vi "New Tutu Outer loop_PN.vi"(6 "Const psi2":dbl=-0.7854, 8 "Const psi1":dbl=0.7854, 11 "Measured stats":dbl[](array[numeric])=[1.0, 0.0, 0.0, 0.156025, 0.156025, 0.156025, 0.0, 0.0, 0.0]) -> (2 "Converged":bool=TRUE, 3 "Corrected stats":dbl[](array[numeric])=[0.5313101533513194, -2.164673295316678e-14, 0.0, 0.20114821816046824, 0.47554583238904846, 0.156025, 1.0016756706463598e-14, 0.0, 0.0] format="%#_3g")   [LabVIEW 2010]
uses:
  XW calib map/Map method.ctl
  XW calib map/XW_Map_Global.vi
panel:
  out "POST PROC. XW Map method":T1=enum."Const. Psi_eff (std.)"
  out "2D true PDF output":string="\t-3.411158E+0\t-3.342246E+0\t-3.273333E+0\t-3.204421E+0\t-3.135509E+0\t-3.066596E+0\t-2.997684E+0\t-2.928772E+0\t-2.859860E+0\t-2.790947E+0\t-2.722035E+0\t-2.653123E+0\t-2.584211E+0\t-2.515298E+0\t-2.446386E+0\t-2.377474E+0\t-2.308561E+0\t-2.239649E+0\t-2.170737E+0\t-2.101825E+0\t-2.032912E+0\t-1.964000E+0\t-1.895088E+0\t-1.826175E+0\t-1.757263E+0\t-1.688351E+0\t-1.619439E+0\t-1.550526E+0\t-1.481614E+0\t-1.412702E+0\t-1.343789E+0\t-1.274877E+0\t-1.205965E+0\t-1.137053E+0\t-1.068140E+0\t-9.992281E-1\t-9.303158E-1\t-8.614035E-1\t-7.924912E-1\t-7.235789E-1\t-6.546667E-1\t-5.857544E-1\t-5.168421E-1\t-4.479298E-1\t-3.790175E-1\t-3.101053E-1\t-2.411930E-1\t-1.722807E-1\t-1.033684E-1\t-3.445614E-2\t3.445614E-2\t1.033684E-1\t1.722807E-1\t2.411930E-1\t3.101053E-1\t3.790175E-1\t4.479298E-1\t5.168421E-1\t5.857544E-1\t6.546667E-1\t7.235789E-1\t7.924912E-1\t8.614035E-1\t9.303158E-1\t9.992281E-1\t1.068140E+0\t1.137053E+0\t1.205965E+0\t1.274877E+0\t1.343789E+0\t1.412702E+0\t1.481614E+0\t1.550526E+0\t1.619439E+0\t1.688351E+0\t1.757263E+0\t1.826175E+0\t1.895088E+0\t1.964000E+0\t2.032912E+0\t2.101825E+0\t2.170737E+0\t2.239649E+0\t2.308561E+0\t2.377474E+0\t2.446386E+0\t2.515298E+0\t2.584211E+0\t2.653123E+0\t2.722035E+0\t2.790947E+0\t2.859860E+0\t2.928772E+0\t2.997684E+0\t3.066596E+0\t3.135509E+0\t3.204421E+0\t3.273333E+0\t3.342246E+0\t3.411158E+0\r\n-1.694652E+0\t1.119788E-11\t1.826614E-11\t2.949991E-11\t4.716912E-11\t7.467200E-11\t1.170364E-10\t1.816130E-10\t2.790205E-10\t4.244127E-10\t6.391513E-10\t9.529760E-10\t1.406771E-9\t2.056022E-9\t2.975056E-9\t4.262119E-9\t6.045318E-9\t8.489374E-9\t1.180308E-8\t1.624718E-8\t2.214235E-8\t2.987668E-8\t3.991206E-8\t5.278845E-8\t6.912526E-8\t8.961850E-8\t1.150328E-7\t1.461869E-7\t1.839326E-7\t2.291246E-7\t2.825842E-7\t3.450539E-7\t4.171470E-7\t4.992917E-7\t5.916742E-7\t6.941830E-7\t8.063588E-7\t9.273544E-7\t1.055908E-6\t1.190336E-6\t1.328545E-6\t1.468067E-6\t1.606122E-6\t1.739699E-6\t1.865661E-6\t1.980863E-6\t2.082281E-6\t2.167141E-6\t2.233048E-6\t2.278096E-6\t2.300959E-6\t2.300959E-6\t2.278096E-6\t2.233048E-6\t2.167141E-6\t2.082281E-6\t1.980863E-6\t1.865661E-6\t1.739699E-6\t1.606122E-6\t1.468067E-6\t1.328545E-6\t1.190336E-6\t1.055908E-6\t9.273544E-7\t8.063588E-7\t6.941830E-7\t5.916742E-7\t4.992917E-7\t4.171470E-7\t3.450539E-7\t2.825842E-7\t2.291246E-7\t1.839326E-7\t1.461869E-7\t1.150328E-7\t8.961850E-8\t6.912526E-8\t5.278845E-8\t3.991206E-8\t2.987668E-8\t2.214235E-8\t1.624718E-8\t1.180308E-8\t8.489374E-9\t6.045318E-9\t4.262119E-9\t2.975056E-9\t2.056022E-9\t1.406771E-9\t9.529760E-10\t6.391513E-10\t4.244127E-10\t2.790205E-10\t1.816130E-10\t1.170364E-10\t7.467200E-11\t4.716912E-11\t2.949991E-11\t1.826614E-11\t1.119788E-11\r\n-1.649695E+0\t1.832407E-11\t2.989048E-11\t4.827329E-11\t7.718695E-11\t1.221923E-10\t1.915169E-10\t2.971893E-10\t4.565857E-10\t6.945037E-10\t1.045899E-9\t1.559438E-9\t2.302022E-9\t3.364448E-9\t4.868344E-9\t6.974479E-9\t9.892483E-9\t1.389191E-8\t1.931441E-8\t2.658668E-8\t3.623346E-8\t4.888983E-8\t6.531159E-8\t8.638237E-8\t1.131157E-7\t1.466506E-7\t1.882382E-7\t2.392185E-7\t3.009850E-7\t3.749366E-7\t4.624172E-7\t5.646419E-7\t6.826142E-7\t8.170348E-7\t9.682084E-7\t1.135952E-6\t1.319516E-6\t1.517511E-6\t1.727875E-6\t1.947852E-6\t2.174014E-6\t2.402326E-6\t2.628237E-6\t2.846822E-6\t3.052945E-6\t3.241460E-6\t3.407419E-6\t3.546282E-6\t3.654132E-6\t3.727847E-6\t3.765261E-6\t3.765261E-6\t3.727847E-6\t3.654132E-6\t3.546282E-6\t3.407419E-6\t3.241460E-6\t3.052945E-6\t2.846822E-6\t2.628237E-6\t2.402326E-6\t2.174014E-6\t1.947852E-6\t1.727875E-6\t1.517511E-6\t1.319516E-6\t1.135952E-6\t9.682084E-7\t8.170348E-7\t6.826142E-7\t5.646419E-7\t4.624172E-7\t3.749366E-7\t3.009850E-7\t2.392185E-7\t1.882382E-7\t1.466506E-7\t1.131157E-7\t8.638237E-8\t6.531159E-8\t4.888983E-8\t3.623346E-8\t2.658668E-8\t1.931441E-8\t1.389191E-8\t9.892483E-9\t6.974479E-9\t4.868344E-9\t3.364448E-9\t2.302022E-9\t1.559438E-9\t1.045899E-9\t6.945037E-10\t4.565857E-10\t2.971893E-10\t1.915169E-10\t1.221923E-10\t7.718695E-11\t4.827329E-11\t2.989048E-11\t1.832407E-11\r\n-1.604737E+0\t2.968549E-11\t4.842339E-11\t7.820403E-11\t1.250449E-10\t1.979549E-10\t3.102625E-10\t4.814547E-10\t7.396812E-10\t1.125115E-9\t1.694385E-9\t2.526332E-9\t3.729338E-9\t5.450497E-9\t7.886849E-9\t1.129884E-8\t1.602609E-8\t2.250526E-8\t3.128986E-8\t4.307114E-8\t5.869918E-8\t7.920284E-8\t1.058065E-7\t1.399418E-7\t1.832505E-7\t2.375779E-7\t3.049510E-7\t3.875404E-7\t4.876037E-7\t6.074074E-7\t7.491283E-7\t9.147351E-7\t1.105853E-6\t1.323618E-6\t1.568524E-6\t1.840274E-6\t2.137651E-6\t2.458409E-6\t2.799204E-6\t3.155572E-6\t3.521962E-6\t3.891833E-6\t4.257815E-6\t4.611928E-6\t4.945853E-6\t5.251253E-6\t5.520110E-6\t5.745073E-6\t5.919792E-6\t6.039213E-6\t6.099824E-6\t6.099824E-6\t6.039213E-6\t5.919792E-6\t5.745073E-6\t5.520110E-6\t5.251253E-6\t4.945853E-6\t4.611928E-6\t4.257815E-6\t3.891833E-6\t3.521962E-6\t3.155572E-6\t2.799204E-6\t2.458409E-6\t2.137651E-6\t1.840274E-6\t1.568524E-6\t1.323618E-6\t1.105853E-6\t9.147351E-7\t7.491283E-7\t6.074074E-7\t4.876037E-7\t3.875404E-7\t3.049510E-7\t2.375779E-7\t1.832505E-7\t1.399418E-7\t1.058065E-7\t7.920284E-8\t5.869918E-8\t4.307114E-8\t3.128986E-8\t2.250526E-8\t1.602609E-8\t1.129884E-8\t7.886849E-9\t5.450497E-9\t3.729338E-9\t2.526332E-9\t1.694385E-9\t1.125115E-9\t7.396812E-10\t4.814547E-10\t3.102625E-10\t1.979549E-10\t1.250449E-10\t7.820403E-11\t4.842339E-11\t2.968549E-11\r\n-1.559779E+0\t4.761048E-11\t7.766288E-11\t1.254260E-10\t2.005508E-10\t3.174859E-10\t4.976083E-10\t7.721714E-10\t1.186323E-9\t1.804493E-9\t2.717505E-9\t4.051806E-9\t5.981223E-9\t8.741670E-9\t1.264916E-8\t1.812142E-8\t2.570312E-8\t3.609461E-8\t5.018362E-8\t6.907878E-8\t9.414350E-8\t1.270279E-7\t1.696957E-7\t2.244428E-7\t2.939026E-7\t3.810346E-7\t4.890895E-7\t6.215489E-7\t7.820335E-7\t9.741782E-7\t1.201474E-6\t1.467080E-6\t1.773601E-6\t2.122859E-6\t2.515645E-6\t2.951486E-6\t3.428428E-6\t3.942870E-6\t4.489448E-6\t5.061001E-6\t5.648628E-6\t6.241838E-6\t6.828812E-6\t7.396748E-6\t7.932307E-6\t8.422117E-6\t8.853317E-6\t9.214120E-6\t9.494339E-6\t9.685870E-6\t9.783080E-6\t9.783080E-6\t9.685870E-6\t9.494339E-6\t9.214120E-6\t8.853317E-6\t8.422117E-6\t7.932307E-6\t7.396748E-6\t6.828812E-6\t6.241838E-6\t5.648628E-6\t5.061001E-6\t4.489448E-6\t3.942870E-6\t3.428428E-6\t2.951486E-6\t2.515645E-6\t2.122859E-6\t1.773601E-6\t1.467080E-6\t1.201474E-6\t9.741782E-7\t7.820335E-7\t6.215489E-7\t4.890895E-7\t3.810346E-7\t2.939026E-7\t2.244428E-7\t1.696957E-7\t1.270279E-7\t9.414350E-8\t6.907878E-8\t5.018362E-8\t3.609461E-8\t2.570312E-8\t1.812142E-8\t1.264916E-8\t8.741670E-9\t5.981223E-9\t4.051806E-9\t2.717505E-9\t1.804493E-9\t1.186323E-9\t7.721714E-10\t4.976083E-10\t3.174859E-10\t2.005508E-10\t1.254260E-10\t7.766288E-11\t4.761048E-11\r\n-1.514821E+0\t7.559567E-11\t1.233127E-10\t1.991507E-10\t3.184336E-10\t5.041025E-10\t7.900998E-10\t1.226050E-9\t1.883637E-9\t2.865164E-9\t4.314841E-9\t6.433437E-9\t9.496956E-9\t1.387998E-8\t2.008428E-8\t2.877310E-8\t4.081128E-8\t5.731084E-8\t7.968129E-8\t1.096829E-7\t1.494806E-7\t2.016942E-7\t2.694419E-7\t3.563691E-7\t4.666571E-7\t6.050047E-7\t7.765738E-7\t9.868922E-7\t1.241709E-6\t1.546795E-6\t1.907695E-6\t2.329421E-6\t2.816114E-6\t3.370664E-6\t3.994328E-6\t4.686354E-6\t5.443641E-6\t6.260469E-6\t7.128322E-6\t8.035831E-6\t8.968862E-6\t9.910759E-6\t1.084275E-5\t1.174452E-5\t1.259488E-5\t1.337259E-5\t1.405725E-5\t1.463013E-5\t1.507506E-5\t1.537917E-5\t1.553352E-5\t1.553352E-5\t1.537917E-5\t1.507506E-5\t1.463013E-5\t1.405725E-5\t1.337259E-5\t1.259488E-5\t1.174452E-5\t1.084275E-5\t9.910759E-6\t8.968862E-6\t8.035831E-6\t7.128322E-6\t6.260469E-6\t5.443641E-6\t4.686354E-6\t3.994328E-6\t3.370664E-6\t2.816114E-6\t2.329421E-6\t1.907695E-6\t1.546795E-6\t1.241709E-6\t9.868922E-7\t7.765738E-7\t6.050047E-7\t4.666571E-7\t3.563691E-7\t2.694419E-7\t2.016942E-7\t1.494806E-7\t1.096829E-7\t7.968129E-8\t5.731084E-8\t4.081128E-8\t2.877310E-8\t2.008428E-8\t1.387998E-8\t9.496956E-9\t6.433437E-9\t4.314841E-9\t2.865164E-9\t1.883637E-9\t1.226050E-9\t7.900998E-10\t5.041025E-10\t3.184336E-10\t1.991507E-10\t1.233127E-10\t7.559567E-11\r\n-1.469864E+0\t1.188304E-10\t1.938377E-10\t3.130490E-10\t5.005521E-10\t7.924089E-10\t1.241974E-9\t1.927252E-9\t2.960927E-9\t4.503809E-9\t6.782584E-9\t1.011285E-8\t1.492845E-8\t2.181822E-8\t3.157088E-8\t4.522902E-8\t6.415207E-8\t9.008806E-8\t1.252526E-7\t1.724128E-7\t2.349715E-7\t3.170472E-7\t4.235412E-7\t5.601837E-7\t7.335476E-7\t9.510191E-7\t1.220712E-6\t1.551316E-6\t1.951867E-6\t2.431438E-6\t2.998744E-6\t3.661664E-6\t4.426706E-6\t5.298415E-6\t6.278765E-6\t7.366574E-6\t8.556968E-6\t9.840956E-6\t1.120515E-5\t1.263168E-5\t1.409833E-5\t1.557892E-5\t1.704394E-5\t1.846144E-5\t1.979814E-5\t2.102065E-5\t2.209688E-5\t2.299740E-5\t2.369679E-5\t2.417483E-5\t2.441746E-5\t2.441746E-5\t2.417483E-5\t2.369679E-5\t2.299740E-5\t2.209688E-5\t2.102065E-5\t1.979814E-5\t1.846144E-5\t1.704394E-5\t1.557892E-5\t1.409833E-5\t1.263168E-5\t1.120515E-5\t9.840956E-6\t8.556968E-6\t7.366574E-6\t6.278765E-6\t5.298415E-6\t4.426706E-6\t3.661664E-6\t2.998744E-6\t2.431438E-6\t1.951867E-6\t1.551316E-6\t1.220712E-6\t9.510191E-7\t7.335476E-7\t5.601837E-7\t4.235412E-7\t3.170472E-7\t2.349715E-7\t1.724128E-7\t1.252526E-7\t9.008806E-8\t6.415207E-8\t4.522902E-8\t3.157088E-8\t2.181822E-8\t1.492845E-8\t1.011285E-8\t6.782584E-9\t4.503809E-9\t2.960927E-9\t1.927252E-9\t1.241974E-9\t7.924089E-10\t5.005521E-10\t3.130490E-10\t1.938377E-10\t1.188304E-10\r\n-1.424906E+0\t1.849243E-10\t3.016510E-10\t4.871680E-10\t7.789612E-10\t1.233150E-9\t1.932765E-9\t2.999198E-9\t4.607807E-9\t7.008845E-9\t1.055509E-8\t1.573766E-8\t2.323172E-8\t3.395360E-8\t4.913073E-8\t7.038558E-8\t9.983371E-8\t1.401954E-7\t1.949186E-7\t2.683095E-7\t3.656636E-7\t4.933901E-7\t6.591165E-7\t8.717601E-7\t1.141550E-6\t1.479980E-6\t1.899677E-6\t2.414163E-6\t3.037503E-6\t3.783814E-6\t4.666657E-6\t5.698296E-6\t6.888858E-6\t8.245414E-6\t9.771039E-6\t1.146389E-5\t1.331639E-5\t1.531454E-5\t1.743750E-5\t1.965748E-5\t2.193988E-5\t2.424398E-5\t2.652385E-5\t2.872977E-5\t3.080994E-5\t3.271242E-5\t3.438725E-5\t3.578864E-5\t3.687704E-5\t3.762097E-5\t3.799855E-5\t3.799855E-5\t3.762097E-5\t3.687704E-5\t3.578864E-5\t3.438725E-5\t3.271242E-5\t3.080994E-5\t2.872977E-5\t2.652385E-5\t2.424398E-5\t2.193988E-5\t1.965748E-5\t1.743750E-5\t1.531454E-5\t1.331639E-5\t1.146389E-5\t9.771039E-6\t8.245414E-6\t6.888858E-6\t5.698296E-6\t4.666657E-6\t3.783814E-6\t3.037503E-6\t2.414163E-6\t1.899677E-6\t1.479980E-6\t1.141550E-6\t8.717601E-7\t6.591165E-7\t4.933901E-7\t3.656636E-7\t2.683095E-7\t1.949186E-7\t1.401954E-7\t9.983371E-8\t7.038558E-8\t4.913073E-8\t3.395360E-8\t2.323172E-8\t1.573766E-8\t1.055509E-8\t7.008845E-9\t4.607807E-9\t2.999198E-9\t1.932765E-9\t1.233150E-9\t7.789612E-10\t4.871680E-10\t3.016510E-10\t1.849243E-10\r\n-1.379948E+0\t2.849027E-10\t4.647372E-10\t7.505530E-10\t1.200103E-9\t1.899846E-9\t2.977704E-9\t4.620699E-9\t7.098995E-9\t1.079814E-8\t1.626164E-8\t2.424614E-8\t3.579184E-8\t5.231044E-8\t7.569302E-8\t1.084392E-7\t1.538083E-7\t2.159913E-7\t3.003004E-7\t4.133697E-7\t5.633578E-7\t7.601390E-7\t1.015465E-6\t1.343073E-6\t1.758723E-6\t2.280123E-6\t2.926728E-6\t3.719369E-6\t4.679714E-6\t5.829514E-6\t7.189662E-6\t8.779052E-6\t1.061328E-5\t1.270326E-5\t1.505370E-5\t1.766179E-5\t2.051583E-5\t2.359426E-5\t2.686500E-5\t3.028519E-5\t3.380157E-5\t3.735137E-5\t4.086383E-5\t4.426238E-5\t4.746718E-5\t5.039822E-5\t5.297854E-5\t5.513760E-5\t5.681444E-5\t5.796057E-5\t5.854227E-5\t5.854227E-5\t5.796057E-5\t5.681444E-5\t5.513760E-5\t5.297854E-5\t5.039822E-5\t4.746718E-5\t4.426238E-5\t4.086383E-5\t3.735137E-5\t3.380157E-5\t3.028519E-5\t2.686500E-5\t2.359426E-5\t2.051583E-5\t1.766179E-5\t1.505370E-5\t1.270326E-5\t1.061328E-5\t8.779052E-6\t7.189662E-6\t5.829514E-6\t4.679714E-6\t3.719369E-6\t2.926728E-6\t2.280123E-6\t1.758723E-6\t1.343073E-6\t1.015465E-6\t7.601390E-7\t5.633578E-7\t4.133697E-7\t3.003004E-7\t2.159913E-7\t1.538083E-7\t1.084392E-7\t7.569302E-8\t5.231044E-8\t3.579184E-8\t2.424614E-8\t1.626164E-8\t1.079814E-8\t7.098995E-9\t4.620699E-9\t2.977704E-9\t1.899846E-9\t1.200103E-9\t7.505530E-10\t4.647372E-10\t2.849027E-10\r\n-1.334990E+0\t4.345454E-10\t7.088365E-10\t1.144775E-9\t1.830447E-9\t2.897725E-9\t4.541718E-9\t7.047683E-9\t1.082768E-8\t1.646978E-8\t2.480293E-8\t3.698123E-8\t5.459120E-8\t7.978606E-8\t1.154501E-7\t1.653960E-7\t2.345948E-7\t3.294390E-7\t4.580307E-7\t6.304886E-7\t8.592568E-7\t1.159396E-6\t1.548829E-6\t2.048511E-6\t2.682478E-6\t3.477739E-6\t4.463967E-6\t5.672937E-6\t7.137695E-6\t8.891418E-6\t1.096597E-5\t1.339018E-5\t1.618782E-5\t1.937554E-5\t2.296054E-5\t2.693849E-5\t3.129159E-5\t3.598695E-5\t4.097562E-5\t4.619224E-5\t5.155557E-5\t5.696986E-5\t6.232722E-5\t6.751083E-5\t7.239893E-5\t7.686947E-5\t8.080508E-5\t8.409816E-5\t8.665575E-5\t8.840387E-5\t8.929111E-5\t8.929111E-5\t8.840387E-5\t8.665575E-5\t8.409816E-5\t8.080508E-5\t7.686947E-5\t7.239893E-5\t6.751083E-5\t6.232722E-5\t5.696986E-5\t5.155557E-5\t4.619224E-5\t4.097562E-5\t3.598695E-5\t3.129159E-5\t2.693849E-5\t2.296054E-5\t1.937554E-5\t1.618782E-5\t1.339018E-5\t1.096597E-5\t8.891418E-6\t7.137695E-6\t5.672937E-6\t4.463967E-6\t3.477739E-6\t2.682478E-6\t2.048511E-6\t1.548829E-6\t1.159396E-6\t8.592568E-7\t6.304886E-7\t4.580307E-7\t3.294390E-7\t2.345948E-7\t1.653960E-7\t1.154501E-7\t7.978606E-8\t5.459120E-8\t3.698123E-8\t2.480293E-8\t1.646978E-8\t1.082768E-8\t7.047683E-9\t4.541718E-9\t2.897725E-9\t1.830447E-9\t1.144775E-9\t7.088365E-10\t4.345454E-10\r\n-1.290033E+0\t6.561602E-10\t1.070338E-9\t1.728601E-9\t2.763960E-9\t4.375542E-9\t6.857960E-9\t1.064195E-8\t1.634972E-8\t2.486924E-8\t3.745224E-8\t5.584137E-8\t8.243230E-8\t1.204763E-7\t1.743288E-7\t2.497467E-7\t3.542364E-7\t4.974504E-7\t6.916229E-7\t9.520330E-7\t1.297471E-6\t1.750679E-6\t2.338720E-6\t3.093236E-6\t4.050521E-6\t5.251360E-6\t6.740556E-6\t8.566091E-6\t1.077786E-5\t1.342597E-5\t1.655853E-5\t2.021906E-5\t2.444349E-5\t2.925691E-5\t3.467023E-5\t4.067692E-5\t4.725007E-5\t5.434003E-5\t6.187287E-5\t6.974993E-5\t7.784851E-5\t8.602405E-5\t9.411363E-5\t1.019408E-4\t1.093218E-4\t1.160723E-4\t1.220151E-4\t1.269876E-4\t1.308495E-4\t1.334892E-4\t1.348289E-4\t1.348289E-4\t1.334892E-4\t1.308495E-4\t1.269876E-4\t1.220151E-4\t1.160723E-4\t1.093218E-4\t1.019408E-4\t9.411363E-5\t8.602405E-5\t7.784851E-5\t6.974993E-5\t6.187287E-5\t5.434003E-5\t4.725007E-5\t4.067692E-5\t3.467023E-5\t2.925691E-5\t2.444349E-5\t2.021906E-5\t1.655853E-5\t1.342597E-5\t1.077786E-5\t8.566091E-6\t6.740556E-6\t5.251360E-6\t4.050521E-6\t3.093236E-6\t2.338720E-6\t1.750679E-6\t1.297471E-6\t9.520330E-7\t6.916229E-7\t4.974504E-7\t3.542364E-7\t2.497467E-7\t1.743288E-7\t1.204763E-7\t8.243230E-8\t5.584137E-8\t3.745224E-8\t2.486924E-8\t1.634972E-8\t1.064195E-8\t6.857960E-9\t4.375542E-9\t2.763960E-9\t1.728601E-9\t1.070338E-9\t6.561602E-10\r\n-1.245075E+0\t9.808909E-10\t1.600043E-9\t2.584078E-9\t4.131832E-9\t6.540978E-9\t1.025193E-8\t1.590860E-8\t2.444112E-8\t3.717691E-8\t5.598718E-8\t8.347701E-8\t1.232277E-7\t1.800995E-7\t2.606034E-7\t3.733451E-7\t5.295464E-7\t7.436363E-7\t1.033904E-6\t1.423190E-6\t1.939584E-6\t2.617081E-6\t3.496142E-6\t4.624064E-6\t6.055105E-6\t7.850233E-6\t1.007643E-5\t1.280541E-5\t1.611178E-5\t2.007043E-5\t2.475328E-5\t3.022539E-5\t3.654046E-5\t4.373602E-5\t5.182837E-5\t6.080774E-5\t7.063391E-5\t8.123266E-5\t9.249348E-5\t1.042689E-4\t1.163754E-4\t1.285970E-4\t1.406900E-4\t1.523909E-4\t1.634247E-4\t1.735160E-4\t1.823997E-4\t1.898331E-4\t1.956063E-4\t1.995523E-4\t2.015551E-4\t2.015551E-4\t1.995523E-4\t1.956063E-4\t1.898331E-4\t1.823997E-4\t1.735160E-4\t1.634247E-4\t1.523909E-4\t1.406900E-4\t1.285970E-4\t1.163754E-4\t1.042689E-4\t9.249348E-5\t8.123266E-5\t7.063391E-5\t6.080774E-5\t5.182837E-5\t4.373602E-5\t3.654046E-5\t3.022539E-5\t2.475328E-5\t2.007043E-5\t1.611178E-5\t1.280541E-5\t1.007643E-5\t7.850233E-6\t6.055105E-6\t4.624064E-6\t3.496142E-6\t2.617081E-6\t1.939584E-6\t1.423190E-6\t1.033904E-6\t7.436363E-7\t5.295464E-7\t3.733451E-7\t2.606034E-7\t1.800995E-7\t1.232277E-7\t8.347701E-8\t5.598718E-8\t3.717691E-8\t2.444112E-8\t1.590860E-8\t1.025193E-8\t6.540978E-9\t4.131832E-9\t2.584078E-9\t1.600043E-9\t9.808909E-10\r\n-1.200117E+0\t1.451669E-9\t2.367983E-9\t3.824305E-9\t6.114902E-9\t9.680316E-9\t1.517234E-8\t2.354392E-8\t3.617162E-8\t5.501995E-8\t8.285819E-8\t1.235417E-7\t1.823707E-7\t2.665382E-7\t3.856798E-7\t5.525319E-7\t7.837019E-7\t1.100544E-6\t1.530126E-6\t2.106249E-6\t2.870486E-6\t3.873148E-6\t5.174113E-6\t6.843381E-6\t8.961249E-6\t1.161795E-5\t1.491260E-5\t1.895136E-5\t2.384462E-5\t2.970322E-5\t3.663360E-5\t4.473204E-5\t5.407804E-5\t6.472710E-5\t7.670337E-5\t8.999239E-5\t1.045346E-4\t1.202202E-4\t1.368857E-4\t1.543126E-4\t1.722297E-4\t1.903170E-4\t2.082141E-4\t2.255308E-4\t2.418603E-4\t2.567949E-4\t2.699424E-4\t2.809435E-4\t2.894875E-4\t2.953274E-4\t2.982914E-4\t2.982914E-4\t2.953274E-4\t2.894875E-4\t2.809435E-4\t2.699424E-4\t2.567949E-4\t2.418603E-4\t2.255308E-4\t2.082141E-4\t1.903170E-4\t1.722297E-4\t1.543126E-4\t1.368857E-4\t1.202202E-4\t1.045346E-4\t8.999239E-5\t7.670337E-5\t6.472710E-5\t5.407804E-5\t4.473204E-5\t3.663360E-5\t2.970322E-5\t2.384462E-5\t1.895136E-5\t1.491260E-5\t1.161795E-5\t8.961249E-6\t6.843381E-6\t5.174113E-6\t3.873148E-6\t2.870486E-6\t2.106249E-6\t1.530126E-6\t1.100544E-6\t7.837019E-7\t5.525319E-7\t3.856798E-7\t2.665382E-7\t1.823707E-7\t1.235417E-7\t8.285819E-8\t5.501995E-8\t3.617162E-8\t2.354392E-8\t1.517234E-8\t9.680316E-9\t6.114902E-9\t3.824305E-9\t2.367983E-9\t1.451669E-9\r\n-1.155159E+0\t2.126917E-9\t3.469457E-9\t5.603191E-9\t8.959267E-9\t1.418314E-8\t2.222980E-8\t3.449544E-8\t5.299695E-8\t8.061264E-8\t1.213999E-7\t1.810076E-7\t2.672010E-7\t3.905192E-7\t5.650799E-7\t8.095438E-7\t1.148243E-6\t1.612465E-6\t2.241868E-6\t3.085977E-6\t4.205701E-6\t5.674754E-6\t7.580866E-6\t1.002660E-5\t1.312960E-5\t1.702207E-5\t2.184924E-5\t2.776664E-5\t3.493601E-5\t4.351975E-5\t5.367382E-5\t6.553928E-5\t7.923260E-5\t9.483510E-5\t1.123822E-4\t1.318526E-4\t1.531592E-4\t1.761410E-4\t2.005584E-4\t2.260916E-4\t2.523428E-4\t2.788435E-4\t3.050655E-4\t3.304371E-4\t3.543623E-4\t3.762437E-4\t3.955069E-4\t4.116251E-4\t4.241434E-4\t4.326998E-4\t4.370425E-4\t4.370425E-4\t4.326998E-4\t4.241434E-4\t4.116251E-4\t3.955069E-4\t3.762437E-4\t3.543623E-4\t3.304371E-4\t3.050655E-4\t2.788435E-4\t2.523428E-4\t2.260916E-4\t2.005584E-4\t1.761410E-4\t1.531592E-4\t1.318526E-4\t1.123822E-4\t9.483510E-5\t7.923260E-5\t6.553928E-5\t5.367382E-5\t4.351975E-5\t3.493601E-5\t2.776664E-5\t2.184924E-5\t1.702207E-5\t1.312960E-5\t1.002660E-5\t7.580866E-6\t5.674754E-6\t4.205701E-6\t3.085977E-6\t2.241868E-6\t1.612465E-6\t1.148243E-6\t8.095438E-7\t5.650799E-7\t3.905192E-7\t2.672010E-7\t1.810076E-7\t1.213999E-7\t8.061264E-8\t5.299695E-8\t3.449544E-8\t2.222980E-8\t1.418314E-8\t8.959267E-9\t5.603191E-9\t3.469457E-9\t2.126917E-9\r\n-1.110201E+0\t3.085102E-9\t5.032462E-9\t8.127453E-9\t1.299546E-8\t2.057271E-8\t3.224442E-8\t5.003579E-8\t7.687231E-8\t1.169290E-7\t1.760911E-7\t2.625522E-7\t3.875762E-7\t5.664499E-7\t8.196509E-7\t1.174247E-6\t1.665532E-6\t2.338888E-6\t3.251839E-6\t4.476223E-6\t6.100387E-6\t8.231256E-6\t1.099608E-5\t1.454363E-5\t1.904454E-5\t2.469059E-5\t3.169242E-5\t4.027563E-5\t5.067484E-5\t6.312559E-5\t7.785411E-5\t9.506501E-5\t1.149272E-4\t1.375587E-4\t1.630108E-4\t1.912528E-4\t2.221581E-4\t2.554933E-4\t2.909109E-4\t3.279468E-4\t3.660244E-4\t4.044637E-4\t4.424989E-4\t4.793005E-4\t5.140041E-4\t5.457432E-4\t5.736845E-4\t5.970640E-4\t6.152219E-4\t6.276329E-4\t6.339320E-4\t6.339320E-4\t6.276329E-4\t6.152219E-4\t5.970640E-4\t5.736845E-4\t5.457432E-4\t5.140041E-4\t4.793005E-4\t4.424989E-4\t4.044637E-4\t3.660244E-4\t3.279468E-4\t2.909109E-4\t2.554933E-4\t2.221581E-4\t1.912528E-4\t1.630108E-4\t1.375587E-4\t1.149272E-4\t9.506501E-5\t7.785411E-5\t6.312559E-5\t5.067484E-5\t4.027563E-5\t3.169242E-5\t2.469059E-5\t1.904454E-5\t1.454363E-5\t1.099608E-5\t8.231256E-6\t6.100387E-6\t4.476223E-6\t3.251839E-6\t2.338888E-6\t1.665532E-6\t1.174247E-6\t8.196509E-7\t5.664499E-7\t3.875762E-7\t2.625522E-7\t1.760911E-7\t1.169290E-7\t7.687231E-8\t5.003579E-8\t3.224442E-8\t2.057271E-8\t1.299546E-8\t8.127453E-9\t5.032462E-9\t3.085102E-9\r\n-1.065244E+0\t4.430214E-9\t7.226627E-9\t1.167104E-8\t1.866150E-8\t2.954246E-8\t4.630306E-8\t7.185150E-8\t1.103888E-7\t1.679103E-7\t2.528672E-7\t3.770256E-7\t5.565602E-7\t8.134232E-7\t1.177020E-6\t1.686221E-6\t2.391707E-6\t3.358648E-6\t4.669648E-6\t6.427866E-6\t8.760169E-6\t1.182010E-5\t1.579039E-5\t2.088468E-5\t2.734800E-5\t3.545574E-5\t4.551038E-5\t5.783590E-5\t7.276918E-5\t9.064849E-5\t1.117987E-4\t1.365136E-4\t1.650357E-4\t1.975346E-4\t2.340839E-4\t2.746394E-4\t3.190195E-4\t3.668889E-4\t4.177487E-4\t4.709324E-4\t5.256118E-4\t5.808108E-4\t6.354294E-4\t6.882765E-4\t7.381110E-4\t7.836884E-4\t8.238121E-4\t8.573853E-4\t8.834600E-4\t9.012822E-4\t9.103277E-4\t9.103277E-4\t9.012822E-4\t8.834600E-4\t8.573853E-4\t8.238121E-4\t7.836884E-4\t7.381110E-4\t6.882765E-4\t6.354294E-4\t5.808108E-4\t5.256118E-4\t4.709324E-4\t4.177487E-4\t3.668889E-4\t3.190195E-4\t2.746394E-4\t2.340839E-4\t1.975346E-4\t1.650357E-4\t1.365136E-4\t1.117987E-4\t9.064849E-5\t7.276918E-5\t5.783590E-5\t4.551038E-5\t3.545574E-5\t2.734800E-5\t2.088468E-5\t1.579039E-5\t1.182010E-5\t8.760169E-6\t6.427866E-6\t4.669648E-6\t3.358648E-6\t2.391707E-6\t1.686221E-6\t1.177020E-6\t8.134232E-7\t5.565602E-7\t3.770256E-7\t2.528672E-7\t1.679103E-7\t1.103888E-7\t7.185150E-8\t4.630306E-8\t2.954246E-8\t1.866150E-8\t1.167104E-8\t7.226627E-9\t4.430214E-9\r\n-1.020286E+0\t6.298192E-9\t1.027370E-8\t1.659208E-8\t2.653003E-8\t4.199889E-8\t6.582652E-8\t1.021473E-7\t1.569337E-7\t2.387088E-7\t3.594874E-7\t5.359966E-7\t7.912311E-7\t1.156399E-6\t1.673305E-6\t2.397208E-6\t3.400158E-6\t4.774806E-6\t6.638582E-6\t9.138143E-6\t1.245385E-5\t1.680399E-5\t2.244834E-5\t2.969060E-5\t3.887915E-5\t5.040548E-5\t6.469961E-5\t8.222211E-5\t1.034519E-4\t1.288700E-4\t1.589380E-4\t1.940738E-4\t2.346222E-4\t2.808241E-4\t3.327842E-4\t3.904397E-4\t4.535325E-4\t5.215858E-4\t5.938903E-4\t6.694987E-4\t7.472334E-4\t8.257068E-4\t9.033550E-4\t9.784849E-4\t1.049332E-3\t1.114127E-3\t1.171168E-3\t1.218898E-3\t1.255967E-3\t1.281303E-3\t1.294163E-3\t1.294163E-3\t1.281303E-3\t1.255967E-3\t1.218898E-3\t1.171168E-3\t1.114127E-3\t1.049332E-3\t9.784849E-4\t9.033550E-4\t8.257068E-4\t7.472334E-4\t6.694987E-4\t5.938903E-4\t5.215858E-4\t4.535325E-4\t3.904397E-4\t3.327842E-4\t2.808241E-4\t2.346222E-4\t1.940738E-4\t1.589380E-4\t1.288700E-4\t1.034519E-4\t8.222211E-5\t6.469961E-5\t5.040548E-5\t3.887915E-5\t2.969060E-5\t2.244834E-5\t1.680399E-5\t1.245385E-5\t9.138143E-6\t6.638582E-6\t4.774806E-6\t3.400158E-6\t2.397208E-6\t1.673305E-6\t1.156399E-6\t7.912311E-7\t5.359966E-7\t3.594874E-7\t2.387088E-7\t1.569337E-7\t1.021473E-7\t6.582652E-8\t4.199889E-8\t2.653003E-8\t1.659208E-8\t1.027370E-8\t6.298192E-9\r\n-9.753281E-1\t8.864273E-9\t1.445953E-8\t2.335221E-8\t3.733920E-8\t5.911056E-8\t9.264632E-8\t1.437654E-7\t2.208734E-7\t3.359663E-7\t5.059539E-7\t7.543784E-7\t1.113604E-6\t1.627552E-6\t2.355062E-6\t3.373905E-6\t4.785490E-6\t6.720212E-6\t9.343349E-6\t1.286131E-5\t1.752794E-5\t2.365046E-5\t3.159449E-5\t4.178748E-5\t5.471974E-5\t7.094225E-5\t9.106026E-5\t1.157220E-4\t1.456015E-4\t1.813756E-4\t2.236944E-4\t2.731456E-4\t3.302147E-4\t3.952407E-4\t4.683709E-4\t5.495172E-4\t6.383159E-4\t7.340963E-4\t8.358599E-4\t9.422735E-4\t1.051680E-3\t1.162126E-3\t1.271410E-3\t1.377150E-3\t1.476863E-3\t1.568057E-3\t1.648339E-3\t1.715515E-3\t1.767687E-3\t1.803347E-3\t1.821445E-3\t1.821445E-3\t1.803347E-3\t1.767687E-3\t1.715515E-3\t1.648339E-3\t1.568057E-3\t1.476863E-3\t1.377150E-3\t1.271410E-3\t1.162126E-3\t1.051680E-3\t9.422735E-4\t8.358599E-4\t7.340963E-4\t6.383159E-4\t5.495172E-4\t4.683709E-4\t3.952407E-4\t3.302147E-4\t2.731456E-4\t2.236944E-4\t1.813756E-4\t1.456015E-4\t1.157220E-4\t9.106026E-5\t7.094225E-5\t5.471974E-5\t4.178748E-5\t3.159449E-5\t2.365046E-5\t1.752794E-5\t1.286131E-5\t9.343349E-6\t6.720212E-6\t4.785490E-6\t3.373905E-6\t2.355062E-6\t1.627552E-6\t1.113604E-6\t7.543784E-7\t5.059539E-7\t3.359663E-7\t2.208734E-7\t1.437654E-7\t9.264632E-8\t5.911056E-8\t3.733920E-8\t2.335221E-8\t1.445953E-8\t8.864273E-9\r\n-9.303704E-1\t1.235112E-8\t2.014732E-8\t3.253803E-8\t5.202694E-8\t8.236228E-8\t1.290897E-7\t2.003169E-7\t3.077562E-7\t4.681219E-7\t7.049759E-7\t1.051121E-6\t1.551651E-6\t2.267766E-6\t3.281450E-6\t4.701064E-6\t6.667910E-6\t9.363674E-6\t1.301865E-5\t1.792043E-5\t2.442273E-5\t3.295361E-5\t4.402250E-5\t5.822500E-5\t7.624430E-5\t9.884809E-5\t1.268797E-4\t1.612424E-4\t2.028753E-4\t2.527216E-4\t3.116868E-4\t3.805902E-4\t4.601080E-4\t5.507126E-4\t6.526093E-4\t7.656752E-4\t8.894037E-4\t1.022860E-3\t1.164654E-3\t1.312926E-3\t1.465368E-3\t1.619259E-3\t1.771532E-3\t1.918866E-3\t2.057801E-3\t2.184868E-3\t2.296730E-3\t2.390329E-3\t2.463024E-3\t2.512711E-3\t2.537929E-3\t2.537929E-3\t2.512711E-3\t2.463024E-3\t2.390329E-3\t2.296730E-3\t2.184868E-3\t2.057801E-3\t1.918866E-3\t1.771532E-3\t1.619259E-3\t1.465368E-3\t1.312926E-3\t1.164654E-3\t1.022860E-3\t8.894037E-4\t7.656752E-4\t6.526093E-4\t5.507126E-4\t4.601080E-4\t3.805902E-4\t3.116868E-4\t2.527216E-4\t2.028753E-4\t1.612424E-4\t1.268797E-4\t9.884809E-5\t7.624430E-5\t5.822500E-5\t4.402250E-5\t3.295361E-5\t2.442273E-5\t1.792043E-5\t1.301865E-5\t9.363674E-6\t6.667910E-6\t4.701064E-6\t3.281450E-6\t2.267766E-6\t1.551651E-6\t1.051121E-6\t7.049759E-7\t4.681219E-7\t3.077562E-7\t2.003169E-7\t1.290897E-7\t8.236228E-8\t5.202694E-8\t3.253803E-8\t2.014732E-8\t1.235112E-8\r\n-8.854126E-1\t1.703750E-8\t2.779180E-8\t4.488391E-8\t7.176748E-8\t1.136129E-7\t1.780700E-7\t2.763230E-7\t4.245278E-7\t6.457410E-7\t9.724643E-7\t1.449946E-6\t2.140392E-6\t3.128223E-6\t4.526527E-6\t6.484785E-6\t9.197909E-6\t1.291652E-5\t1.795830E-5\t2.471997E-5\t3.368942E-5\t4.545716E-5\t6.072592E-5\t8.031726E-5\t1.051736E-4\t1.363539E-4\t1.750216E-4\t2.224224E-4\t2.798521E-4\t3.486115E-4\t4.299498E-4\t5.249971E-4\t6.346863E-4\t7.596689E-4\t9.002283E-4\t1.056195E-3\t1.226869E-3\t1.410963E-3\t1.606557E-3\t1.811089E-3\t2.021372E-3\t2.233653E-3\t2.443703E-3\t2.646940E-3\t2.838591E-3\t3.013870E-3\t3.168176E-3\t3.297290E-3\t3.397567E-3\t3.466107E-3\t3.500893E-3\t3.500893E-3\t3.466107E-3\t3.397567E-3\t3.297290E-3\t3.168176E-3\t3.013870E-3\t2.838591E-3\t2.646940E-3\t2.443703E-3\t2.233653E-3\t2.021372E-3\t1.811089E-3\t1.606557E-3\t1.410963E-3\t1.226869E-3\t1.056195E-3\t9.002283E-4\t7.596689E-4\t6.346863E-4\t5.249971E-4\t4.299498E-4\t3.486115E-4\t2.798521E-4\t2.224224E-4\t1.750216E-4\t1.363539E-4\t1.051736E-4\t8.031726E-5\t6.072592E-5\t4.545716E-5\t3.368942E-5\t2.471997E-5\t1.795830E-5\t1.291652E-5\t9.197909E-6\t6.484785E-6\t4.526527E-6\t3.128223E-6\t2.140392E-6\t1.449946E-6\t9.724643E-7\t6.457410E-7\t4.245278E-7\t2.763230E-7\t1.780700E-7\t1.136129E-7\t7.176748E-8\t4.488391E-8\t2.779180E-8\t1.703750E-8\r\n-8.404548E-1\t2.326705E-8\t3.795353E-8\t6.129516E-8\t9.800837E-8\t1.551541E-7\t2.431791E-7\t3.773570E-7\t5.797512E-7\t8.818482E-7\t1.328034E-6\t1.980101E-6\t2.923000E-6\t4.272019E-6\t6.181595E-6\t8.855866E-6\t1.256101E-5\t1.763929E-5\t2.452453E-5\t3.375852E-5\t4.600754E-5\t6.207801E-5\t8.292960E-5\t1.096843E-4\t1.436290E-4\t1.862101E-4\t2.390160E-4\t3.037484E-4\t3.821766E-4\t4.760769E-4\t5.871557E-4\t7.169558E-4\t8.667515E-4\t1.037432E-3\t1.229386E-3\t1.442379E-3\t1.675459E-3\t1.926865E-3\t2.193975E-3\t2.473291E-3\t2.760461E-3\t3.050361E-3\t3.337213E-3\t3.614761E-3\t3.876486E-3\t4.115854E-3\t4.326580E-3\t4.502903E-3\t4.639845E-3\t4.733446E-3\t4.780952E-3\t4.780952E-3\t4.733446E-3\t4.639845E-3\t4.502903E-3\t4.326580E-3\t4.115854E-3\t3.876486E-3\t3.614761E-3\t3.337213E-3\t3.050361E-3\t2.760461E-3\t2.473291E-3\t2.193975E-3\t1.926865E-3\t1.675459E-3\t1.442379E-3\t1.229386E-3\t1.037432E-3\t8.667515E-4\t7.169558E-4\t5.871557E-4\t4.760769E-4\t3.821766E-4\t3.037484E-4\t2.390160E-4\t1.862101E-4\t1.436290E-4\t1.096843E-4\t8.292960E-5\t6.207801E-5\t4.600754E-5\t3.375852E-5\t2.452453E-5\t1.763929E-5\t1.256101E-5\t8.855866E-6\t6.181595E-6\t4.272019E-6\t2.923000E-6\t1.980101E-6\t1.328034E-6\t8.818482E-7\t5.797512E-7\t3.773570E-7\t2.431791E-7\t1.551541E-7\t9.800837E-8\t6.129516E-8\t3.795353E-8\t2.326705E-8\r\n-7.954971E-1\t3.145667E-8\t5.131257E-8\t8.287007E-8\t1.325057E-7\t2.097658E-7\t3.287743E-7\t5.101806E-7\t7.838143E-7\t1.192245E-6\t1.795480E-6\t2.677065E-6\t3.951849E-6\t5.775701E-6\t8.357418E-6\t1.197299E-5\t1.698228E-5\t2.384804E-5\t3.315677E-5\t4.564097E-5\t6.220146E-5\t8.392847E-5\t1.121195E-4\t1.482914E-4\t1.941841E-4\t2.517530E-4\t3.231459E-4\t4.106630E-4\t5.166966E-4\t6.436484E-4\t7.938250E-4\t9.693128E-4\t1.171834E-3\t1.402592E-3\t1.662110E-3\t1.950073E-3\t2.265194E-3\t2.605090E-3\t2.966219E-3\t3.343849E-3\t3.732099E-3\t4.124039E-3\t4.511858E-3\t4.887098E-3\t5.240947E-3\t5.564569E-3\t5.849467E-3\t6.087853E-3\t6.272996E-3\t6.399542E-3\t6.463770E-3\t6.463770E-3\t6.399542E-3\t6.272996E-3\t6.087853E-3\t5.849467E-3\t5.564569E-3\t5.240947E-3\t4.887098E-3\t4.511858E-3\t4.124039E-3\t3.732099E-3\t3.343849E-3\t2.966219E-3\t2.605090E-3\t2.265194E-3\t1.950073E-3\t1.662110E-3\t1.402592E-3\t1.171834E-3\t9.693128E-4\t7.938250E-4\t6.436484E-4\t5.166966E-4\t4.106630E-4\t3.231459E-4\t2.517530E-4\t1.941841E-4\t1.482914E-4\t1.121195E-4\t8.392847E-5\t6.220146E-5\t4.564097E-5\t3.315677E-5\t2.384804E-5\t1.698228E-5\t1.197299E-5\t8.357418E-6\t5.775701E-6\t3.951849E-6\t2.677065E-6\t1.795480E-6\t1.192245E-6\t7.838143E-7\t5.101806E-7\t3.287743E-7\t2.097658E-7\t1.325057E-7\t8.287007E-8\t5.131257E-8\t3.145667E-8\r\n-7.505393E-1\t4.210371E-8\t6.868017E-8\t1.109188E-7\t1.773545E-7\t2.807646E-7\t4.400535E-7\t6.828599E-7\t1.049109E-6\t1.595780E-6\t2.403191E-6\t3.583163E-6\t5.289418E-6\t7.730584E-6\t1.118613E-5\t1.602545E-5\t2.273022E-5\t3.191981E-5\t4.437924E-5\t6.108893E-5\t8.325459E-5\t1.123355E-4\t1.500682E-4\t1.984831E-4\t2.599090E-4\t3.369630E-4\t4.325200E-4\t5.496588E-4\t6.915812E-4\t8.615020E-4\t1.062508E-3\t1.297393E-3\t1.568461E-3\t1.877323E-3\t2.224678E-3\t2.610109E-3\t3.031886E-3\t3.486826E-3\t3.970185E-3\t4.475631E-3\t4.995291E-3\t5.519890E-3\t6.038972E-3\t6.541219E-3\t7.014833E-3\t7.447990E-3\t7.829317E-3\t8.148389E-3\t8.396197E-3\t8.565575E-3\t8.651541E-3\t8.651541E-3\t8.565575E-3\t8.396197E-3\t8.148389E-3\t7.829317E-3\t7.447990E-3\t7.014833E-3\t6.541219E-3\t6.038972E-3\t5.519890E-3\t4.995291E-3\t4.475631E-3\t3.970185E-3\t3.486826E-3\t3.031886E-3\t2.610109E-3\t2.224678E-3\t1.877323E-3\t1.568461E-3\t1.297393E-3\t1.062508E-3\t8.615020E-4\t6.915812E-4\t5.496588E-4\t4.325200E-4\t3.369630E-4\t2.599090E-4\t1.984831E-4\t1.500682E-4\t1.123355E-4\t8.325459E-5\t6.108893E-5\t4.437924E-5\t3.191981E-5\t2.273022E-5\t1.602545E-5\t1.118613E-5\t7.730584E-6\t5.289418E-6\t3.583163E-6\t2.403191E-6\t1.595780E-6\t1.049109E-6\t6.828599E-7\t4.400535E-7\t2.807646E-7\t1.773545E-7\t1.109188E-7\t6.868017E-8\t4.210371E-8\r\n-7.055815E-1\t5.579099E-8\t9.100704E-8\t1.469769E-7\t2.350098E-7\t3.720369E-7\t5.831082E-7\t9.048472E-7\t1.390159E-6\t2.114544E-6\t3.184432E-6\t4.747995E-6\t7.008927E-6\t1.024368E-5\t1.482257E-5\t2.123508E-5\t3.011947E-5\t4.229645E-5\t5.880626E-5\t8.094801E-5\t1.103194E-4\t1.488540E-4\t1.988531E-4\t2.630069E-4\t3.444015E-4\t4.465046E-4\t5.731257E-4\t7.283445E-4\t9.164038E-4\t1.141563E-3\t1.407914E-3\t1.719156E-3\t2.078344E-3\t2.487612E-3\t2.947888E-3\t3.458615E-3\t4.017507E-3\t4.620341E-3\t5.260832E-3\t5.930591E-3\t6.619184E-3\t7.314322E-3\t8.002150E-3\t8.667669E-3\t9.295249E-3\t9.869219E-3\t1.037451E-2\t1.079731E-2\t1.112567E-2\t1.135011E-2\t1.146403E-2\t1.146403E-2\t1.135011E-2\t1.112567E-2\t1.079731E-2\t1.037451E-2\t9.869219E-3\t9.295249E-3\t8.667669E-3\t8.002150E-3\t7.314322E-3\t6.619184E-3\t5.930591E-3\t5.260832E-3\t4.620341E-3\t4.017507E-3\t3.458615E-3\t2.947888E-3\t2.487612E-3\t2.078344E-3\t1.719156E-3\t1.407914E-3\t1.141563E-3\t9.164038E-4\t7.283445E-4\t5.731257E-4\t4.465046E-4\t3.444015E-4\t2.630069E-4\t1.988531E-4\t1.488540E-4\t1.103194E-4\t8.094801E-5\t5.880626E-5\t4.229645E-5\t3.011947E-5\t2.123508E-5\t1.482257E-5\t1.024368E-5\t7.008927E-6\t4.747995E-6\t3.184432E-6\t2.114544E-6\t1.390159E-6\t9.048472E-7\t5.831082E-7\t3.720369E-7\t2.350098E-7\t1.469769E-7\t9.100704E-8\t5.579099E-8\r\n-6.606238E-1\t7.318867E-8\t1.193864E-7\t1.928096E-7\t3.082945E-7\t4.880516E-7\t7.649426E-7\t1.187012E-6\t1.823661E-6\t2.773936E-6\t4.177454E-6\t6.228593E-6\t9.194568E-6\t1.343803E-5\t1.944478E-5\t2.785695E-5\t3.951183E-5\t5.548603E-5\t7.714420E-5\t1.061906E-4\t1.447210E-4\t1.952722E-4\t2.608628E-4\t3.450221E-4\t4.517985E-4\t5.857411E-4\t7.518473E-4\t9.554690E-4\t1.202172E-3\t1.497544E-3\t1.846953E-3\t2.255251E-3\t2.726448E-3\t3.263340E-3\t3.867147E-3\t4.537138E-3\t5.270312E-3\t6.061132E-3\t6.901352E-3\t7.779966E-3\t8.683288E-3\t9.595195E-3\t1.049751E-2\t1.137057E-2\t1.219385E-2\t1.294680E-2\t1.360966E-2\t1.416430E-2\t1.459506E-2\t1.488949E-2\t1.503893E-2\t1.503893E-2\t1.488949E-2\t1.459506E-2\t1.416430E-2\t1.360966E-2\t1.294680E-2\t1.219385E-2\t1.137057E-2\t1.049751E-2\t9.595195E-3\t8.683288E-3\t7.779966E-3\t6.901352E-3\t6.061132E-3\t5.270312E-3\t4.537138E-3\t3.867147E-3\t3.263340E-3\t2.726448E-3\t2.255251E-3\t1.846953E-3\t1.497544E-3\t1.202172E-3\t9.554690E-4\t7.518473E-4\t5.857411E-4\t4.517985E-4\t3.450221E-4\t2.608628E-4\t1.952722E-4\t1.447210E-4\t1.061906E-4\t7.714420E-5\t5.548603E-5\t3.951183E-5\t2.785695E-5\t1.944478E-5\t1.343803E-5\t9.194568E-6\t6.228593E-6\t4.177454E-6\t2.773936E-6\t1.823661E-6\t1.187012E-6\t7.649426E-7\t4.880516E-7\t3.082945E-7\t1.928096E-7\t1.193864E-7\t7.318867E-8\r\n-6.156660E-1\t9.505165E-8\t1.550496E-7\t2.504059E-7\t4.003885E-7\t6.338429E-7\t9.934470E-7\t1.541597E-6\t2.368427E-6\t3.602568E-6\t5.425347E-6\t8.089204E-6\t1.194118E-5\t1.745225E-5\t2.525335E-5\t3.617841E-5\t5.131484E-5\t7.206087E-5\t1.001888E-4\t1.379119E-4\t1.879522E-4\t2.536040E-4\t3.387879E-4\t4.480874E-4\t5.867601E-4\t7.607142E-4\t9.764397E-4\t1.240888E-3\t1.561286E-3\t1.944892E-3\t2.398676E-3\t2.928942E-3\t3.540894E-3\t4.238168E-3\t5.022344E-3\t5.892476E-3\t6.844665E-3\t7.871719E-3\t8.962930E-3\t1.010400E-2\t1.127717E-2\t1.246148E-2\t1.363334E-2\t1.476719E-2\t1.583641E-2\t1.681428E-2\t1.767515E-2\t1.839547E-2\t1.895492E-2\t1.933730E-2\t1.953137E-2\t1.953137E-2\t1.933730E-2\t1.895492E-2\t1.839547E-2\t1.767515E-2\t1.681428E-2\t1.583641E-2\t1.476719E-2\t1.363334E-2\t1.246148E-2\t1.127717E-2\t1.010400E-2\t8.962930E-3\t7.871719E-3\t6.844665E-3\t5.892476E-3\t5.022344E-3\t4.238168E-3\t3.540894E-3\t2.928942E-3\t2.398676E-3\t1.944892E-3\t1.561286E-3\t1.240888E-3\t9.764397E-4\t7.607142E-4\t5.867601E-4\t4.480874E-4\t3.387879E-4\t2.536040E-4\t1.879522E-4\t1.379119E-4\t1.001888E-4\t7.206087E-5\t5.131484E-5\t3.617841E-5\t2.525335E-5\t1.745225E-5\t1.194118E-5\t8.089204E-6\t5.425347E-6\t3.602568E-6\t2.368427E-6\t1.541597E-6\t9.934470E-7\t6.338429E-7\t4.003885E-7\t2.504059E-7\t1.550496E-7\t9.505165E-8\r\n-5.707082E-1\t1.222114E-7\t1.993529E-7\t3.219559E-7\t5.147940E-7\t8.149547E-7\t1.277311E-6\t1.982087E-6\t3.045172E-6\t4.631953E-6\t6.975565E-6\t1.040058E-5\t1.535320E-5\t2.243900E-5\t3.246914E-5\t4.651589E-5\t6.597734E-5\t9.265127E-5\t1.288164E-4\t1.773183E-4\t2.416570E-4\t3.260679E-4\t4.355919E-4\t5.761222E-4\t7.544188E-4\t9.780778E-4\t1.255444E-3\t1.595454E-3\t2.007402E-3\t2.500618E-3\t3.084065E-3\t3.765847E-3\t4.552656E-3\t5.449167E-3\t6.457410E-3\t7.576170E-3\t8.800433E-3\t1.012095E-2\t1.152396E-2\t1.299108E-2\t1.449946E-2\t1.602218E-2\t1.752888E-2\t1.898671E-2\t2.036144E-2\t2.161873E-2\t2.272558E-2\t2.365173E-2\t2.437102E-2\t2.486266E-2\t2.511219E-2\t2.511219E-2\t2.486266E-2\t2.437102E-2\t2.365173E-2\t2.272558E-2\t2.161873E-2\t2.036144E-2\t1.898671E-2\t1.752888E-2\t1.602218E-2\t1.449946E-2\t1.299108E-2\t1.152396E-2\t1.012095E-2\t8.800433E-3\t7.576170E-3\t6.457410E-3\t5.449167E-3\t4.552656E-3\t3.765847E-3\t3.084065E-3\t2.500618E-3\t2.007402E-3\t1.595454E-3\t1.255444E-3\t9.780778E-4\t7.544188E-4\t5.761222E-4\t4.355919E-4\t3.260679E-4\t2.416570E-4\t1.773183E-4\t1.288164E-4\t9.265127E-5\t6.597734E-5\t4.651589E-5\t3.246914E-5\t2.243900E-5\t1.535320E-5\t1.040058E-5\t6.975565E-6\t4.631953E-6\t3.045172E-6\t1.982087E-6\t1.277311E-6\t8.149547E-7\t5.147940E-7\t3.219559E-7\t1.993529E-7\t1.222114E-7\r\n-5.257505E-1\t1.555606E-7\t2.537526E-7\t4.098117E-7\t6.552717E-7\t1.037341E-6\t1.625865E-6\t2.522962E-6\t3.876144E-6\t5.895927E-6\t8.879067E-6\t1.323871E-5\t1.954281E-5\t2.856218E-5\t4.132937E-5\t5.920921E-5\t8.398134E-5\t1.179341E-4\t1.639679E-4\t2.257052E-4\t3.076007E-4\t4.150458E-4\t5.544569E-4\t7.333353E-4\t9.602857E-4\t1.244977E-3\t1.598031E-3\t2.030824E-3\t2.555185E-3\t3.182991E-3\t3.925649E-3\t4.793477E-3\t5.794992E-3\t6.936143E-3\t8.219518E-3\t9.643566E-3\t1.120191E-2\t1.288278E-2\t1.466864E-2\t1.653611E-2\t1.845610E-2\t2.039433E-2\t2.231218E-2\t2.416784E-2\t2.591770E-2\t2.751808E-2\t2.892697E-2\t3.010585E-2\t3.102142E-2\t3.164722E-2\t3.196484E-2\t3.196484E-2\t3.164722E-2\t3.102142E-2\t3.010585E-2\t2.892697E-2\t2.751808E-2\t2.591770E-2\t2.416784E-2\t2.231218E-2\t2.039433E-2\t1.845610E-2\t1.653611E-2\t1.466864E-2\t1.288278E-2\t1.120191E-2\t9.643566E-3\t8.219518E-3\t6.936143E-3\t5.794992E-3\t4.793477E-3\t3.925649E-3\t3.182991E-3\t2.555185E-3\t2.030824E-3\t1.598031E-3\t1.244977E-3\t9.602857E-4\t7.333353E-4\t5.544569E-4\t4.150458E-4\t3.076007E-4\t2.257052E-4\t1.639679E-4\t1.179341E-4\t8.398134E-5\t5.920921E-5\t4.132937E-5\t2.856218E-5\t1.954281E-5\t1.323871E-5\t8.879067E-6\t5.895927E-6\t3.876144E-6\t2.522962E-6\t1.625865E-6\t1.037341E-6\t6.552717E-7\t4.098117E-7\t2.537526E-7\t1.555606E-7\r\n-4.807927E-1\t1.960305E-7\t3.197676E-7\t5.164264E-7\t8.257440E-7\t1.307210E-6\t2.048843E-6\t3.179323E-6\t4.884542E-6\t7.429783E-6\t1.118900E-5\t1.668283E-5\t2.462697E-5\t3.599278E-5\t5.208142E-5\t7.461280E-5\t1.058295E-4\t1.486153E-4\t2.066251E-4\t2.844236E-4\t3.876246E-4\t5.230221E-4\t6.987017E-4\t9.241163E-4\t1.210109E-3\t1.568864E-3\t2.013767E-3\t2.559153E-3\t3.219929E-3\t4.011062E-3\t4.946927E-3\t6.040525E-3\t7.302589E-3\t8.740617E-3\t1.035787E-2\t1.215239E-2\t1.411614E-2\t1.623430E-2\t1.848476E-2\t2.083807E-2\t2.325755E-2\t2.570002E-2\t2.811682E-2\t3.045522E-2\t3.266032E-2\t3.467706E-2\t3.645248E-2\t3.793804E-2\t3.909181E-2\t3.988041E-2\t4.028066E-2\t4.028066E-2\t3.988041E-2\t3.909181E-2\t3.793804E-2\t3.645248E-2\t3.467706E-2\t3.266032E-2\t3.045522E-2\t2.811682E-2\t2.570002E-2\t2.325755E-2\t2.083807E-2\t1.848476E-2\t1.623430E-2\t1.411614E-2\t1.215239E-2\t1.035787E-2\t8.740617E-3\t7.302589E-3\t6.040525E-3\t4.946927E-3\t4.011062E-3\t3.219929E-3\t2.559153E-3\t2.013767E-3\t1.568864E-3\t1.210109E-3\t9.241163E-4\t6.987017E-4\t5.230221E-4\t3.876246E-4\t2.844236E-4\t2.066251E-4\t1.486153E-4\t1.058295E-4\t7.461280E-5\t5.208142E-5\t3.599278E-5\t2.462697E-5\t1.668283E-5\t1.118900E-5\t7.429783E-6\t4.884542E-6\t3.179323E-6\t2.048843E-6\t1.307210E-6\t8.257440E-7\t5.164264E-7\t3.197676E-7\t1.960305E-7\r\n-4.358349E-1\t2.445590E-7\t3.989280E-7\t6.442709E-7\t1.030162E-6\t1.630818E-6\t2.556046E-6\t3.966385E-6\t6.093741E-6\t9.269071E-6\t1.395891E-5\t2.081276E-5\t3.072353E-5\t4.490302E-5\t6.497450E-5\t9.308365E-5\t1.320283E-4\t1.854059E-4\t2.577764E-4\t3.548344E-4\t4.835834E-4\t6.524995E-4\t8.716696E-4\t1.152887E-3\t1.509679E-3\t1.957246E-3\t2.512288E-3\t3.192688E-3\t4.017043E-3\t5.004025E-3\t6.171569E-3\t7.535894E-3\t9.110390E-3\t1.090441E-2\t1.292202E-2\t1.516079E-2\t1.761068E-2\t2.025320E-2\t2.306078E-2\t2.599666E-2\t2.901510E-2\t3.206222E-2\t3.507731E-2\t3.799460E-2\t4.074559E-2\t4.326158E-2\t4.547651E-2\t4.732983E-2\t4.876922E-2\t4.975306E-2\t5.025239E-2\t5.025239E-2\t4.975306E-2\t4.876922E-2\t4.732983E-2\t4.547651E-2\t4.326158E-2\t4.074559E-2\t3.799460E-2\t3.507731E-2\t3.206222E-2\t2.901510E-2\t2.599666E-2\t2.306078E-2\t2.025320E-2\t1.761068E-2\t1.516079E-2\t1.292202E-2\t1.090441E-2\t9.110390E-3\t7.535894E-3\t6.171569E-3\t5.004025E-3\t4.017043E-3\t3.192688E-3\t2.512288E-3\t1.957246E-3\t1.509679E-3\t1.152887E-3\t8.716696E-4\t6.524995E-4\t4.835834E-4\t3.548344E-4\t2.577764E-4\t1.854059E-4\t1.320283E-4\t9.308365E-5\t6.497450E-5\t4.490302E-5\t3.072353E-5\t2.081276E-5\t1.395891E-5\t9.269071E-6\t6.093741E-6\t3.966385E-6\t2.556046E-6\t1.630818E-6\t1.030162E-6\t6.442709E-7\t3.989280E-7\t2.445590E-7\r\n-3.908772E-1\t3.020507E-7\t4.927093E-7\t7.957281E-7\t1.272336E-6\t2.014196E-6\t3.156929E-6\t4.898815E-6\t7.526277E-6\t1.144807E-5\t1.724041E-5\t2.570549E-5\t3.794611E-5\t5.545896E-5\t8.024891E-5\t1.149660E-4\t1.630659E-4\t2.289917E-4\t3.183752E-4\t4.382500E-4\t5.972657E-4\t8.058910E-4\t1.076584E-3\t1.423911E-3\t1.864579E-3\t2.417362E-3\t3.102884E-3\t3.943234E-3\t4.961381E-3\t6.180387E-3\t7.622401E-3\t9.307455E-3\t1.125209E-2\t1.346785E-2\t1.595977E-2\t1.872483E-2\t2.175066E-2\t2.501438E-2\t2.848198E-2\t3.210803E-2\t3.583606E-2\t3.959951E-2\t4.332339E-2\t4.692649E-2\t5.032419E-2\t5.343164E-2\t5.616727E-2\t5.845628E-2\t6.023404E-2\t6.144916E-2\t6.206588E-2\t6.206588E-2\t6.144916E-2\t6.023404E-2\t5.845628E-2\t5.616727E-2\t5.343164E-2\t5.032419E-2\t4.692649E-2\t4.332339E-2\t3.959951E-2\t3.583606E-2\t3.210803E-2\t2.848198E-2\t2.501438E-2\t2.175066E-2\t1.872483E-2\t1.595977E-2\t1.346785E-2\t1.125209E-2\t9.307455E-3\t7.622401E-3\t6.180387E-3\t4.961381E-3\t3.943234E-3\t3.102884E-3\t2.417362E-3\t1.864579E-3\t1.423911E-3\t1.076584E-3\t8.058910E-4\t5.972657E-4\t4.382500E-4\t3.183752E-4\t2.289917E-4\t1.630659E-4\t1.149660E-4\t8.024891E-5\t5.545896E-5\t3.794611E-5\t2.570549E-5\t1.724041E-5\t1.144807E-5\t7.526277E-6\t4.898815E-6\t3.156929E-6\t2.014196E-6\t1.272336E-6\t7.957281E-7\t4.927093E-7\t3.020507E-7\r\n-3.459194E-1\t3.693279E-7\t6.024528E-7\t9.729644E-7\t1.555729E-6\t2.462828E-6\t3.860087E-6\t5.989951E-6\t9.202640E-6\t1.399796E-5\t2.108045E-5\t3.143100E-5\t4.639803E-5\t6.781159E-5\t9.812313E-5\t1.405730E-4\t1.993863E-4\t2.799961E-4\t3.892885E-4\t5.358635E-4\t7.302976E-4\t9.853910E-4\t1.316377E-3\t1.741066E-3\t2.279885E-3\t2.955792E-3\t3.794005E-3\t4.821530E-3\t6.066453E-3\t7.556974E-3\t9.320174E-3\t1.138055E-2\t1.375832E-2\t1.646761E-2\t1.951457E-2\t2.289551E-2\t2.659528E-2\t3.058595E-2\t3.482591E-2\t3.925961E-2\t4.381799E-2\t4.841969E-2\t5.297301E-2\t5.737865E-2\t6.153313E-2\t6.533273E-2\t6.867767E-2\t7.147652E-2\t7.365026E-2\t7.513602E-2\t7.589010E-2\t7.589010E-2\t7.513602E-2\t7.365026E-2\t7.147652E-2\t6.867767E-2\t6.533273E-2\t6.153313E-2\t5.737865E-2\t5.297301E-2\t4.841969E-2\t4.381799E-2\t3.925961E-2\t3.482591E-2\t3.058595E-2\t2.659528E-2\t2.289551E-2\t1.951457E-2\t1.646761E-2\t1.375832E-2\t1.138055E-2\t9.320174E-3\t7.556974E-3\t6.066453E-3\t4.821530E-3\t3.794005E-3\t2.955792E-3\t2.279885E-3\t1.741066E-3\t1.316377E-3\t9.853910E-4\t7.302976E-4\t5.358635E-4\t3.892885E-4\t2.799961E-4\t1.993863E-4\t1.405730E-4\t9.812313E-5\t6.781159E-5\t4.639803E-5\t3.143100E-5\t2.108045E-5\t1.399796E-5\t9.202640E-6\t5.989951E-6\t3.860087E-6\t2.462828E-6\t1.555729E-6\t9.729644E-7\t6.024528E-7\t3.693279E-7\r\n-3.009616E-1\t4.470750E-7\t7.292750E-7\t1.177783E-6\t1.883225E-6\t2.981277E-6\t4.672673E-6\t7.250894E-6\t1.113989E-5\t1.694466E-5\t2.551809E-5\t3.804754E-5\t5.616527E-5\t8.208660E-5\t1.187790E-4\t1.701650E-4\t2.413591E-4\t3.389380E-4\t4.712375E-4\t6.486680E-4\t8.840324E-4\t1.192825E-3\t1.593488E-3\t2.107577E-3\t2.759824E-3\t3.578016E-3\t4.592680E-3\t5.836509E-3\t7.343501E-3\t9.147791E-3\t1.128216E-2\t1.377627E-2\t1.665458E-2\t1.993421E-2\t2.362257E-2\t2.771523E-2\t3.219385E-2\t3.702460E-2\t4.215710E-2\t4.752414E-2\t5.304211E-2\t5.861252E-2\t6.412435E-2\t6.945742E-2\t7.448646E-2\t7.908591E-2\t8.313500E-2\t8.652303E-2\t8.915436E-2\t9.095289E-2\t9.186572E-2\t9.186572E-2\t9.095289E-2\t8.915436E-2\t8.652303E-2\t8.313500E-2\t7.908591E-2\t7.448646E-2\t6.945742E-2\t6.412435E-2\t5.861252E-2\t5.304211E-2\t4.752414E-2\t4.215710E-2\t3.702460E-2\t3.219385E-2\t2.771523E-2\t2.362257E-2\t1.993421E-2\t1.665458E-2\t1.377627E-2\t1.128216E-2\t9.147791E-3\t7.343501E-3\t5.836509E-3\t4.592680E-3\t3.578016E-3\t2.759824E-3\t2.107577E-3\t1.593488E-3\t1.192825E-3\t8.840324E-4\t6.486680E-4\t4.712375E-4\t3.389380E-4\t2.413591E-4\t1.701650E-4\t1.187790E-4\t8.208660E-5\t5.616527E-5\t3.804754E-5\t2.551809E-5\t1.694466E-5\t1.113989E-5\t7.250894E-6\t4.672673E-6\t2.981277E-6\t1.883225E-6\t1.177783E-6\t7.292750E-7\t4.470750E-7\r\n-2.560039E-1\t5.357779E-7\t8.739684E-7\t1.411464E-6\t2.256871E-6\t3.572784E-6\t5.599765E-6\t8.689523E-6\t1.335012E-5\t2.030661E-5\t3.058107E-5\t4.559644E-5\t6.730887E-5\t9.837317E-5\t1.423456E-4\t2.039269E-4\t2.892465E-4\t4.061857E-4\t5.647344E-4\t7.773684E-4\t1.059431E-3\t1.429491E-3\t1.909647E-3\t2.525736E-3\t3.307392E-3\t4.287920E-3\t5.503900E-3\t6.994514E-3\t8.800505E-3\t1.096278E-2\t1.352062E-2\t1.650958E-2\t1.995897E-2\t2.388930E-2\t2.830946E-2\t3.321413E-2\t3.858134E-2\t4.437054E-2\t5.052138E-2\t5.695327E-2\t6.356604E-2\t7.024166E-2\t7.684708E-2\t8.323827E-2\t8.926511E-2\t9.477712E-2\t9.962958E-2\t1.036898E-1\t1.068432E-1\t1.089986E-1\t1.100925E-1\t1.100925E-1\t1.089986E-1\t1.068432E-1\t1.036898E-1\t9.962958E-2\t9.477712E-2\t8.926511E-2\t8.323827E-2\t7.684708E-2\t7.024166E-2\t6.356604E-2\t5.695327E-2\t5.052138E-2\t4.437054E-2\t3.858134E-2\t3.321413E-2\t2.830946E-2\t2.388930E-2\t1.995897E-2\t1.650958E-2\t1.352062E-2\t1.096278E-2\t8.800505E-3\t6.994514E-3\t5.503900E-3\t4.287920E-3\t3.307392E-3\t2.525736E-3\t1.909647E-3\t1.429491E-3\t1.059431E-3\t7.773684E-4\t5.647344E-4\t4.061857E-4\t2.892465E-4\t2.039269E-4\t1.423456E-4\t9.837317E-5\t6.730887E-5\t4.559644E-5\t3.058107E-5\t2.030661E-5\t1.335012E-5\t8.689523E-6\t5.599765E-6\t3.572784E-6\t2.256871E-6\t1.411464E-6\t8.739684E-7\t5.357779E-7\r\n-2.110461E-1\t6.356605E-7\t1.036898E-6\t1.674596E-6\t2.677609E-6\t4.238842E-6\t6.643704E-6\t1.030947E-5\t1.583892E-5\t2.409228E-5\t3.628216E-5\t5.409678E-5\t7.985695E-5\t1.167124E-4\t1.688825E-4\t2.419441E-4\t3.431694E-4\t4.819091E-4\t6.700153E-4\t9.222897E-4\t1.256936E-3\t1.695984E-3\t2.265654E-3\t2.996597E-3\t3.923975E-3\t5.087297E-3\t6.529968E-3\t8.298470E-3\t1.044114E-2\t1.300652E-2\t1.604121E-2\t1.958738E-2\t2.367983E-2\t2.834287E-2\t3.358707E-2\t3.940610E-2\t4.577388E-2\t5.264234E-2\t5.993985E-2\t6.757081E-2\t7.541637E-2\t8.333649E-2\t9.117334E-2\t9.875600E-2\t1.059064E-1\t1.124460E-1\t1.182031E-1\t1.230202E-1\t1.267615E-1\t1.293187E-1\t1.306166E-1\t1.306166E-1\t1.293187E-1\t1.267615E-1\t1.230202E-1\t1.182031E-1\t1.124460E-1\t1.059064E-1\t9.875600E-2\t9.117334E-2\t8.333649E-2\t7.541637E-2\t6.757081E-2\t5.993985E-2\t5.264234E-2\t4.577388E-2\t3.940610E-2\t3.358707E-2\t2.834287E-2\t2.367983E-2\t1.958738E-2\t1.604121E-2\t1.300652E-2\t1.044114E-2\t8.298470E-3\t6.529968E-3\t5.087297E-3\t3.923975E-3\t2.996597E-3\t2.265654E-3\t1.695984E-3\t1.256936E-3\t9.222897E-4\t6.700153E-4\t4.819091E-4\t3.431694E-4\t2.419441E-4\t1.688825E-4\t1.167124E-4\t7.985695E-5\t5.409678E-5\t3.628216E-5\t2.409228E-5\t1.583892E-5\t1.030947E-5\t6.643704E-6\t4.238842E-6\t2.677609E-6\t1.674596E-6\t1.036898E-6\t6.356605E-7\r\n-1.660883E-1\t7.466237E-7\t1.217903E-6\t1.966920E-6\t3.145022E-6\t4.978789E-6\t7.803453E-6\t1.210913E-5\t1.860382E-5\t2.829791E-5\t4.261570E-5\t6.354010E-5\t9.379707E-5\t1.370862E-4\t1.983632E-4\t2.841787E-4\t4.030743E-4\t5.660329E-4\t7.869756E-4\t1.083288E-3\t1.476351E-3\t1.992041E-3\t2.661154E-3\t3.519694E-3\t4.608958E-3\t5.975354E-3\t7.669862E-3\t9.747081E-3\t1.226379E-2\t1.527698E-2\t1.884143E-2\t2.300662E-2\t2.781347E-2\t3.329050E-2\t3.945015E-2\t4.628497E-2\t5.376434E-2\t6.183178E-2\t7.040316E-2\t7.936621E-2\t8.858133E-2\t9.788401E-2\t1.070889E-1\t1.159952E-1\t1.243938E-1\t1.320750E-1\t1.388370E-1\t1.444951E-1\t1.488895E-1\t1.518930E-1\t1.534175E-1\t1.534175E-1\t1.518930E-1\t1.488895E-1\t1.444951E-1\t1.388370E-1\t1.320750E-1\t1.243938E-1\t1.159952E-1\t1.070889E-1\t9.788401E-2\t8.858133E-2\t7.936621E-2\t7.040316E-2\t6.183178E-2\t5.376434E-2\t4.628497E-2\t3.945015E-2\t3.329050E-2\t2.781347E-2\t2.300662E-2\t1.884143E-2\t1.527698E-2\t1.226379E-2\t9.747081E-3\t7.669862E-3\t5.975354E-3\t4.608958E-3\t3.519694E-3\t2.661154E-3\t1.992041E-3\t1.476351E-3\t1.083288E-3\t7.869756E-4\t5.660329E-4\t4.030743E-4\t2.841787E-4\t1.983632E-4\t1.370862E-4\t9.379707E-5\t6.354010E-5\t4.261570E-5\t2.829791E-5\t1.860382E-5\t1.210913E-5\t7.803453E-6\t4.978789E-6\t3.145022E-6\t1.966920E-6\t1.217903E-6\t7.466237E-7\r\n-1.211306E-1\t8.681892E-7\t1.416202E-6\t2.287174E-6\t3.657095E-6\t5.789437E-6\t9.074014E-6\t1.408074E-5\t2.163290E-5\t3.290538E-5\t4.955440E-5\t7.388572E-5\t1.090691E-4\t1.594066E-4\t2.306608E-4\t3.304488E-4\t4.687030E-4\t6.581945E-4\t9.151112E-4\t1.259669E-3\t1.716731E-3\t2.316386E-3\t3.094444E-3\t4.092771E-3\t5.359390E-3\t6.948263E-3\t8.918672E-3\t1.133410E-2\t1.426058E-2\t1.776439E-2\t2.190919E-2\t2.675257E-2\t3.234206E-2\t3.871087E-2\t4.587343E-2\t5.382110E-2\t6.251827E-2\t7.189924E-2\t8.186623E-2\t9.228864E-2\t1.030042E-1\t1.138215E-1\t1.245251E-1\t1.348816E-1\t1.446476E-1\t1.535794E-1\t1.614425E-1\t1.680218E-1\t1.731317E-1\t1.766243E-1\t1.783970E-1\t1.783970E-1\t1.766243E-1\t1.731317E-1\t1.680218E-1\t1.614425E-1\t1.535794E-1\t1.446476E-1\t1.348816E-1\t1.245251E-1\t1.138215E-1\t1.030042E-1\t9.228864E-2\t8.186623E-2\t7.189924E-2\t6.251827E-2\t5.382110E-2\t4.587343E-2\t3.871087E-2\t3.234206E-2\t2.675257E-2\t2.190919E-2\t1.776439E-2\t1.426058E-2\t1.133410E-2\t8.918672E-3\t6.948263E-3\t5.359390E-3\t4.092771E-3\t3.094444E-3\t2.316386E-3\t1.716731E-3\t1.259669E-3\t9.151112E-4\t6.581945E-4\t4.687030E-4\t3.304488E-4\t2.306608E-4\t1.594066E-4\t1.090691E-4\t7.388572E-5\t4.955440E-5\t3.290538E-5\t2.163290E-5\t1.408074E-5\t9.074014E-6\t5.789437E-6\t3.657095E-6\t2.287174E-6\t1.416202E-6\t8.681892E-7\r\n-7.617280E-2\t9.994546E-7\t1.630324E-6\t2.632982E-6\t4.210028E-6\t6.664768E-6\t1.044595E-5\t1.620967E-5\t2.490367E-5\t3.788050E-5\t5.704675E-5\t8.505683E-5\t1.255598E-4\t1.835080E-4\t2.655354E-4\t3.804108E-4\t5.395682E-4\t7.577098E-4\t1.053471E-3\t1.450124E-3\t1.976291E-3\t2.666611E-3\t3.562307E-3\t4.711576E-3\t6.169700E-3\t7.998802E-3\t1.026713E-2\t1.304776E-2\t1.641670E-2\t2.045027E-2\t2.522174E-2\t3.079741E-2\t3.723200E-2\t4.456374E-2\t5.280924E-2\t6.195855E-2\t7.197068E-2\t8.277001E-2\t9.424394E-2\t1.062422E-1\t1.185778E-1\t1.310307E-1\t1.433526E-1\t1.552749E-1\t1.665176E-1\t1.767998E-1\t1.858517E-1\t1.934258E-1\t1.993083E-1\t2.033289E-1\t2.053696E-1\t2.053696E-1\t2.033289E-1\t1.993083E-1\t1.934258E-1\t1.858517E-1\t1.767998E-1\t1.665176E-1\t1.552749E-1\t1.433526E-1\t1.310307E-1\t1.185778E-1\t1.062422E-1\t9.424394E-2\t8.277001E-2\t7.197068E-2\t6.195855E-2\t5.280924E-2\t4.456374E-2\t3.723200E-2\t3.079741E-2\t2.522174E-2\t2.045027E-2\t1.641670E-2\t1.304776E-2\t1.026713E-2\t7.998802E-3\t6.169700E-3\t4.711576E-3\t3.562307E-3\t2.666611E-3\t1.976291E-3\t1.450124E-3\t1.053471E-3\t7.577098E-4\t5.395682E-4\t3.804108E-4\t2.655354E-4\t1.835080E-4\t1.255598E-4\t8.505683E-5\t5.704675E-5\t3.788050E-5\t2.490367E-5\t1.620967E-5\t1.044595E-5\t6.664768E-6\t4.210028E-6\t2.632982E-6\t1.630324E-6\t9.994546E-7\r\n-3.121503E-2\t1.139063E-6\t1.858056E-6\t3.000770E-6\t4.798105E-6\t7.595735E-6\t1.190510E-5\t1.847392E-5\t2.838234E-5\t4.317182E-5\t6.501531E-5\t9.693798E-5\t1.430986E-4\t2.091413E-4\t3.026266E-4\t4.335484E-4\t6.149377E-4\t8.635504E-4\t1.200625E-3\t1.652684E-3\t2.252349E-3\t3.039095E-3\t4.059907E-3\t5.369711E-3\t7.031513E-3\t9.116113E-3\t1.170129E-2\t1.487033E-2\t1.870986E-2\t2.330686E-2\t2.874483E-2\t3.509934E-2\t4.243275E-2\t5.078862E-2\t6.018589E-2\t7.061322E-2\t8.202389E-2\t9.433172E-2\t1.074084E-1\t1.210826E-1\t1.351413E-1\t1.493337E-1\t1.633768E-1\t1.769645E-1\t1.897775E-1\t2.014961E-1\t2.118124E-1\t2.204444E-1\t2.271486E-1\t2.317309E-1\t2.340566E-1\t2.340566E-1\t2.317309E-1\t2.271486E-1\t2.204444E-1\t2.118124E-1\t2.014961E-1\t1.897775E-1\t1.769645E-1\t1.633768E-1\t1.493337E-1\t1.351413E-1\t1.210826E-1\t1.074084E-1\t9.433172E-2\t8.202389E-2\t7.061322E-2\t6.018589E-2\t5.078862E-2\t4.243275E-2\t3.509934E-2\t2.874483E-2\t2.330686E-2\t1.870986E-2\t1.487033E-2\t1.170129E-2\t9.116113E-3\t7.031513E-3\t5.369711E-3\t4.059907E-3\t3.039095E-3\t2.252349E-3\t1.652684E-3\t1.200625E-3\t8.635504E-4\t6.149377E-4\t4.335484E-4\t3.026266E-4\t2.091413E-4\t1.430986E-4\t9.693798E-5\t6.501531E-5\t4.317182E-5\t2.838234E-5\t1.847392E-5\t1.190510E-5\t7.595735E-6\t4.798105E-6\t3.000770E-6\t1.858056E-6\t1.139063E-6\r\n1.374274E-2\t1.285194E-6\t2.096426E-6\t3.385740E-6\t5.413655E-6\t8.570193E-6\t1.343240E-5\t2.084394E-5\t3.202352E-5\t4.871035E-5\t7.335614E-5\t1.093742E-4\t1.614567E-4\t2.359720E-4\t3.414507E-4\t4.891684E-4\t6.938282E-4\t9.743355E-4\t1.354653E-3\t1.864708E-3\t2.541303E-3\t3.428982E-3\t4.580754E-3\t6.058593E-3\t7.933587E-3\t1.028562E-2\t1.320245E-2\t1.677805E-2\t2.111016E-2\t2.629690E-2\t3.243252E-2\t3.960224E-2\t4.787645E-2\t5.730430E-2\t6.790715E-2\t7.967220E-2\t9.254675E-2\t1.064336E-1\t1.211878E-1\t1.366163E-1\t1.524787E-1\t1.684917E-1\t1.843365E-1\t1.996673E-1\t2.141241E-1\t2.273460E-1\t2.389858E-1\t2.487253E-1\t2.562895E-1\t2.614597E-1\t2.640838E-1\t2.640838E-1\t2.614597E-1\t2.562895E-1\t2.487253E-1\t2.389858E-1\t2.273460E-1\t2.141241E-1\t1.996673E-1\t1.843365E-1\t1.684917E-1\t1.524787E-1\t1.366163E-1\t1.211878E-1\t1.064336E-1\t9.254675E-2\t7.967220E-2\t6.790715E-2\t5.730430E-2\t4.787645E-2\t3.960224E-2\t3.243252E-2\t2.629690E-2\t2.111016E-2\t1.677805E-2\t1.320245E-2\t1.028562E-2\t7.933587E-3\t6.058593E-3\t4.580754E-3\t3.428982E-3\t2.541303E-3\t1.864708E-3\t1.354653E-3\t9.743355E-4\t6.938282E-4\t4.891684E-4\t3.414507E-4\t2.359720E-4\t1.614567E-4\t1.093742E-4\t7.335614E-5\t4.871035E-5\t3.202352E-5\t2.084394E-5\t1.343240E-5\t8.570193E-6\t5.413655E-6\t3.385740E-6\t2.096426E-6\t1.285194E-6\r\n5.870050E-2\t1.435574E-6\t2.341728E-6\t3.781904E-6\t6.047104E-6\t9.572988E-6\t1.500412E-5\t2.328288E-5\t3.577057E-5\t5.440992E-5\t8.193951E-5\t1.221720E-4\t1.803487E-4\t2.635830E-4\t3.814037E-4\t5.464058E-4\t7.750128E-4\t1.088342E-3\t1.513161E-3\t2.082896E-3\t2.838660E-3\t3.830205E-3\t5.116746E-3\t6.767506E-3\t8.861893E-3\t1.148914E-2\t1.474726E-2\t1.874124E-2\t2.358025E-2\t2.937389E-2\t3.622743E-2\t4.423608E-2\t5.347846E-2\t6.400945E-2\t7.585293E-2\t8.899461E-2\t1.033756E-1\t1.188873E-1\t1.353680E-1\t1.526017E-1\t1.703201E-1\t1.882069E-1\t2.059056E-1\t2.230303E-1\t2.391787E-1\t2.539477E-1\t2.669495E-1\t2.778286E-1\t2.862779E-1\t2.920530E-1\t2.949841E-1\t2.949841E-1\t2.920530E-1\t2.862779E-1\t2.778286E-1\t2.669495E-1\t2.539477E-1\t2.391787E-1\t2.230303E-1\t2.059056E-1\t1.882069E-1\t1.703201E-1\t1.526017E-1\t1.353680E-1\t1.188873E-1\t1.033756E-1\t8.899461E-2\t7.585293E-2\t6.400945E-2\t5.347846E-2\t4.423608E-2\t3.622743E-2\t2.937389E-2\t2.358025E-2\t1.874124E-2\t1.474726E-2\t1.148914E-2\t8.861893E-3\t6.767506E-3\t5.116746E-3\t3.830205E-3\t2.838660E-3\t2.082896E-3\t1.513161E-3\t1.088342E-3\t7.750128E-4\t5.464058E-4\t3.814037E-4\t2.635830E-4\t1.803487E-4\t1.221720E-4\t8.193951E-5\t5.440992E-5\t3.577057E-5\t2.328288E-5\t1.500412E-5\t9.572988E-6\t6.047104E-6\t3.781904E-6\t2.341728E-6\t1.435574E-6\r\n1.036583E-1\t1.587518E-6\t2.589581E-6\t4.182187E-6\t6.687140E-6\t1.058621E-5\t1.659218E-5\t2.574718E-5\t3.955659E-5\t6.016876E-5\t9.061213E-5\t1.351029E-4\t1.994371E-4\t2.914811E-4\t4.217721E-4\t6.042384E-4\t8.570414E-4\t1.203534E-3\t1.673316E-3\t2.303354E-3\t3.139108E-3\t4.235601E-3\t5.658311E-3\t7.483790E-3\t9.799851E-3\t1.270517E-2\t1.630814E-2\t2.072485E-2\t2.607602E-2\t3.248287E-2\t4.006180E-2\t4.891811E-2\t5.913871E-2\t7.078432E-2\t8.388134E-2\t9.841395E-2\t1.143171E-1\t1.314705E-1\t1.496956E-1\t1.687533E-1\t1.883471E-1\t2.081270E-1\t2.276990E-1\t2.466362E-1\t2.644938E-1\t2.808259E-1\t2.952038E-1\t3.072344E-1\t3.165780E-1\t3.229644E-1\t3.262057E-1\t3.262057E-1\t3.229644E-1\t3.165780E-1\t3.072344E-1\t2.952038E-1\t2.808259E-1\t2.644938E-1\t2.466362E-1\t2.276990E-1\t2.081270E-1\t1.883471E-1\t1.687533E-1\t1.496956E-1\t1.314705E-1\t1.143171E-1\t9.841395E-2\t8.388134E-2\t7.078432E-2\t5.913871E-2\t4.891811E-2\t4.006180E-2\t3.248287E-2\t2.607602E-2\t2.072485E-2\t1.630814E-2\t1.270517E-2\t9.799851E-3\t7.483790E-3\t5.658311E-3\t4.235601E-3\t3.139108E-3\t2.303354E-3\t1.673316E-3\t1.203534E-3\t8.570414E-4\t6.042384E-4\t4.217721E-4\t2.914811E-4\t1.994371E-4\t1.351029E-4\t9.061213E-5\t6.016876E-5\t3.955659E-5\t2.574718E-5\t1.659218E-5\t1.058621E-5\t6.687140E-6\t4.182187E-6\t2.589581E-6\t1.587518E-6\r\n1.486160E-1\t1.737991E-6\t2.835035E-6\t4.578597E-6\t7.320984E-6\t1.158963E-5\t1.816488E-5\t2.818764E-5\t4.330598E-5\t6.587189E-5\t9.920085E-5\t1.479087E-4\t2.183409E-4\t3.191093E-4\t4.617500E-4\t6.615114E-4\t9.382765E-4\t1.317612E-3\t1.831922E-3\t2.521678E-3\t3.436650E-3\t4.637075E-3\t6.194637E-3\t8.193145E-3\t1.072873E-2\t1.390943E-2\t1.785391E-2\t2.268926E-2\t2.854765E-2\t3.556177E-2\t4.385908E-2\t5.355484E-2\t6.474420E-2\t7.749365E-2\t9.183208E-2\t1.077422E-1\t1.251527E-1\t1.439320E-1\t1.638845E-1\t1.847487E-1\t2.061997E-1\t2.278545E-1\t2.492816E-1\t2.700137E-1\t2.895640E-1\t3.074442E-1\t3.231849E-1\t3.363558E-1\t3.465850E-1\t3.535767E-1\t3.571253E-1\t3.571253E-1\t3.535767E-1\t3.465850E-1\t3.363558E-1\t3.231849E-1\t3.074442E-1\t2.895640E-1\t2.700137E-1\t2.492816E-1\t2.278545E-1\t2.061997E-1\t1.847487E-1\t1.638845E-1\t1.439320E-1\t1.251527E-1\t1.077422E-1\t9.183208E-2\t7.749365E-2\t6.474420E-2\t5.355484E-2\t4.385908E-2\t3.556177E-2\t2.854765E-2\t2.268926E-2\t1.785391E-2\t1.390943E-2\t1.072873E-2\t8.193145E-3\t6.194637E-3\t4.637075E-3\t3.436650E-3\t2.521678E-3\t1.831922E-3\t1.317612E-3\t9.382765E-4\t6.615114E-4\t4.617500E-4\t3.191093E-4\t2.183409E-4\t1.479087E-4\t9.920085E-5\t6.587189E-5\t4.330598E-5\t2.818764E-5\t1.816488E-5\t1.158963E-5\t7.320984E-6\t4.578597E-6\t2.835035E-6\t1.737991E-6\r\n1.935738E-1\t1.883704E-6\t3.072724E-6\t4.962466E-6\t7.934774E-6\t1.256130E-5\t1.968782E-5\t3.055089E-5\t4.693675E-5\t7.139458E-5\t1.075178E-4\t1.603093E-4\t2.366465E-4\t3.458634E-4\t5.004630E-4\t7.169724E-4\t1.016941E-3\t1.428080E-3\t1.985510E-3\t2.733095E-3\t3.724779E-3\t5.025846E-3\t6.713994E-3\t8.880057E-3\t1.162823E-2\t1.507560E-2\t1.935078E-2\t2.459152E-2\t3.094108E-2\t3.854327E-2\t4.753622E-2\t5.804486E-2\t7.017235E-2\t8.399071E-2\t9.953126E-2\t1.167753E-1\t1.356454E-1\t1.559993E-1\t1.776246E-1\t2.002380E-1\t2.234874E-1\t2.469577E-1\t2.701813E-1\t2.926516E-1\t3.138410E-1\t3.332202E-1\t3.502807E-1\t3.645558E-1\t3.756426E-1\t3.832205E-1\t3.870666E-1\t3.870666E-1\t3.832205E-1\t3.756426E-1\t3.645558E-1\t3.502807E-1\t3.332202E-1\t3.138410E-1\t2.926516E-1\t2.701813E-1\t2.469577E-1\t2.234874E-1\t2.002380E-1\t1.776246E-1\t1.559993E-1\t1.356454E-1\t1.167753E-1\t9.953126E-2\t8.399071E-2\t7.017235E-2\t5.804486E-2\t4.753622E-2\t3.854327E-2\t3.094108E-2\t2.459152E-2\t1.935078E-2\t1.507560E-2\t1.162823E-2\t8.880057E-3\t6.713994E-3\t5.025846E-3\t3.724779E-3\t2.733095E-3\t1.985510E-3\t1.428080E-3\t1.016941E-3\t7.169724E-4\t5.004630E-4\t3.458634E-4\t2.366465E-4\t1.603093E-4\t1.075178E-4\t7.139458E-5\t4.693675E-5\t3.055089E-5\t1.968782E-5\t1.256130E-5\t7.934774E-6\t4.962466E-6\t3.072724E-6\t1.883704E-6\r\n2.385316E-1\t2.021221E-6\t3.297044E-6\t5.324744E-6\t8.514041E-6\t1.347832E-5\t2.112511E-5\t3.278121E-5\t5.036330E-5\t7.660664E-5\t1.153670E-4\t1.720125E-4\t2.539226E-4\t3.711126E-4\t5.369986E-4\t7.693140E-4\t1.091182E-3\t1.532335E-3\t2.130460E-3\t2.932621E-3\t3.996701E-3\t5.392751E-3\t7.204140E-3\t9.528334E-3\t1.247713E-2\t1.617617E-2\t2.076346E-2\t2.638679E-2\t3.319989E-2\t4.135707E-2\t5.100654E-2\t6.228235E-2\t7.529518E-2\t9.012233E-2\t1.067974E-1\t1.253003E-1\t1.455480E-1\t1.673878E-1\t1.905918E-1\t2.148561E-1\t2.398028E-1\t2.649866E-1\t2.899055E-1\t3.140162E-1\t3.367525E-1\t3.575465E-1\t3.758524E-1\t3.911697E-1\t4.030659E-1\t4.111970E-1\t4.153239E-1\t4.153239E-1\t4.111970E-1\t4.030659E-1\t3.911697E-1\t3.758524E-1\t3.575465E-1\t3.367525E-1\t3.140162E-1\t2.899055E-1\t2.649866E-1\t2.398028E-1\t2.148561E-1\t1.905918E-1\t1.673878E-1\t1.455480E-1\t1.253003E-1\t1.067974E-1\t9.012233E-2\t7.529518E-2\t6.228235E-2\t5.100654E-2\t4.135707E-2\t3.319989E-2\t2.638679E-2\t2.076346E-2\t1.617617E-2\t1.247713E-2\t9.528334E-3\t7.204140E-3\t5.392751E-3\t3.996701E-3\t2.932621E-3\t2.130460E-3\t1.532335E-3\t1.091182E-3\t7.693140E-4\t5.369986E-4\t3.711126E-4\t2.539226E-4\t1.720125E-4\t1.153670E-4\t7.660664E-5\t5.036330E-5\t3.278121E-5\t2.112511E-5\t1.347832E-5\t8.514041E-6\t5.324744E-6\t3.297044E-6\t2.021221E-6\r\n2.834893E-1\t2.147094E-6\t3.502370E-6\t5.656347E-6\t9.044259E-6\t1.431769E-5\t2.244069E-5\t3.482269E-5\t5.349971E-5\t8.137738E-5\t1.225516E-4\t1.827247E-4\t2.697358E-4\t3.942239E-4\t5.704406E-4\t8.172236E-4\t1.159136E-3\t1.627762E-3\t2.263136E-3\t3.115252E-3\t4.245598E-3\t5.728589E-3\t7.652783E-3\t1.012172E-2\t1.325416E-2\t1.718355E-2\t2.205652E-2\t2.803005E-2\t3.526744E-2\t4.393261E-2\t5.418301E-2\t6.616103E-2\t7.998424E-2\t9.573476E-2\t1.134483E-1\t1.331034E-1\t1.546122E-1\t1.778120E-1\t2.024611E-1\t2.282364E-1\t2.547367E-1\t2.814888E-1\t3.079596E-1\t3.335718E-1\t3.577240E-1\t3.798130E-1\t3.992589E-1\t4.155301E-1\t4.281671E-1\t4.368046E-1\t4.411885E-1\t4.411885E-1\t4.368046E-1\t4.281671E-1\t4.155301E-1\t3.992589E-1\t3.798130E-1\t3.577240E-1\t3.335718E-1\t3.079596E-1\t2.814888E-1\t2.547367E-1\t2.282364E-1\t2.024611E-1\t1.778120E-1\t1.546122E-1\t1.331034E-1\t1.134483E-1\t9.573476E-2\t7.998424E-2\t6.616103E-2\t5.418301E-2\t4.393261E-2\t3.526744E-2\t2.803005E-2\t2.205652E-2\t1.718355E-2\t1.325416E-2\t1.012172E-2\t7.652783E-3\t5.728589E-3\t4.245598E-3\t3.115252E-3\t2.263136E-3\t1.627762E-3\t1.159136E-3\t8.172236E-4\t5.704406E-4\t3.942239E-4\t2.697358E-4\t1.827247E-4\t1.225516E-4\t8.137738E-5\t5.349971E-5\t3.482269E-5\t2.244069E-5\t1.431769E-5\t9.044259E-6\t5.656347E-6\t3.502370E-6\t2.147094E-6\r\n3.284471E-1\t2.258003E-6\t3.683285E-6\t5.948526E-6\t9.511442E-6\t1.505728E-5\t2.359986E-5\t3.662146E-5\t5.626325E-5\t8.558093E-5\t1.288820E-4\t1.921634E-4\t2.836690E-4\t4.145876E-4\t5.999068E-4\t8.594373E-4\t1.219011E-3\t1.711844E-3\t2.380038E-3\t3.276171E-3\t4.464905E-3\t6.024499E-3\t8.048088E-3\t1.064456E-2\t1.393880E-2\t1.807117E-2\t2.319585E-2\t2.947795E-2\t3.708918E-2\t4.620195E-2\t5.698183E-2\t6.957858E-2\t8.411584E-2\t1.006800E-1\t1.193085E-1\t1.399789E-1\t1.625987E-1\t1.869969E-1\t2.129192E-1\t2.400260E-1\t2.678951E-1\t2.960291E-1\t3.238673E-1\t3.508025E-1\t3.762023E-1\t3.994323E-1\t4.198827E-1\t4.369943E-1\t4.502841E-1\t4.593678E-1\t4.639781E-1\t4.639781E-1\t4.593678E-1\t4.502841E-1\t4.369943E-1\t4.198827E-1\t3.994323E-1\t3.762023E-1\t3.508025E-1\t3.238673E-1\t2.960291E-1\t2.678951E-1\t2.400260E-1\t2.129192E-1\t1.869969E-1\t1.625987E-1\t1.399789E-1\t1.193085E-1\t1.006800E-1\t8.411584E-2\t6.957858E-2\t5.698183E-2\t4.620195E-2\t3.708918E-2\t2.947795E-2\t2.319585E-2\t1.807117E-2\t1.393880E-2\t1.064456E-2\t8.048088E-3\t6.024499E-3\t4.464905E-3\t3.276171E-3\t2.380038E-3\t1.711844E-3\t1.219011E-3\t8.594373E-4\t5.999068E-4\t4.145876E-4\t2.836690E-4\t1.921634E-4\t1.288820E-4\t8.558093E-5\t5.626325E-5\t3.662146E-5\t2.359986E-5\t1.505728E-5\t9.511442E-6\t5.948526E-6\t3.683285E-6\t2.258003E-6\r\n3.734049E-1\t2.350898E-6\t3.834818E-6\t6.193252E-6\t9.902748E-6\t1.567674E-5\t2.457078E-5\t3.812809E-5\t5.857795E-5\t8.910179E-5\t1.341843E-4\t2.000691E-4\t2.953394E-4\t4.316440E-4\t6.245873E-4\t8.947952E-4\t1.269162E-3\t1.782271E-3\t2.477954E-3\t3.410955E-3\t4.648594E-3\t6.272351E-3\t8.379192E-3\t1.108248E-2\t1.451225E-2\t1.881463E-2\t2.415014E-2\t3.069069E-2\t3.861505E-2\t4.810273E-2\t5.932610E-2\t7.244109E-2\t8.757641E-2\t1.048220E-1\t1.242169E-1\t1.457377E-1\t1.692881E-1\t1.946901E-1\t2.216788E-1\t2.499008E-1\t2.789165E-1\t3.082079E-1\t3.371914E-1\t3.652348E-1\t3.916795E-1\t4.158652E-1\t4.371569E-1\t4.549725E-1\t4.688091E-1\t4.782665E-1\t4.830665E-1\t4.830665E-1\t4.782665E-1\t4.688091E-1\t4.549725E-1\t4.371569E-1\t4.158652E-1\t3.916795E-1\t3.652348E-1\t3.371914E-1\t3.082079E-1\t2.789165E-1\t2.499008E-1\t2.216788E-1\t1.946901E-1\t1.692881E-1\t1.457377E-1\t1.242169E-1\t1.048220E-1\t8.757641E-2\t7.244109E-2\t5.932610E-2\t4.810273E-2\t3.861505E-2\t3.069069E-2\t2.415014E-2\t1.881463E-2\t1.451225E-2\t1.108248E-2\t8.379192E-3\t6.272351E-3\t4.648594E-3\t3.410955E-3\t2.477954E-3\t1.782271E-3\t1.269162E-3\t8.947952E-4\t6.245873E-4\t4.316440E-4\t2.953394E-4\t2.000691E-4\t1.341843E-4\t8.910179E-5\t5.857795E-5\t3.812809E-5\t2.457078E-5\t1.567674E-5\t9.902748E-6\t6.193252E-6\t3.834818E-6\t2.350898E-6\r\n4.183626E-1\t2.423145E-6\t3.952667E-6\t6.383579E-6\t1.020707E-5\t1.615851E-5\t2.532587E-5\t3.929981E-5\t6.037813E-5\t9.184000E-5\t1.383080E-4\t2.062175E-4\t3.044155E-4\t4.449090E-4\t6.437817E-4\t9.222934E-4\t1.308165E-3\t1.837042E-3\t2.554105E-3\t3.515778E-3\t4.791452E-3\t6.465109E-3\t8.636695E-3\t1.142306E-2\t1.495823E-2\t1.939283E-2\t2.489230E-2\t3.163385E-2\t3.980174E-2\t4.958099E-2\t6.114927E-2\t7.466730E-2\t9.026775E-2\t1.080433E-1\t1.280342E-1\t1.502164E-1\t1.744905E-1\t2.006731E-1\t2.284913E-1\t2.575806E-1\t2.874880E-1\t3.176796E-1\t3.475537E-1\t3.764589E-1\t4.037163E-1\t4.286453E-1\t4.505913E-1\t4.689544E-1\t4.832162E-1\t4.929643E-1\t4.979118E-1\t4.979118E-1\t4.929643E-1\t4.832162E-1\t4.689544E-1\t4.505913E-1\t4.286453E-1\t4.037163E-1\t3.764589E-1\t3.475537E-1\t3.176796E-1\t2.874880E-1\t2.575806E-1\t2.284913E-1\t2.006731E-1\t1.744905E-1\t1.502164E-1\t1.280342E-1\t1.080433E-1\t9.026775E-2\t7.466730E-2\t6.114927E-2\t4.958099E-2\t3.980174E-2\t3.163385E-2\t2.489230E-2\t1.939283E-2\t1.495823E-2\t1.142306E-2\t8.636695E-3\t6.465109E-3\t4.791452E-3\t3.515778E-3\t2.554105E-3\t1.837042E-3\t1.308165E-3\t9.222934E-4\t6.437817E-4\t4.449090E-4\t3.044155E-4\t2.062175E-4\t1.383080E-4\t9.184000E-5\t6.037813E-5\t3.929981E-5\t2.532587E-5\t1.615851E-5\t1.020707E-5\t6.383579E-6\t3.952667E-6\t2.423145E-6\r\n4.633204E-1\t2.472640E-6\t4.033405E-6\t6.513970E-6\t1.041556E-5\t1.648856E-5\t2.584318E-5\t4.010255E-5\t6.161142E-5\t9.371593E-5\t1.411330E-4\t2.104297E-4\t3.106335E-4\t4.539967E-4\t6.569316E-4\t9.411322E-4\t1.334886E-3\t1.874566E-3\t2.606275E-3\t3.587591E-3\t4.889322E-3\t6.597165E-3\t8.813109E-3\t1.165639E-2\t1.526377E-2\t1.978895E-2\t2.540076E-2\t3.228001E-2\t4.061474E-2\t5.059373E-2\t6.239831E-2\t7.619246E-2\t9.211157E-2\t1.102502E-1\t1.306495E-1\t1.532848E-1\t1.780547E-1\t2.047721E-1\t2.331585E-1\t2.628420E-1\t2.933602E-1\t3.241685E-1\t3.546529E-1\t3.841485E-1\t4.119626E-1\t4.374008E-1\t4.597951E-1\t4.785333E-1\t4.930864E-1\t5.030336E-1\t5.080821E-1\t5.080821E-1\t5.030336E-1\t4.930864E-1\t4.785333E-1\t4.597951E-1\t4.374008E-1\t4.119626E-1\t3.841485E-1\t3.546529E-1\t3.241685E-1\t2.933602E-1\t2.628420E-1\t2.331585E-1\t2.047721E-1\t1.780547E-1\t1.532848E-1\t1.306495E-1\t1.102502E-1\t9.211157E-2\t7.619246E-2\t6.239831E-2\t5.059373E-2\t4.061474E-2\t3.228001E-2\t2.540076E-2\t1.978895E-2\t1.526377E-2\t1.165639E-2\t8.813109E-3\t6.597165E-3\t4.889322E-3\t3.587591E-3\t2.606275E-3\t1.874566E-3\t1.334886E-3\t9.411322E-4\t6.569316E-4\t4.539967E-4\t3.106335E-4\t2.104297E-4\t1.411330E-4\t9.371593E-5\t6.161142E-5\t4.010255E-5\t2.584318E-5\t1.648856E-5\t1.041556E-5\t6.513970E-6\t4.033405E-6\t2.472640E-6\r\n5.082782E-1\t2.497920E-6\t4.074641E-6\t6.580568E-6\t1.052205E-5\t1.665714E-5\t2.610739E-5\t4.051256E-5\t6.224132E-5\t9.467407E-5\t1.425760E-4\t2.125811E-4\t3.138094E-4\t4.586383E-4\t6.636480E-4\t9.507542E-4\t1.348534E-3\t1.893731E-3\t2.632922E-3\t3.624270E-3\t4.939310E-3\t6.664614E-3\t8.903213E-3\t1.177556E-2\t1.541982E-2\t1.999127E-2\t2.566045E-2\t3.261003E-2\t4.102998E-2\t5.111100E-2\t6.303626E-2\t7.697144E-2\t9.305330E-2\t1.113774E-1\t1.319852E-1\t1.548519E-1\t1.798751E-1\t2.068657E-1\t2.355423E-1\t2.655292E-1\t2.963595E-1\t3.274828E-1\t3.582788E-1\t3.880760E-1\t4.161745E-1\t4.418727E-1\t4.644960E-1\t4.834258E-1\t4.981277E-1\t5.081765E-1\t5.132767E-1\t5.132767E-1\t5.081765E-1\t4.981277E-1\t4.834258E-1\t4.644960E-1\t4.418727E-1\t4.161745E-1\t3.880760E-1\t3.582788E-1\t3.274828E-1\t2.963595E-1\t2.655292E-1\t2.355423E-1\t2.068657E-1\t1.798751E-1\t1.548519E-1\t1.319852E-1\t1.113774E-1\t9.305330E-2\t7.697144E-2\t6.303626E-2\t5.111100E-2\t4.102998E-2\t3.261003E-2\t2.566045E-2\t1.999127E-2\t1.541982E-2\t1.177556E-2\t8.903213E-3\t6.664614E-3\t4.939310E-3\t3.624270E-3\t2.632922E-3\t1.893731E-3\t1.348534E-3\t9.507542E-4\t6.636480E-4\t4.586383E-4\t3.138094E-4\t2.125811E-4\t1.425760E-4\t9.467407E-5\t6.224132E-5\t4.051256E-5\t2.610739E-5\t1.665714E-5\t1.052205E-5\t6.580568E-6\t4.074641E-6\t2.497920E-6\r\n5.532359E-1\t2.498229E-6\t4.075145E-6\t6.581381E-6\t1.052335E-5\t1.665920E-5\t2.611062E-5\t4.051756E-5\t6.224902E-5\t9.468577E-5\t1.425936E-4\t2.126074E-4\t3.138482E-4\t4.586950E-4\t6.637300E-4\t9.508717E-4\t1.348700E-3\t1.893965E-3\t2.633247E-3\t3.624718E-3\t4.939920E-3\t6.665438E-3\t8.904314E-3\t1.177702E-2\t1.542173E-2\t1.999374E-2\t2.566362E-2\t3.261407E-2\t4.103505E-2\t5.111731E-2\t6.304405E-2\t7.698095E-2\t9.306481E-2\t1.113912E-1\t1.320015E-1\t1.548711E-1\t1.798973E-1\t2.068912E-1\t2.355714E-1\t2.655621E-1\t2.963962E-1\t3.275233E-1\t3.583231E-1\t3.881239E-1\t4.162259E-1\t4.419273E-1\t4.645534E-1\t4.834855E-1\t4.981893E-1\t5.082393E-1\t5.133401E-1\t5.133401E-1\t5.082393E-1\t4.981893E-1\t4.834855E-1\t4.645534E-1\t4.419273E-1\t4.162259E-1\t3.881239E-1\t3.583231E-1\t3.275233E-1\t2.963962E-1\t2.655621E-1\t2.355714E-1\t2.068912E-1\t1.798973E-1\t1.548711E-1\t1.320015E-1\t1.113912E-1\t9.306481E-2\t7.698095E-2\t6.304405E-2\t5.111731E-2\t4.103505E-2\t3.261407E-2\t2.566362E-2\t1.999374E-2\t1.542173E-2\t1.177702E-2\t8.904314E-3\t6.665438E-3\t4.939920E-3\t3.624718E-3\t2.633247E-3\t1.893965E-3\t1.348700E-3\t9.508717E-4\t6.637300E-4\t4.586950E-4\t3.138482E-4\t2.126074E-4\t1.425936E-4\t9.468577E-5\t6.224902E-5\t4.051756E-5\t2.611062E-5\t1.665920E-5\t1.052335E-5\t6.581381E-6\t4.075145E-6\t2.498229E-6\r\n5.981937E-1\t2.473557E-6\t4.034901E-6\t6.516386E-6\t1.041943E-5\t1.649468E-5\t2.585276E-5\t4.011743E-5\t6.163427E-5\t9.375069E-5\t1.411854E-4\t2.105077E-4\t3.107488E-4\t4.541651E-4\t6.571753E-4\t9.414813E-4\t1.335381E-3\t1.875261E-3\t2.607242E-3\t3.588922E-3\t4.891136E-3\t6.599612E-3\t8.816378E-3\t1.166071E-2\t1.526943E-2\t1.979629E-2\t2.541018E-2\t3.229198E-2\t4.062980E-2\t5.061250E-2\t6.242146E-2\t7.622072E-2\t9.214574E-2\t1.102911E-1\t1.306979E-1\t1.533416E-1\t1.781207E-1\t2.048481E-1\t2.332450E-1\t2.629395E-1\t2.934691E-1\t3.242888E-1\t3.547844E-1\t3.842910E-1\t4.121154E-1\t4.375630E-1\t4.599657E-1\t4.787108E-1\t4.932693E-1\t5.032202E-1\t5.082706E-1\t5.082706E-1\t5.032202E-1\t4.932693E-1\t4.787108E-1\t4.599657E-1\t4.375630E-1\t4.121154E-1\t3.842910E-1\t3.547844E-1\t3.242888E-1\t2.934691E-1\t2.629395E-1\t2.332450E-1\t2.048481E-1\t1.781207E-1\t1.533416E-1\t1.306979E-1\t1.102911E-1\t9.214574E-2\t7.622072E-2\t6.242146E-2\t5.061250E-2\t4.062980E-2\t3.229198E-2\t2.541018E-2\t1.979629E-2\t1.526943E-2\t1.166071E-2\t8.816378E-3\t6.599612E-3\t4.891136E-3\t3.588922E-3\t2.607242E-3\t1.875261E-3\t1.335381E-3\t9.414813E-4\t6.571753E-4\t4.541651E-4\t3.107488E-4\t2.105077E-4\t1.411854E-4\t9.375069E-5\t6.163427E-5\t4.011743E-5\t2.585276E-5\t1.649468E-5\t1.041943E-5\t6.516386E-6\t4.034901E-6\t2.473557E-6\r\n6.431515E-1\t2.424643E-6\t3.955111E-6\t6.387525E-6\t1.021338E-5\t1.616850E-5\t2.534153E-5\t3.932411E-5\t6.041546E-5\t9.189679E-5\t1.383935E-4\t2.063450E-4\t3.046037E-4\t4.451841E-4\t6.441797E-4\t9.228636E-4\t1.308974E-3\t1.838178E-3\t2.555684E-3\t3.517952E-3\t4.794414E-3\t6.469106E-3\t8.642035E-3\t1.143012E-2\t1.496748E-2\t1.940482E-2\t2.490770E-2\t3.165341E-2\t3.982635E-2\t4.961164E-2\t6.118708E-2\t7.471346E-2\t9.032357E-2\t1.081101E-1\t1.281134E-1\t1.503093E-1\t1.745984E-1\t2.007972E-1\t2.286326E-1\t2.577399E-1\t2.876657E-1\t3.178760E-1\t3.477686E-1\t3.766917E-1\t4.039659E-1\t4.289103E-1\t4.508699E-1\t4.692444E-1\t4.835150E-1\t4.932690E-1\t4.982196E-1\t4.982196E-1\t4.932690E-1\t4.835150E-1\t4.692444E-1\t4.508699E-1\t4.289103E-1\t4.039659E-1\t3.766917E-1\t3.477686E-1\t3.178760E-1\t2.876657E-1\t2.577399E-1\t2.286326E-1\t2.007972E-1\t1.745984E-1\t1.503093E-1\t1.281134E-1\t1.081101E-1\t9.032357E-2\t7.471346E-2\t6.118708E-2\t4.961164E-2\t3.982635E-2\t3.165341E-2\t2.490770E-2\t1.940482E-2\t1.496748E-2\t1.143012E-2\t8.642035E-3\t6.469106E-3\t4.794414E-3\t3.517952E-3\t2.555684E-3\t1.838178E-3\t1.308974E-3\t9.228636E-4\t6.441797E-4\t4.451841E-4\t3.046037E-4\t2.063450E-4\t1.383935E-4\t9.189679E-5\t6.041546E-5\t3.932411E-5\t2.534153E-5\t1.616850E-5\t1.021338E-5\t6.387525E-6\t3.955111E-6\t2.424643E-6\r\n6.881092E-1\t2.352934E-6\t3.838138E-6\t6.198613E-6\t9.911321E-6\t1.569031E-5\t2.459205E-5\t3.816110E-5\t5.862867E-5\t8.917892E-5\t1.343005E-4\t2.002423E-4\t2.955950E-4\t4.320177E-4\t6.251280E-4\t8.955698E-4\t1.270261E-3\t1.783814E-3\t2.480100E-3\t3.413908E-3\t4.652618E-3\t6.277781E-3\t8.386446E-3\t1.109207E-2\t1.452481E-2\t1.883092E-2\t2.417105E-2\t3.071726E-2\t3.864848E-2\t4.814437E-2\t5.937746E-2\t7.250380E-2\t8.765223E-2\t1.049127E-1\t1.243244E-1\t1.458639E-1\t1.694346E-1\t1.948586E-1\t2.218707E-1\t2.501172E-1\t2.791580E-1\t3.084748E-1\t3.374833E-1\t3.655509E-1\t3.920185E-1\t4.162252E-1\t4.375354E-1\t4.553664E-1\t4.692150E-1\t4.786805E-1\t4.834847E-1\t4.834847E-1\t4.786805E-1\t4.692150E-1\t4.553664E-1\t4.375354E-1\t4.162252E-1\t3.920185E-1\t3.655509E-1\t3.374833E-1\t3.084748E-1\t2.791580E-1\t2.501172E-1\t2.218707E-1\t1.948586E-1\t1.694346E-1\t1.458639E-1\t1.243244E-1\t1.049127E-1\t8.765223E-2\t7.250380E-2\t5.937746E-2\t4.814437E-2\t3.864848E-2\t3.071726E-2\t2.417105E-2\t1.883092E-2\t1.452481E-2\t1.109207E-2\t8.386446E-3\t6.277781E-3\t4.652618E-3\t3.413908E-3\t2.480100E-3\t1.783814E-3\t1.270261E-3\t8.955698E-4\t6.251280E-4\t4.320177E-4\t2.955950E-4\t2.002423E-4\t1.343005E-4\t8.917892E-5\t5.862867E-5\t3.816110E-5\t2.459205E-5\t1.569031E-5\t9.911321E-6\t6.198613E-6\t3.838138E-6\t2.352934E-6\r\n7.330670E-1\t2.260516E-6\t3.687386E-6\t5.955147E-6\t9.522030E-6\t1.507404E-5\t2.362613E-5\t3.666222E-5\t5.632588E-5\t8.567620E-5\t1.290255E-4\t1.923773E-4\t2.839848E-4\t4.150491E-4\t6.005746E-4\t8.603941E-4\t1.220368E-3\t1.713750E-3\t2.382687E-3\t3.279818E-3\t4.469875E-3\t6.031206E-3\t8.057047E-3\t1.065641E-2\t1.395432E-2\t1.809129E-2\t2.322167E-2\t2.951076E-2\t3.713047E-2\t4.625338E-2\t5.704527E-2\t6.965604E-2\t8.420947E-2\t1.007920E-1\t1.194413E-1\t1.401347E-1\t1.627797E-1\t1.872050E-1\t2.131562E-1\t2.402932E-1\t2.681934E-1\t2.963586E-1\t3.242278E-1\t3.511930E-1\t3.766210E-1\t3.998769E-1\t4.203501E-1\t4.374808E-1\t4.507854E-1\t4.598792E-1\t4.644946E-1\t4.644946E-1\t4.598792E-1\t4.507854E-1\t4.374808E-1\t4.203501E-1\t3.998769E-1\t3.766210E-1\t3.511930E-1\t3.242278E-1\t2.963586E-1\t2.681934E-1\t2.402932E-1\t2.131562E-1\t1.872050E-1\t1.627797E-1\t1.401347E-1\t1.194413E-1\t1.007920E-1\t8.420947E-2\t6.965604E-2\t5.704527E-2\t4.625338E-2\t3.713047E-2\t2.951076E-2\t2.322167E-2\t1.809129E-2\t1.395432E-2\t1.065641E-2\t8.057047E-3\t6.031206E-3\t4.469875E-3\t3.279818E-3\t2.382687E-3\t1.713750E-3\t1.220368E-3\t8.603941E-4\t6.005746E-4\t4.150491E-4\t2.839848E-4\t1.923773E-4\t1.290255E-4\t8.567620E-5\t5.632588E-5\t3.666222E-5\t2.362613E-5\t1.507404E-5\t9.522030E-6\t5.955147E-6\t3.687386E-6\t2.260516E-6\r\n7.780248E-1\t2.150016E-6\t3.507136E-6\t5.664043E-6\t9.056566E-6\t1.433718E-5\t2.247122E-5\t3.487007E-5\t5.357251E-5\t8.148811E-5\t1.227184E-4\t1.829733E-4\t2.701028E-4\t3.947604E-4\t5.712168E-4\t8.183356E-4\t1.160713E-3\t1.629977E-3\t2.266215E-3\t3.119491E-3\t4.251375E-3\t5.736384E-3\t7.663196E-3\t1.013549E-2\t1.327219E-2\t1.720694E-2\t2.208653E-2\t2.806819E-2\t3.531543E-2\t4.399239E-2\t5.425673E-2\t6.625106E-2\t8.009308E-2\t9.586503E-2\t1.136027E-1\t1.332846E-1\t1.548225E-1\t1.780539E-1\t2.027366E-1\t2.285470E-1\t2.550833E-1\t2.818718E-1\t3.083786E-1\t3.340257E-1\t3.582108E-1\t3.803298E-1\t3.998022E-1\t4.160955E-1\t4.287497E-1\t4.373990E-1\t4.417888E-1\t4.417888E-1\t4.373990E-1\t4.287497E-1\t4.160955E-1\t3.998022E-1\t3.803298E-1\t3.582108E-1\t3.340257E-1\t3.083786E-1\t2.818718E-1\t2.550833E-1\t2.285470E-1\t2.027366E-1\t1.780539E-1\t1.548225E-1\t1.332846E-1\t1.136027E-1\t9.586503E-2\t8.009308E-2\t6.625106E-2\t5.425673E-2\t4.399239E-2\t3.531543E-2\t2.806819E-2\t2.208653E-2\t1.720694E-2\t1.327219E-2\t1.013549E-2\t7.663196E-3\t5.736384E-3\t4.251375E-3\t3.119491E-3\t2.266215E-3\t1.629977E-3\t1.160713E-3\t8.183356E-4\t5.712168E-4\t3.947604E-4\t2.701028E-4\t1.829733E-4\t1.227184E-4\t8.148811E-5\t5.357251E-5\t3.487007E-5\t2.247122E-5\t1.433718E-5\t9.056566E-6\t5.664043E-6\t3.507136E-6\t2.150016E-6\r\n8.229825E-1\t2.024472E-6\t3.302347E-6\t5.333308E-6\t8.527735E-6\t1.350000E-5\t2.115908E-5\t3.283394E-5\t5.044431E-5\t7.672985E-5\t1.155526E-4\t1.722892E-4\t2.543310E-4\t3.717095E-4\t5.378623E-4\t7.705513E-4\t1.092937E-3\t1.534799E-3\t2.133886E-3\t2.937338E-3\t4.003129E-3\t5.401424E-3\t7.215727E-3\t9.543658E-3\t1.249720E-2\t1.620219E-2\t2.079685E-2\t2.642923E-2\t3.325329E-2\t4.142358E-2\t5.108857E-2\t6.238252E-2\t7.541628E-2\t9.026728E-2\t1.069692E-1\t1.255018E-1\t1.457821E-1\t1.676570E-1\t1.908983E-1\t2.152017E-1\t2.401885E-1\t2.654127E-1\t2.903718E-1\t3.145213E-1\t3.372941E-1\t3.581216E-1\t3.764569E-1\t3.917988E-1\t4.037142E-1\t4.118584E-1\t4.159919E-1\t4.159919E-1\t4.118584E-1\t4.037142E-1\t3.917988E-1\t3.764569E-1\t3.581216E-1\t3.372941E-1\t3.145213E-1\t2.903718E-1\t2.654127E-1\t2.401885E-1\t2.152017E-1\t1.908983E-1\t1.676570E-1\t1.457821E-1\t1.255018E-1\t1.069692E-1\t9.026728E-2\t7.541628E-2\t6.238252E-2\t5.108857E-2\t4.142358E-2\t3.325329E-2\t2.642923E-2\t2.079685E-2\t1.620219E-2\t1.249720E-2\t9.543658E-3\t7.215727E-3\t5.401424E-3\t4.003129E-3\t2.937338E-3\t2.133886E-3\t1.534799E-3\t1.092937E-3\t7.705513E-4\t5.378623E-4\t3.717095E-4\t2.543310E-4\t1.722892E-4\t1.155526E-4\t7.672985E-5\t5.044431E-5\t3.283394E-5\t2.115908E-5\t1.350000E-5\t8.527735E-6\t5.333308E-6\t3.302347E-6\t2.024472E-6\r\n8.679403E-1\t1.887200E-6\t3.078427E-6\t4.971677E-6\t7.949501E-6\t1.258461E-5\t1.972436E-5\t3.060759E-5\t4.702387E-5\t7.152709E-5\t1.077174E-4\t1.606069E-4\t2.370858E-4\t3.465053E-4\t5.013919E-4\t7.183031E-4\t1.018829E-3\t1.430731E-3\t1.989195E-3\t2.738168E-3\t3.731692E-3\t5.035174E-3\t6.726455E-3\t8.896539E-3\t1.164981E-2\t1.510358E-2\t1.938669E-2\t2.463717E-2\t3.099851E-2\t3.861481E-2\t4.762445E-2\t5.815260E-2\t7.030259E-2\t8.414659E-2\t9.971599E-2\t1.169920E-1\t1.358972E-1\t1.562888E-1\t1.779542E-1\t2.006097E-1\t2.239022E-1\t2.474161E-1\t2.706828E-1\t2.931948E-1\t3.144235E-1\t3.338387E-1\t3.509308E-1\t3.652324E-1\t3.763398E-1\t3.839318E-1\t3.877850E-1\t3.877850E-1\t3.839318E-1\t3.763398E-1\t3.652324E-1\t3.509308E-1\t3.338387E-1\t3.144235E-1\t2.931948E-1\t2.706828E-1\t2.474161E-1\t2.239022E-1\t2.006097E-1\t1.779542E-1\t1.562888E-1\t1.358972E-1\t1.169920E-1\t9.971599E-2\t8.414659E-2\t7.030259E-2\t5.815260E-2\t4.762445E-2\t3.861481E-2\t3.099851E-2\t2.463717E-2\t1.938669E-2\t1.510358E-2\t1.164981E-2\t8.896539E-3\t6.726455E-3\t5.035174E-3\t3.731692E-3\t2.738168E-3\t1.989195E-3\t1.430731E-3\t1.018829E-3\t7.183031E-4\t5.013919E-4\t3.465053E-4\t2.370858E-4\t1.606069E-4\t1.077174E-4\t7.152709E-5\t4.702387E-5\t3.060759E-5\t1.972436E-5\t1.258461E-5\t7.949501E-6\t4.971677E-6\t3.078427E-6\t1.887200E-6\r\n9.128981E-1\t1.741647E-6\t2.841000E-6\t4.588230E-6\t7.336386E-6\t1.161401E-5\t1.820310E-5\t2.824694E-5\t4.339709E-5\t6.601047E-5\t9.940954E-5\t1.482199E-4\t2.188002E-4\t3.197806E-4\t4.627214E-4\t6.629031E-4\t9.402504E-4\t1.320384E-3\t1.835776E-3\t2.526983E-3\t3.443880E-3\t4.646830E-3\t6.207669E-3\t8.210382E-3\t1.075131E-2\t1.393869E-2\t1.789147E-2\t2.273699E-2\t2.860771E-2\t3.563659E-2\t4.395135E-2\t5.366750E-2\t6.488041E-2\t7.765668E-2\t9.202527E-2\t1.079688E-1\t1.254159E-1\t1.442348E-1\t1.642293E-1\t1.851374E-1\t2.066335E-1\t2.283338E-1\t2.498060E-1\t2.705818E-1\t2.901731E-1\t3.080910E-1\t3.238648E-1\t3.370634E-1\t3.473141E-1\t3.543206E-1\t3.578766E-1\t3.578766E-1\t3.543206E-1\t3.473141E-1\t3.370634E-1\t3.238648E-1\t3.080910E-1\t2.901731E-1\t2.705818E-1\t2.498060E-1\t2.283338E-1\t2.066335E-1\t1.851374E-1\t1.642293E-1\t1.442348E-1\t1.254159E-1\t1.079688E-1\t9.202527E-2\t7.765668E-2\t6.488041E-2\t5.366750E-2\t4.395135E-2\t3.563659E-2\t2.860771E-2\t2.273699E-2\t1.789147E-2\t1.393869E-2\t1.075131E-2\t8.210382E-3\t6.207669E-3\t4.646830E-3\t3.443880E-3\t2.526983E-3\t1.835776E-3\t1.320384E-3\t9.402504E-4\t6.629031E-4\t4.627214E-4\t3.197806E-4\t2.188002E-4\t1.482199E-4\t9.940954E-5\t6.601047E-5\t4.339709E-5\t2.824694E-5\t1.820310E-5\t1.161401E-5\t7.336386E-6\t4.588230E-6\t2.841000E-6\t1.741647E-6\r\n9.578558E-1\t1.591251E-6\t2.595670E-6\t4.192021E-6\t6.702865E-6\t1.061110E-5\t1.663120E-5\t2.580773E-5\t3.964961E-5\t6.031025E-5\t9.082521E-5\t1.354206E-4\t1.999061E-4\t2.921665E-4\t4.227639E-4\t6.056593E-4\t8.590568E-4\t1.206364E-3\t1.677251E-3\t2.308770E-3\t3.146490E-3\t4.245561E-3\t5.671617E-3\t7.501389E-3\t9.822896E-3\t1.273504E-2\t1.634648E-2\t2.077358E-2\t2.613734E-2\t3.255925E-2\t4.015601E-2\t4.903314E-2\t5.927778E-2\t7.095077E-2\t8.407859E-2\t9.864538E-2\t1.145859E-1\t1.317797E-1\t1.500476E-1\t1.691502E-1\t1.887900E-1\t2.086165E-1\t2.282344E-1\t2.472161E-1\t2.651158E-1\t2.814863E-1\t2.958980E-1\t3.079569E-1\t3.173224E-1\t3.237238E-1\t3.269728E-1\t3.269728E-1\t3.237238E-1\t3.173224E-1\t3.079569E-1\t2.958980E-1\t2.814863E-1\t2.651158E-1\t2.472161E-1\t2.282344E-1\t2.086165E-1\t1.887900E-1\t1.691502E-1\t1.500476E-1\t1.317797E-1\t1.145859E-1\t9.864538E-2\t8.407859E-2\t7.095077E-2\t5.927778E-2\t4.903314E-2\t4.015601E-2\t3.255925E-2\t2.613734E-2\t2.077358E-2\t1.634648E-2\t1.273504E-2\t9.822896E-3\t7.501389E-3\t5.671617E-3\t4.245561E-3\t3.146490E-3\t2.308770E-3\t1.677251E-3\t1.206364E-3\t8.590568E-4\t6.056593E-4\t4.227639E-4\t2.921665E-4\t1.999061E-4\t1.354206E-4\t9.082521E-5\t6.031025E-5\t3.964961E-5\t2.580773E-5\t1.663120E-5\t1.061110E-5\t6.702865E-6\t4.192021E-6\t2.595670E-6\t1.591251E-6\r\n1.002814E+0\t1.439306E-6\t2.347815E-6\t3.791734E-6\t6.062823E-6\t9.597872E-6\t1.504312E-5\t2.334340E-5\t3.586356E-5\t5.455136E-5\t8.215251E-5\t1.224896E-4\t1.808175E-4\t2.642682E-4\t3.823951E-4\t5.478262E-4\t7.770273E-4\t1.091171E-3\t1.517094E-3\t2.088311E-3\t2.846038E-3\t3.840162E-3\t5.130046E-3\t6.785097E-3\t8.884929E-3\t1.151900E-2\t1.478559E-2\t1.878996E-2\t2.364154E-2\t2.945024E-2\t3.632160E-2\t4.435107E-2\t5.361747E-2\t6.417584E-2\t7.605011E-2\t8.922594E-2\t1.036443E-1\t1.191963E-1\t1.357198E-1\t1.529984E-1\t1.707628E-1\t1.886961E-1\t2.064408E-1\t2.236100E-1\t2.398004E-1\t2.546078E-1\t2.676434E-1\t2.785507E-1\t2.870220E-1\t2.928122E-1\t2.957509E-1\t2.957509E-1\t2.928122E-1\t2.870220E-1\t2.785507E-1\t2.676434E-1\t2.546078E-1\t2.398004E-1\t2.236100E-1\t2.064408E-1\t1.886961E-1\t1.707628E-1\t1.529984E-1\t1.357198E-1\t1.191963E-1\t1.036443E-1\t8.922594E-2\t7.605011E-2\t6.417584E-2\t5.361747E-2\t4.435107E-2\t3.632160E-2\t2.945024E-2\t2.364154E-2\t1.878996E-2\t1.478559E-2\t1.151900E-2\t8.884929E-3\t6.785097E-3\t5.130046E-3\t3.840162E-3\t2.846038E-3\t2.088311E-3\t1.517094E-3\t1.091171E-3\t7.770273E-4\t5.478262E-4\t3.823951E-4\t2.642682E-4\t1.808175E-4\t1.224896E-4\t8.215251E-5\t5.455136E-5\t3.586356E-5\t2.334340E-5\t1.504312E-5\t9.597872E-6\t6.062823E-6\t3.791734E-6\t2.347815E-6\t1.439306E-6\r\n1.047771E+0\t1.288853E-6\t2.102395E-6\t3.395380E-6\t5.429069E-6\t8.594595E-6\t1.347065E-5\t2.090329E-5\t3.211470E-5\t4.884904E-5\t7.356501E-5\t1.096856E-4\t1.619164E-4\t2.366439E-4\t3.424229E-4\t4.905613E-4\t6.958037E-4\t9.771097E-4\t1.358510E-3\t1.870017E-3\t2.548539E-3\t3.438745E-3\t4.593796E-3\t6.075843E-3\t7.956177E-3\t1.031491E-2\t1.324004E-2\t1.682582E-2\t2.117026E-2\t2.637177E-2\t3.252486E-2\t3.971500E-2\t4.801277E-2\t5.746746E-2\t6.810050E-2\t7.989905E-2\t9.281026E-2\t1.067366E-1\t1.215329E-1\t1.370053E-1\t1.529128E-1\t1.689715E-1\t1.848613E-1\t2.002358E-1\t2.147338E-1\t2.279933E-1\t2.396663E-1\t2.494335E-1\t2.570193E-1\t2.622042E-1\t2.648357E-1\t2.648357E-1\t2.622042E-1\t2.570193E-1\t2.494335E-1\t2.396663E-1\t2.279933E-1\t2.147338E-1\t2.002358E-1\t1.848613E-1\t1.689715E-1\t1.529128E-1\t1.370053E-1\t1.215329E-1\t1.067366E-1\t9.281026E-2\t7.989905E-2\t6.810050E-2\t5.746746E-2\t4.801277E-2\t3.971500E-2\t3.252486E-2\t2.637177E-2\t2.117026E-2\t1.682582E-2\t1.324004E-2\t1.031491E-2\t7.956177E-3\t6.075843E-3\t4.593796E-3\t3.438745E-3\t2.548539E-3\t1.870017E-3\t1.358510E-3\t9.771097E-4\t6.958037E-4\t4.905613E-4\t3.424229E-4\t2.366439E-4\t1.619164E-4\t1.096856E-4\t7.356501E-5\t4.884904E-5\t3.211470E-5\t2.090329E-5\t1.347065E-5\t8.594595E-6\t5.429069E-6\t3.395380E-6\t2.102395E-6\t1.288853E-6\r\n1.092729E+0\t1.142589E-6\t1.863807E-6\t3.010058E-6\t4.812956E-6\t7.619245E-6\t1.194194E-5\t1.853110E-5\t2.847019E-5\t4.330545E-5\t6.521655E-5\t9.723803E-5\t1.435415E-4\t2.097886E-4\t3.035633E-4\t4.348904E-4\t6.168411E-4\t8.662233E-4\t1.204341E-3\t1.657800E-3\t2.259320E-3\t3.048502E-3\t4.072474E-3\t5.386332E-3\t7.053277E-3\t9.144329E-3\t1.173751E-2\t1.491636E-2\t1.876778E-2\t2.337900E-2\t2.883381E-2\t3.520798E-2\t4.256409E-2\t5.094582E-2\t6.037218E-2\t7.083178E-2\t8.227777E-2\t9.462370E-2\t1.077408E-1\t1.214574E-1\t1.355596E-1\t1.497959E-1\t1.638825E-1\t1.775122E-1\t1.903649E-1\t2.021197E-1\t2.124680E-1\t2.211268E-1\t2.278517E-1\t2.324482E-1\t2.347811E-1\t2.347811E-1\t2.324482E-1\t2.278517E-1\t2.211268E-1\t2.124680E-1\t2.021197E-1\t1.903649E-1\t1.775122E-1\t1.638825E-1\t1.497959E-1\t1.355596E-1\t1.214574E-1\t1.077408E-1\t9.462370E-2\t8.227777E-2\t7.083178E-2\t6.037218E-2\t5.094582E-2\t4.256409E-2\t3.520798E-2\t2.883381E-2\t2.337900E-2\t1.876778E-2\t1.491636E-2\t1.173751E-2\t9.144329E-3\t7.053277E-3\t5.386332E-3\t4.072474E-3\t3.048502E-3\t2.259320E-3\t1.657800E-3\t1.204341E-3\t8.662233E-4\t6.168411E-4\t4.348904E-4\t3.035633E-4\t2.097886E-4\t1.435415E-4\t9.723803E-5\t6.521655E-5\t4.330545E-5\t2.847019E-5\t1.853110E-5\t1.194194E-5\t7.619245E-6\t4.812956E-6\t3.010058E-6\t1.863807E-6\t1.142589E-6\r\n1.137687E+0\t1.002796E-6\t1.635775E-6\t2.641785E-6\t4.224103E-6\t6.687050E-6\t1.048088E-5\t1.626387E-5\t2.498694E-5\t3.800714E-5\t5.723748E-5\t8.534121E-5\t1.259796E-4\t1.841215E-4\t2.664231E-4\t3.816826E-4\t5.413722E-4\t7.602431E-4\t1.056993E-3\t1.454972E-3\t1.982898E-3\t2.675526E-3\t3.574217E-3\t4.727328E-3\t6.190327E-3\t8.025544E-3\t1.030145E-2\t1.309138E-2\t1.647159E-2\t2.051864E-2\t2.530606E-2\t3.090038E-2\t3.735648E-2\t4.471273E-2\t5.298580E-2\t6.216570E-2\t7.221130E-2\t8.304674E-2\t9.455903E-2\t1.065974E-1\t1.189743E-1\t1.314688E-1\t1.438319E-1\t1.557941E-1\t1.670743E-1\t1.773909E-1\t1.864731E-1\t1.940725E-1\t1.999746E-1\t2.040087E-1\t2.060562E-1\t2.060562E-1\t2.040087E-1\t1.999746E-1\t1.940725E-1\t1.864731E-1\t1.773909E-1\t1.670743E-1\t1.557941E-1\t1.438319E-1\t1.314688E-1\t1.189743E-1\t1.065974E-1\t9.455903E-2\t8.304674E-2\t7.221130E-2\t6.216570E-2\t5.298580E-2\t4.471273E-2\t3.735648E-2\t3.090038E-2\t2.530606E-2\t2.051864E-2\t1.647159E-2\t1.309138E-2\t1.030145E-2\t8.025544E-3\t6.190327E-3\t4.727328E-3\t3.574217E-3\t2.675526E-3\t1.982898E-3\t1.454972E-3\t1.056993E-3\t7.602431E-4\t5.413722E-4\t3.816826E-4\t2.664231E-4\t1.841215E-4\t1.259796E-4\t8.534121E-5\t5.723748E-5\t3.800714E-5\t2.498694E-5\t1.626387E-5\t1.048088E-5\t6.687050E-6\t4.224103E-6\t2.641785E-6\t1.635775E-6\t1.002796E-6\r\n1.182645E+0\t8.713073E-7\t1.421289E-6\t2.295389E-6\t3.670230E-6\t5.810229E-6\t9.106602E-6\t1.413131E-5\t2.171059E-5\t3.302356E-5\t4.973237E-5\t7.415108E-5\t1.094608E-4\t1.599791E-4\t2.314891E-4\t3.316356E-4\t4.703863E-4\t6.605583E-4\t9.183977E-4\t1.264193E-3\t1.722896E-3\t2.324705E-3\t3.105558E-3\t4.107470E-3\t5.378638E-3\t6.973217E-3\t8.950702E-3\t1.137481E-2\t1.431180E-2\t1.782819E-2\t2.198788E-2\t2.684865E-2\t3.245822E-2\t3.884990E-2\t4.603818E-2\t5.401439E-2\t6.274279E-2\t7.215746E-2\t8.216024E-2\t9.262009E-2\t1.033741E-1\t1.142303E-1\t1.249723E-1\t1.353660E-1\t1.451671E-1\t1.541310E-1\t1.620223E-1\t1.686253E-1\t1.737535E-1\t1.772587E-1\t1.790377E-1\t1.790377E-1\t1.772587E-1\t1.737535E-1\t1.686253E-1\t1.620223E-1\t1.541310E-1\t1.451671E-1\t1.353660E-1\t1.249723E-1\t1.142303E-1\t1.033741E-1\t9.262009E-2\t8.216024E-2\t7.215746E-2\t6.274279E-2\t5.401439E-2\t4.603818E-2\t3.884990E-2\t3.245822E-2\t2.684865E-2\t2.198788E-2\t1.782819E-2\t1.431180E-2\t1.137481E-2\t8.950702E-3\t6.973217E-3\t5.378638E-3\t4.107470E-3\t3.105558E-3\t2.324705E-3\t1.722896E-3\t1.264193E-3\t9.183977E-4\t6.605583E-4\t4.703863E-4\t3.316356E-4\t2.314891E-4\t1.599791E-4\t1.094608E-4\t7.415108E-5\t4.973237E-5\t3.302356E-5\t2.171059E-5\t1.413131E-5\t9.106602E-6\t5.810229E-6\t3.670230E-6\t2.295389E-6\t1.421289E-6\t8.713073E-7\r\n1.227602E+0\t7.494904E-7\t1.222579E-6\t1.974472E-6\t3.157097E-6\t4.997906E-6\t7.833415E-6\t1.215562E-5\t1.867525E-5\t2.840656E-5\t4.277933E-5\t6.378407E-5\t9.415721E-5\t1.376125E-4\t1.991248E-4\t2.852698E-4\t4.046219E-4\t5.682062E-4\t7.899972E-4\t1.087447E-3\t1.482019E-3\t1.999690E-3\t2.671372E-3\t3.533208E-3\t4.626654E-3\t5.998297E-3\t7.699311E-3\t9.784505E-3\t1.231087E-2\t1.533564E-2\t1.891377E-2\t2.309496E-2\t2.792026E-2\t3.341832E-2\t3.960162E-2\t4.646268E-2\t5.397077E-2\t6.206918E-2\t7.067348E-2\t7.967094E-2\t8.892144E-2\t9.825984E-2\t1.075001E-1\t1.164406E-1\t1.248714E-1\t1.325821E-1\t1.393701E-1\t1.450499E-1\t1.494611E-1\t1.524763E-1\t1.540065E-1\t1.540065E-1\t1.524763E-1\t1.494611E-1\t1.450499E-1\t1.393701E-1\t1.325821E-1\t1.248714E-1\t1.164406E-1\t1.075001E-1\t9.825984E-2\t8.892144E-2\t7.967094E-2\t7.067348E-2\t6.206918E-2\t5.397077E-2\t4.646268E-2\t3.960162E-2\t3.341832E-2\t2.792026E-2\t2.309496E-2\t1.891377E-2\t1.533564E-2\t1.231087E-2\t9.784505E-3\t7.699311E-3\t5.998297E-3\t4.626654E-3\t3.533208E-3\t2.671372E-3\t1.999690E-3\t1.482019E-3\t1.087447E-3\t7.899972E-4\t5.682062E-4\t4.046219E-4\t2.852698E-4\t1.991248E-4\t1.376125E-4\t9.415721E-5\t6.378407E-5\t4.277933E-5\t2.840656E-5\t1.867525E-5\t1.215562E-5\t7.833415E-6\t4.997906E-6\t3.157097E-6\t1.974472E-6\t1.222579E-6\t7.494904E-7\r\n1.272560E+0\t6.382590E-7\t1.041137E-6\t1.681442E-6\t2.688554E-6\t4.256169E-6\t6.670862E-6\t1.035161E-5\t1.590367E-5\t2.419076E-5\t3.643047E-5\t5.431791E-5\t8.018339E-5\t1.171895E-4\t1.695728E-4\t2.429331E-4\t3.445722E-4\t4.838790E-4\t6.727542E-4\t9.260598E-4\t1.262074E-3\t1.702917E-3\t2.274915E-3\t3.008846E-3\t3.940015E-3\t5.108093E-3\t6.556661E-3\t8.332392E-3\t1.048382E-2\t1.305969E-2\t1.610679E-2\t1.966745E-2\t2.377663E-2\t2.845873E-2\t3.372436E-2\t3.956718E-2\t4.596100E-2\t5.285753E-2\t6.018487E-2\t6.784702E-2\t7.572466E-2\t8.367716E-2\t9.154603E-2\t9.915970E-2\t1.063393E-1\t1.129056E-1\t1.186863E-1\t1.235231E-1\t1.272797E-1\t1.298473E-1\t1.311505E-1\t1.311505E-1\t1.298473E-1\t1.272797E-1\t1.235231E-1\t1.186863E-1\t1.129056E-1\t1.063393E-1\t9.915970E-2\t9.154603E-2\t8.367716E-2\t7.572466E-2\t6.784702E-2\t6.018487E-2\t5.285753E-2\t4.596100E-2\t3.956718E-2\t3.372436E-2\t2.845873E-2\t2.377663E-2\t1.966745E-2\t1.610679E-2\t1.305969E-2\t1.048382E-2\t8.332392E-3\t6.556661E-3\t5.108093E-3\t3.940015E-3\t3.008846E-3\t2.274915E-3\t1.702917E-3\t1.262074E-3\t9.260598E-4\t6.727542E-4\t4.838790E-4\t3.445722E-4\t2.429331E-4\t1.695728E-4\t1.171895E-4\t8.018339E-5\t5.431791E-5\t3.643047E-5\t2.419076E-5\t1.590367E-5\t1.035161E-5\t6.670862E-6\t4.256169E-6\t2.688554E-6\t1.681442E-6\t1.041137E-6\t6.382590E-7\r\n1.317518E+0\t5.381011E-7\t8.777579E-7\t1.417584E-6\t2.266657E-6\t3.588276E-6\t5.624046E-6\t8.727202E-6\t1.340801E-5\t2.039466E-5\t3.071367E-5\t4.579415E-5\t6.760072E-5\t9.879972E-5\t1.429628E-4\t2.048112E-4\t2.905007E-4\t4.079470E-4\t5.671831E-4\t7.807391E-4\t1.064024E-3\t1.435689E-3\t1.917927E-3\t2.536687E-3\t3.321734E-3\t4.306512E-3\t5.527766E-3\t7.024843E-3\t8.838664E-3\t1.101031E-2\t1.357925E-2\t1.658116E-2\t2.004551E-2\t2.399288E-2\t2.843221E-2\t3.335815E-2\t3.874863E-2\t4.456293E-2\t5.074044E-2\t5.720022E-2\t6.384167E-2\t7.054623E-2\t7.718030E-2\t8.359920E-2\t8.965217E-2\t9.518808E-2\t1.000616E-1\t1.041394E-1\t1.073065E-1\t1.094712E-1\t1.105699E-1\t1.105699E-1\t1.094712E-1\t1.073065E-1\t1.041394E-1\t1.000616E-1\t9.518808E-2\t8.965217E-2\t8.359920E-2\t7.718030E-2\t7.054623E-2\t6.384167E-2\t5.720022E-2\t5.074044E-2\t4.456293E-2\t3.874863E-2\t3.335815E-2\t2.843221E-2\t2.399288E-2\t2.004551E-2\t1.658116E-2\t1.357925E-2\t1.101031E-2\t8.838664E-3\t7.024843E-3\t5.527766E-3\t4.306512E-3\t3.321734E-3\t2.536687E-3\t1.917927E-3\t1.435689E-3\t1.064024E-3\t7.807391E-4\t5.671831E-4\t4.079470E-4\t2.905007E-4\t2.048112E-4\t1.429628E-4\t9.879972E-5\t6.760072E-5\t4.579415E-5\t3.071367E-5\t2.039466E-5\t1.340801E-5\t8.727202E-6\t5.624046E-6\t3.588276E-6\t2.266657E-6\t1.417584E-6\t8.777579E-7\t5.381011E-7\r\n1.362476E+0\t4.491246E-7\t7.326183E-7\t1.183182E-6\t1.891859E-6\t2.994944E-6\t4.694095E-6\t7.284135E-6\t1.119096E-5\t1.702235E-5\t2.563508E-5\t3.822196E-5\t5.642276E-5\t8.246292E-5\t1.193235E-4\t1.709451E-4\t2.424656E-4\t3.404918E-4\t4.733978E-4\t6.516418E-4\t8.880851E-4\t1.198294E-3\t1.600793E-3\t2.117239E-3\t2.772476E-3\t3.594419E-3\t4.613735E-3\t5.863266E-3\t7.377167E-3\t9.189729E-3\t1.133388E-2\t1.383942E-2\t1.673093E-2\t2.002559E-2\t2.373087E-2\t2.784229E-2\t3.234144E-2\t3.719433E-2\t4.235037E-2\t4.774201E-2\t5.328528E-2\t5.888122E-2\t6.441832E-2\t6.977584E-2\t7.482794E-2\t7.944847E-2\t8.351612E-2\t8.691969E-2\t8.956308E-2\t9.136985E-2\t9.228686E-2\t9.228686E-2\t9.136985E-2\t8.956308E-2\t8.691969E-2\t8.351612E-2\t7.944847E-2\t7.482794E-2\t6.977584E-2\t6.441832E-2\t5.888122E-2\t5.328528E-2\t4.774201E-2\t4.235037E-2\t3.719433E-2\t3.234144E-2\t2.784229E-2\t2.373087E-2\t2.002559E-2\t1.673093E-2\t1.383942E-2\t1.133388E-2\t9.189729E-3\t7.377167E-3\t5.863266E-3\t4.613735E-3\t3.594419E-3\t2.772476E-3\t2.117239E-3\t1.600793E-3\t1.198294E-3\t8.880851E-4\t6.516418E-4\t4.733978E-4\t3.404918E-4\t2.424656E-4\t1.709451E-4\t1.193235E-4\t8.246292E-5\t5.642276E-5\t3.822196E-5\t2.563508E-5\t1.702235E-5\t1.119096E-5\t7.284135E-6\t4.694095E-6\t2.994944E-6\t1.891859E-6\t1.183182E-6\t7.326183E-7\t4.491246E-7\r\n1.407434E+0\t3.711128E-7\t6.053643E-7\t9.776666E-7\t1.563248E-6\t2.474730E-6\t3.878742E-6\t6.018899E-6\t9.247114E-6\t1.406561E-5\t2.118233E-5\t3.158290E-5\t4.662226E-5\t6.813931E-5\t9.859734E-5\t1.412523E-4\t2.003499E-4\t2.813492E-4\t3.911698E-4\t5.384532E-4\t7.338270E-4\t9.901532E-4\t1.322739E-3\t1.749480E-3\t2.290904E-3\t2.970077E-3\t3.812340E-3\t4.844831E-3\t6.095771E-3\t7.593495E-3\t9.365217E-3\t1.143555E-2\t1.382481E-2\t1.654720E-2\t1.960888E-2\t2.300615E-2\t2.672381E-2\t3.073377E-2\t3.499421E-2\t3.944934E-2\t4.402976E-2\t4.865370E-2\t5.322902E-2\t5.765595E-2\t6.183051E-2\t6.564847E-2\t6.900958E-2\t7.182195E-2\t7.400619E-2\t7.549914E-2\t7.625686E-2\t7.625686E-2\t7.549914E-2\t7.400619E-2\t7.182195E-2\t6.900958E-2\t6.564847E-2\t6.183051E-2\t5.765595E-2\t5.322902E-2\t4.865370E-2\t4.402976E-2\t3.944934E-2\t3.499421E-2\t3.073377E-2\t2.672381E-2\t2.300615E-2\t1.960888E-2\t1.654720E-2\t1.382481E-2\t1.143555E-2\t9.365217E-3\t7.593495E-3\t6.095771E-3\t4.844831E-3\t3.812340E-3\t2.970077E-3\t2.290904E-3\t1.749480E-3\t1.322739E-3\t9.901532E-4\t7.338270E-4\t5.384532E-4\t3.911698E-4\t2.813492E-4\t2.003499E-4\t1.412523E-4\t9.859734E-5\t6.813931E-5\t4.662226E-5\t3.158290E-5\t2.118233E-5\t1.406561E-5\t9.247114E-6\t6.018899E-6\t3.878742E-6\t2.474730E-6\t1.563248E-6\t9.776666E-7\t6.053643E-7\t3.711128E-7\r\n1.452391E+0\t3.035855E-7\t4.952129E-7\t7.997714E-7\t1.278801E-6\t2.024431E-6\t3.172971E-6\t4.923707E-6\t7.564520E-6\t1.150624E-5\t1.732802E-5\t2.583611E-5\t3.813893E-5\t5.574076E-5\t8.065667E-5\t1.155502E-4\t1.638945E-4\t2.301552E-4\t3.199930E-4\t4.404769E-4\t6.003006E-4\t8.099860E-4\t1.082055E-3\t1.431147E-3\t1.874053E-3\t2.429645E-3\t3.118651E-3\t3.963271E-3\t4.986592E-3\t6.211791E-3\t7.661132E-3\t9.354749E-3\t1.130926E-2\t1.353629E-2\t1.604087E-2\t1.881998E-2\t2.186118E-2\t2.514149E-2\t2.862671E-2\t3.227118E-2\t3.601815E-2\t3.980072E-2\t4.354353E-2\t4.716494E-2\t5.057990E-2\t5.370314E-2\t5.645267E-2\t5.875331E-2\t6.054011E-2\t6.176140E-2\t6.238125E-2\t6.238125E-2\t6.176140E-2\t6.054011E-2\t5.875331E-2\t5.645267E-2\t5.370314E-2\t5.057990E-2\t4.716494E-2\t4.354353E-2\t3.980072E-2\t3.601815E-2\t3.227118E-2\t2.862671E-2\t2.514149E-2\t2.186118E-2\t1.881998E-2\t1.604087E-2\t1.353629E-2\t1.130926E-2\t9.354749E-3\t7.661132E-3\t6.211791E-3\t4.986592E-3\t3.963271E-3\t3.118651E-3\t2.429645E-3\t1.874053E-3\t1.431147E-3\t1.082055E-3\t8.099860E-4\t6.003006E-4\t4.404769E-4\t3.199930E-4\t2.301552E-4\t1.638945E-4\t1.155502E-4\t8.065667E-5\t5.574076E-5\t3.813893E-5\t2.583611E-5\t1.732802E-5\t1.150624E-5\t7.564520E-6\t4.923707E-6\t3.172971E-6\t2.024431E-6\t1.278801E-6\t7.997714E-7\t4.952129E-7\t3.035855E-7\r\n1.497349E+0\t2.458624E-7\t4.010542E-7\t6.477048E-7\t1.035653E-6\t1.639510E-6\t2.569669E-6\t3.987525E-6\t6.126219E-6\t9.318473E-6\t1.403331E-5\t2.092369E-5\t3.088728E-5\t4.514234E-5\t6.532080E-5\t9.357977E-5\t1.327320E-4\t1.863941E-4\t2.591503E-4\t3.567256E-4\t4.861608E-4\t6.559771E-4\t8.763155E-4\t1.159032E-3\t1.517725E-3\t1.967678E-3\t2.525678E-3\t3.209704E-3\t4.038453E-3\t5.030696E-3\t6.204463E-3\t7.576059E-3\t9.158946E-3\t1.096253E-2\t1.299089E-2\t1.524159E-2\t1.770454E-2\t2.036114E-2\t2.318369E-2\t2.613521E-2\t2.916974E-2\t3.223311E-2\t3.526426E-2\t3.819711E-2\t4.096275E-2\t4.349215E-2\t4.571889E-2\t4.758209E-2\t4.902915E-2\t5.001823E-2\t5.052022E-2\t5.052022E-2\t5.001823E-2\t4.902915E-2\t4.758209E-2\t4.571889E-2\t4.349215E-2\t4.096275E-2\t3.819711E-2\t3.526426E-2\t3.223311E-2\t2.916974E-2\t2.613521E-2\t2.318369E-2\t2.036114E-2\t1.770454E-2\t1.524159E-2\t1.299089E-2\t1.096253E-2\t9.158946E-3\t7.576059E-3\t6.204463E-3\t5.030696E-3\t4.038453E-3\t3.209704E-3\t2.525678E-3\t1.967678E-3\t1.517725E-3\t1.159032E-3\t8.763155E-4\t6.559771E-4\t4.861608E-4\t3.567256E-4\t2.591503E-4\t1.863941E-4\t1.327320E-4\t9.357977E-5\t6.532080E-5\t4.514234E-5\t3.088728E-5\t2.092369E-5\t1.403331E-5\t9.318473E-6\t6.126219E-6\t3.987525E-6\t2.569669E-6\t1.639510E-6\t1.035653E-6\t6.477048E-7\t4.010542E-7\t2.458624E-7\r\n1.542307E+0\t1.971240E-7\t3.215514E-7\t5.193072E-7\t8.303503E-7\t1.314502E-6\t2.060272E-6\t3.197059E-6\t4.911790E-6\t7.471229E-6\t1.125142E-5\t1.677589E-5\t2.476435E-5\t3.619356E-5\t5.237195E-5\t7.502901E-5\t1.064199E-4\t1.494443E-4\t2.077777E-4\t2.860102E-4\t3.897869E-4\t5.259397E-4\t7.025994E-4\t9.292714E-4\t1.216859E-3\t1.577616E-3\t2.025001E-3\t2.573429E-3\t3.237891E-3\t4.033437E-3\t4.974523E-3\t6.074221E-3\t7.343326E-3\t8.789376E-3\t1.041565E-2\t1.222018E-2\t1.419489E-2\t1.632486E-2\t1.858788E-2\t2.095431E-2\t2.338729E-2\t2.584339E-2\t2.827366E-2\t3.062511E-2\t3.284252E-2\t3.487050E-2\t3.665582E-2\t3.814967E-2\t3.930987E-2\t4.010288E-2\t4.050536E-2\t4.050536E-2\t4.010288E-2\t3.930987E-2\t3.814967E-2\t3.665582E-2\t3.487050E-2\t3.284252E-2\t3.062511E-2\t2.827366E-2\t2.584339E-2\t2.338729E-2\t2.095431E-2\t1.858788E-2\t1.632486E-2\t1.419489E-2\t1.222018E-2\t1.041565E-2\t8.789376E-3\t7.343326E-3\t6.074221E-3\t4.974523E-3\t4.033437E-3\t3.237891E-3\t2.573429E-3\t2.025001E-3\t1.577616E-3\t1.216859E-3\t9.292714E-4\t7.025994E-4\t5.259397E-4\t3.897869E-4\t2.860102E-4\t2.077777E-4\t1.494443E-4\t1.064199E-4\t7.502901E-5\t5.237195E-5\t3.619356E-5\t2.476435E-5\t1.677589E-5\t1.125142E-5\t7.471229E-6\t4.911790E-6\t3.197059E-6\t2.060272E-6\t1.314502E-6\t8.303503E-7\t5.193072E-7\t3.215514E-7\t1.971240E-7\r\n1.587265E+0\t1.564670E-7\t2.552312E-7\t4.121997E-7\t6.590900E-7\t1.043385E-6\t1.635339E-6\t2.537663E-6\t3.898730E-6\t5.930282E-6\t8.930806E-6\t1.331585E-5\t1.965669E-5\t2.872861E-5\t4.157020E-5\t5.955423E-5\t8.447070E-5\t1.186213E-4\t1.649234E-4\t2.270204E-4\t3.093931E-4\t4.174643E-4\t5.576877E-4\t7.376085E-4\t9.658813E-4\t1.252232E-3\t1.607343E-3\t2.042658E-3\t2.570074E-3\t3.201538E-3\t3.948524E-3\t4.821408E-3\t5.828759E-3\t6.976560E-3\t8.267413E-3\t9.699759E-3\t1.126718E-2\t1.295784E-2\t1.475412E-2\t1.663247E-2\t1.856364E-2\t2.051317E-2\t2.244220E-2\t2.430866E-2\t2.606872E-2\t2.767843E-2\t2.909553E-2\t3.028127E-2\t3.120218E-2\t3.183163E-2\t3.215110E-2\t3.215110E-2\t3.183163E-2\t3.120218E-2\t3.028127E-2\t2.909553E-2\t2.767843E-2\t2.606872E-2\t2.430866E-2\t2.244220E-2\t2.051317E-2\t1.856364E-2\t1.663247E-2\t1.475412E-2\t1.295784E-2\t1.126718E-2\t9.699759E-3\t8.267413E-3\t6.976560E-3\t5.828759E-3\t4.821408E-3\t3.948524E-3\t3.201538E-3\t2.570074E-3\t2.042658E-3\t1.607343E-3\t1.252232E-3\t9.658813E-4\t7.376085E-4\t5.576877E-4\t4.174643E-4\t3.093931E-4\t2.270204E-4\t1.649234E-4\t1.186213E-4\t8.447070E-5\t5.955423E-5\t4.157020E-5\t2.872861E-5\t1.965669E-5\t1.331585E-5\t8.930806E-6\t5.930282E-6\t3.898730E-6\t2.537663E-6\t1.635339E-6\t1.043385E-6\t6.590900E-7\t4.121997E-7\t2.552312E-7\t1.564670E-7\r\n1.632222E+0\t1.229539E-7\t2.005641E-7\t3.239121E-7\t5.179217E-7\t8.199062E-7\t1.285071E-6\t1.994130E-6\t3.063674E-6\t4.660095E-6\t7.017946E-6\t1.046377E-5\t1.544649E-5\t2.257533E-5\t3.266642E-5\t4.679851E-5\t6.637821E-5\t9.321420E-5\t1.295990E-4\t1.783957E-4\t2.431252E-4\t3.280490E-4\t4.382385E-4\t5.796226E-4\t7.590024E-4\t9.840203E-4\t1.263072E-3\t1.605148E-3\t2.019598E-3\t2.515811E-3\t3.102803E-3\t3.788727E-3\t4.580317E-3\t5.482274E-3\t6.496644E-3\t7.622201E-3\t8.853903E-3\t1.018245E-2\t1.159398E-2\t1.307001E-2\t1.458756E-2\t1.611952E-2\t1.763538E-2\t1.910207E-2\t2.048515E-2\t2.175008E-2\t2.286366E-2\t2.379543E-2\t2.451909E-2\t2.501372E-2\t2.526477E-2\t2.526477E-2\t2.501372E-2\t2.451909E-2\t2.379543E-2\t2.286366E-2\t2.175008E-2\t2.048515E-2\t1.910207E-2\t1.763538E-2\t1.611952E-2\t1.458756E-2\t1.307001E-2\t1.159398E-2\t1.018245E-2\t8.853903E-3\t7.622201E-3\t6.496644E-3\t5.482274E-3\t4.580317E-3\t3.788727E-3\t3.102803E-3\t2.515811E-3\t2.019598E-3\t1.605148E-3\t1.263072E-3\t9.840203E-4\t7.590024E-4\t5.796226E-4\t4.382385E-4\t3.280490E-4\t2.431252E-4\t1.783957E-4\t1.295990E-4\t9.321420E-5\t6.637821E-5\t4.679851E-5\t3.266642E-5\t2.257533E-5\t1.544649E-5\t1.046377E-5\t7.017946E-6\t4.660095E-6\t3.063674E-6\t1.994130E-6\t1.285071E-6\t8.199062E-7\t5.179217E-7\t3.239121E-7\t2.005641E-7\t1.229539E-7\r\n1.677180E+0\t9.565280E-8\t1.560302E-7\t2.519896E-7\t4.029207E-7\t6.378516E-7\t9.997300E-7\t1.551347E-6\t2.383406E-6\t3.625353E-6\t5.459659E-6\t8.140364E-6\t1.201670E-5\t1.756263E-5\t2.541306E-5\t3.640722E-5\t5.163938E-5\t7.251662E-5\t1.008224E-4\t1.387841E-4\t1.891409E-4\t2.552080E-4\t3.409306E-4\t4.509213E-4\t5.904711E-4\t7.655253E-4\t9.826152E-4\t1.248736E-3\t1.571160E-3\t1.957193E-3\t2.413847E-3\t2.947466E-3\t3.563289E-3\t4.264973E-3\t5.054108E-3\t5.929743E-3\t6.887954E-3\t7.921504E-3\t9.019617E-3\t1.016791E-2\t1.134849E-2\t1.254029E-2\t1.371956E-2\t1.486059E-2\t1.593656E-2\t1.692063E-2\t1.778694E-2\t1.851182E-2\t1.907480E-2\t1.945960E-2\t1.965490E-2\t1.965490E-2\t1.945960E-2\t1.907480E-2\t1.851182E-2\t1.778694E-2\t1.692063E-2\t1.593656E-2\t1.486059E-2\t1.371956E-2\t1.254029E-2\t1.134849E-2\t1.016791E-2\t9.019617E-3\t7.921504E-3\t6.887954E-3\t5.929743E-3\t5.054108E-3\t4.264973E-3\t3.563289E-3\t2.947466E-3\t2.413847E-3\t1.957193E-3\t1.571160E-3\t1.248736E-3\t9.826152E-4\t7.655253E-4\t5.904711E-4\t4.509213E-4\t3.409306E-4\t2.552080E-4\t1.891409E-4\t1.387841E-4\t1.008224E-4\t7.251662E-5\t5.163938E-5\t3.640722E-5\t2.541306E-5\t1.756263E-5\t1.201670E-5\t8.140364E-6\t5.459659E-6\t3.625353E-6\t2.383406E-6\t1.551347E-6\t9.997300E-7\t6.378516E-7\t4.029207E-7\t2.519896E-7\t1.560302E-7\t9.565280E-8\r\n1.722138E+0\t7.366976E-8\t1.201711E-7\t1.940770E-7\t3.103210E-7\t4.912598E-7\t7.699709E-7\t1.194814E-6\t1.835649E-6\t2.792170E-6\t4.204914E-6\t6.269536E-6\t9.255007E-6\t1.352637E-5\t1.957260E-5\t2.804007E-5\t3.977155E-5\t5.585076E-5\t7.765130E-5\t1.068886E-4\t1.456723E-4\t1.965558E-4\t2.625775E-4\t3.472901E-4\t4.547683E-4\t5.895914E-4\t7.567894E-4\t9.617496E-4\t1.210074E-3\t1.507388E-3\t1.859093E-3\t2.270076E-3\t2.744369E-3\t3.284792E-3\t3.892567E-3\t4.566962E-3\t5.304956E-3\t6.100974E-3\t6.946717E-3\t7.831106E-3\t8.740367E-3\t9.658268E-3\t1.056652E-2\t1.144531E-2\t1.227400E-2\t1.303191E-2\t1.369912E-2\t1.425741E-2\t1.469100E-2\t1.498737E-2\t1.513778E-2\t1.513778E-2\t1.498737E-2\t1.469100E-2\t1.425741E-2\t1.369912E-2\t1.303191E-2\t1.227400E-2\t1.144531E-2\t1.056652E-2\t9.658268E-3\t8.740367E-3\t7.831106E-3\t6.946717E-3\t6.100974E-3\t5.304956E-3\t4.566962E-3\t3.892567E-3\t3.284792E-3\t2.744369E-3\t2.270076E-3\t1.859093E-3\t1.507388E-3\t1.210074E-3\t9.617496E-4\t7.567894E-4\t5.895914E-4\t4.547683E-4\t3.472901E-4\t2.625775E-4\t1.965558E-4\t1.456723E-4\t1.068886E-4\t7.765130E-5\t5.585076E-5\t3.977155E-5\t2.804007E-5\t1.957260E-5\t1.352637E-5\t9.255007E-6\t6.269536E-6\t4.204914E-6\t2.792170E-6\t1.835649E-6\t1.194814E-6\t7.699709E-7\t4.912598E-7\t3.103210E-7\t1.940770E-7\t1.201711E-7\t7.366976E-8\r\n1.767096E+0\t5.617161E-8\t9.162792E-8\t1.479796E-7\t2.366131E-7\t3.745750E-7\t5.870863E-7\t9.110203E-7\t1.399643E-6\t2.128970E-6\t3.206156E-6\t4.780387E-6\t7.056744E-6\t1.031356E-5\t1.492369E-5\t2.137995E-5\t3.032496E-5\t4.258501E-5\t5.920745E-5\t8.150026E-5\t1.110720E-4\t1.498695E-4\t2.002097E-4\t2.648012E-4\t3.467511E-4\t4.495508E-4\t5.770357E-4\t7.333135E-4\t9.226557E-4\t1.149351E-3\t1.417519E-3\t1.730884E-3\t2.092523E-3\t2.504583E-3\t2.967999E-3\t3.482211E-3\t4.044915E-3\t4.651862E-3\t5.296723E-3\t5.971051E-3\t6.664342E-3\t7.364222E-3\t8.056742E-3\t8.726802E-3\t9.358664E-3\t9.936549E-3\t1.044529E-2\t1.087097E-2\t1.120157E-2\t1.142755E-2\t1.154224E-2\t1.154224E-2\t1.142755E-2\t1.120157E-2\t1.087097E-2\t1.044529E-2\t9.936549E-3\t9.358664E-3\t8.726802E-3\t8.056742E-3\t7.364222E-3\t6.664342E-3\t5.971051E-3\t5.296723E-3\t4.651862E-3\t4.044915E-3\t3.482211E-3\t2.967999E-3\t2.504583E-3\t2.092523E-3\t1.730884E-3\t1.417519E-3\t1.149351E-3\t9.226557E-4\t7.333135E-4\t5.770357E-4\t4.495508E-4\t3.467511E-4\t2.648012E-4\t2.002097E-4\t1.498695E-4\t1.110720E-4\t8.150026E-5\t5.920745E-5\t4.258501E-5\t3.032496E-5\t2.137995E-5\t1.492369E-5\t1.031356E-5\t7.056744E-6\t4.780387E-6\t3.206156E-6\t2.128970E-6\t1.399643E-6\t9.110203E-7\t5.870863E-7\t3.745750E-7\t2.366131E-7\t1.479796E-7\t9.162792E-8\t5.617161E-8\r\n1.812053E+0\t4.240144E-8\t6.916582E-8\t1.117032E-7\t1.786086E-7\t2.827499E-7\t4.431652E-7\t6.876885E-7\t1.056528E-6\t1.607064E-6\t2.420184E-6\t3.608500E-6\t5.326821E-6\t7.785248E-6\t1.126523E-5\t1.613877E-5\t2.289095E-5\t3.214552E-5\t4.469305E-5\t6.152090E-5\t8.384330E-5\t1.131298E-4\t1.511294E-4\t1.998866E-4\t2.617469E-4\t3.393458E-4\t4.355784E-4\t5.535455E-4\t6.964715E-4\t8.675938E-4\t1.070022E-3\t1.306567E-3\t1.579552E-3\t1.890598E-3\t2.240410E-3\t2.628565E-3\t3.053325E-3\t3.511483E-3\t3.998259E-3\t4.507279E-3\t5.030614E-3\t5.558922E-3\t6.081675E-3\t6.587473E-3\t7.064437E-3\t7.500657E-3\t7.884680E-3\t8.206007E-3\t8.455568E-3\t8.626144E-3\t8.712718E-3\t8.712718E-3\t8.626144E-3\t8.455568E-3\t8.206007E-3\t7.884680E-3\t7.500657E-3\t7.064437E-3\t6.587473E-3\t6.081675E-3\t5.558922E-3\t5.030614E-3\t4.507279E-3\t3.998259E-3\t3.511483E-3\t3.053325E-3\t2.628565E-3\t2.240410E-3\t1.890598E-3\t1.579552E-3\t1.306567E-3\t1.070022E-3\t8.675938E-4\t6.964715E-4\t5.535455E-4\t4.355784E-4\t3.393458E-4\t2.617469E-4\t1.998866E-4\t1.511294E-4\t1.131298E-4\t8.384330E-5\t6.152090E-5\t4.469305E-5\t3.214552E-5\t2.289095E-5\t1.613877E-5\t1.126523E-5\t7.785248E-6\t5.326821E-6\t3.608500E-6\t2.420184E-6\t1.607064E-6\t1.056528E-6\t6.876885E-7\t4.431652E-7\t2.827499E-7\t1.786086E-7\t1.117032E-7\t6.916582E-8\t4.240144E-8\r\n1.857011E+0\t3.168694E-8\t5.168818E-8\t8.347669E-8\t1.334757E-7\t2.113014E-7\t3.311810E-7\t5.139153E-7\t7.895519E-7\t1.200972E-6\t1.808624E-6\t2.696662E-6\t3.980777E-6\t5.817980E-6\t8.418596E-6\t1.206063E-5\t1.710660E-5\t2.402261E-5\t3.339949E-5\t4.597508E-5\t6.265679E-5\t8.454285E-5\t1.129402E-4\t1.493769E-4\t1.956056E-4\t2.535959E-4\t3.255114E-4\t4.136691E-4\t5.204789E-4\t6.483600E-4\t7.996360E-4\t9.764083E-4\t1.180412E-3\t1.412859E-3\t1.674277E-3\t1.964348E-3\t2.281775E-3\t2.624160E-3\t2.987932E-3\t3.368327E-3\t3.759419E-3\t4.154228E-3\t4.544886E-3\t4.922873E-3\t5.279312E-3\t5.605303E-3\t5.892286E-3\t6.132417E-3\t6.318916E-3\t6.446388E-3\t6.511086E-3\t6.511086E-3\t6.446388E-3\t6.318916E-3\t6.132417E-3\t5.892286E-3\t5.605303E-3\t5.279312E-3\t4.922873E-3\t4.544886E-3\t4.154228E-3\t3.759419E-3\t3.368327E-3\t2.987932E-3\t2.624160E-3\t2.281775E-3\t1.964348E-3\t1.674277E-3\t1.412859E-3\t1.180412E-3\t9.764083E-4\t7.996360E-4\t6.483600E-4\t5.204789E-4\t4.136691E-4\t3.255114E-4\t2.535959E-4\t1.956056E-4\t1.493769E-4\t1.129402E-4\t8.454285E-5\t6.265679E-5\t4.597508E-5\t3.339949E-5\t2.402261E-5\t1.710660E-5\t1.206063E-5\t8.418596E-6\t5.817980E-6\t3.980777E-6\t2.696662E-6\t1.808624E-6\t1.200972E-6\t7.895519E-7\t5.139153E-7\t3.311810E-7\t2.113014E-7\t1.334757E-7\t8.347669E-8\t5.168818E-8\t3.168694E-8\r\n1.901969E+0\t2.344316E-8\t3.824081E-8\t6.175912E-8\t9.875023E-8\t1.563285E-7\t2.450198E-7\t3.802134E-7\t5.841395E-7\t8.885232E-7\t1.338086E-6\t1.995089E-6\t2.945125E-6\t4.304355E-6\t6.228386E-6\t8.922899E-6\t1.265609E-5\t1.777281E-5\t2.471017E-5\t3.401405E-5\t4.635579E-5\t6.254790E-5\t8.355732E-5\t1.105145E-4\t1.447162E-4\t1.876195E-4\t2.408252E-4\t3.060476E-4\t3.850694E-4\t4.796805E-4\t5.916000E-4\t7.223827E-4\t8.733122E-4\t1.045285E-3\t1.238691E-3\t1.453297E-3\t1.688141E-3\t1.941450E-3\t2.210582E-3\t2.492012E-3\t2.781356E-3\t3.073450E-3\t3.362473E-3\t3.642122E-3\t3.905828E-3\t4.147008E-3\t4.359329E-3\t4.536987E-3\t4.674965E-3\t4.769274E-3\t4.817140E-3\t4.817140E-3\t4.769274E-3\t4.674965E-3\t4.536987E-3\t4.359329E-3\t4.147008E-3\t3.905828E-3\t3.642122E-3\t3.362473E-3\t3.073450E-3\t2.781356E-3\t2.492012E-3\t2.210582E-3\t1.941450E-3\t1.688141E-3\t1.453297E-3\t1.238691E-3\t1.045285E-3\t8.733122E-4\t7.223827E-4\t5.916000E-4\t4.796805E-4\t3.850694E-4\t3.060476E-4\t2.408252E-4\t1.876195E-4\t1.447162E-4\t1.105145E-4\t8.355732E-5\t6.254790E-5\t4.635579E-5\t3.401405E-5\t2.471017E-5\t1.777281E-5\t1.265609E-5\t8.922899E-6\t6.228386E-6\t4.304355E-6\t2.945125E-6\t1.995089E-6\t1.338086E-6\t8.885232E-7\t5.841395E-7\t3.802134E-7\t2.450198E-7\t1.563285E-7\t9.875023E-8\t6.175912E-8\t3.824081E-8\t2.344316E-8\r\n1.946927E+0\t1.717070E-8\t2.800909E-8\t4.523483E-8\t7.232859E-8\t1.145012E-7\t1.794623E-7\t2.784834E-7\t4.278470E-7\t6.507897E-7\t9.800674E-7\t1.461283E-6\t2.157126E-6\t3.152681E-6\t4.561917E-6\t6.535486E-6\t9.269822E-6\t1.301751E-5\t1.809871E-5\t2.491324E-5\t3.395282E-5\t4.581257E-5\t6.120070E-5\t8.094522E-5\t1.059959E-4\t1.374200E-4\t1.763900E-4\t2.241614E-4\t2.820401E-4\t3.513371E-4\t4.333114E-4\t5.291018E-4\t6.396486E-4\t7.656084E-4\t9.072667E-4\t1.064452E-3\t1.236462E-3\t1.421995E-3\t1.619118E-3\t1.825248E-3\t2.037176E-3\t2.251117E-3\t2.462809E-3\t2.667635E-3\t2.860784E-3\t3.037434E-3\t3.192946E-3\t3.323070E-3\t3.424131E-3\t3.493206E-3\t3.528265E-3\t3.528265E-3\t3.493206E-3\t3.424131E-3\t3.323070E-3\t3.192946E-3\t3.037434E-3\t2.860784E-3\t2.667635E-3\t2.462809E-3\t2.251117E-3\t2.037176E-3\t1.825248E-3\t1.619118E-3\t1.421995E-3\t1.236462E-3\t1.064452E-3\t9.072667E-4\t7.656084E-4\t6.396486E-4\t5.291018E-4\t4.333114E-4\t3.513371E-4\t2.820401E-4\t2.241614E-4\t1.763900E-4\t1.374200E-4\t1.059959E-4\t8.094522E-5\t6.120070E-5\t4.581257E-5\t3.395282E-5\t2.491324E-5\t1.809871E-5\t1.301751E-5\t9.269822E-6\t6.535486E-6\t4.561917E-6\t3.152681E-6\t2.157126E-6\t1.461283E-6\t9.800674E-7\t6.507897E-7\t4.278470E-7\t2.784834E-7\t1.794623E-7\t1.145012E-7\t7.232859E-8\t4.523483E-8\t2.800909E-8\t1.717070E-8\r\n1.991884E+0\t1.245077E-8\t2.030986E-8\t3.280054E-8\t5.244668E-8\t8.302675E-8\t1.301311E-7\t2.019330E-7\t3.102390E-7\t4.718986E-7\t7.106634E-7\t1.059601E-6\t1.564169E-6\t2.286062E-6\t3.307923E-6\t4.738991E-6\t6.721704E-6\t9.439217E-6\t1.312368E-5\t1.806501E-5\t2.461976E-5\t3.321946E-5\t4.437766E-5\t5.869474E-5\t7.685941E-5\t9.964556E-5\t1.279033E-4\t1.625432E-4\t2.045120E-4\t2.547604E-4\t3.142014E-4\t3.836606E-4\t4.638199E-4\t5.551555E-4\t6.578743E-4\t7.718524E-4\t8.965791E-4\t1.031112E-3\t1.174050E-3\t1.323518E-3\t1.477190E-3\t1.632323E-3\t1.785824E-3\t1.934347E-3\t2.074403E-3\t2.202494E-3\t2.315259E-3\t2.409614E-3\t2.482895E-3\t2.532983E-3\t2.558404E-3\t2.558404E-3\t2.532983E-3\t2.482895E-3\t2.409614E-3\t2.315259E-3\t2.202494E-3\t2.074403E-3\t1.934347E-3\t1.785824E-3\t1.632323E-3\t1.477190E-3\t1.323518E-3\t1.174050E-3\t1.031112E-3\t8.965791E-4\t7.718524E-4\t6.578743E-4\t5.551555E-4\t4.638199E-4\t3.836606E-4\t3.142014E-4\t2.547604E-4\t2.045120E-4\t1.625432E-4\t1.279033E-4\t9.964556E-5\t7.685941E-5\t5.869474E-5\t4.437766E-5\t3.321946E-5\t2.461976E-5\t1.806501E-5\t1.312368E-5\t9.439217E-6\t6.721704E-6\t4.738991E-6\t3.307923E-6\t2.286062E-6\t1.564169E-6\t1.059601E-6\t7.106634E-7\t4.718986E-7\t3.102390E-7\t2.019330E-7\t1.301311E-7\t8.302675E-8\t5.244668E-8\t3.280054E-8\t2.030986E-8\t1.245077E-8\r\n2.036842E+0\t8.937996E-9\t1.457978E-8\t2.354643E-8\t3.764975E-8\t5.960217E-8\t9.341685E-8\t1.449611E-7\t2.227104E-7\t3.387605E-7\t5.101619E-7\t7.606525E-7\t1.122865E-6\t1.641089E-6\t2.374649E-6\t3.401966E-6\t4.825290E-6\t6.776103E-6\t9.421057E-6\t1.296828E-5\t1.767372E-5\t2.384716E-5\t3.185726E-5\t4.213502E-5\t5.517484E-5\t7.153227E-5\t9.181760E-5\t1.166844E-4\t1.468125E-4\t1.828841E-4\t2.255548E-4\t2.754173E-4\t3.329611E-4\t3.985279E-4\t4.722663E-4\t5.540875E-4\t6.436247E-4\t7.402017E-4\t8.428117E-4\t9.501103E-4\t1.060426E-3\t1.171791E-3\t1.281984E-3\t1.388604E-3\t1.489145E-3\t1.581098E-3\t1.662048E-3\t1.729782E-3\t1.782388E-3\t1.818345E-3\t1.836594E-3\t1.836594E-3\t1.818345E-3\t1.782388E-3\t1.729782E-3\t1.662048E-3\t1.581098E-3\t1.489145E-3\t1.388604E-3\t1.281984E-3\t1.171791E-3\t1.060426E-3\t9.501103E-4\t8.428117E-4\t7.402017E-4\t6.436247E-4\t5.540875E-4\t4.722663E-4\t3.985279E-4\t3.329611E-4\t2.754173E-4\t2.255548E-4\t1.828841E-4\t1.468125E-4\t1.166844E-4\t9.181760E-5\t7.153227E-5\t5.517484E-5\t4.213502E-5\t3.185726E-5\t2.384716E-5\t1.767372E-5\t1.296828E-5\t9.421057E-6\t6.776103E-6\t4.825290E-6\t3.401966E-6\t2.374649E-6\t1.641089E-6\t1.122865E-6\t7.606525E-7\t5.101619E-7\t3.387605E-7\t2.227104E-7\t1.449611E-7\t9.341685E-8\t5.960217E-8\t3.764975E-8\t2.354643E-8\t1.457978E-8\t8.937996E-9\r\n2.081800E+0\t6.352143E-9\t1.036170E-8\t1.673421E-8\t2.675729E-8\t4.235866E-8\t6.639041E-8\t1.030224E-7\t1.582780E-7\t2.407536E-7\t3.625669E-7\t5.405880E-7\t7.980090E-7\t1.166305E-6\t1.687639E-6\t2.417743E-6\t3.429285E-6\t4.815708E-6\t6.695450E-6\t9.216423E-6\t1.256053E-5\t1.694794E-5\t2.264063E-5\t2.994494E-5\t3.921220E-5\t5.083726E-5\t6.525384E-5\t8.292645E-5\t1.043381E-4\t1.299739E-4\t1.602995E-4\t1.957363E-4\t2.366321E-4\t2.832297E-4\t3.356349E-4\t3.937843E-4\t4.574175E-4\t5.260539E-4\t5.989777E-4\t6.752338E-4\t7.536344E-4\t8.327800E-4\t9.110934E-4\t9.868668E-4\t1.058321E-3\t1.123671E-3\t1.181201E-3\t1.229339E-3\t1.266725E-3\t1.292279E-3\t1.305249E-3\t1.305249E-3\t1.292279E-3\t1.266725E-3\t1.229339E-3\t1.181201E-3\t1.123671E-3\t1.058321E-3\t9.868668E-4\t9.110934E-4\t8.327800E-4\t7.536344E-4\t6.752338E-4\t5.989777E-4\t5.260539E-4\t4.574175E-4\t3.937843E-4\t3.356349E-4\t2.832297E-4\t2.366321E-4\t1.957363E-4\t1.602995E-4\t1.299739E-4\t1.043381E-4\t8.292645E-5\t6.525384E-5\t5.083726E-5\t3.921220E-5\t2.994494E-5\t2.264063E-5\t1.694794E-5\t1.256053E-5\t9.216423E-6\t6.695450E-6\t4.815708E-6\t3.429285E-6\t2.417743E-6\t1.687639E-6\t1.166305E-6\t7.980090E-7\t5.405880E-7\t3.625669E-7\t2.407536E-7\t1.582780E-7\t1.030224E-7\t6.639041E-8\t4.235866E-8\t2.675729E-8\t1.673421E-8\t1.036170E-8\t6.352143E-9\r\n2.126758E+0\t4.469269E-9\t7.290334E-9\t1.177393E-8\t1.882601E-8\t2.980289E-8\t4.671125E-8\t7.248492E-8\t1.113620E-7\t1.693905E-7\t2.550964E-7\t3.803493E-7\t5.614667E-7\t8.205941E-7\t1.187397E-6\t1.701086E-6\t2.412791E-6\t3.388257E-6\t4.710814E-6\t6.484531E-6\t8.837395E-6\t1.192430E-5\t1.592960E-5\t2.106879E-5\t2.758909E-5\t3.576830E-5\t4.591158E-5\t5.834575E-5\t7.341069E-5\t9.144761E-5\t1.127843E-4\t1.377170E-4\t1.664906E-4\t1.992760E-4\t2.361475E-4\t2.770605E-4\t3.218318E-4\t3.701233E-4\t4.214314E-4\t4.750840E-4\t5.302454E-4\t5.859310E-4\t6.410311E-4\t6.943441E-4\t7.446179E-4\t7.905971E-4\t8.310746E-4\t8.649437E-4\t8.912482E-4\t9.092276E-4\t9.183528E-4\t9.183528E-4\t9.092276E-4\t8.912482E-4\t8.649437E-4\t8.310746E-4\t7.905971E-4\t7.446179E-4\t6.943441E-4\t6.410311E-4\t5.859310E-4\t5.302454E-4\t4.750840E-4\t4.214314E-4\t3.701233E-4\t3.218318E-4\t2.770605E-4\t2.361475E-4\t1.992760E-4\t1.664906E-4\t1.377170E-4\t1.127843E-4\t9.144761E-5\t7.341069E-5\t5.834575E-5\t4.591158E-5\t3.576830E-5\t2.758909E-5\t2.106879E-5\t1.592960E-5\t1.192430E-5\t8.837395E-6\t6.484531E-6\t4.710814E-6\t3.388257E-6\t2.412791E-6\t1.701086E-6\t1.187397E-6\t8.205941E-7\t5.614667E-7\t3.803493E-7\t2.550964E-7\t1.693905E-7\t1.113620E-7\t7.248492E-8\t4.671125E-8\t2.980289E-8\t1.882601E-8\t1.177393E-8\t7.290334E-9\t4.469269E-9\r\n2.171716E+0\t3.113069E-9\t5.078082E-9\t8.201129E-9\t1.311326E-8\t2.075920E-8\t3.253672E-8\t5.048937E-8\t7.756917E-8\t1.179890E-7\t1.776874E-7\t2.649323E-7\t3.910896E-7\t5.715848E-7\t8.270811E-7\t1.184891E-6\t1.680630E-6\t2.360090E-6\t3.281317E-6\t4.516800E-6\t6.155687E-6\t8.305873E-6\t1.109576E-5\t1.467546E-5\t1.921718E-5\t2.491441E-5\t3.197971E-5\t4.064073E-5\t5.113421E-5\t6.369783E-5\t7.855987E-5\t9.592679E-5\t1.159690E-4\t1.388057E-4\t1.644885E-4\t1.929865E-4\t2.241720E-4\t2.578094E-4\t2.935480E-4\t3.309197E-4\t3.693424E-4\t4.081302E-4\t4.465102E-4\t4.836454E-4\t5.186635E-4\t5.506904E-4\t5.788850E-4\t6.024765E-4\t6.207989E-4\t6.333224E-4\t6.396786E-4\t6.396786E-4\t6.333224E-4\t6.207989E-4\t6.024765E-4\t5.788850E-4\t5.506904E-4\t5.186635E-4\t4.836454E-4\t4.465102E-4\t4.081302E-4\t3.693424E-4\t3.309197E-4\t2.935480E-4\t2.578094E-4\t2.241720E-4\t1.929865E-4\t1.644885E-4\t1.388057E-4\t1.159690E-4\t9.592679E-5\t7.855987E-5\t6.369783E-5\t5.113421E-5\t4.064073E-5\t3.197971E-5\t2.491441E-5\t1.921718E-5\t1.467546E-5\t1.109576E-5\t8.305873E-6\t6.155687E-6\t4.516800E-6\t3.281317E-6\t2.360090E-6\t1.680630E-6\t1.184891E-6\t8.270811E-7\t5.715848E-7\t3.910896E-7\t2.649323E-7\t1.776874E-7\t1.179890E-7\t7.756917E-8\t5.048937E-8\t3.253672E-8\t2.075920E-8\t1.311326E-8\t8.201129E-9\t5.078082E-9\t3.113069E-9\r\n2.216673E+0\t2.146728E-9\t3.501773E-9\t5.655383E-9\t9.042718E-9\t1.431525E-8\t2.243686E-8\t3.481675E-8\t5.349060E-8\t8.136351E-8\t1.225307E-7\t1.826936E-7\t2.696898E-7\t3.941568E-7\t5.703434E-7\t8.170843E-7\t1.158939E-6\t1.627485E-6\t2.262750E-6\t3.114721E-6\t4.244875E-6\t5.727612E-6\t7.651479E-6\t1.011999E-5\t1.325190E-5\t1.718063E-5\t2.205276E-5\t2.802528E-5\t3.526143E-5\t4.392512E-5\t5.417377E-5\t6.614975E-5\t7.997061E-5\t9.571845E-5\t1.134290E-4\t1.330808E-4\t1.545858E-4\t1.777817E-4\t2.024266E-4\t2.281976E-4\t2.546933E-4\t2.814408E-4\t3.079071E-4\t3.335150E-4\t3.576630E-4\t3.797483E-4\t3.991909E-4\t4.154593E-4\t4.280942E-4\t4.367302E-4\t4.411133E-4\t4.411133E-4\t4.367302E-4\t4.280942E-4\t4.154593E-4\t3.991909E-4\t3.797483E-4\t3.576630E-4\t3.335150E-4\t3.079071E-4\t2.814408E-4\t2.546933E-4\t2.281976E-4\t2.024266E-4\t1.777817E-4\t1.545858E-4\t1.330808E-4\t1.134290E-4\t9.571845E-5\t7.997061E-5\t6.614975E-5\t5.417377E-5\t4.392512E-5\t3.526143E-5\t2.802528E-5\t2.205276E-5\t1.718063E-5\t1.325190E-5\t1.011999E-5\t7.651479E-6\t5.727612E-6\t4.244875E-6\t3.114721E-6\t2.262750E-6\t1.627485E-6\t1.158939E-6\t8.170843E-7\t5.703434E-7\t3.941568E-7\t2.696898E-7\t1.826936E-7\t1.225307E-7\t8.136351E-8\t5.349060E-8\t3.481675E-8\t2.243686E-8\t1.431525E-8\t9.042718E-9\t5.655383E-9\t3.501773E-9\t2.146728E-9\r\n2.261631E+0\t1.465553E-9\t2.390631E-9\t3.860881E-9\t6.173386E-9\t9.772901E-9\t1.531745E-8\t2.376910E-8\t3.651757E-8\t5.554617E-8\t8.365066E-8\t1.247233E-7\t1.841149E-7\t2.690874E-7\t3.893685E-7\t5.578164E-7\t7.911974E-7\t1.111070E-6\t1.544760E-6\t2.126393E-6\t2.897939E-6\t3.910192E-6\t5.223599E-6\t6.908832E-6\t9.046956E-6\t1.172906E-5\t1.505523E-5\t1.913261E-5\t2.407267E-5\t2.998730E-5\t3.698397E-5\t4.515987E-5\t5.459525E-5\t6.534616E-5\t7.743697E-5\t9.085309E-5\t1.055344E-4\t1.213700E-4\t1.381949E-4\t1.557885E-4\t1.738769E-4\t1.921372E-4\t2.102055E-4\t2.276878E-4\t2.441735E-4\t2.592509E-4\t2.725242E-4\t2.836305E-4\t2.922562E-4\t2.981519E-4\t3.011443E-4\t3.011443E-4\t2.981519E-4\t2.922562E-4\t2.836305E-4\t2.725242E-4\t2.592509E-4\t2.441735E-4\t2.276878E-4\t2.102055E-4\t1.921372E-4\t1.738769E-4\t1.557885E-4\t1.381949E-4\t1.213700E-4\t1.055344E-4\t9.085309E-5\t7.743697E-5\t6.534616E-5\t5.459525E-5\t4.515987E-5\t3.698397E-5\t2.998730E-5\t2.407267E-5\t1.913261E-5\t1.505523E-5\t1.172906E-5\t9.046956E-6\t6.908832E-6\t5.223599E-6\t3.910192E-6\t2.897939E-6\t2.126393E-6\t1.544760E-6\t1.111070E-6\t7.911974E-7\t5.578164E-7\t3.893685E-7\t2.690874E-7\t1.841149E-7\t1.247233E-7\t8.365066E-8\t5.554617E-8\t3.651757E-8\t2.376910E-8\t1.531745E-8\t9.772901E-9\t6.173386E-9\t3.860881E-9\t2.390631E-9\t1.465553E-9\r\n2.306589E+0\t9.905172E-10\t1.615745E-9\t2.609438E-9\t4.172381E-9\t6.605170E-9\t1.035254E-8\t1.606472E-8\t2.468098E-8\t3.754176E-8\t5.653662E-8\t8.429623E-8\t1.244370E-7\t1.818670E-7\t2.631609E-7\t3.770091E-7\t5.347433E-7\t7.509342E-7\t1.044050E-6\t1.437157E-6\t1.958618E-6\t2.642765E-6\t3.530452E-6\t4.669443E-6\t6.114528E-6\t7.927274E-6\t1.017531E-5\t1.293108E-5\t1.626990E-5\t2.026739E-5\t2.499620E-5\t3.052201E-5\t3.689906E-5\t4.416524E-5\t5.233700E-5\t6.140450E-5\t7.132710E-5\t8.202986E-5\t9.340119E-5\t1.052921E-4\t1.175175E-4\t1.298590E-4\t1.420707E-4\t1.538864E-4\t1.650285E-4\t1.752188E-4\t1.841898E-4\t1.916961E-4\t1.975260E-4\t2.015107E-4\t2.035331E-4\t2.035331E-4\t2.015107E-4\t1.975260E-4\t1.916961E-4\t1.841898E-4\t1.752188E-4\t1.650285E-4\t1.538864E-4\t1.420707E-4\t1.298590E-4\t1.175175E-4\t1.052921E-4\t9.340119E-5\t8.202986E-5\t7.132710E-5\t6.140450E-5\t5.233700E-5\t4.416524E-5\t3.689906E-5\t3.052201E-5\t2.499620E-5\t2.026739E-5\t1.626990E-5\t1.293108E-5\t1.017531E-5\t7.927274E-6\t6.114528E-6\t4.669443E-6\t3.530452E-6\t2.642765E-6\t1.958618E-6\t1.437157E-6\t1.044050E-6\t7.509342E-7\t5.347433E-7\t3.770091E-7\t2.631609E-7\t1.818670E-7\t1.244370E-7\t8.429623E-8\t5.653662E-8\t3.754176E-8\t2.468098E-8\t1.606472E-8\t1.035254E-8\t6.605170E-9\t4.172381E-9\t2.609438E-9\t1.615745E-9\t9.905172E-10\r\n2.351547E+0\t6.627635E-10\t1.081109E-9\t1.745997E-9\t2.791775E-9\t4.419575E-9\t6.926975E-9\t1.074904E-8\t1.651425E-8\t2.511951E-8\t3.782914E-8\t5.640333E-8\t8.326185E-8\t1.216888E-7\t1.760832E-7\t2.522600E-7\t3.578013E-7\t5.024565E-7\t6.985830E-7\t9.616138E-7\t1.310528E-6\t1.768297E-6\t2.362255E-6\t3.124364E-6\t4.091283E-6\t5.304207E-6\t6.808389E-6\t8.652296E-6\t1.088633E-5\t1.356109E-5\t1.672517E-5\t2.042254E-5\t2.468948E-5\t2.955134E-5\t3.501914E-5\t4.108627E-5\t4.772557E-5\t5.488688E-5\t6.249553E-5\t7.045186E-5\t7.863194E-5\t8.688975E-5\t9.506074E-5\t1.029667E-4\t1.104220E-4\t1.172404E-4\t1.232429E-4\t1.282655E-4\t1.321663E-4\t1.348325E-4\t1.361857E-4\t1.361857E-4\t1.348325E-4\t1.321663E-4\t1.282655E-4\t1.232429E-4\t1.172404E-4\t1.104220E-4\t1.029667E-4\t9.506074E-5\t8.688975E-5\t7.863194E-5\t7.045186E-5\t6.249553E-5\t5.488688E-5\t4.772557E-5\t4.108627E-5\t3.501914E-5\t2.955134E-5\t2.468948E-5\t2.042254E-5\t1.672517E-5\t1.356109E-5\t1.088633E-5\t8.652296E-6\t6.808389E-6\t5.304207E-6\t4.091283E-6\t3.124364E-6\t2.362255E-6\t1.768297E-6\t1.310528E-6\t9.616138E-7\t6.985830E-7\t5.024565E-7\t3.578013E-7\t2.522600E-7\t1.760832E-7\t1.216888E-7\t8.326185E-8\t5.640333E-8\t3.782914E-8\t2.511951E-8\t1.651425E-8\t1.074904E-8\t6.926975E-9\t4.419575E-9\t2.791775E-9\t1.745997E-9\t1.081109E-9\t6.627635E-10\r\n2.396504E+0\t4.390270E-10\t7.161469E-10\t1.156581E-9\t1.849324E-9\t2.927610E-9\t4.588558E-9\t7.120367E-9\t1.093935E-8\t1.663963E-8\t2.505873E-8\t3.736262E-8\t5.515421E-8\t8.060892E-8\t1.166408E-7\t1.671017E-7\t2.370143E-7\t3.328366E-7\t4.627545E-7\t6.369910E-7\t8.681185E-7\t1.171353E-6\t1.564802E-6\t2.069638E-6\t2.710143E-6\t3.513606E-6\t4.510005E-6\t5.731443E-6\t7.211307E-6\t8.983117E-6\t1.107907E-5\t1.352827E-5\t1.635477E-5\t1.957536E-5\t2.319733E-5\t2.721632E-5\t3.161431E-5\t3.635810E-5\t4.139821E-5\t4.666863E-5\t5.208727E-5\t5.755740E-5\t6.297002E-5\t6.820708E-5\t7.314559E-5\t7.766224E-5\t8.163844E-5\t8.496548E-5\t8.754945E-5\t8.931560E-5\t9.021199E-5\t9.021199E-5\t8.931560E-5\t8.754945E-5\t8.496548E-5\t8.163844E-5\t7.766224E-5\t7.314559E-5\t6.820708E-5\t6.297002E-5\t5.755740E-5\t5.208727E-5\t4.666863E-5\t4.139821E-5\t3.635810E-5\t3.161431E-5\t2.721632E-5\t2.319733E-5\t1.957536E-5\t1.635477E-5\t1.352827E-5\t1.107907E-5\t8.983117E-6\t7.211307E-6\t5.731443E-6\t4.510005E-6\t3.513606E-6\t2.710143E-6\t2.069638E-6\t1.564802E-6\t1.171353E-6\t8.681185E-7\t6.369910E-7\t4.627545E-7\t3.328366E-7\t2.370143E-7\t1.671017E-7\t1.166408E-7\t8.060892E-8\t5.515421E-8\t3.736262E-8\t2.505873E-8\t1.663963E-8\t1.093935E-8\t7.120367E-9\t4.588558E-9\t2.927610E-9\t1.849324E-9\t1.156581E-9\t7.161469E-10\t4.390270E-10\r\n2.441462E+0\t2.879121E-10\t4.696462E-10\t7.584812E-10\t1.212779E-9\t1.919914E-9\t3.009158E-9\t4.669508E-9\t7.173982E-9\t1.091220E-8\t1.643341E-8\t2.450226E-8\t3.616991E-8\t5.286300E-8\t7.649257E-8\t1.095846E-7\t1.554330E-7\t2.182729E-7\t3.034725E-7\t4.177361E-7\t5.693085E-7\t7.681684E-7\t1.026191E-6\t1.357260E-6\t1.777301E-6\t2.304208E-6\t2.957643E-6\t3.758657E-6\t4.729146E-6\t5.891092E-6\t7.265607E-6\t8.871786E-6\t1.072539E-5\t1.283744E-5\t1.521272E-5\t1.784835E-5\t2.073254E-5\t2.384349E-5\t2.714878E-5\t3.060510E-5\t3.415862E-5\t3.774591E-5\t4.129548E-5\t4.472993E-5\t4.796858E-5\t5.093058E-5\t5.353816E-5\t5.572002E-5\t5.741457E-5\t5.857281E-5\t5.916066E-5\t5.916066E-5\t5.857281E-5\t5.741457E-5\t5.572002E-5\t5.353816E-5\t5.093058E-5\t4.796858E-5\t4.472993E-5\t4.129548E-5\t3.774591E-5\t3.415862E-5\t3.060510E-5\t2.714878E-5\t2.384349E-5\t2.073254E-5\t1.784835E-5\t1.521272E-5\t1.283744E-5\t1.072539E-5\t8.871786E-6\t7.265607E-6\t5.891092E-6\t4.729146E-6\t3.758657E-6\t2.957643E-6\t2.304208E-6\t1.777301E-6\t1.357260E-6\t1.026191E-6\t7.681684E-7\t5.693085E-7\t4.177361E-7\t3.034725E-7\t2.182729E-7\t1.554330E-7\t1.095846E-7\t7.649257E-8\t5.286300E-8\t3.616991E-8\t2.450226E-8\t1.643341E-8\t1.091220E-8\t7.173982E-9\t4.669508E-9\t3.009158E-9\t1.919914E-9\t1.212779E-9\t7.584812E-10\t4.696462E-10\t2.879121E-10\r\n2.486420E+0\t1.869238E-10\t3.049128E-10\t4.924358E-10\t7.873840E-10\t1.246484E-9\t1.953663E-9\t3.031628E-9\t4.657631E-9\t7.084632E-9\t1.066922E-8\t1.590783E-8\t2.348292E-8\t3.432073E-8\t4.966198E-8\t7.114665E-8\t1.009132E-7\t1.417113E-7\t1.970263E-7\t2.712107E-7\t3.696175E-7\t4.987251E-7\t6.662435E-7\t8.811864E-7\t1.153893E-6\t1.495983E-6\t1.920218E-6\t2.440268E-6\t3.070347E-6\t3.824728E-6\t4.717117E-6\t5.759912E-6\t6.963347E-6\t8.334571E-6\t9.876693E-6\t1.158785E-5\t1.346038E-5\t1.548013E-5\t1.762605E-5\t1.987003E-5\t2.217712E-5\t2.450613E-5\t2.681065E-5\t2.904042E-5\t3.114309E-5\t3.306613E-5\t3.475907E-5\t3.617562E-5\t3.727579E-5\t3.802777E-5\t3.840942E-5\t3.840942E-5\t3.802777E-5\t3.727579E-5\t3.617562E-5\t3.475907E-5\t3.306613E-5\t3.114309E-5\t2.904042E-5\t2.681065E-5\t2.450613E-5\t2.217712E-5\t1.987003E-5\t1.762605E-5\t1.548013E-5\t1.346038E-5\t1.158785E-5\t9.876693E-6\t8.334571E-6\t6.963347E-6\t5.759912E-6\t4.717117E-6\t3.824728E-6\t3.070347E-6\t2.440268E-6\t1.920218E-6\t1.495983E-6\t1.153893E-6\t8.811864E-7\t6.662435E-7\t4.987251E-7\t3.696175E-7\t2.712107E-7\t1.970263E-7\t1.417113E-7\t1.009132E-7\t7.114665E-8\t4.966198E-8\t3.432073E-8\t2.348292E-8\t1.590783E-8\t1.066922E-8\t7.084632E-9\t4.657631E-9\t3.031628E-9\t1.953663E-9\t1.246484E-9\t7.873840E-10\t4.924358E-10\t3.049128E-10\t1.869238E-10\r\n2.531378E+0\t1.201450E-10\t1.959821E-10\t3.165122E-10\t5.060896E-10\t8.011752E-10\t1.255714E-9\t1.948573E-9\t2.993684E-9\t4.553634E-9\t6.857619E-9\t1.022473E-8\t1.509361E-8\t2.205959E-8\t3.192014E-8\t4.572938E-8\t6.486178E-8\t9.108469E-8\t1.266383E-7\t1.743202E-7\t2.375709E-7\t3.205546E-7\t4.282268E-7\t5.663810E-7\t7.416628E-7\t9.615401E-7\t1.234216E-6\t1.568478E-6\t1.973460E-6\t2.458337E-6\t3.031918E-6\t3.702173E-6\t4.475678E-6\t5.357030E-6\t6.348226E-6\t7.448069E-6\t8.651633E-6\t9.949826E-6\t1.132911E-5\t1.277143E-5\t1.425430E-5\t1.575127E-5\t1.723249E-5\t1.866568E-5\t2.001716E-5\t2.125320E-5\t2.234133E-5\t2.325182E-5\t2.395895E-5\t2.444228E-5\t2.468759E-5\t2.468759E-5\t2.444228E-5\t2.395895E-5\t2.325182E-5\t2.234133E-5\t2.125320E-5\t2.001716E-5\t1.866568E-5\t1.723249E-5\t1.575127E-5\t1.425430E-5\t1.277143E-5\t1.132911E-5\t9.949826E-6\t8.651633E-6\t7.448069E-6\t6.348226E-6\t5.357030E-6\t4.475678E-6\t3.702173E-6\t3.031918E-6\t2.458337E-6\t1.973460E-6\t1.568478E-6\t1.234216E-6\t9.615401E-7\t7.416628E-7\t5.663810E-7\t4.282268E-7\t3.205546E-7\t2.375709E-7\t1.743202E-7\t1.266383E-7\t9.108469E-8\t6.486178E-8\t4.572938E-8\t3.192014E-8\t2.205959E-8\t1.509361E-8\t1.022473E-8\t6.857619E-9\t4.553634E-9\t2.993684E-9\t1.948573E-9\t1.255714E-9\t8.011752E-10\t5.060896E-10\t3.165122E-10\t1.959821E-10\t1.201450E-10\r\n2.576335E+0\t7.645088E-11\t1.247077E-10\t2.014037E-10\t3.220360E-10\t5.098054E-10\t7.990381E-10\t1.239920E-9\t1.904947E-9\t2.897577E-9\t4.363654E-9\t6.506218E-9\t9.604394E-9\t1.403700E-8\t2.031149E-8\t2.909861E-8\t4.127297E-8\t5.795919E-8\t8.058272E-8\t1.109238E-7\t1.511716E-7\t2.039760E-7\t2.724901E-7\t3.604006E-7\t4.719363E-7\t6.118491E-7\t7.853591E-7\t9.980568E-7\t1.255756E-6\t1.564294E-6\t1.929276E-6\t2.355774E-6\t2.847972E-6\t3.408796E-6\t4.039516E-6\t4.739370E-6\t5.505224E-6\t6.331293E-6\t7.208964E-6\t8.126739E-6\t9.070325E-6\t1.002288E-5\t1.096541E-5\t1.187738E-5\t1.273736E-5\t1.352388E-5\t1.421628E-5\t1.479564E-5\t1.524561E-5\t1.555316E-5\t1.570925E-5\t1.570925E-5\t1.555316E-5\t1.524561E-5\t1.479564E-5\t1.421628E-5\t1.352388E-5\t1.273736E-5\t1.187738E-5\t1.096541E-5\t1.002288E-5\t9.070325E-6\t8.126739E-6\t7.208964E-6\t6.331293E-6\t5.505224E-6\t4.739370E-6\t4.039516E-6\t3.408796E-6\t2.847972E-6\t2.355774E-6\t1.929276E-6\t1.564294E-6\t1.255756E-6\t9.980568E-7\t7.853591E-7\t6.118491E-7\t4.719363E-7\t3.604006E-7\t2.724901E-7\t2.039760E-7\t1.511716E-7\t1.109238E-7\t8.058272E-8\t5.795919E-8\t4.127297E-8\t2.909861E-8\t2.031149E-8\t1.403700E-8\t9.604394E-9\t6.506218E-9\t4.363654E-9\t2.897577E-9\t1.904947E-9\t1.239920E-9\t7.990381E-10\t5.098054E-10\t3.220360E-10\t2.014037E-10\t1.247077E-10\t7.645088E-11\r\n2.621293E+0\t4.816100E-11\t7.856089E-11\t1.268763E-10\t2.028698E-10\t3.211570E-10\t5.033621E-10\t7.811000E-10\t1.200040E-9\t1.825358E-9\t2.748928E-9\t4.098657E-9\t6.050384E-9\t8.842750E-9\t1.279543E-8\t1.833096E-8\t2.600032E-8\t3.651197E-8\t5.076389E-8\t6.987753E-8\t9.523207E-8\t1.284967E-7\t1.716579E-7\t2.270380E-7\t2.973010E-7\t3.854405E-7\t4.947448E-7\t6.287359E-7\t7.910761E-7\t9.854426E-7\t1.215367E-6\t1.484043E-6\t1.794109E-6\t2.147405E-6\t2.544733E-6\t2.985614E-6\t3.468071E-6\t3.988461E-6\t4.541359E-6\t5.119521E-6\t5.713942E-6\t6.314013E-6\t6.907773E-6\t7.482276E-6\t8.024028E-6\t8.519501E-6\t8.955688E-6\t9.320663E-6\t9.604122E-6\t9.797868E-6\t9.896202E-6\t9.896202E-6\t9.797868E-6\t9.604122E-6\t9.320663E-6\t8.955688E-6\t8.519501E-6\t8.024028E-6\t7.482276E-6\t6.907773E-6\t6.314013E-6\t5.713942E-6\t5.119521E-6\t4.541359E-6\t3.988461E-6\t3.468071E-6\t2.985614E-6\t2.544733E-6\t2.147405E-6\t1.794109E-6\t1.484043E-6\t1.215367E-6\t9.854426E-7\t7.910761E-7\t6.287359E-7\t4.947448E-7\t3.854405E-7\t2.973010E-7\t2.270380E-7\t1.716579E-7\t1.284967E-7\t9.523207E-8\t6.987753E-8\t5.076389E-8\t3.651197E-8\t2.600032E-8\t1.833096E-8\t1.279543E-8\t8.842750E-9\t6.050384E-9\t4.098657E-9\t2.748928E-9\t1.825358E-9\t1.200040E-9\t7.811000E-10\t5.033621E-10\t3.211570E-10\t2.028698E-10\t1.268763E-10\t7.856089E-11\t4.816100E-11\r\n2.666251E+0\t3.003617E-11\t4.899542E-11\t7.912786E-11\t1.265221E-10\t2.002933E-10\t3.139276E-10\t4.871421E-10\t7.484191E-10\t1.138406E-9\t1.714401E-9\t2.556175E-9\t3.773393E-9\t5.514884E-9\t7.980017E-9\t1.143232E-8\t1.621541E-8\t2.277112E-8\t3.165949E-8\t4.357994E-8\t5.939260E-8\t8.013847E-8\t1.070564E-7\t1.415949E-7\t1.854153E-7\t2.403845E-7\t3.085534E-7\t3.921185E-7\t4.933638E-7\t6.145828E-7\t7.579778E-7\t9.255410E-7\t1.118917E-6\t1.339254E-6\t1.587053E-6\t1.862013E-6\t2.162903E-6\t2.487451E-6\t2.832272E-6\t3.192849E-6\t3.563567E-6\t3.937808E-6\t4.308113E-6\t4.666409E-6\t5.004279E-6\t5.313286E-6\t5.585320E-6\t5.812940E-6\t5.989723E-6\t6.110555E-6\t6.171882E-6\t6.171882E-6\t6.110555E-6\t5.989723E-6\t5.812940E-6\t5.585320E-6\t5.313286E-6\t5.004279E-6\t4.666409E-6\t4.308113E-6\t3.937808E-6\t3.563567E-6\t3.192849E-6\t2.832272E-6\t2.487451E-6\t2.162903E-6\t1.862013E-6\t1.587053E-6\t1.339254E-6\t1.118917E-6\t9.255410E-7\t7.579778E-7\t6.145828E-7\t4.933638E-7\t3.921185E-7\t3.085534E-7\t2.403845E-7\t1.854153E-7\t1.415949E-7\t1.070564E-7\t8.013847E-8\t5.939260E-8\t4.357994E-8\t3.165949E-8\t2.277112E-8\t1.621541E-8\t1.143232E-8\t7.980017E-9\t5.514884E-9\t3.773393E-9\t2.556175E-9\t1.714401E-9\t1.138406E-9\t7.484191E-10\t4.871421E-10\t3.139276E-10\t2.002933E-10\t1.265221E-10\t7.912786E-11\t4.899542E-11\t3.003617E-11\r\n2.711209E+0\t1.854512E-11\t3.025106E-11\t4.885562E-11\t7.811808E-11\t1.236664E-10\t1.938272E-10\t3.007744E-10\t4.620937E-10\t7.028817E-10\t1.058516E-9\t1.578250E-9\t2.329792E-9\t3.405035E-9\t4.927073E-9\t7.058614E-9\t1.001182E-8\t1.405949E-8\t1.954741E-8\t2.690740E-8\t3.667055E-8\t4.947960E-8\t6.609947E-8\t8.742442E-8\t1.144803E-7\t1.484197E-7\t1.905090E-7\t2.421043E-7\t3.046158E-7\t3.794596E-7\t4.679955E-7\t5.714534E-7\t6.908488E-7\t8.268909E-7\t9.798881E-7\t1.149656E-6\t1.335433E-6\t1.535817E-6\t1.748719E-6\t1.971349E-6\t2.200240E-6\t2.431306E-6\t2.659943E-6\t2.881164E-6\t3.089773E-6\t3.280563E-6\t3.448523E-6\t3.589062E-6\t3.698212E-6\t3.772817E-6\t3.810682E-6\t3.810682E-6\t3.772817E-6\t3.698212E-6\t3.589062E-6\t3.448523E-6\t3.280563E-6\t3.089773E-6\t2.881164E-6\t2.659943E-6\t2.431306E-6\t2.200240E-6\t1.971349E-6\t1.748719E-6\t1.535817E-6\t1.335433E-6\t1.149656E-6\t9.798881E-7\t8.268909E-7\t6.908488E-7\t5.714534E-7\t4.679955E-7\t3.794596E-7\t3.046158E-7\t2.421043E-7\t1.905090E-7\t1.484197E-7\t1.144803E-7\t8.742442E-8\t6.609947E-8\t4.947960E-8\t3.667055E-8\t2.690740E-8\t1.954741E-8\t1.405949E-8\t1.001182E-8\t7.058614E-9\t4.927073E-9\t3.405035E-9\t2.329792E-9\t1.578250E-9\t1.058516E-9\t7.028817E-10\t4.620937E-10\t3.007744E-10\t1.938272E-10\t1.236664E-10\t7.811808E-11\t4.885562E-11\t3.025106E-11\t1.854512E-11\r\n2.756167E+0\t1.133577E-11\t1.849106E-11\t2.986316E-11\t4.774993E-11\t7.559148E-11\t1.184775E-10\t1.838493E-10\t2.824563E-10\t4.296388E-10\t6.470215E-10\t9.647105E-10\t1.424093E-9\t2.081339E-9\t3.011689E-9\t4.314601E-9\t6.119757E-9\t8.593909E-9\t1.194842E-8\t1.644724E-8\t2.241500E-8\t3.024457E-8\t4.040352E-8\t5.343846E-8\t6.997644E-8\t9.072202E-8\t1.164492E-7\t1.479870E-7\t1.861974E-7\t2.319459E-7\t2.860638E-7\t3.493027E-7\t4.222836E-7\t5.054398E-7\t5.989598E-7\t7.027309E-7\t8.162880E-7\t9.387735E-7\t1.068910E-6\t1.204994E-6\t1.344904E-6\t1.486144E-6\t1.625899E-6\t1.761121E-6\t1.888634E-6\t2.005255E-6\t2.107921E-6\t2.193826E-6\t2.260545E-6\t2.306147E-6\t2.329292E-6\t2.329292E-6\t2.306147E-6\t2.260545E-6\t2.193826E-6\t2.107921E-6\t2.005255E-6\t1.888634E-6\t1.761121E-6\t1.625899E-6\t1.486144E-6\t1.344904E-6\t1.204994E-6\t1.068910E-6\t9.387735E-7\t8.162880E-7\t7.027309E-7\t5.989598E-7\t5.054398E-7\t4.222836E-7\t3.493027E-7\t2.860638E-7\t2.319459E-7\t1.861974E-7\t1.479870E-7\t1.164492E-7\t9.072202E-8\t6.997644E-8\t5.343846E-8\t4.040352E-8\t3.024457E-8\t2.241500E-8\t1.644724E-8\t1.194842E-8\t8.593909E-9\t6.119757E-9\t4.314601E-9\t3.011689E-9\t2.081339E-9\t1.424093E-9\t9.647105E-10\t6.470215E-10\t4.296388E-10\t2.824563E-10\t1.838493E-10\t1.184775E-10\t7.559148E-11\t4.774993E-11\t2.986316E-11\t1.849106E-11\t1.133577E-11\r\n"
  out "2D measured PDF output":string="\t-3.411158E+0\t-3.342246E+0\t-3.273333E+0\t-3.204421E+0\t-3.135509E+0\t-3.066596E+0\t-2.997684E+0\t-2.928772E+0\t-2.859860E+0\t-2.790947E+0\t-2.722035E+0\t-2.653123E+0\t-2.584211E+0\t-2.515298E+0\t-2.446386E+0\t-2.377474E+0\t-2.308561E+0\t-2.239649E+0\t-2.170737E+0\t-2.101825E+0\t-2.032912E+0\t-1.964000E+0\t-1.895088E+0\t-1.826175E+0\t-1.757263E+0\t-1.688351E+0\t-1.619439E+0\t-1.550526E+0\t-1.481614E+0\t-1.412702E+0\t-1.343789E+0\t-1.274877E+0\t-1.205965E+0\t-1.137053E+0\t-1.068140E+0\t-9.992281E-1\t-9.303158E-1\t-8.614035E-1\t-7.924912E-1\t-7.235789E-1\t-6.546667E-1\t-5.857544E-1\t-5.168421E-1\t-4.479298E-1\t-3.790175E-1\t-3.101053E-1\t-2.411930E-1\t-1.722807E-1\t-1.033684E-1\t-3.445614E-2\t3.445614E-2\t1.033684E-1\t1.722807E-1\t2.411930E-1\t3.101053E-1\t3.790175E-1\t4.479298E-1\t5.168421E-1\t5.857544E-1\t6.546667E-1\t7.235789E-1\t7.924912E-1\t8.614035E-1\t9.303158E-1\t9.992281E-1\t1.068140E+0\t1.137053E+0\t1.205965E+0\t1.274877E+0\t1.343789E+0\t1.412702E+0\t1.481614E+0\t1.550526E+0\t1.619439E+0\t1.688351E+0\t1.757263E+0\t1.826175E+0\t1.895088E+0\t1.964000E+0\t2.032912E+0\t2.101825E+0\t2.170737E+0\t2.239649E+0\t2.308561E+0\t2.377474E+0\t2.446386E+0\t2.515298E+0\t2.584211E+0\t2.653123E+0\t2.722035E+0\t2.790947E+0\t2.859860E+0\t2.928772E+0\t2.997684E+0\t3.066596E+0\t3.135509E+0\t3.204421E+0\t3.273333E+0\t3.342246E+0\t3.411158E+0\r\n-1.694652E+0\t0.000000E+0\t0.000000E+0\t0.000000E+0\t0.000000E+0\t0.000000E+0\t0.000000E+0\t0.000000E+0\t0.000000E+0\t0.000000E+0\t0.000000E+0\t0.000000E+0\t0.000000E+0\t0.000000E+0\t0.000000E+0\t0.000000E+0\t0.000000E+0\t0.000000E+0\t0.000000E+0\t0.000000E+0\t0.000000E+0\t0.000000E+0\t0.000000E+0\t0.000000E+0\t0.000000E+0\t0.000000E+0\t0.000000E+0\t0.000000E+0\t0.000000E+0\t0.000000E+0\t0.000000E+0\t0.000000E+0\t0.000000E+0\t0.000000E+0\t0.000000E+0\t0.000000E+0\t0.000000E+0\t0.000000E+0\t0.000000E+0\t0.000000E+0\t0.000000E+0\t0.000000E+0\t0.000000E+0\t0.000000E+0\t0.000000E+0\t0.000000E+0\t0.000000E+0\t0.000000E+0\t0.000000E+0\t0.000000E+0\t0.000000E+0\t0.000000E+0\t0.000000E+0\t0.000000E+0\t0.000000E+0\t0.000000E+0\t0.000000E+0\t0.000000E+0\t0.000000E+0\t0.000000E+0\t0.000000E+0\t0.000000E+0\t0.000000E+0\t0.000000E+0\t0.000000E+0\t0.000000E+0\t0.000000E+0\t0.000000E+0\t0.000000E+0\t0.000000E+0\t0.000000E+0\t0.000000E+0\t0.000000E+0\t0.000000E+0\t0.000000E+0\t0.000000E+0\t0.000000E+0\t0.000000E+0\t0.000000E+0\t0.000000E+0\t0.000000E+0\t0.000000E+0\t0.000000E+0\t0.000000E+0\t0.000000E+0\t0.000000E+0\t0.000000E+0\t0.000000E+0\t0.000000E+0\t0.000000E+0\t0.000000E+0\t0.000000E+0\t0.000000E+0\t0.000000E+0\t0.000000E+0\t0.000000E+0\t0.000000E+0\t0.000000E+0\t0.000000E+0\t0.000000E+0\t0.000000E+0\r\n-1.649695E+0\t0.000000E+0\t0.000000E+0\t0.000000E+0\t0.000000E+0\t0.000000E+0\t0.000000E+0\t0.000000E+0\t0.000000E+0\t0.000000E+0\t0.000000E+0\t0.000000E+0\t0.000000E+0\t0.000000E+0\t0.000000E+0\t0.000000E+0\t0.000000E+0\t0.000000E+0\t0.000000E+0\t0.000000E+0\t0.000000E+0\t0.000000E+0\t0.000000E+0\t0.000000E+0\t0.000000E+0\t0.000000E+0\t0.000000E+0\t0.000000E+0\t0.000000E+0\t0.000000E+0\t0.000000E+0\t0.000000E+0\t0.000000E+0\t0.000000E+0\t0.000000E+0\t0.000000E+0\t0.000000E+0\t0.000000E+0\t0.000000E+0\t0.000000E+0\t0.000000E+0\t0.000000E+0\t0.000000E+0\t0.000000E+0\t0.000000E+0\t0.000000E+0\t0.000000E+0\t0.000000E+0\t0.000000E+0\t0.000000E+0\t0.000000E+0\t0.000000E+0\t0.000000E+0\t0.000000E+0\t0.000000E+0\t0.000000E+0\t0.000000E+0\t0.000000E+0\t0.000000E+0\t0.000000E+0\t0.000000E+0\t0.000000E+0\t0.000000E+0\t0.000000E+0\t0.000000E+0\t0.000000E+0\t0.000000E+0\t0.000000E+0\t0.000000E+0\t0.000000E+0\t0.000000E+0\t0.000000E+0\t0.000000E+0\t0.000000E+0\t0.000000E+0\t0.000000E+0\t0.000000E+0\t0.000000E+0\t0.000000E+0\t0.000000E+0\t0.000000E+0\t0.000000E+0\t0.000000E+0\t0.000000E+0\t0.000000E+0\t0.000000E+0\t0.000000E+0\t0.000000E+0\t0.000000E+0\t0.000000E+0\t0.000000E+0\t0.000000E+0\t0.000000E+0\t0.000000E+0\t0.000000E+0\t0.000000E+0\t0.000000E+0\t0.000000E+0\t0.000000E+0\t0.000000E+0\t0.000000E+0\r\n-1.604737E+0\t0.000000E+0\t0.000000E+0\t0.000000E+0\t0.000000E+0\t0.000000E+0\t0.000000E+0\t0.000000E+0\t0.000000E+0\t0.000000E+0\t0.000000E+0\t0.000000E+0\t0.000000E+0\t0.000000E+0\t0.000000E+0\t0.000000E+0\t0.000000E+0\t0.000000E+0\t0.000000E+0\t0.000000E+0\t0.000000E+0\t0.000000E+0\t0.000000E+0\t0.000000E+0\t0.000000E+0\t0.000000E+0\t0.000000E+0\t0.000000E+0\t0.000000E+0\t0.000000E+0\t0.000000E+0\t0.000000E+0\t0.000000E+0\t0.000000E+0\t0.000000E+0\t0.000000E+0\t0.000000E+0\t0.000000E+0\t0.000000E+0\t0.000000E+0\t0.000000E+0\t0.000000E+0\t0.000000E+0\t0.000000E+0\t0.000000E+0\t0.000000E+0\t0.000000E+0\t0.000000E+0\t0.000000E+0\t0.000000E+0\t0.000000E+0\t0.000000E+0\t0.000000E+0\t0.000000E+0\t0.000000E+0\t0.000000E+0\t0.000000E+0\t0.000000E+0\t0.000000E+0\t0.000000E+0\t0.000000E+0\t0.000000E+0\t0.000000E+0\t0.000000E+0\t0.000000E+0\t0.000000E+0\t0.000000E+0\t0.000000E+0\t0.000000E+0\t0.000000E+0\t0.000000E+0\t0.000000E+0\t0.000000E+0\t0.000000E+0\t0.000000E+0\t0.000000E+0\t0.000000E+0\t0.000000E+0\t0.000000E+0\t0.000000E+0\t0.000000E+0\t0.000000E+0\t0.000000E+0\t0.000000E+0\t0.000000E+0\t0.000000E+0\t0.000000E+0\t0.000000E+0\t0.000000E+0\t0.000000E+0\t0.000000E+0\t0.000000E+0\t0.000000E+0\t0.000000E+0\t0.000000E+0\t0.000000E+0\t0.000000E+0\t0.000000E+0\t0.000000E+0\t0.000000E+0\t0.000000E+0\r\n-1.559779E+0\t0.000000E+0\t0.000000E+0\t0.000000E+0\t0.000000E+0\t0.000000E+0\t0.000000E+0\t0.000000E+0\t0.000000E+0\t0.000000E+0\t0.000000E+0\t0.000000E+0\t0.000000E+0\t0.000000E+0\t0.000000E+0\t0.000000E+0\t0.000000E+0\t0.000000E+0\t0.000000E+0\t0.000000E+0\t0.000000E+0\t0.000000E+0\t0.000000E+0\t0.000000E+0\t0.000000E+0\t0.000000E+0\t0.000000E+0\t0.000000E+0\t0.000000E+0\t0.000000E+0\t0.000000E+0\t0.000000E+0\t0.000000E+0\t0.000000E+0\t0.000000E+0\t0.000000E+0\t0.000000E+0\t0.000000E+0\t0.000000E+0\t0.000000E+0\t0.000000E+0\t0.000000E+0\t0.000000E+0\t0.000000E+0\t0.000000E+0\t0.000000E+0\t0.000000E+0\t0.000000E+0\t0.000000E+0\t0.000000E+0\t0.000000E+0\t0.000000E+0\t0.000000E+0\t0.000000E+0\t0.000000E+0\t0.000000E+0\t0.000000E+0\t0.000000E+0\t0.000000E+0\t0.000000E+0\t0.000000E+0\t0.000000E+0\t0.000000E+0\t0.000000E+0\t0.000000E+0\t0.000000E+0\t0.000000E+0\t0.000000E+0\t0.000000E+0\t0.000000E+0\t0.000000E+0\t0.000000E+0\t0.000000E+0\t0.000000E+0\t0.000000E+0\t0.000000E+0\t0.000000E+0\t0.000000E+0\t0.000000E+0\t0.000000E+0\t0.000000E+0\t0.000000E+0\t0.000000E+0\t0.000000E+0\t0.000000E+0\t0.000000E+0\t0.000000E+0\t0.000000E+0\t0.000000E+0\t0.000000E+0\t0.000000E+0\t0.000000E+0\t0.000000E+0\t0.000000E+0\t0.000000E+0\t0.000000E+0\t0.000000E+0\t0.000000E+0\t0.000000E+0\t0.000000E+0\t0.000000E+0\r\n-1.514821E+0\t0.000000E+0\t0.000000E+0\t0.000000E+0\t0.000000E+0\t0.000000E+0\t0.000000E+0\t0.000000E+0\t0.000000E+0\t0.000000E+0\t0.000000E+0\t0.000000E+0\t0.000000E+0\t0.000000E+0\t0.000000E+0\t0.000000E+0\t0.000000E+0\t0.000000E+0\t0.000000E+0\t0.000000E+0\t0.000000E+0\t0.000000E+0\t0.000000E+0\t0.000000E+0\t0.000000E+0\t0.000000E+0\t0.000000E+0\t0.000000E+0\t0.000000E+0\t0.000000E+0\t0.000000E+0\t0.000000E+0\t0.000000E+0\t0.000000E+0\t0.000000E+0\t0.000000E+0\t0.000000E+0\t0.000000E+0\t0.000000E+0\t0.000000E+0\t0.000000E+0\t0.000000E+0\t0.000000E+0\t0.000000E+0\t0.000000E+0\t0.000000E+0\t0.000000E+0\t0.000000E+0\t0.000000E+0\t0.000000E+0\t0.000000E+0\t0.000000E+0\t0.000000E+0\t0.000000E+0\t0.000000E+0\t0.000000E+0\t0.000000E+0\t0.000000E+0\t0.000000E+0\t0.000000E+0\t0.000000E+0\t0.000000E+0\t0.000000E+0\t0.000000E+0\t0.000000E+0\t0.000000E+0\t0.000000E+0\t0.000000E+0\t0.000000E+0\t0.000000E+0\t0.000000E+0\t0.000000E+0\t0.000000E+0\t0.000000E+0\t0.000000E+0\t0.000000E+0\t0.000000E+0\t0.000000E+0\t0.000000E+0\t0.000000E+0\t0.000000E+0\t0.000000E+0\t0.000000E+0\t0.000000E+0\t0.000000E+0\t0.000000E+0\t0.000000E+0\t0.000000E+0\t0.000000E+0\t0.000000E+0\t0.000000E+0\t0.000000E+0\t0.000000E+0\t0.000000E+0\t0.000000E+0\t0.000000E+0\t0.000000E+0\t0.000000E+0\t0.000000E+0\t0.000000E+0\t0.000000E+0\r\n-1.469864E+0\t0.000000E+0\t0.000000E+0\t0.000000E+0\t0.000000E+0\t0.000000E+0\t0.000000E+0\t0.000000E+0\t0.000000E+0\t0.000000E+0\t0.000000E+0\t0.000000E+0\t0.000000E+0\t0.000000E+0\t0.000000E+0\t0.000000E+0\t0.000000E+0\t0.000000E+0\t0.000000E+0\t0.000000E+0\t0.000000E+0\t0.000000E+0\t0.000000E+0\t0.000000E+0\t0.000000E+0\t0.000000E+0\t0.000000E+0\t0.000000E+0\t0.000000E+0\t0.000000E+0\t0.000000E+0\t0.000000E+0\t0.000000E+0\t0.000000E+0\t0.000000E+0\t0.000000E+0\t0.000000E+0\t0.000000E+0\t0.000000E+0\t0.000000E+0\t0.000000E+0\t0.000000E+0\t0.000000E+0\t0.000000E+0\t0.000000E+0\t0.000000E+0\t0.000000E+0\t0.000000E+0\t0.000000E+0\t0.000000E+0\t0.000000E+0\t0.000000E+0\t0.000000E+0\t0.000000E+0\t0.000000E+0\t0.000000E+0\t0.000000E+0\t0.000000E+0\t0.000000E+0\t0.000000E+0\t0.000000E+0\t0.000000E+0\t0.000000E+0\t0.000000E+0\t0.000000E+0\t0.000000E+0\t0.000000E+0\t0.000000E+0\t0.000000E+0\t0.000000E+0\t0.000000E+0\t0.000000E+0\t0.000000E+0\t0.000000E+0\t0.000000E+0\t0.000000E+0\t0.000000E+0\t0.000000E+0\t0.000000E+0\t0.000000E+0\t0.000000E+0\t0.000000E+0\t0.000000E+0\t0.000000E+0\t0.000000E+0\t0.000000E+0\t0.000000E+0\t0.000000E+0\t0.000000E+0\t0.000000E+0\t0.000000E+0\t0.000000E+0\t0.000000E+0\t0.000000E+0\t0.000000E+0\t0.000000E+0\t0.000000E+0\t0.000000E+0\t0.000000E+0\t0.000000E+0\t0.000000E+0\r\n-1.424906E+0\t0.000000E+0\t0.000000E+0\t0.000000E+0\t0.000000E+0\t0.000000E+0\t0.000000E+0\t0.000000E+0\t0.000000E+0\t0.000000E+0\t0.000000E+0\t0.000000E+0\t0.000000E+0\t0.000000E+0\t0.000000E+0\t0.000000E+0\t0.000000E+0\t0.000000E+0\t0.000000E+0\t0.000000E+0\t0.000000E+0\t0.000000E+0\t0.000000E+0\t0.000000E+0\t0.000000E+0\t0.000000E+0\t0.000000E+0\t0.000000E+0\t0.000000E+0\t0.000000E+0\t0.000000E+0\t0.000000E+0\t0.000000E+0\t0.000000E+0\t0.000000E+0\t0.000000E+0\t0.000000E+0\t0.000000E+0\t0.000000E+0\t0.000000E+0\t0.000000E+0\t0.000000E+0\t0.000000E+0\t0.000000E+0\t0.000000E+0\t0.000000E+0\t0.000000E+0\t0.000000E+0\t0.000000E+0\t0.000000E+0\t0.000000E+0\t0.000000E+0\t0.000000E+0\t0.000000E+0\t0.000000E+0\t0.000000E+0\t0.000000E+0\t0.000000E+0\t0.000000E+0\t0.000000E+0\t0.000000E+0\t0.000000E+0\t0.000000E+0\t0.000000E+0\t0.000000E+0\t0.000000E+0\t0.000000E+0\t0.000000E+0\t0.000000E+0\t0.000000E+0\t0.000000E+0\t0.000000E+0\t0.000000E+0\t0.000000E+0\t0.000000E+0\t0.000000E+0\t0.000000E+0\t0.000000E+0\t0.000000E+0\t0.000000E+0\t0.000000E+0\t0.000000E+0\t0.000000E+0\t0.000000E+0\t0.000000E+0\t0.000000E+0\t0.000000E+0\t0.000000E+0\t0.000000E+0\t0.000000E+0\t0.000000E+0\t0.000000E+0\t0.000000E+0\t0.000000E+0\t0.000000E+0\t0.000000E+0\t0.000000E+0\t0.000000E+0\t0.000000E+0\t0.000000E+0\t0.000000E+0\r\n-1.379948E+0\t0.000000E+0\t0.000000E+0\t0.000000E+0\t0.000000E+0\t0.000000E+0\t0.000000E+0\t0.000000E+0\t0.000000E+0\t0.000000E+0\t0.000000E+0\t0.000000E+0\t0.000000E+0\t0.000000E+0\t0.000000E+0\t0.000000E+0\t0.000000E+0\t0.000000E+0\t0.000000E+0\t0.000000E+0\t0.000000E+0\t0.000000E+0\t0.000000E+0\t0.000000E+0\t0.000000E+0\t0.000000E+0\t0.000000E+0\t0.000000E+0\t0.000000E+0\t0.000000E+0\t0.000000E+0\t0.000000E+0\t0.000000E+0\t0.000000E+0\t0.000000E+0\t0.000000E+0\t0.000000E+0\t0.000000E+0\t0.000000E+0\t0.000000E+0\t0.000000E+0\t0.000000E+0\t0.000000E+0\t0.000000E+0\t0.000000E+0\t0.000000E+0\t0.000000E+0\t0.000000E+0\t0.000000E+0\t0.000000E+0\t0.000000E+0\t0.000000E+0\t0.000000E+0\t0.000000E+0\t0.000000E+0\t0.000000E+0\t0.000000E+0\t0.000000E+0\t0.000000E+0\t0.000000E+0\t0.000000E+0\t0.000000E+0\t0.000000E+0\t0.000000E+0\t0.000000E+0\t0.000000E+0\t0.000000E+0\t0.000000E+0\t0.000000E+0\t0.000000E+0\t0.000000E+0\t0.000000E+0\t0.000000E+0\t0.000000E+0\t0.000000E+0\t0.000000E+0\t0.000000E+0\t0.000000E+0\t0.000000E+0\t0.000000E+0\t0.000000E+0\t0.000000E+0\t0.000000E+0\t0.000000E+0\t0.000000E+0\t0.000000E+0\t0.000000E+0\t0.000000E+0\t0.000000E+0\t0.000000E+0\t0.000000E+0\t0.000000E+0\t0.000000E+0\t0.000000E+0\t0.000000E+0\t0.000000E+0\t0.000000E+0\t0.000000E+0\t0.000000E+0\t0.000000E+0\t0.000000E+0\r\n-1.334990E+0\t0.000000E+0\t0.000000E+0\t0.000000E+0\t0.000000E+0\t0.000000E+0\t0.000000E+0\t0.000000E+0\t0.000000E+0\t0.000000E+0\t0.000000E+0\t0.000000E+0\t0.000000E+0\t0.000000E+0\t0.000000E+0\t0.000000E+0\t0.000000E+0\t0.000000E+0\t0.000000E+0\t0.000000E+0\t0.000000E+0\t0.000000E+0\t0.000000E+0\t0.000000E+0\t0.000000E+0\t0.000000E+0\t0.000000E+0\t0.000000E+0\t0.000000E+0\t0.000000E+0\t0.000000E+0\t0.000000E+0\t0.000000E+0\t0.000000E+0\t0.000000E+0\t0.000000E+0\t0.000000E+0\t0.000000E+0\t0.000000E+0\t0.000000E+0\t0.000000E+0\t0.000000E+0\t0.000000E+0\t0.000000E+0\t0.000000E+0\t0.000000E+0\t0.000000E+0\t0.000000E+0\t0.000000E+0\t0.000000E+0\t0.000000E+0\t0.000000E+0\t0.000000E+0\t0.000000E+0\t0.000000E+0\t0.000000E+0\t0.000000E+0\t0.000000E+0\t0.000000E+0\t0.000000E+0\t0.000000E+0\t0.000000E+0\t0.000000E+0\t0.000000E+0\t0.000000E+0\t0.000000E+0\t0.000000E+0\t0.000000E+0\t0.000000E+0\t0.000000E+0\t0.000000E+0\t0.000000E+0\t0.000000E+0\t0.000000E+0\t0.000000E+0\t0.000000E+0\t0.000000E+0\t0.000000E+0\t0.000000E+0\t0.000000E+0\t0.000000E+0\t0.000000E+0\t0.000000E+0\t0.000000E+0\t0.000000E+0\t0.000000E+0\t0.000000E+0\t0.000000E+0\t0.000000E+0\t0.000000E+0\t0.000000E+0\t0.000000E+0\t0.000000E+0\t0.000000E+0\t0.000000E+0\t0.000000E+0\t0.000000E+0\t0.000000E+0\t0.000000E+0\t0.000000E+0\t0.000000E+0\r\n-1.290033E+0\t0.000000E+0\t0.000000E+0\t0.000000E+0\t0.000000E+0\t0.000000E+0\t0.000000E+0\t0.000000E+0\t0.000000E+0\t0.000000E+0\t0.000000E+0\t0.000000E+0\t0.000000E+0\t0.000000E+0\t0.000000E+0\t0.000000E+0\t0.000000E+0\t0.000000E+0\t0.000000E+0\t0.000000E+0\t0.000000E+0\t0.000000E+0\t0.000000E+0\t0.000000E+0\t0.000000E+0\t0.000000E+0\t0.000000E+0\t0.000000E+0\t0.000000E+0\t0.000000E+0\t0.000000E+0\t0.000000E+0\t0.000000E+0\t0.000000E+0\t0.000000E+0\t0.000000E+0\t0.000000E+0\t0.000000E+0\t0.000000E+0\t0.000000E+0\t0.000000E+0\t0.000000E+0\t0.000000E+0\t0.000000E+0\t0.000000E+0\t0.000000E+0\t0.000000E+0\t0.000000E+0\t0.000000E+0\t0.000000E+0\t0.000000E+0\t0.000000E+0\t0.000000E+0\t0.000000E+0\t0.000000E+0\t0.000000E+0\t0.000000E+0\t0.000000E+0\t0.000000E+0\t0.000000E+0\t0.000000E+0\t0.000000E+0\t0.000000E+0\t0.000000E+0\t0.000000E+0\t0.000000E+0\t0.000000E+0\t0.000000E+0\t0.000000E+0\t0.000000E+0\t0.000000E+0\t0.000000E+0\t0.000000E+0\t0.000000E+0\t0.000000E+0\t0.000000E+0\t0.000000E+0\t0.000000E+0\t0.000000E+0\t0.000000E+0\t0.000000E+0\t0.000000E+0\t0.000000E+0\t0.000000E+0\t0.000000E+0\t0.000000E+0\t0.000000E+0\t0.000000E+0\t0.000000E+0\t0.000000E+0\t0.000000E+0\t0.000000E+0\t0.000000E+0\t0.000000E+0\t0.000000E+0\t0.000000E+0\t0.000000E+0\t0.000000E+0\t0.000000E+0\t0.000000E+0\t0.000000E+0\r\n-1.245075E+0\t0.000000E+0\t0.000000E+0\t0.000000E+0\t0.000000E+0\t0.000000E+0\t0.000000E+0\t0.000000E+0\t0.000000E+0\t0.000000E+0\t0.000000E+0\t0.000000E+0\t0.000000E+0\t0.000000E+0\t0.000000E+0\t0.000000E+0\t0.000000E+0\t0.000000E+0\t0.000000E+0\t0.000000E+0\t0.000000E+0\t0.000000E+0\t0.000000E+0\t0.000000E+0\t0.000000E+0\t0.000000E+0\t0.000000E+0\t0.000000E+0\t0.000000E+0\t0.000000E+0\t0.000000E+0\t0.000000E+0\t0.000000E+0\t0.000000E+0\t0.000000E+0\t0.000000E+0\t0.000000E+0\t0.000000E+0\t0.000000E+0\t0.000000E+0\t0.000000E+0\t0.000000E+0\t0.000000E+0\t0.000000E+0\t0.000000E+0\t0.000000E+0\t0.000000E+0\t0.000000E+0\t0.000000E+0\t0.000000E+0\t0.000000E+0\t0.000000E+0\t0.000000E+0\t0.000000E+0\t0.000000E+0\t0.000000E+0\t0.000000E+0\t0.000000E+0\t0.000000E+0\t0.000000E+0\t0.000000E+0\t0.000000E+0\t0.000000E+0\t0.000000E+0\t0.000000E+0\t0.000000E+0\t0.000000E+0\t0.000000E+0\t0.000000E+0\t0.000000E+0\t0.000000E+0\t0.000000E+0\t0.000000E+0\t0.000000E+0\t0.000000E+0\t0.000000E+0\t0.000000E+0\t0.000000E+0\t0.000000E+0\t0.000000E+0\t0.000000E+0\t0.000000E+0\t0.000000E+0\t0.000000E+0\t0.000000E+0\t0.000000E+0\t0.000000E+0\t0.000000E+0\t0.000000E+0\t0.000000E+0\t0.000000E+0\t0.000000E+0\t0.000000E+0\t0.000000E+0\t0.000000E+0\t0.000000E+0\t0.000000E+0\t0.000000E+0\t0.000000E+0\t0.000000E+0\t0.000000E+0\r\n-1.200117E+0\t0.000000E+0\t0.000000E+0\t0.000000E+0\t0.000000E+0\t0.000000E+0\t0.000000E+0\t0.000000E+0\t0.000000E+0\t0.000000E+0\t0.000000E+0\t0.000000E+0\t0.000000E+0\t0.000000E+0\t0.000000E+0\t0.000000E+0\t0.000000E+0\t0.000000E+0\t0.000000E+0\t0.000000E+0\t0.000000E+0\t0.000000E+0\t0.000000E+0\t0.000000E+0\t0.000000E+0\t0.000000E+0\t0.000000E+0\t0.000000E+0\t0.000000E+0\t0.000000E+0\t0.000000E+0\t0.000000E+0\t0.000000E+0\t0.000000E+0\t0.000000E+0\t0.000000E+0\t0.000000E+0\t0.000000E+0\t0.000000E+0\t0.000000E+0\t0.000000E+0\t0.000000E+0\t0.000000E+0\t0.000000E+0\t0.000000E+0\t0.000000E+0\t0.000000E+0\t0.000000E+0\t0.000000E+0\t0.000000E+0\t0.000000E+0\t0.000000E+0\t0.000000E+0\t0.000000E+0\t0.000000E+0\t0.000000E+0\t0.000000E+0\t0.000000E+0\t0.000000E+0\t0.000000E+0\t0.000000E+0\t0.000000E+0\t0.000000E+0\t0.000000E+0\t0.000000E+0\t0.000000E+0\t0.000000E+0\t0.000000E+0\t0.000000E+0\t0.000000E+0\t0.000000E+0\t0.000000E+0\t0.000000E+0\t0.000000E+0\t0.000000E+0\t0.000000E+0\t0.000000E+0\t0.000000E+0\t0.000000E+0\t0.000000E+0\t0.000000E+0\t0.000000E+0\t0.000000E+0\t0.000000E+0\t0.000000E+0\t0.000000E+0\t0.000000E+0\t0.000000E+0\t0.000000E+0\t0.000000E+0\t0.000000E+0\t0.000000E+0\t0.000000E+0\t0.000000E+0\t0.000000E+0\t0.000000E+0\t0.000000E+0\t0.000000E+0\t0.000000E+0\t0.000000E+0\t0.000000E+0\r\n-1.155159E+0\t0.000000E+0\t0.000000E+0\t0.000000E+0\t0.000000E+0\t0.000000E+0\t0.000000E+0\t0.000000E+0\t0.000000E+0\t0.000000E+0\t0.000000E+0\t0.000000E+0\t0.000000E+0\t0.000000E+0\t0.000000E+0\t0.000000E+0\t0.000000E+0\t0.000000E+0\t0.000000E+0\t0.000000E+0\t0.000000E+0\t0.000000E+0\t0.000000E+0\t0.000000E+0\t0.000000E+0\t0.000000E+0\t0.000000E+0\t0.000000E+0\t0.000000E+0\t0.000000E+0\t0.000000E+0\t0.000000E+0\t0.000000E+0\t0.000000E+0\t0.000000E+0\t0.000000E+0\t0.000000E+0\t0.000000E+0\t0.000000E+0\t0.000000E+0\t0.000000E+0\t0.000000E+0\t0.000000E+0\t0.000000E+0\t0.000000E+0\t0.000000E+0\t0.000000E+0\t0.000000E+0\t0.000000E+0\t0.000000E+0\t0.000000E+0\t0.000000E+0\t0.000000E+0\t0.000000E+0\t0.000000E+0\t0.000000E+0\t0.000000E+0\t0.000000E+0\t0.000000E+0\t0.000000E+0\t0.000000E+0\t0.000000E+0\t0.000000E+0\t0.000000E+0\t0.000000E+0\t0.000000E+0\t0.000000E+0\t0.000000E+0\t0.000000E+0\t0.000000E+0\t0.000000E+0\t0.000000E+0\t0.000000E+0\t0.000000E+0\t0.000000E+0\t0.000000E+0\t0.000000E+0\t0.000000E+0\t0.000000E+0\t0.000000E+0\t0.000000E+0\t0.000000E+0\t0.000000E+0\t0.000000E+0\t0.000000E+0\t0.000000E+0\t0.000000E+0\t0.000000E+0\t0.000000E+0\t0.000000E+0\t0.000000E+0\t0.000000E+0\t0.000000E+0\t0.000000E+0\t0.000000E+0\t0.000000E+0\t0.000000E+0\t0.000000E+0\t0.000000E+0\t0.000000E+0\t0.000000E+0\r\n-1.110201E+0\t0.000000E+0\t0.000000E+0\t0.000000E+0\t0.000000E+0\t0.000000E+0\t0.000000E+0\t0.000000E+0\t0.000000E+0\t0.000000E+0\t0.000000E+0\t0.000000E+0\t0.000000E+0\t0.000000E+0\t0.000000E+0\t0.000000E+0\t0.000000E+0\t0.000000E+0\t0.000000E+0\t0.000000E+0\t0.000000E+0\t0.000000E+0\t0.000000E+0\t0.000000E+0\t0.000000E+0\t0.000000E+0\t0.000000E+0\t0.000000E+0\t0.000000E+0\t0.000000E+0\t0.000000E+0\t0.000000E+0\t0.000000E+0\t0.000000E+0\t0.000000E+0\t0.000000E+0\t0.000000E+0\t0.000000E+0\t0.000000E+0\t0.000000E+0\t0.000000E+0\t0.000000E+0\t0.000000E+0\t0.000000E+0\t0.000000E+0\t0.000000E+0\t0.000000E+0\t0.000000E+0\t0.000000E+0\t0.000000E+0\t0.000000E+0\t0.000000E+0\t0.000000E+0\t0.000000E+0\t0.000000E+0\t0.000000E+0\t0.000000E+0\t0.000000E+0\t0.000000E+0\t0.000000E+0\t0.000000E+0\t0.000000E+0\t0.000000E+0\t0.000000E+0\t0.000000E+0\t0.000000E+0\t0.000000E+0\t0.000000E+0\t0.000000E+0\t0.000000E+0\t0.000000E+0\t0.000000E+0\t0.000000E+0\t0.000000E+0\t0.000000E+0\t0.000000E+0\t0.000000E+0\t0.000000E+0\t0.000000E+0\t0.000000E+0\t0.000000E+0\t0.000000E+0\t0.000000E+0\t0.000000E+0\t0.000000E+0\t0.000000E+0\t0.000000E+0\t0.000000E+0\t0.000000E+0\t0.000000E+0\t0.000000E+0\t0.000000E+0\t0.000000E+0\t0.000000E+0\t0.000000E+0\t0.000000E+0\t0.000000E+0\t0.000000E+0\t0.000000E+0\t0.000000E+0\t0.000000E+0\r\n-1.065244E+0\t0.000000E+0\t0.000000E+0\t0.000000E+0\t0.000000E+0\t0.000000E+0\t0.000000E+0\t0.000000E+0\t0.000000E+0\t0.000000E+0\t0.000000E+0\t0.000000E+0\t0.000000E+0\t0.000000E+0\t0.000000E+0\t0.000000E+0\t0.000000E+0\t0.000000E+0\t0.000000E+0\t0.000000E+0\t0.000000E+0\t0.000000E+0\t0.000000E+0\t0.000000E+0\t0.000000E+0\t0.000000E+0\t0.000000E+0\t0.000000E+0\t0.000000E+0\t0.000000E+0\t0.000000E+0\t0.000000E+0\t0.000000E+0\t0.000000E+0\t0.000000E+0\t0.000000E+0\t0.000000E+0\t0.000000E+0\t0.000000E+0\t0.000000E+0\t0.000000E+0\t0.000000E+0\t0.000000E+0\t0.000000E+0\t0.000000E+0\t0.000000E+0\t0.000000E+0\t0.000000E+0\t0.000000E+0\t0.000000E+0\t0.000000E+0\t0.000000E+0\t0.000000E+0\t0.000000E+0\t0.000000E+0\t0.000000E+0\t0.000000E+0\t0.000000E+0\t0.000000E+0\t0.000000E+0\t0.000000E+0\t0.000000E+0\t0.000000E+0\t0.000000E+0\t0.000000E+0\t0.000000E+0\t0.000000E+0\t0.000000E+0\t0.000000E+0\t0.000000E+0\t0.000000E+0\t0.000000E+0\t0.000000E+0\t0.000000E+0\t0.000000E+0\t0.000000E+0\t0.000000E+0\t0.000000E+0\t0.000000E+0\t0.000000E+0\t0.000000E+0\t0.000000E+0\t0.000000E+0\t0.000000E+0\t0.000000E+0\t0.000000E+0\t0.000000E+0\t0.000000E+0\t0.000000E+0\t0.000000E+0\t0.000000E+0\t0.000000E+0\t0.000000E+0\t0.000000E+0\t0.000000E+0\t0.000000E+0\t0.000000E+0\t0.000000E+0\t0.000000E+0\t0.000000E+0\t0.000000E+0\r\n-1.020286E+0\t0.000000E+0\t0.000000E+0\t0.000000E+0\t0.000000E+0\t0.000000E+0\t0.000000E+0\t0.000000E+0\t0.000000E+0\t0.000000E+0\t0.000000E+0\t0.000000E+0\t0.000000E+0\t0.000000E+0\t0.000000E+0\t0.000000E+0\t0.000000E+0\t0.000000E+0\t0.000000E+0\t0.000000E+0\t0.000000E+0\t0.000000E+0\t0.000000E+0\t0.000000E+0\t0.000000E+0\t0.000000E+0\t0.000000E+0\t0.000000E+0\t0.000000E+0\t0.000000E+0\t0.000000E+0\t0.000000E+0\t0.000000E+0\t0.000000E+0\t0.000000E+0\t0.000000E+0\t0.000000E+0\t0.000000E+0\t0.000000E+0\t0.000000E+0\t0.000000E+0\t0.000000E+0\t0.000000E+0\t0.000000E+0\t0.000000E+0\t0.000000E+0\t0.000000E+0\t0.000000E+0\t0.000000E+0\t0.000000E+0\t0.000000E+0\t0.000000E+0\t0.000000E+0\t0.000000E+0\t0.000000E+0\t0.000000E+0\t0.000000E+0\t0.000000E+0\t0.000000E+0\t0.000000E+0\t0.000000E+0\t0.000000E+0\t0.000000E+0\t0.000000E+0\t0.000000E+0\t0.000000E+0\t0.000000E+0\t0.000000E+0\t0.000000E+0\t0.000000E+0\t0.000000E+0\t0.000000E+0\t0.000000E+0\t0.000000E+0\t0.000000E+0\t0.000000E+0\t0.000000E+0\t0.000000E+0\t0.000000E+0\t0.000000E+0\t0.000000E+0\t0.000000E+0\t0.000000E+0\t0.000000E+0\t0.000000E+0\t0.000000E+0\t0.000000E+0\t0.000000E+0\t0.000000E+0\t0.000000E+0\t0.000000E+0\t0.000000E+0\t0.000000E+0\t0.000000E+0\t0.000000E+0\t0.000000E+0\t0.000000E+0\t0.000000E+0\t0.000000E+0\t0.000000E+0\t0.000000E+0\r\n-9.753281E-1\t0.000000E+0\t0.000000E+0\t0.000000E+0\t0.000000E+0\t0.000000E+0\t0.000000E+0\t0.000000E+0\t0.000000E+0\t0.000000E+0\t0.000000E+0\t0.000000E+0\t0.000000E+0\t0.000000E+0\t0.000000E+0\t0.000000E+0\t0.000000E+0\t0.000000E+0\t0.000000E+0\t0.000000E+0\t0.000000E+0\t0.000000E+0\t0.000000E+0\t0.000000E+0\t0.000000E+0\t0.000000E+0\t0.000000E+0\t0.000000E+0\t0.000000E+0\t0.000000E+0\t0.000000E+0\t0.000000E+0\t0.000000E+0\t0.000000E+0\t0.000000E+0\t0.000000E+0\t0.000000E+0\t0.000000E+0\t0.000000E+0\t0.000000E+0\t0.000000E+0\t0.000000E+0\t0.000000E+0\t0.000000E+0\t0.000000E+0\t0.000000E+0\t0.000000E+0\t0.000000E+0\t0.000000E+0\t0.000000E+0\t0.000000E+0\t0.000000E+0\t0.000000E+0\t0.000000E+0\t0.000000E+0\t0.000000E+0\t0.000000E+0\t0.000000E+0\t0.000000E+0\t0.000000E+0\t0.000000E+0\t0.000000E+0\t0.000000E+0\t0.000000E+0\t0.000000E+0\t0.000000E+0\t0.000000E+0\t0.000000E+0\t0.000000E+0\t0.000000E+0\t0.000000E+0\t0.000000E+0\t0.000000E+0\t0.000000E+0\t0.000000E+0\t0.000000E+0\t0.000000E+0\t0.000000E+0\t0.000000E+0\t0.000000E+0\t0.000000E+0\t0.000000E+0\t0.000000E+0\t0.000000E+0\t0.000000E+0\t0.000000E+0\t0.000000E+0\t0.000000E+0\t0.000000E+0\t0.000000E+0\t0.000000E+0\t0.000000E+0\t0.000000E+0\t0.000000E+0\t0.000000E+0\t0.000000E+0\t0.000000E+0\t0.000000E+0\t0.000000E+0\t0.000000E+0\t0.000000E+0\r\n-9.303704E-1\t0.000000E+0\t0.000000E+0\t0.000000E+0\t0.000000E+0\t0.000000E+0\t0.000000E+0\t0.000000E+0\t0.000000E+0\t0.000000E+0\t0.000000E+0\t0.000000E+0\t0.000000E+0\t0.000000E+0\t0.000000E+0\t0.000000E+0\t0.000000E+0\t0.000000E+0\t0.000000E+0\t0.000000E+0\t0.000000E+0\t0.000000E+0\t0.000000E+0\t0.000000E+0\t0.000000E+0\t0.000000E+0\t0.000000E+0\t0.000000E+0\t0.000000E+0\t0.000000E+0\t0.000000E+0\t0.000000E+0\t0.000000E+0\t0.000000E+0\t0.000000E+0\t0.000000E+0\t0.000000E+0\t0.000000E+0\t0.000000E+0\t0.000000E+0\t0.000000E+0\t0.000000E+0\t0.000000E+0\t0.000000E+0\t0.000000E+0\t0.000000E+0\t0.000000E+0\t0.000000E+0\t0.000000E+0\t0.000000E+0\t0.000000E+0\t0.000000E+0\t0.000000E+0\t0.000000E+0\t0.000000E+0\t0.000000E+0\t0.000000E+0\t0.000000E+0\t0.000000E+0\t0.000000E+0\t0.000000E+0\t0.000000E+0\t0.000000E+0\t0.000000E+0\t0.000000E+0\t0.000000E+0\t0.000000E+0\t0.000000E+0\t0.000000E+0\t0.000000E+0\t0.000000E+0\t0.000000E+0\t0.000000E+0\t0.000000E+0\t0.000000E+0\t0.000000E+0\t0.000000E+0\t0.000000E+0\t0.000000E+0\t0.000000E+0\t0.000000E+0\t0.000000E+0\t0.000000E+0\t0.000000E+0\t0.000000E+0\t0.000000E+0\t0.000000E+0\t0.000000E+0\t0.000000E+0\t0.000000E+0\t0.000000E+0\t0.000000E+0\t0.000000E+0\t0.000000E+0\t0.000000E+0\t0.000000E+0\t0.000000E+0\t0.000000E+0\t0.000000E+0\t0.000000E+0\t0.000000E+0\r\n-8.854126E-1\t0.000000E+0\t0.000000E+0\t0.000000E+0\t0.000000E+0\t0.000000E+0\t0.000000E+0\t0.000000E+0\t0.000000E+0\t0.000000E+0\t0.000000E+0\t0.000000E+0\t0.000000E+0\t0.000000E+0\t0.000000E+0\t0.000000E+0\t0.000000E+0\t0.000000E+0\t0.000000E+0\t0.000000E+0\t0.000000E+0\t0.000000E+0\t0.000000E+0\t0.000000E+0\t0.000000E+0\t0.000000E+0\t0.000000E+0\t0.000000E+0\t0.000000E+0\t0.000000E+0\t0.000000E+0\t0.000000E+0\t0.000000E+0\t0.000000E+0\t0.000000E+0\t0.000000E+0\t0.000000E+0\t0.000000E+0\t0.000000E+0\t0.000000E+0\t0.000000E+0\t0.000000E+0\t0.000000E+0\t0.000000E+0\t0.000000E+0\t0.000000E+0\t0.000000E+0\t0.000000E+0\t0.000000E+0\t0.000000E+0\t0.000000E+0\t0.000000E+0\t0.000000E+0\t0.000000E+0\t0.000000E+0\t0.000000E+0\t0.000000E+0\t0.000000E+0\t0.000000E+0\t0.000000E+0\t0.000000E+0\t0.000000E+0\t0.000000E+0\t0.000000E+0\t0.000000E+0\t0.000000E+0\t0.000000E+0\t0.000000E+0\t0.000000E+0\t0.000000E+0\t0.000000E+0\t0.000000E+0\t0.000000E+0\t0.000000E+0\t0.000000E+0\t0.000000E+0\t0.000000E+0\t0.000000E+0\t0.000000E+0\t0.000000E+0\t0.000000E+0\t0.000000E+0\t0.000000E+0\t0.000000E+0\t0.000000E+0\t0.000000E+0\t0.000000E+0\t0.000000E+0\t0.000000E+0\t0.000000E+0\t0.000000E+0\t0.000000E+0\t0.000000E+0\t0.000000E+0\t0.000000E+0\t0.000000E+0\t0.000000E+0\t0.000000E+0\t0.000000E+0\t0.000000E+0\t0.000000E+0\r\n-8.404548E-1\t0.000000E+0\t0.000000E+0\t0.000000E+0\t0.000000E+0\t0.000000E+0\t0.000000E+0\t0.000000E+0\t0.000000E+0\t0.000000E+0\t0.000000E+0\t0.000000E+0\t0.000000E+0\t0.000000E+0\t0.000000E+0\t0.000000E+0\t0.000000E+0\t0.000000E+0\t0.000000E+0\t0.000000E+0\t0.000000E+0\t0.000000E+0\t0.000000E+0\t0.000000E+0\t0.000000E+0\t0.000000E+0\t0.000000E+0\t0.000000E+0\t0.000000E+0\t0.000000E+0\t0.000000E+0\t0.000000E+0\t0.000000E+0\t0.000000E+0\t0.000000E+0\t0.000000E+0\t0.000000E+0\t0.000000E+0\t0.000000E+0\t0.000000E+0\t0.000000E+0\t0.000000E+0\t0.000000E+0\t0.000000E+0\t0.000000E+0\t0.000000E+0\t0.000000E+0\t0.000000E+0\t0.000000E+0\t0.000000E+0\t0.000000E+0\t0.000000E+0\t0.000000E+0\t0.000000E+0\t0.000000E+0\t0.000000E+0\t0.000000E+0\t0.000000E+0\t0.000000E+0\t0.000000E+0\t0.000000E+0\t0.000000E+0\t0.000000E+0\t0.000000E+0\t0.000000E+0\t0.000000E+0\t0.000000E+0\t0.000000E+0\t0.000000E+0\t0.000000E+0\t0.000000E+0\t0.000000E+0\t0.000000E+0\t0.000000E+0\t0.000000E+0\t0.000000E+0\t0.000000E+0\t0.000000E+0\t0.000000E+0\t0.000000E+0\t0.000000E+0\t0.000000E+0\t0.000000E+0\t0.000000E+0\t0.000000E+0\t0.000000E+0\t0.000000E+0\t0.000000E+0\t0.000000E+0\t0.000000E+0\t0.000000E+0\t0.000000E+0\t0.000000E+0\t0.000000E+0\t0.000000E+0\t0.000000E+0\t0.000000E+0\t0.000000E+0\t0.000000E+0\t0.000000E+0\t0.000000E+0\r\n-7.954971E-1\t0.000000E+0\t0.000000E+0\t0.000000E+0\t0.000000E+0\t0.000000E+0\t0.000000E+0\t0.000000E+0\t0.000000E+0\t0.000000E+0\t0.000000E+0\t0.000000E+0\t0.000000E+0\t0.000000E+0\t0.000000E+0\t0.000000E+0\t0.000000E+0\t0.000000E+0\t0.000000E+0\t0.000000E+0\t0.000000E+0\t0.000000E+0\t0.000000E+0\t0.000000E+0\t0.000000E+0\t0.000000E+0\t0.000000E+0\t0.000000E+0\t0.000000E+0\t0.000000E+0\t0.000000E+0\t0.000000E+0\t0.000000E+0\t0.000000E+0\t0.000000E+0\t0.000000E+0\t0.000000E+0\t0.000000E+0\t0.000000E+0\t0.000000E+0\t0.000000E+0\t0.000000E+0\t0.000000E+0\t0.000000E+0\t0.000000E+0\t0.000000E+0\t0.000000E+0\t0.000000E+0\t0.000000E+0\t0.000000E+0\t0.000000E+0\t0.000000E+0\t0.000000E+0\t0.000000E+0\t0.000000E+0\t0.000000E+0\t0.000000E+0\t0.000000E+0\t0.000000E+0\t0.000000E+0\t0.000000E+0\t0.000000E+0\t0.000000E+0\t0.000000E+0\t0.000000E+0\t0.000000E+0\t0.000000E+0\t0.000000E+0\t0.000000E+0\t0.000000E+0\t0.000000E+0\t0.000000E+0\t0.000000E+0\t0.000000E+0\t0.000000E+0\t0.000000E+0\t0.000000E+0\t0.000000E+0\t0.000000E+0\t0.000000E+0\t0.000000E+0\t0.000000E+0\t0.000000E+0\t0.000000E+0\t0.000000E+0\t0.000000E+0\t0.000000E+0\t0.000000E+0\t0.000000E+0\t0.000000E+0\t0.000000E+0\t0.000000E+0\t0.000000E+0\t0.000000E+0\t0.000000E+0\t0.000000E+0\t0.000000E+0\t0.000000E+0\t0.000000E+0\t0.000000E+0\t0.000000E+0\r\n-7.505393E-1\t0.000000E+0\t0.000000E+0\t0.000000E+0\t0.000000E+0\t0.000000E+0\t0.000000E+0\t0.000000E+0\t0.000000E+0\t0.000000E+0\t0.000000E+0\t0.000000E+0\t0.000000E+0\t0.000000E+0\t0.000000E+0\t0.000000E+0\t0.000000E+0\t0.000000E+0\t0.000000E+0\t0.000000E+0\t0.000000E+0\t0.000000E+0\t0.000000E+0\t0.000000E+0\t0.000000E+0\t0.000000E+0\t0.000000E+0\t0.000000E+0\t0.000000E+0\t0.000000E+0\t0.000000E+0\t0.000000E+0\t0.000000E+0\t0.000000E+0\t0.000000E+0\t0.000000E+0\t0.000000E+0\t0.000000E+0\t0.000000E+0\t0.000000E+0\t0.000000E+0\t0.000000E+0\t0.000000E+0\t0.000000E+0\t0.000000E+0\t0.000000E+0\t0.000000E+0\t0.000000E+0\t0.000000E+0\t0.000000E+0\t0.000000E+0\t0.000000E+0\t0.000000E+0\t0.000000E+0\t0.000000E+0\t0.000000E+0\t0.000000E+0\t0.000000E+0\t0.000000E+0\t0.000000E+0\t0.000000E+0\t0.000000E+0\t0.000000E+0\t0.000000E+0\t0.000000E+0\t0.000000E+0\t0.000000E+0\t0.000000E+0\t0.000000E+0\t0.000000E+0\t0.000000E+0\t0.000000E+0\t0.000000E+0\t0.000000E+0\t0.000000E+0\t0.000000E+0\t0.000000E+0\t0.000000E+0\t0.000000E+0\t0.000000E+0\t0.000000E+0\t0.000000E+0\t0.000000E+0\t0.000000E+0\t0.000000E+0\t0.000000E+0\t0.000000E+0\t0.000000E+0\t0.000000E+0\t0.000000E+0\t0.000000E+0\t0.000000E+0\t0.000000E+0\t0.000000E+0\t0.000000E+0\t0.000000E+0\t0.000000E+0\t0.000000E+0\t0.000000E+0\t0.000000E+0\t0.000000E+0\r\n-7.055815E-1\t0.000000E+0\t0.000000E+0\t0.000000E+0\t0.000000E+0\t0.000000E+0\t0.000000E+0\t0.000000E+0\t0.000000E+0\t0.000000E+0\t0.000000E+0\t0.000000E+0\t0.000000E+0\t0.000000E+0\t0.000000E+0\t0.000000E+0\t0.000000E+0\t0.000000E+0\t0.000000E+0\t0.000000E+0\t0.000000E+0\t0.000000E+0\t0.000000E+0\t0.000000E+0\t0.000000E+0\t0.000000E+0\t0.000000E+0\t0.000000E+0\t0.000000E+0\t0.000000E+0\t0.000000E+0\t0.000000E+0\t0.000000E+0\t0.000000E+0\t0.000000E+0\t0.000000E+0\t0.000000E+0\t0.000000E+0\t0.000000E+0\t0.000000E+0\t0.000000E+0\t0.000000E+0\t0.000000E+0\t0.000000E+0\t0.000000E+0\t0.000000E+0\t0.000000E+0\t0.000000E+0\t0.000000E+0\t0.000000E+0\t0.000000E+0\t0.000000E+0\t0.000000E+0\t0.000000E+0\t0.000000E+0\t0.000000E+0\t0.000000E+0\t0.000000E+0\t0.000000E+0\t0.000000E+0\t0.000000E+0\t0.000000E+0\t0.000000E+0\t0.000000E+0\t0.000000E+0\t0.000000E+0\t0.000000E+0\t0.000000E+0\t0.000000E+0\t0.000000E+0\t0.000000E+0\t0.000000E+0\t0.000000E+0\t0.000000E+0\t0.000000E+0\t0.000000E+0\t0.000000E+0\t0.000000E+0\t0.000000E+0\t0.000000E+0\t0.000000E+0\t0.000000E+0\t0.000000E+0\t0.000000E+0\t0.000000E+0\t0.000000E+0\t0.000000E+0\t0.000000E+0\t0.000000E+0\t0.000000E+0\t0.000000E+0\t0.000000E+0\t0.000000E+0\t0.000000E+0\t0.000000E+0\t0.000000E+0\t0.000000E+0\t0.000000E+0\t0.000000E+0\t0.000000E+0\t0.000000E+0\r\n-6.606238E-1\t0.000000E+0\t0.000000E+0\t0.000000E+0\t0.000000E+0\t0.000000E+0\t0.000000E+0\t0.000000E+0\t0.000000E+0\t0.000000E+0\t0.000000E+0\t0.000000E+0\t0.000000E+0\t0.000000E+0\t0.000000E+0\t0.000000E+0\t0.000000E+0\t0.000000E+0\t0.000000E+0\t0.000000E+0\t0.000000E+0\t0.000000E+0\t0.000000E+0\t0.000000E+0\t0.000000E+0\t0.000000E+0\t0.000000E+0\t0.000000E+0\t0.000000E+0\t0.000000E+0\t0.000000E+0\t0.000000E+0\t0.000000E+0\t0.000000E+0\t0.000000E+0\t0.000000E+0\t0.000000E+0\t0.000000E+0\t0.000000E+0\t0.000000E+0\t0.000000E+0\t0.000000E+0\t0.000000E+0\t0.000000E+0\t0.000000E+0\t0.000000E+0\t0.000000E+0\t0.000000E+0\t0.000000E+0\t0.000000E+0\t0.000000E+0\t0.000000E+0\t0.000000E+0\t0.000000E+0\t0.000000E+0\t0.000000E+0\t0.000000E+0\t0.000000E+0\t0.000000E+0\t0.000000E+0\t0.000000E+0\t0.000000E+0\t0.000000E+0\t0.000000E+0\t0.000000E+0\t0.000000E+0\t0.000000E+0\t0.000000E+0\t0.000000E+0\t0.000000E+0\t0.000000E+0\t0.000000E+0\t0.000000E+0\t0.000000E+0\t0.000000E+0\t0.000000E+0\t0.000000E+0\t0.000000E+0\t0.000000E+0\t0.000000E+0\t0.000000E+0\t0.000000E+0\t0.000000E+0\t0.000000E+0\t0.000000E+0\t0.000000E+0\t0.000000E+0\t0.000000E+0\t0.000000E+0\t0.000000E+0\t0.000000E+0\t0.000000E+0\t0.000000E+0\t0.000000E+0\t0.000000E+0\t0.000000E+0\t0.000000E+0\t0.000000E+0\t0.000000E+0\t0.000000E+0\t0.000000E+0\r\n-6.156660E-1\t0.000000E+0\t0.000000E+0\t0.000000E+0\t0.000000E+0\t0.000000E+0\t0.000000E+0\t0.000000E+0\t0.000000E+0\t0.000000E+0\t0.000000E+0\t0.000000E+0\t0.000000E+0\t0.000000E+0\t0.000000E+0\t0.000000E+0\t0.000000E+0\t0.000000E+0\t0.000000E+0\t0.000000E+0\t0.000000E+0\t0.000000E+0\t0.000000E+0\t0.000000E+0\t0.000000E+0\t0.000000E+0\t0.000000E+0\t0.000000E+0\t0.000000E+0\t0.000000E+0\t0.000000E+0\t0.000000E+0\t0.000000E+0\t0.000000E+0\t0.000000E+0\t0.000000E+0\t0.000000E+0\t0.000000E+0\t0.000000E+0\t0.000000E+0\t0.000000E+0\t0.000000E+0\t0.000000E+0\t0.000000E+0\t0.000000E+0\t0.000000E+0\t0.000000E+0\t0.000000E+0\t0.000000E+0\t0.000000E+0\t0.000000E+0\t0.000000E+0\t0.000000E+0\t0.000000E+0\t0.000000E+0\t0.000000E+0\t0.000000E+0\t0.000000E+0\t0.000000E+0\t0.000000E+0\t0.000000E+0\t0.000000E+0\t0.000000E+0\t0.000000E+0\t0.000000E+0\t0.000000E+0\t0.000000E+0\t0.000000E+0\t0.000000E+0\t0.000000E+0\t0.000000E+0\t0.000000E+0\t0.000000E+0\t0.000000E+0\t0.000000E+0\t0.000000E+0\t0.000000E+0\t0.000000E+0\t0.000000E+0\t0.000000E+0\t0.000000E+0\t0.000000E+0\t0.000000E+0\t0.000000E+0\t0.000000E+0\t0.000000E+0\t0.000000E+0\t0.000000E+0\t0.000000E+0\t0.000000E+0\t0.000000E+0\t0.000000E+0\t0.000000E+0\t0.000000E+0\t0.000000E+0\t0.000000E+0\t0.000000E+0\t0.000000E+0\t0.000000E+0\t0.000000E+0\t0.000000E+0\r\n-5.707082E-1\t0.000000E+0\t0.000000E+0\t0.000000E+0\t0.000000E+0\t0.000000E+0\t0.000000E+0\t0.000000E+0\t0.000000E+0\t0.000000E+0\t0.000000E+0\t0.000000E+0\t0.000000E+0\t0.000000E+0\t0.000000E+0\t0.000000E+0\t0.000000E+0\t0.000000E+0\t0.000000E+0\t0.000000E+0\t0.000000E+0\t0.000000E+0\t0.000000E+0\t0.000000E+0\t0.000000E+0\t0.000000E+0\t0.000000E+0\t0.000000E+0\t0.000000E+0\t0.000000E+0\t0.000000E+0\t0.000000E+0\t0.000000E+0\t0.000000E+0\t0.000000E+0\t0.000000E+0\t0.000000E+0\t0.000000E+0\t0.000000E+0\t0.000000E+0\t0.000000E+0\t0.000000E+0\t0.000000E+0\t0.000000E+0\t0.000000E+0\t0.000000E+0\t0.000000E+0\t0.000000E+0\t0.000000E+0\t0.000000E+0\t0.000000E+0\t0.000000E+0\t0.000000E+0\t0.000000E+0\t0.000000E+0\t0.000000E+0\t0.000000E+0\t0.000000E+0\t0.000000E+0\t0.000000E+0\t0.000000E+0\t0.000000E+0\t0.000000E+0\t0.000000E+0\t0.000000E+0\t0.000000E+0\t0.000000E+0\t0.000000E+0\t0.000000E+0\t0.000000E+0\t0.000000E+0\t0.000000E+0\t0.000000E+0\t0.000000E+0\t0.000000E+0\t0.000000E+0\t0.000000E+0\t0.000000E+0\t0.000000E+0\t0.000000E+0\t0.000000E+0\t0.000000E+0\t0.000000E+0\t0.000000E+0\t0.000000E+0\t0.000000E+0\t0.000000E+0\t0.000000E+0\t0.000000E+0\t0.000000E+0\t0.000000E+0\t0.000000E+0\t0.000000E+0\t0.000000E+0\t0.000000E+0\t0.000000E+0\t0.000000E+0\t0.000000E+0\t0.000000E+0\t0.000000E+0\t0.000000E+0\r\n-5.257505E-1\t0.000000E+0\t0.000000E+0\t0.000000E+0\t0.000000E+0\t0.000000E+0\t0.000000E+0\t0.000000E+0\t0.000000E+0\t0.000000E+0\t0.000000E+0\t0.000000E+0\t0.000000E+0\t0.000000E+0\t0.000000E+0\t0.000000E+0\t0.000000E+0\t0.000000E+0\t0.000000E+0\t0.000000E+0\t0.000000E+0\t0.000000E+0\t0.000000E+0\t0.000000E+0\t0.000000E+0\t0.000000E+0\t0.000000E+0\t0.000000E+0\t0.000000E+0\t0.000000E+0\t0.000000E+0\t0.000000E+0\t0.000000E+0\t0.000000E+0\t0.000000E+0\t0.000000E+0\t0.000000E+0\t0.000000E+0\t0.000000E+0\t0.000000E+0\t0.000000E+0\t0.000000E+0\t0.000000E+0\t0.000000E+0\t0.000000E+0\t0.000000E+0\t0.000000E+0\t0.000000E+0\t0.000000E+0\t0.000000E+0\t0.000000E+0\t0.000000E+0\t0.000000E+0\t0.000000E+0\t0.000000E+0\t0.000000E+0\t0.000000E+0\t0.000000E+0\t0.000000E+0\t0.000000E+0\t0.000000E+0\t0.000000E+0\t0.000000E+0\t0.000000E+0\t0.000000E+0\t0.000000E+0\t0.000000E+0\t0.000000E+0\t0.000000E+0\t0.000000E+0\t0.000000E+0\t0.000000E+0\t0.000000E+0\t0.000000E+0\t0.000000E+0\t0.000000E+0\t0.000000E+0\t0.000000E+0\t0.000000E+0\t0.000000E+0\t0.000000E+0\t0.000000E+0\t0.000000E+0\t0.000000E+0\t0.000000E+0\t0.000000E+0\t0.000000E+0\t0.000000E+0\t0.000000E+0\t0.000000E+0\t0.000000E+0\t0.000000E+0\t0.000000E+0\t0.000000E+0\t0.000000E+0\t0.000000E+0\t0.000000E+0\t0.000000E+0\t0.000000E+0\t0.000000E+0\t0.000000E+0\r\n-4.807927E-1\t0.000000E+0\t0.000000E+0\t0.000000E+0\t0.000000E+0\t0.000000E+0\t0.000000E+0\t0.000000E+0\t0.000000E+0\t0.000000E+0\t0.000000E+0\t0.000000E+0\t0.000000E+0\t0.000000E+0\t0.000000E+0\t0.000000E+0\t0.000000E+0\t0.000000E+0\t0.000000E+0\t0.000000E+0\t0.000000E+0\t0.000000E+0\t0.000000E+0\t0.000000E+0\t0.000000E+0\t0.000000E+0\t0.000000E+0\t0.000000E+0\t0.000000E+0\t0.000000E+0\t0.000000E+0\t0.000000E+0\t0.000000E+0\t0.000000E+0\t0.000000E+0\t0.000000E+0\t0.000000E+0\t0.000000E+0\t0.000000E+0\t0.000000E+0\t0.000000E+0\t0.000000E+0\t0.000000E+0\t0.000000E+0\t0.000000E+0\t0.000000E+0\t0.000000E+0\t0.000000E+0\t0.000000E+0\t0.000000E+0\t0.000000E+0\t0.000000E+0\t0.000000E+0\t0.000000E+0\t0.000000E+0\t0.000000E+0\t0.000000E+0\t0.000000E+0\t0.000000E+0\t0.000000E+0\t0.000000E+0\t0.000000E+0\t0.000000E+0\t0.000000E+0\t0.000000E+0\t0.000000E+0\t0.000000E+0\t0.000000E+0\t0.000000E+0\t0.000000E+0\t0.000000E+0\t0.000000E+0\t0.000000E+0\t0.000000E+0\t0.000000E+0\t0.000000E+0\t0.000000E+0\t0.000000E+0\t0.000000E+0\t0.000000E+0\t0.000000E+0\t0.000000E+0\t0.000000E+0\t0.000000E+0\t0.000000E+0\t0.000000E+0\t0.000000E+0\t0.000000E+0\t0.000000E+0\t0.000000E+0\t0.000000E+0\t0.000000E+0\t0.000000E+0\t0.000000E+0\t0.000000E+0\t0.000000E+0\t0.000000E+0\t0.000000E+0\t0.000000E+0\t0.000000E+0\t0.000000E+0\r\n-4.358349E-1\t0.000000E+0\t0.000000E+0\t0.000000E+0\t0.000000E+0\t0.000000E+0\t0.000000E+0\t0.000000E+0\t0.000000E+0\t0.000000E+0\t0.000000E+0\t0.000000E+0\t0.000000E+0\t0.000000E+0\t0.000000E+0\t0.000000E+0\t0.000000E+0\t0.000000E+0\t0.000000E+0\t0.000000E+0\t0.000000E+0\t0.000000E+0\t0.000000E+0\t0.000000E+0\t0.000000E+0\t0.000000E+0\t0.000000E+0\t0.000000E+0\t0.000000E+0\t0.000000E+0\t0.000000E+0\t0.000000E+0\t0.000000E+0\t0.000000E+0\t0.000000E+0\t0.000000E+0\t0.000000E+0\t0.000000E+0\t0.000000E+0\t0.000000E+0\t0.000000E+0\t0.000000E+0\t0.000000E+0\t0.000000E+0\t0.000000E+0\t0.000000E+0\t0.000000E+0\t0.000000E+0\t0.000000E+0\t0.000000E+0\t0.000000E+0\t0.000000E+0\t0.000000E+0\t0.000000E+0\t0.000000E+0\t0.000000E+0\t0.000000E+0\t0.000000E+0\t0.000000E+0\t0.000000E+0\t0.000000E+0\t0.000000E+0\t0.000000E+0\t0.000000E+0\t0.000000E+0\t0.000000E+0\t0.000000E+0\t0.000000E+0\t0.000000E+0\t0.000000E+0\t0.000000E+0\t0.000000E+0\t0.000000E+0\t0.000000E+0\t0.000000E+0\t0.000000E+0\t0.000000E+0\t0.000000E+0\t0.000000E+0\t0.000000E+0\t0.000000E+0\t0.000000E+0\t0.000000E+0\t0.000000E+0\t0.000000E+0\t0.000000E+0\t0.000000E+0\t0.000000E+0\t0.000000E+0\t0.000000E+0\t0.000000E+0\t0.000000E+0\t0.000000E+0\t0.000000E+0\t0.000000E+0\t0.000000E+0\t0.000000E+0\t0.000000E+0\t0.000000E+0\t0.000000E+0\t0.000000E+0\r\n-3.908772E-1\t0.000000E+0\t0.000000E+0\t0.000000E+0\t0.000000E+0\t0.000000E+0\t0.000000E+0\t0.000000E+0\t0.000000E+0\t0.000000E+0\t0.000000E+0\t0.000000E+0\t0.000000E+0\t0.000000E+0\t0.000000E+0\t0.000000E+0\t0.000000E+0\t0.000000E+0\t0.000000E+0\t0.000000E+0\t0.000000E+0\t0.000000E+0\t0.000000E+0\t0.000000E+0\t0.000000E+0\t0.000000E+0\t0.000000E+0\t0.000000E+0\t0.000000E+0\t0.000000E+0\t0.000000E+0\t0.000000E+0\t0.000000E+0\t0.000000E+0\t0.000000E+0\t0.000000E+0\t0.000000E+0\t0.000000E+0\t0.000000E+0\t0.000000E+0\t0.000000E+0\t0.000000E+0\t0.000000E+0\t0.000000E+0\t0.000000E+0\t0.000000E+0\t0.000000E+0\t0.000000E+0\t0.000000E+0\t0.000000E+0\t0.000000E+0\t0.000000E+0\t0.000000E+0\t0.000000E+0\t0.000000E+0\t0.000000E+0\t0.000000E+0\t0.000000E+0\t0.000000E+0\t0.000000E+0\t0.000000E+0\t0.000000E+0\t0.000000E+0\t0.000000E+0\t0.000000E+0\t0.000000E+0\t0.000000E+0\t0.000000E+0\t0.000000E+0\t0.000000E+0\t0.000000E+0\t0.000000E+0\t0.000000E+0\t0.000000E+0\t0.000000E+0\t0.000000E+0\t0.000000E+0\t0.000000E+0\t0.000000E+0\t0.000000E+0\t0.000000E+0\t0.000000E+0\t0.000000E+0\t0.000000E+0\t0.000000E+0\t0.000000E+0\t0.000000E+0\t0.000000E+0\t0.000000E+0\t0.000000E+0\t0.000000E+0\t0.000000E+0\t0.000000E+0\t0.000000E+0\t0.000000E+0\t0.000000E+0\t0.000000E+0\t0.000000E+0\t0.000000E+0\t0.000000E+0\t0.000000E+0\r\n-3.459194E-1\t0.000000E+0\t0.000000E+0\t0.000000E+0\t0.000000E+0\t0.000000E+0\t0.000000E+0\t0.000000E+0\t0.000000E+0\t0.000000E+0\t0.000000E+0\t0.000000E+0\t0.000000E+0\t0.000000E+0\t0.000000E+0\t0.000000E+0\t0.000000E+0\t0.000000E+0\t0.000000E+0\t0.000000E+0\t0.000000E+0\t0.000000E+0\t0.000000E+0\t0.000000E+0\t0.000000E+0\t0.000000E+0\t0.000000E+0\t0.000000E+0\t0.000000E+0\t0.000000E+0\t0.000000E+0\t0.000000E+0\t0.000000E+0\t0.000000E+0\t0.000000E+0\t0.000000E+0\t0.000000E+0\t0.000000E+0\t0.000000E+0\t0.000000E+0\t0.000000E+0\t0.000000E+0\t0.000000E+0\t0.000000E+0\t0.000000E+0\t0.000000E+0\t0.000000E+0\t0.000000E+0\t0.000000E+0\t0.000000E+0\t0.000000E+0\t0.000000E+0\t0.000000E+0\t0.000000E+0\t0.000000E+0\t0.000000E+0\t0.000000E+0\t0.000000E+0\t0.000000E+0\t0.000000E+0\t0.000000E+0\t0.000000E+0\t0.000000E+0\t0.000000E+0\t0.000000E+0\t0.000000E+0\t0.000000E+0\t0.000000E+0\t0.000000E+0\t0.000000E+0\t0.000000E+0\t0.000000E+0\t0.000000E+0\t0.000000E+0\t0.000000E+0\t0.000000E+0\t0.000000E+0\t0.000000E+0\t0.000000E+0\t0.000000E+0\t0.000000E+0\t0.000000E+0\t0.000000E+0\t0.000000E+0\t0.000000E+0\t0.000000E+0\t0.000000E+0\t0.000000E+0\t0.000000E+0\t0.000000E+0\t0.000000E+0\t0.000000E+0\t0.000000E+0\t0.000000E+0\t0.000000E+0\t0.000000E+0\t0.000000E+0\t0.000000E+0\t0.000000E+0\t0.000000E+0\t0.000000E+0\r\n-3.009616E-1\t0.000000E+0\t0.000000E+0\t0.000000E+0\t0.000000E+0\t0.000000E+0\t0.000000E+0\t0.000000E+0\t0.000000E+0\t0.000000E+0\t0.000000E+0\t0.000000E+0\t0.000000E+0\t0.000000E+0\t0.000000E+0\t0.000000E+0\t0.000000E+0\t0.000000E+0\t0.000000E+0\t0.000000E+0\t0.000000E+0\t0.000000E+0\t0.000000E+0\t0.000000E+0\t0.000000E+0\t0.000000E+0\t0.000000E+0\t0.000000E+0\t0.000000E+0\t0.000000E+0\t0.000000E+0\t0.000000E+0\t0.000000E+0\t0.000000E+0\t0.000000E+0\t0.000000E+0\t0.000000E+0\t0.000000E+0\t0.000000E+0\t0.000000E+0\t0.000000E+0\t0.000000E+0\t0.000000E+0\t0.000000E+0\t0.000000E+0\t0.000000E+0\t0.000000E+0\t0.000000E+0\t0.000000E+0\t0.000000E+0\t0.000000E+0\t0.000000E+0\t0.000000E+0\t0.000000E+0\t0.000000E+0\t0.000000E+0\t0.000000E+0\t0.000000E+0\t0.000000E+0\t0.000000E+0\t0.000000E+0\t0.000000E+0\t0.000000E+0\t0.000000E+0\t0.000000E+0\t0.000000E+0\t0.000000E+0\t0.000000E+0\t0.000000E+0\t0.000000E+0\t0.000000E+0\t0.000000E+0\t0.000000E+0\t0.000000E+0\t0.000000E+0\t0.000000E+0\t0.000000E+0\t0.000000E+0\t0.000000E+0\t0.000000E+0\t0.000000E+0\t0.000000E+0\t0.000000E+0\t0.000000E+0\t0.000000E+0\t0.000000E+0\t0.000000E+0\t0.000000E+0\t0.000000E+0\t0.000000E+0\t0.000000E+0\t0.000000E+0\t0.000000E+0\t0.000000E+0\t0.000000E+0\t0.000000E+0\t0.000000E+0\t0.000000E+0\t0.000000E+0\t0.000000E+0\t0.000000E+0\r\n-2.560039E-1\t0.000000E+0\t0.000000E+0\t0.000000E+0\t0.000000E+0\t0.000000E+0\t0.000000E+0\t0.000000E+0\t0.000000E+0\t0.000000E+0\t0.000000E+0\t0.000000E+0\t0.000000E+0\t0.000000E+0\t0.000000E+0\t0.000000E+0\t0.000000E+0\t0.000000E+0\t0.000000E+0\t0.000000E+0\t0.000000E+0\t0.000000E+0\t0.000000E+0\t0.000000E+0\t0.000000E+0\t0.000000E+0\t0.000000E+0\t0.000000E+0\t0.000000E+0\t0.000000E+0\t0.000000E+0\t0.000000E+0\t0.000000E+0\t0.000000E+0\t0.000000E+0\t0.000000E+0\t0.000000E+0\t0.000000E+0\t0.000000E+0\t0.000000E+0\t0.000000E+0\t0.000000E+0\t0.000000E+0\t0.000000E+0\t0.000000E+0\t0.000000E+0\t0.000000E+0\t0.000000E+0\t0.000000E+0\t0.000000E+0\t0.000000E+0\t0.000000E+0\t0.000000E+0\t0.000000E+0\t0.000000E+0\t0.000000E+0\t0.000000E+0\t0.000000E+0\t0.000000E+0\t0.000000E+0\t0.000000E+0\t0.000000E+0\t0.000000E+0\t0.000000E+0\t0.000000E+0\t0.000000E+0\t0.000000E+0\t0.000000E+0\t0.000000E+0\t0.000000E+0\t0.000000E+0\t0.000000E+0\t0.000000E+0\t0.000000E+0\t0.000000E+0\t0.000000E+0\t0.000000E+0\t0.000000E+0\t0.000000E+0\t0.000000E+0\t0.000000E+0\t0.000000E+0\t0.000000E+0\t0.000000E+0\t0.000000E+0\t0.000000E+0\t0.000000E+0\t0.000000E+0\t0.000000E+0\t0.000000E+0\t0.000000E+0\t0.000000E+0\t0.000000E+0\t0.000000E+0\t0.000000E+0\t0.000000E+0\t0.000000E+0\t0.000000E+0\t0.000000E+0\t0.000000E+0\t0.000000E+0\r\n-2.110461E-1\t0.000000E+0\t0.000000E+0\t0.000000E+0\t0.000000E+0\t0.000000E+0\t0.000000E+0\t0.000000E+0\t0.000000E+0\t0.000000E+0\t0.000000E+0\t0.000000E+0\t0.000000E+0\t0.000000E+0\t0.000000E+0\t0.000000E+0\t0.000000E+0\t0.000000E+0\t0.000000E+0\t0.000000E+0\t0.000000E+0\t0.000000E+0\t0.000000E+0\t0.000000E+0\t0.000000E+0\t0.000000E+0\t0.000000E+0\t0.000000E+0\t0.000000E+0\t0.000000E+0\t0.000000E+0\t0.000000E+0\t0.000000E+0\t0.000000E+0\t0.000000E+0\t0.000000E+0\t0.000000E+0\t0.000000E+0\t0.000000E+0\t0.000000E+0\t0.000000E+0\t0.000000E+0\t0.000000E+0\t0.000000E+0\t0.000000E+0\t0.000000E+0\t0.000000E+0\t0.000000E+0\t0.000000E+0\t0.000000E+0\t0.000000E+0\t0.000000E+0\t0.000000E+0\t0.000000E+0\t0.000000E+0\t0.000000E+0\t0.000000E+0\t0.000000E+0\t0.000000E+0\t0.000000E+0\t0.000000E+0\t0.000000E+0\t0.000000E+0\t0.000000E+0\t0.000000E+0\t0.000000E+0\t0.000000E+0\t0.000000E+0\t0.000000E+0\t0.000000E+0\t0.000000E+0\t0.000000E+0\t0.000000E+0\t0.000000E+0\t0.000000E+0\t0.000000E+0\t0.000000E+0\t0.000000E+0\t0.000000E+0\t0.000000E+0\t0.000000E+0\t0.000000E+0\t0.000000E+0\t0.000000E+0\t0.000000E+0\t0.000000E+0\t0.000000E+0\t0.000000E+0\t0.000000E+0\t0.000000E+0\t0.000000E+0\t0.000000E+0\t0.000000E+0\t0.000000E+0\t0.000000E+0\t0.000000E+0\t0.000000E+0\t0.000000E+0\t0.000000E+0\t0.000000E+0\t0.000000E+0\r\n-1.660883E-1\t0.000000E+0\t0.000000E+0\t0.000000E+0\t0.000000E+0\t0.000000E+0\t0.000000E+0\t0.000000E+0\t0.000000E+0\t0.000000E+0\t0.000000E+0\t0.000000E+0\t0.000000E+0\t0.000000E+0\t0.000000E+0\t0.000000E+0\t0.000000E+0\t0.000000E+0\t0.000000E+0\t0.000000E+0\t0.000000E+0\t0.000000E+0\t0.000000E+0\t0.000000E+0\t0.000000E+0\t0.000000E+0\t0.000000E+0\t0.000000E+0\t0.000000E+0\t0.000000E+0\t0.000000E+0\t0.000000E+0\t0.000000E+0\t0.000000E+0\t0.000000E+0\t0.000000E+0\t0.000000E+0\t0.000000E+0\t0.000000E+0\t0.000000E+0\t0.000000E+0\t0.000000E+0\t0.000000E+0\t0.000000E+0\t0.000000E+0\t0.000000E+0\t0.000000E+0\t0.000000E+0\t0.000000E+0\t0.000000E+0\t0.000000E+0\t0.000000E+0\t0.000000E+0\t0.000000E+0\t0.000000E+0\t0.000000E+0\t0.000000E+0\t0.000000E+0\t0.000000E+0\t0.000000E+0\t0.000000E+0\t0.000000E+0\t0.000000E+0\t0.000000E+0\t0.000000E+0\t0.000000E+0\t0.000000E+0\t0.000000E+0\t0.000000E+0\t0.000000E+0\t0.000000E+0\t0.000000E+0\t0.000000E+0\t0.000000E+0\t0.000000E+0\t0.000000E+0\t0.000000E+0\t0.000000E+0\t0.000000E+0\t0.000000E+0\t0.000000E+0\t0.000000E+0\t0.000000E+0\t0.000000E+0\t0.000000E+0\t0.000000E+0\t0.000000E+0\t0.000000E+0\t0.000000E+0\t0.000000E+0\t0.000000E+0\t0.000000E+0\t0.000000E+0\t0.000000E+0\t0.000000E+0\t0.000000E+0\t0.000000E+0\t0.000000E+0\t0.000000E+0\t0.000000E+0\t0.000000E+0\r\n-1.211306E-1\t0.000000E+0\t0.000000E+0\t0.000000E+0\t0.000000E+0\t0.000000E+0\t0.000000E+0\t0.000000E+0\t0.000000E+0\t0.000000E+0\t0.000000E+0\t0.000000E+0\t0.000000E+0\t0.000000E+0\t0.000000E+0\t0.000000E+0\t0.000000E+0\t0.000000E+0\t0.000000E+0\t0.000000E+0\t0.000000E+0\t0.000000E+0\t0.000000E+0\t0.000000E+0\t0.000000E+0\t0.000000E+0\t0.000000E+0\t0.000000E+0\t0.000000E+0\t0.000000E+0\t0.000000E+0\t0.000000E+0\t0.000000E+0\t0.000000E+0\t0.000000E+0\t0.000000E+0\t0.000000E+0\t0.000000E+0\t0.000000E+0\t0.000000E+0\t0.000000E+0\t0.000000E+0\t0.000000E+0\t0.000000E+0\t0.000000E+0\t0.000000E+0\t0.000000E+0\t0.000000E+0\t0.000000E+0\t0.000000E+0\t0.000000E+0\t0.000000E+0\t0.000000E+0\t0.000000E+0\t0.000000E+0\t0.000000E+0\t0.000000E+0\t0.000000E+0\t0.000000E+0\t0.000000E+0\t0.000000E+0\t0.000000E+0\t0.000000E+0\t0.000000E+0\t0.000000E+0\t0.000000E+0\t0.000000E+0\t0.000000E+0\t0.000000E+0\t0.000000E+0\t0.000000E+0\t0.000000E+0\t0.000000E+0\t0.000000E+0\t0.000000E+0\t0.000000E+0\t0.000000E+0\t0.000000E+0\t0.000000E+0\t0.000000E+0\t0.000000E+0\t0.000000E+0\t0.000000E+0\t0.000000E+0\t0.000000E+0\t0.000000E+0\t0.000000E+0\t0.000000E+0\t0.000000E+0\t0.000000E+0\t0.000000E+0\t0.000000E+0\t0.000000E+0\t0.000000E+0\t0.000000E+0\t0.000000E+0\t0.000000E+0\t0.000000E+0\t0.000000E+0\t0.000000E+0\t0.000000E+0\r\n-7.617280E-2\t0.000000E+0\t0.000000E+0\t0.000000E+0\t0.000000E+0\t0.000000E+0\t0.000000E+0\t0.000000E+0\t0.000000E+0\t0.000000E+0\t0.000000E+0\t0.000000E+0\t0.000000E+0\t0.000000E+0\t0.000000E+0\t0.000000E+0\t0.000000E+0\t0.000000E+0\t0.000000E+0\t0.000000E+0\t0.000000E+0\t0.000000E+0\t0.000000E+0\t0.000000E+0\t0.000000E+0\t0.000000E+0\t0.000000E+0\t0.000000E+0\t0.000000E+0\t0.000000E+0\t0.000000E+0\t0.000000E+0\t0.000000E+0\t0.000000E+0\t0.000000E+0\t0.000000E+0\t0.000000E+0\t0.000000E+0\t0.000000E+0\t0.000000E+0\t0.000000E+0\t0.000000E+0\t0.000000E+0\t0.000000E+0\t0.000000E+0\t0.000000E+0\t0.000000E+0\t0.000000E+0\t0.000000E+0\t0.000000E+0\t0.000000E+0\t0.000000E+0\t0.000000E+0\t0.000000E+0\t0.000000E+0\t0.000000E+0\t0.000000E+0\t0.000000E+0\t0.000000E+0\t0.000000E+0\t0.000000E+0\t0.000000E+0\t0.000000E+0\t0.000000E+0\t0.000000E+0\t0.000000E+0\t0.000000E+0\t0.000000E+0\t0.000000E+0\t0.000000E+0\t0.000000E+0\t0.000000E+0\t0.000000E+0\t0.000000E+0\t0.000000E+0\t0.000000E+0\t0.000000E+0\t0.000000E+0\t0.000000E+0\t0.000000E+0\t0.000000E+0\t0.000000E+0\t0.000000E+0\t0.000000E+0\t0.000000E+0\t0.000000E+0\t0.000000E+0\t0.000000E+0\t0.000000E+0\t0.000000E+0\t0.000000E+0\t0.000000E+0\t0.000000E+0\t0.000000E+0\t0.000000E+0\t0.000000E+0\t0.000000E+0\t0.000000E+0\t0.000000E+0\t0.000000E+0\t0.000000E+0\r\n-3.121503E-2\t0.000000E+0\t0.000000E+0\t0.000000E+0\t0.000000E+0\t0.000000E+0\t0.000000E+0\t0.000000E+0\t0.000000E+0\t0.000000E+0\t0.000000E+0\t0.000000E+0\t0.000000E+0\t0.000000E+0\t0.000000E+0\t0.000000E+0\t0.000000E+0\t0.000000E+0\t0.000000E+0\t0.000000E+0\t0.000000E+0\t0.000000E+0\t0.000000E+0\t0.000000E+0\t0.000000E+0\t0.000000E+0\t0.000000E+0\t0.000000E+0\t0.000000E+0\t0.000000E+0\t0.000000E+0\t0.000000E+0\t0.000000E+0\t0.000000E+0\t0.000000E+0\t0.000000E+0\t0.000000E+0\t0.000000E+0\t0.000000E+0\t0.000000E+0\t0.000000E+0\t0.000000E+0\t0.000000E+0\t0.000000E+0\t0.000000E+0\t0.000000E+0\t0.000000E+0\t0.000000E+0\t0.000000E+0\t0.000000E+0\t0.000000E+0\t0.000000E+0\t0.000000E+0\t0.000000E+0\t0.000000E+0\t0.000000E+0\t0.000000E+0\t0.000000E+0\t0.000000E+0\t0.000000E+0\t0.000000E+0\t0.000000E+0\t0.000000E+0\t0.000000E+0\t0.000000E+0\t0.000000E+0\t0.000000E+0\t0.000000E+0\t0.000000E+0\t0.000000E+0\t0.000000E+0\t0.000000E+0\t0.000000E+0\t0.000000E+0\t0.000000E+0\t0.000000E+0\t0.000000E+0\t0.000000E+0\t0.000000E+0\t0.000000E+0\t0.000000E+0\t0.000000E+0\t0.000000E+0\t0.000000E+0\t0.000000E+0\t0.000000E+0\t0.000000E+0\t0.000000E+0\t0.000000E+0\t0.000000E+0\t0.000000E+0\t0.000000E+0\t0.000000E+0\t0.000000E+0\t0.000000E+0\t0.000000E+0\t0.000000E+0\t0.000000E+0\t0.000000E+0\t0.000000E+0\t0.000000E+0\r\n1.374274E-2\t0.000000E+0\t0.000000E+0\t0.000000E+0\t0.000000E+0\t0.000000E+0\t0.000000E+0\t0.000000E+0\t0.000000E+0\t0.000000E+0\t0.000000E+0\t0.000000E+0\t0.000000E+0\t0.000000E+0\t0.000000E+0\t0.000000E+0\t0.000000E+0\t0.000000E+0\t0.000000E+0\t0.000000E+0\t0.000000E+0\t0.000000E+0\t0.000000E+0\t0.000000E+0\t0.000000E+0\t0.000000E+0\t0.000000E+0\t0.000000E+0\t0.000000E+0\t0.000000E+0\t0.000000E+0\t0.000000E+0\t0.000000E+0\t0.000000E+0\t0.000000E+0\t0.000000E+0\t0.000000E+0\t0.000000E+0\t0.000000E+0\t0.000000E+0\t0.000000E+0\t0.000000E+0\t0.000000E+0\t0.000000E+0\t0.000000E+0\t0.000000E+0\t0.000000E+0\t0.000000E+0\t0.000000E+0\t0.000000E+0\t0.000000E+0\t0.000000E+0\t0.000000E+0\t0.000000E+0\t0.000000E+0\t0.000000E+0\t0.000000E+0\t0.000000E+0\t0.000000E+0\t0.000000E+0\t0.000000E+0\t0.000000E+0\t0.000000E+0\t0.000000E+0\t0.000000E+0\t0.000000E+0\t0.000000E+0\t0.000000E+0\t0.000000E+0\t0.000000E+0\t0.000000E+0\t0.000000E+0\t0.000000E+0\t0.000000E+0\t0.000000E+0\t0.000000E+0\t0.000000E+0\t0.000000E+0\t0.000000E+0\t0.000000E+0\t0.000000E+0\t0.000000E+0\t0.000000E+0\t0.000000E+0\t0.000000E+0\t0.000000E+0\t0.000000E+0\t0.000000E+0\t0.000000E+0\t0.000000E+0\t0.000000E+0\t0.000000E+0\t0.000000E+0\t0.000000E+0\t0.000000E+0\t0.000000E+0\t0.000000E+0\t0.000000E+0\t0.000000E+0\t0.000000E+0\t0.000000E+0\r\n5.870050E-2\t0.000000E+0\t0.000000E+0\t0.000000E+0\t0.000000E+0\t0.000000E+0\t0.000000E+0\t0.000000E+0\t0.000000E+0\t0.000000E+0\t0.000000E+0\t0.000000E+0\t0.000000E+0\t0.000000E+0\t0.000000E+0\t0.000000E+0\t0.000000E+0\t0.000000E+0\t0.000000E+0\t0.000000E+0\t0.000000E+0\t0.000000E+0\t0.000000E+0\t0.000000E+0\t0.000000E+0\t0.000000E+0\t0.000000E+0\t0.000000E+0\t0.000000E+0\t0.000000E+0\t0.000000E+0\t0.000000E+0\t0.000000E+0\t0.000000E+0\t0.000000E+0\t0.000000E+0\t0.000000E+0\t0.000000E+0\t0.000000E+0\t0.000000E+0\t0.000000E+0\t0.000000E+0\t0.000000E+0\t0.000000E+0\t0.000000E+0\t0.000000E+0\t0.000000E+0\t0.000000E+0\t0.000000E+0\t0.000000E+0\t6.194839E-2\t6.194839E-2\t0.000000E+0\t0.000000E+0\t0.000000E+0\t0.000000E+0\t0.000000E+0\t0.000000E+0\t0.000000E+0\t0.000000E+0\t0.000000E+0\t0.000000E+0\t0.000000E+0\t0.000000E+0\t0.000000E+0\t0.000000E+0\t0.000000E+0\t0.000000E+0\t0.000000E+0\t0.000000E+0\t0.000000E+0\t0.000000E+0\t0.000000E+0\t0.000000E+0\t0.000000E+0\t0.000000E+0\t0.000000E+0\t0.000000E+0\t0.000000E+0\t0.000000E+0\t0.000000E+0\t0.000000E+0\t0.000000E+0\t0.000000E+0\t0.000000E+0\t0.000000E+0\t0.000000E+0\t0.000000E+0\t0.000000E+0\t0.000000E+0\t0.000000E+0\t0.000000E+0\t0.000000E+0\t0.000000E+0\t0.000000E+0\t0.000000E+0\t0.000000E+0\t0.000000E+0\t0.000000E+0\t0.000000E+0\t0.000000E+0\r\n1.036583E-1\t0.000000E+0\t0.000000E+0\t0.000000E+0\t0.000000E+0\t0.000000E+0\t0.000000E+0\t0.000000E+0\t0.000000E+0\t0.000000E+0\t0.000000E+0\t0.000000E+0\t0.000000E+0\t0.000000E+0\t0.000000E+0\t0.000000E+0\t0.000000E+0\t0.000000E+0\t0.000000E+0\t0.000000E+0\t0.000000E+0\t0.000000E+0\t0.000000E+0\t0.000000E+0\t0.000000E+0\t0.000000E+0\t0.000000E+0\t0.000000E+0\t0.000000E+0\t0.000000E+0\t0.000000E+0\t0.000000E+0\t0.000000E+0\t0.000000E+0\t0.000000E+0\t0.000000E+0\t0.000000E+0\t0.000000E+0\t0.000000E+0\t0.000000E+0\t0.000000E+0\t0.000000E+0\t0.000000E+0\t0.000000E+0\t0.000000E+0\t0.000000E+0\t0.000000E+0\t0.000000E+0\t0.000000E+0\t7.453582E-4\t1.722307E-1\t1.722307E-1\t7.453582E-4\t0.000000E+0\t0.000000E+0\t0.000000E+0\t0.000000E+0\t0.000000E+0\t0.000000E+0\t0.000000E+0\t0.000000E+0\t0.000000E+0\t0.000000E+0\t0.000000E+0\t0.000000E+0\t0.000000E+0\t0.000000E+0\t0.000000E+0\t0.000000E+0\t0.000000E+0\t0.000000E+0\t0.000000E+0\t0.000000E+0\t0.000000E+0\t0.000000E+0\t0.000000E+0\t0.000000E+0\t0.000000E+0\t0.000000E+0\t0.000000E+0\t0.000000E+0\t0.000000E+0\t0.000000E+0\t0.000000E+0\t0.000000E+0\t0.000000E+0\t0.000000E+0\t0.000000E+0\t0.000000E+0\t0.000000E+0\t0.000000E+0\t0.000000E+0\t0.000000E+0\t0.000000E+0\t0.000000E+0\t0.000000E+0\t0.000000E+0\t0.000000E+0\t0.000000E+0\t0.000000E+0\t0.000000E+0\r\n1.486160E-1\t0.000000E+0\t0.000000E+0\t0.000000E+0\t0.000000E+0\t0.000000E+0\t0.000000E+0\t0.000000E+0\t0.000000E+0\t0.000000E+0\t0.000000E+0\t0.000000E+0\t0.000000E+0\t0.000000E+0\t0.000000E+0\t0.000000E+0\t0.000000E+0\t0.000000E+0\t0.000000E+0\t0.000000E+0\t0.000000E+0\t0.000000E+0\t0.000000E+0\t0.000000E+0\t0.000000E+0\t0.000000E+0\t0.000000E+0\t0.000000E+0\t0.000000E+0\t0.000000E+0\t0.000000E+0\t0.000000E+0\t0.000000E+0\t0.000000E+0\t0.000000E+0\t0.000000E+0\t0.000000E+0\t0.000000E+0\t0.000000E+0\t0.000000E+0\t0.000000E+0\t0.000000E+0\t0.000000E+0\t0.000000E+0\t0.000000E+0\t0.000000E+0\t0.000000E+0\t0.000000E+0\t0.000000E+0\t1.158238E-1\t2.775366E-1\t2.775366E-1\t1.158238E-1\t0.000000E+0\t0.000000E+0\t0.000000E+0\t0.000000E+0\t0.000000E+0\t0.000000E+0\t0.000000E+0\t0.000000E+0\t0.000000E+0\t0.000000E+0\t0.000000E+0\t0.000000E+0\t0.000000E+0\t0.000000E+0\t0.000000E+0\t0.000000E+0\t0.000000E+0\t0.000000E+0\t0.000000E+0\t0.000000E+0\t0.000000E+0\t0.000000E+0\t0.000000E+0\t0.000000E+0\t0.000000E+0\t0.000000E+0\t0.000000E+0\t0.000000E+0\t0.000000E+0\t0.000000E+0\t0.000000E+0\t0.000000E+0\t0.000000E+0\t0.000000E+0\t0.000000E+0\t0.000000E+0\t0.000000E+0\t0.000000E+0\t0.000000E+0\t0.000000E+0\t0.000000E+0\t0.000000E+0\t0.000000E+0\t0.000000E+0\t0.000000E+0\t0.000000E+0\t0.000000E+0\t0.000000E+0\r\n1.935738E-1\t0.000000E+0\t0.000000E+0\t0.000000E+0\t0.000000E+0\t0.000000E+0\t0.000000E+0\t0.000000E+0\t0.000000E+0\t0.000000E+0\t0.000000E+0\t0.000000E+0\t0.000000E+0\t0.000000E+0\t0.000000E+0\t0.000000E+0\t0.000000E+0\t0.000000E+0\t0.000000E+0\t0.000000E+0\t0.000000E+0\t0.000000E+0\t0.000000E+0\t0.000000E+0\t0.000000E+0\t0.000000E+0\t0.000000E+0\t0.000000E+0\t0.000000E+0\t0.000000E+0\t0.000000E+0\t0.000000E+0\t0.000000E+0\t0.000000E+0\t0.000000E+0\t0.000000E+0\t0.000000E+0\t0.000000E+0\t0.000000E+0\t0.000000E+0\t0.000000E+0\t0.000000E+0\t0.000000E+0\t0.000000E+0\t0.000000E+0\t0.000000E+0\t0.000000E+0\t0.000000E+0\t5.448879E-2\t2.281933E-1\t3.789256E-1\t3.789256E-1\t2.281933E-1\t5.448879E-2\t0.000000E+0\t0.000000E+0\t0.000000E+0\t0.000000E+0\t0.000000E+0\t0.000000E+0\t0.000000E+0\t0.000000E+0\t0.000000E+0\t0.000000E+0\t0.000000E+0\t0.000000E+0\t0.000000E+0\t0.000000E+0\t0.000000E+0\t0.000000E+0\t0.000000E+0\t0.000000E+0\t0.000000E+0\t0.000000E+0\t0.000000E+0\t0.000000E+0\t0.000000E+0\t0.000000E+0\t0.000000E+0\t0.000000E+0\t0.000000E+0\t0.000000E+0\t0.000000E+0\t0.000000E+0\t0.000000E+0\t0.000000E+0\t0.000000E+0\t0.000000E+0\t0.000000E+0\t0.000000E+0\t0.000000E+0\t0.000000E+0\t0.000000E+0\t0.000000E+0\t0.000000E+0\t0.000000E+0\t0.000000E+0\t0.000000E+0\t0.000000E+0\t0.000000E+0\t0.000000E+0\r\n2.385316E-1\t0.000000E+0\t0.000000E+0\t0.000000E+0\t0.000000E+0\t0.000000E+0\t0.000000E+0\t0.000000E+0\t0.000000E+0\t0.000000E+0\t0.000000E+0\t0.000000E+0\t0.000000E+0\t0.000000E+0\t0.000000E+0\t0.000000E+0\t0.000000E+0\t0.000000E+0\t0.000000E+0\t0.000000E+0\t0.000000E+0\t0.000000E+0\t0.000000E+0\t0.000000E+0\t0.000000E+0\t0.000000E+0\t0.000000E+0\t0.000000E+0\t0.000000E+0\t0.000000E+0\t0.000000E+0\t0.000000E+0\t0.000000E+0\t0.000000E+0\t0.000000E+0\t0.000000E+0\t0.000000E+0\t0.000000E+0\t0.000000E+0\t0.000000E+0\t0.000000E+0\t0.000000E+0\t0.000000E+0\t0.000000E+0\t0.000000E+0\t0.000000E+0\t0.000000E+0\t0.000000E+0\t1.682108E-1\t3.367912E-1\t4.765848E-1\t4.765848E-1\t3.367912E-1\t1.682108E-1\t0.000000E+0\t0.000000E+0\t0.000000E+0\t0.000000E+0\t0.000000E+0\t0.000000E+0\t0.000000E+0\t0.000000E+0\t0.000000E+0\t0.000000E+0\t0.000000E+0\t0.000000E+0\t0.000000E+0\t0.000000E+0\t0.000000E+0\t0.000000E+0\t0.000000E+0\t0.000000E+0\t0.000000E+0\t0.000000E+0\t0.000000E+0\t0.000000E+0\t0.000000E+0\t0.000000E+0\t0.000000E+0\t0.000000E+0\t0.000000E+0\t0.000000E+0\t0.000000E+0\t0.000000E+0\t0.000000E+0\t0.000000E+0\t0.000000E+0\t0.000000E+0\t0.000000E+0\t0.000000E+0\t0.000000E+0\t0.000000E+0\t0.000000E+0\t0.000000E+0\t0.000000E+0\t0.000000E+0\t0.000000E+0\t0.000000E+0\t0.000000E+0\t0.000000E+0\t0.000000E+0\r\n2.834893E-1\t0.000000E+0\t0.000000E+0\t0.000000E+0\t0.000000E+0\t0.000000E+0\t0.000000E+0\t0.000000E+0\t0.000000E+0\t0.000000E+0\t0.000000E+0\t0.000000E+0\t0.000000E+0\t0.000000E+0\t0.000000E+0\t0.000000E+0\t0.000000E+0\t0.000000E+0\t0.000000E+0\t0.000000E+0\t0.000000E+0\t0.000000E+0\t0.000000E+0\t0.000000E+0\t0.000000E+0\t0.000000E+0\t0.000000E+0\t0.000000E+0\t0.000000E+0\t0.000000E+0\t0.000000E+0\t0.000000E+0\t0.000000E+0\t0.000000E+0\t0.000000E+0\t0.000000E+0\t0.000000E+0\t0.000000E+0\t0.000000E+0\t0.000000E+0\t0.000000E+0\t0.000000E+0\t0.000000E+0\t0.000000E+0\t0.000000E+0\t0.000000E+0\t0.000000E+0\t1.064713E-1\t2.788757E-1\t4.408988E-1\t5.701768E-1\t5.701768E-1\t4.408988E-1\t2.788757E-1\t1.064713E-1\t0.000000E+0\t0.000000E+0\t0.000000E+0\t0.000000E+0\t0.000000E+0\t0.000000E+0\t0.000000E+0\t0.000000E+0\t0.000000E+0\t0.000000E+0\t0.000000E+0\t0.000000E+0\t0.000000E+0\t0.000000E+0\t0.000000E+0\t0.000000E+0\t0.000000E+0\t0.000000E+0\t0.000000E+0\t0.000000E+0\t0.000000E+0\t0.000000E+0\t0.000000E+0\t0.000000E+0\t0.000000E+0\t0.000000E+0\t0.000000E+0\t0.000000E+0\t0.000000E+0\t0.000000E+0\t0.000000E+0\t0.000000E+0\t0.000000E+0\t0.000000E+0\t0.000000E+0\t0.000000E+0\t0.000000E+0\t0.000000E+0\t0.000000E+0\t0.000000E+0\t0.000000E+0\t0.000000E+0\t0.000000E+0\t0.000000E+0\t0.000000E+0\t0.000000E+0\r\n3.284471E-1\t0.000000E+0\t0.000000E+0\t0.000000E+0\t0.000000E+0\t0.000000E+0\t0.000000E+0\t0.000000E+0\t0.000000E+0\t0.000000E+0\t0.000000E+0\t0.000000E+0\t0.000000E+0\t0.000000E+0\t0.000000E+0\t0.000000E+0\t0.000000E+0\t0.000000E+0\t0.000000E+0\t0.000000E+0\t0.000000E+0\t0.000000E+0\t0.000000E+0\t0.000000E+0\t0.000000E+0\t0.000000E+0\t0.000000E+0\t0.000000E+0\t0.000000E+0\t0.000000E+0\t0.000000E+0\t0.000000E+0\t0.000000E+0\t0.000000E+0\t0.000000E+0\t0.000000E+0\t0.000000E+0\t0.000000E+0\t0.000000E+0\t0.000000E+0\t0.000000E+0\t0.000000E+0\t0.000000E+0\t0.000000E+0\t0.000000E+0\t0.000000E+0\t4.528990E-2\t2.169191E-1\t3.851983E-1\t5.397582E-1\t6.590436E-1\t6.590436E-1\t5.397582E-1\t3.851983E-1\t2.169191E-1\t4.528990E-2\t0.000000E+0\t0.000000E+0\t0.000000E+0\t0.000000E+0\t0.000000E+0\t0.000000E+0\t0.000000E+0\t0.000000E+0\t0.000000E+0\t0.000000E+0\t0.000000E+0\t0.000000E+0\t0.000000E+0\t0.000000E+0\t0.000000E+0\t0.000000E+0\t0.000000E+0\t0.000000E+0\t0.000000E+0\t0.000000E+0\t0.000000E+0\t0.000000E+0\t0.000000E+0\t0.000000E+0\t0.000000E+0\t0.000000E+0\t0.000000E+0\t0.000000E+0\t0.000000E+0\t0.000000E+0\t0.000000E+0\t0.000000E+0\t0.000000E+0\t0.000000E+0\t0.000000E+0\t0.000000E+0\t0.000000E+0\t0.000000E+0\t0.000000E+0\t0.000000E+0\t0.000000E+0\t0.000000E+0\t0.000000E+0\t0.000000E+0\t0.000000E+0\r\n3.734049E-1\t0.000000E+0\t0.000000E+0\t0.000000E+0\t0.000000E+0\t0.000000E+0\t0.000000E+0\t0.000000E+0\t0.000000E+0\t0.000000E+0\t0.000000E+0\t0.000000E+0\t0.000000E+0\t0.000000E+0\t0.000000E+0\t0.000000E+0\t0.000000E+0\t0.000000E+0\t0.000000E+0\t0.000000E+0\t0.000000E+0\t0.000000E+0\t0.000000E+0\t0.000000E+0\t0.000000E+0\t0.000000E+0\t0.000000E+0\t0.000000E+0\t0.000000E+0\t0.000000E+0\t0.000000E+0\t0.000000E+0\t0.000000E+0\t0.000000E+0\t0.000000E+0\t0.000000E+0\t0.000000E+0\t0.000000E+0\t0.000000E+0\t0.000000E+0\t0.000000E+0\t0.000000E+0\t0.000000E+0\t0.000000E+0\t0.000000E+0\t0.000000E+0\t1.540852E-1\t3.230475E-1\t4.859765E-1\t6.324970E-1\t7.423191E-1\t7.423191E-1\t6.324970E-1\t4.859765E-1\t3.230475E-1\t1.540852E-1\t0.000000E+0\t0.000000E+0\t0.000000E+0\t0.000000E+0\t0.000000E+0\t0.000000E+0\t0.000000E+0\t0.000000E+0\t0.000000E+0\t0.000000E+0\t0.000000E+0\t0.000000E+0\t0.000000E+0\t0.000000E+0\t0.000000E+0\t0.000000E+0\t0.000000E+0\t0.000000E+0\t0.000000E+0\t0.000000E+0\t0.000000E+0\t0.000000E+0\t0.000000E+0\t0.000000E+0\t0.000000E+0\t0.000000E+0\t0.000000E+0\t0.000000E+0\t0.000000E+0\t0.000000E+0\t0.000000E+0\t0.000000E+0\t0.000000E+0\t0.000000E+0\t0.000000E+0\t0.000000E+0\t0.000000E+0\t0.000000E+0\t0.000000E+0\t0.000000E+0\t0.000000E+0\t0.000000E+0\t0.000000E+0\t0.000000E+0\t0.000000E+0\r\n4.183626E-1\t0.000000E+0\t0.000000E+0\t0.000000E+0\t0.000000E+0\t0.000000E+0\t0.000000E+0\t0.000000E+0\t0.000000E+0\t0.000000E+0\t0.000000E+0\t0.000000E+0\t0.000000E+0\t0.000000E+0\t0.000000E+0\t0.000000E+0\t0.000000E+0\t0.000000E+0\t0.000000E+0\t0.000000E+0\t0.000000E+0\t0.000000E+0\t0.000000E+0\t0.000000E+0\t0.000000E+0\t0.000000E+0\t0.000000E+0\t0.000000E+0\t0.000000E+0\t0.000000E+0\t0.000000E+0\t0.000000E+0\t0.000000E+0\t0.000000E+0\t0.000000E+0\t0.000000E+0\t0.000000E+0\t0.000000E+0\t0.000000E+0\t0.000000E+0\t0.000000E+0\t0.000000E+0\t0.000000E+0\t0.000000E+0\t0.000000E+0\t9.252746E-2\t2.584029E-1\t4.234039E-1\t5.800182E-1\t7.181422E-1\t8.190088E-1\t8.190088E-1\t7.181422E-1\t5.800182E-1\t4.234039E-1\t2.584029E-1\t9.252746E-2\t0.000000E+0\t0.000000E+0\t0.000000E+0\t0.000000E+0\t0.000000E+0\t0.000000E+0\t0.000000E+0\t0.000000E+0\t0.000000E+0\t0.000000E+0\t0.000000E+0\t0.000000E+0\t0.000000E+0\t0.000000E+0\t0.000000E+0\t0.000000E+0\t0.000000E+0\t0.000000E+0\t0.000000E+0\t0.000000E+0\t0.000000E+0\t0.000000E+0\t0.000000E+0\t0.000000E+0\t0.000000E+0\t0.000000E+0\t0.000000E+0\t0.000000E+0\t0.000000E+0\t0.000000E+0\t0.000000E+0\t0.000000E+0\t0.000000E+0\t0.000000E+0\t0.000000E+0\t0.000000E+0\t0.000000E+0\t0.000000E+0\t0.000000E+0\t0.000000E+0\t0.000000E+0\t0.000000E+0\t0.000000E+0\t0.000000E+0\r\n4.633204E-1\t0.000000E+0\t0.000000E+0\t0.000000E+0\t0.000000E+0\t0.000000E+0\t0.000000E+0\t0.000000E+0\t0.000000E+0\t0.000000E+0\t0.000000E+0\t0.000000E+0\t0.000000E+0\t0.000000E+0\t0.000000E+0\t0.000000E+0\t0.000000E+0\t0.000000E+0\t0.000000E+0\t0.000000E+0\t0.000000E+0\t0.000000E+0\t0.000000E+0\t0.000000E+0\t0.000000E+0\t0.000000E+0\t0.000000E+0\t0.000000E+0\t0.000000E+0\t0.000000E+0\t0.000000E+0\t0.000000E+0\t0.000000E+0\t0.000000E+0\t0.000000E+0\t0.000000E+0\t0.000000E+0\t0.000000E+0\t0.000000E+0\t0.000000E+0\t0.000000E+0\t0.000000E+0\t0.000000E+0\t0.000000E+0\t3.443811E-2\t1.937383E-1\t3.566702E-1\t5.165983E-1\t6.661405E-1\t7.956667E-1\t8.880586E-1\t8.880586E-1\t7.956667E-1\t6.661405E-1\t5.165983E-1\t3.566702E-1\t1.937383E-1\t3.443811E-2\t0.000000E+0\t0.000000E+0\t0.000000E+0\t0.000000E+0\t0.000000E+0\t0.000000E+0\t0.000000E+0\t0.000000E+0\t0.000000E+0\t0.000000E+0\t0.000000E+0\t0.000000E+0\t0.000000E+0\t0.000000E+0\t0.000000E+0\t0.000000E+0\t0.000000E+0\t0.000000E+0\t0.000000E+0\t0.000000E+0\t0.000000E+0\t0.000000E+0\t0.000000E+0\t0.000000E+0\t0.000000E+0\t0.000000E+0\t0.000000E+0\t0.000000E+0\t0.000000E+0\t0.000000E+0\t0.000000E+0\t0.000000E+0\t0.000000E+0\t0.000000E+0\t0.000000E+0\t0.000000E+0\t0.000000E+0\t0.000000E+0\t0.000000E+0\t0.000000E+0\t0.000000E+0\t0.000000E+0\t0.000000E+0\r\n5.082782E-1\t0.000000E+0\t0.000000E+0\t0.000000E+0\t0.000000E+0\t0.000000E+0\t0.000000E+0\t0.000000E+0\t0.000000E+0\t0.000000E+0\t0.000000E+0\t0.000000E+0\t0.000000E+0\t0.000000E+0\t0.000000E+0\t0.000000E+0\t0.000000E+0\t0.000000E+0\t0.000000E+0\t0.000000E+0\t0.000000E+0\t0.000000E+0\t0.000000E+0\t0.000000E+0\t0.000000E+0\t0.000000E+0\t0.000000E+0\t0.000000E+0\t0.000000E+0\t0.000000E+0\t0.000000E+0\t0.000000E+0\t0.000000E+0\t0.000000E+0\t0.000000E+0\t0.000000E+0\t0.000000E+0\t0.000000E+0\t0.000000E+0\t0.000000E+0\t0.000000E+0\t0.000000E+0\t0.000000E+0\t0.000000E+0\t1.314062E-1\t2.885968E-1\t4.474119E-1\t6.013203E-1\t7.432045E-1\t8.640485E-1\t9.484234E-1\t9.484234E-1\t8.640485E-1\t7.432045E-1\t6.013203E-1\t4.474119E-1\t2.885968E-1\t1.314062E-1\t0.000000E+0\t0.000000E+0\t0.000000E+0\t0.000000E+0\t0.000000E+0\t0.000000E+0\t0.000000E+0\t0.000000E+0\t0.000000E+0\t0.000000E+0\t0.000000E+0\t0.000000E+0\t0.000000E+0\t0.000000E+0\t0.000000E+0\t0.000000E+0\t0.000000E+0\t0.000000E+0\t0.000000E+0\t0.000000E+0\t0.000000E+0\t0.000000E+0\t0.000000E+0\t0.000000E+0\t0.000000E+0\t0.000000E+0\t0.000000E+0\t0.000000E+0\t0.000000E+0\t0.000000E+0\t0.000000E+0\t0.000000E+0\t0.000000E+0\t0.000000E+0\t0.000000E+0\t0.000000E+0\t0.000000E+0\t0.000000E+0\t0.000000E+0\t0.000000E+0\t0.000000E+0\t0.000000E+0\t0.000000E+0\r\n5.532359E-1\t0.000000E+0\t0.000000E+0\t0.000000E+0\t0.000000E+0\t0.000000E+0\t0.000000E+0\t0.000000E+0\t0.000000E+0\t0.000000E+0\t0.000000E+0\t0.000000E+0\t0.000000E+0\t0.000000E+0\t0.000000E+0\t0.000000E+0\t0.000000E+0\t0.000000E+0\t0.000000E+0\t0.000000E+0\t0.000000E+0\t0.000000E+0\t0.000000E+0\t0.000000E+0\t0.000000E+0\t0.000000E+0\t0.000000E+0\t0.000000E+0\t0.000000E+0\t0.000000E+0\t0.000000E+0\t0.000000E+0\t0.000000E+0\t0.000000E+0\t0.000000E+0\t0.000000E+0\t0.000000E+0\t0.000000E+0\t0.000000E+0\t0.000000E+0\t0.000000E+0\t0.000000E+0\t0.000000E+0\t7.377468E-2\t2.217484E-1\t3.756303E-1\t5.292827E-1\t6.763769E-1\t8.101642E-1\t9.223353E-1\t9.991323E-1\t9.991323E-1\t9.223353E-1\t8.101642E-1\t6.763769E-1\t5.292827E-1\t3.756303E-1\t2.217484E-1\t7.377468E-2\t0.000000E+0\t0.000000E+0\t0.000000E+0\t0.000000E+0\t0.000000E+0\t0.000000E+0\t0.000000E+0\t0.000000E+0\t0.000000E+0\t0.000000E+0\t0.000000E+0\t0.000000E+0\t0.000000E+0\t0.000000E+0\t0.000000E+0\t0.000000E+0\t0.000000E+0\t0.000000E+0\t0.000000E+0\t0.000000E+0\t0.000000E+0\t0.000000E+0\t0.000000E+0\t0.000000E+0\t0.000000E+0\t0.000000E+0\t0.000000E+0\t0.000000E+0\t0.000000E+0\t0.000000E+0\t0.000000E+0\t0.000000E+0\t0.000000E+0\t0.000000E+0\t0.000000E+0\t0.000000E+0\t0.000000E+0\t0.000000E+0\t0.000000E+0\t0.000000E+0\t0.000000E+0\t0.000000E+0\r\n5.981937E-1\t0.000000E+0\t0.000000E+0\t0.000000E+0\t0.000000E+0\t0.000000E+0\t0.000000E+0\t0.000000E+0\t0.000000E+0\t0.000000E+0\t0.000000E+0\t0.000000E+0\t0.000000E+0\t0.000000E+0\t0.000000E+0\t0.000000E+0\t0.000000E+0\t0.000000E+0\t0.000000E+0\t0.000000E+0\t0.000000E+0\t0.000000E+0\t0.000000E+0\t0.000000E+0\t0.000000E+0\t0.000000E+0\t0.000000E+0\t0.000000E+0\t0.000000E+0\t0.000000E+0\t0.000000E+0\t0.000000E+0\t0.000000E+0\t0.000000E+0\t0.000000E+0\t0.000000E+0\t0.000000E+0\t0.000000E+0\t0.000000E+0\t0.000000E+0\t0.000000E+0\t0.000000E+0\t2.303055E-2\t1.586605E-1\t3.040634E-1\t4.535374E-1\t6.011115E-1\t7.407405E-1\t8.661223E-1\t9.697078E-1\t1.039352E+0\t1.039352E+0\t9.697078E-1\t8.661223E-1\t7.407405E-1\t6.011115E-1\t4.535374E-1\t3.040634E-1\t1.586605E-1\t2.303055E-2\t0.000000E+0\t0.000000E+0\t0.000000E+0\t0.000000E+0\t0.000000E+0\t0.000000E+0\t0.000000E+0\t0.000000E+0\t0.000000E+0\t0.000000E+0\t0.000000E+0\t0.000000E+0\t0.000000E+0\t0.000000E+0\t0.000000E+0\t0.000000E+0\t0.000000E+0\t0.000000E+0\t0.000000E+0\t0.000000E+0\t0.000000E+0\t0.000000E+0\t0.000000E+0\t0.000000E+0\t0.000000E+0\t0.000000E+0\t0.000000E+0\t0.000000E+0\t0.000000E+0\t0.000000E+0\t0.000000E+0\t0.000000E+0\t0.000000E+0\t0.000000E+0\t0.000000E+0\t0.000000E+0\t0.000000E+0\t0.000000E+0\t0.000000E+0\t0.000000E+0\t0.000000E+0\r\n6.431515E-1\t0.000000E+0\t0.000000E+0\t0.000000E+0\t0.000000E+0\t0.000000E+0\t0.000000E+0\t0.000000E+0\t0.000000E+0\t0.000000E+0\t0.000000E+0\t0.000000E+0\t0.000000E+0\t0.000000E+0\t0.000000E+0\t0.000000E+0\t0.000000E+0\t0.000000E+0\t0.000000E+0\t0.000000E+0\t0.000000E+0\t0.000000E+0\t0.000000E+0\t0.000000E+0\t0.000000E+0\t0.000000E+0\t0.000000E+0\t0.000000E+0\t0.000000E+0\t0.000000E+0\t0.000000E+0\t0.000000E+0\t0.000000E+0\t0.000000E+0\t0.000000E+0\t0.000000E+0\t0.000000E+0\t0.000000E+0\t0.000000E+0\t0.000000E+0\t0.000000E+0\t0.000000E+0\t1.016823E-1\t2.354463E-1\t3.771547E-1\t5.212339E-1\t6.619471E-1\t7.935971E-1\t9.103823E-1\t1.005537E+0\t1.068445E+0\t1.068445E+0\t1.005537E+0\t9.103823E-1\t7.935971E-1\t6.619471E-1\t5.212339E-1\t3.771547E-1\t2.354463E-1\t1.016823E-1\t0.000000E+0\t0.000000E+0\t0.000000E+0\t0.000000E+0\t0.000000E+0\t0.000000E+0\t0.000000E+0\t0.000000E+0\t0.000000E+0\t0.000000E+0\t0.000000E+0\t0.000000E+0\t0.000000E+0\t0.000000E+0\t0.000000E+0\t0.000000E+0\t0.000000E+0\t0.000000E+0\t0.000000E+0\t0.000000E+0\t0.000000E+0\t0.000000E+0\t0.000000E+0\t0.000000E+0\t0.000000E+0\t0.000000E+0\t0.000000E+0\t0.000000E+0\t0.000000E+0\t0.000000E+0\t0.000000E+0\t0.000000E+0\t0.000000E+0\t0.000000E+0\t0.000000E+0\t0.000000E+0\t0.000000E+0\t0.000000E+0\t0.000000E+0\t0.000000E+0\t0.000000E+0\r\n6.881092E-1\t0.000000E+0\t0.000000E+0\t0.000000E+0\t0.000000E+0\t0.000000E+0\t0.000000E+0\t0.000000E+0\t0.000000E+0\t0.000000E+0\t0.000000E+0\t0.000000E+0\t0.000000E+0\t0.000000E+0\t0.000000E+0\t0.000000E+0\t0.000000E+0\t0.000000E+0\t0.000000E+0\t0.000000E+0\t0.000000E+0\t0.000000E+0\t0.000000E+0\t0.000000E+0\t0.000000E+0\t0.000000E+0\t0.000000E+0\t0.000000E+0\t0.000000E+0\t0.000000E+0\t0.000000E+0\t0.000000E+0\t0.000000E+0\t0.000000E+0\t0.000000E+0\t0.000000E+0\t0.000000E+0\t0.000000E+0\t0.000000E+0\t0.000000E+0\t0.000000E+0\t5.272174E-2\t1.723111E-1\t3.030832E-1\t4.400728E-1\t5.778936E-1\t7.110991E-1\t8.343883E-1\t9.424934E-1\t1.029430E+0\t1.086010E+0\t1.086010E+0\t1.029430E+0\t9.424934E-1\t8.343883E-1\t7.110991E-1\t5.778936E-1\t4.400728E-1\t3.030832E-1\t1.723111E-1\t5.272174E-2\t0.000000E+0\t0.000000E+0\t0.000000E+0\t0.000000E+0\t0.000000E+0\t0.000000E+0\t0.000000E+0\t0.000000E+0\t0.000000E+0\t0.000000E+0\t0.000000E+0\t0.000000E+0\t0.000000E+0\t0.000000E+0\t0.000000E+0\t0.000000E+0\t0.000000E+0\t0.000000E+0\t0.000000E+0\t0.000000E+0\t0.000000E+0\t0.000000E+0\t0.000000E+0\t0.000000E+0\t0.000000E+0\t0.000000E+0\t0.000000E+0\t0.000000E+0\t0.000000E+0\t0.000000E+0\t0.000000E+0\t0.000000E+0\t0.000000E+0\t0.000000E+0\t0.000000E+0\t0.000000E+0\t0.000000E+0\t0.000000E+0\t0.000000E+0\t0.000000E+0\r\n7.330670E-1\t0.000000E+0\t0.000000E+0\t0.000000E+0\t0.000000E+0\t0.000000E+0\t0.000000E+0\t0.000000E+0\t0.000000E+0\t0.000000E+0\t0.000000E+0\t0.000000E+0\t0.000000E+0\t0.000000E+0\t0.000000E+0\t0.000000E+0\t0.000000E+0\t0.000000E+0\t0.000000E+0\t0.000000E+0\t0.000000E+0\t0.000000E+0\t0.000000E+0\t0.000000E+0\t0.000000E+0\t0.000000E+0\t0.000000E+0\t0.000000E+0\t0.000000E+0\t0.000000E+0\t0.000000E+0\t0.000000E+0\t0.000000E+0\t0.000000E+0\t0.000000E+0\t0.000000E+0\t0.000000E+0\t0.000000E+0\t0.000000E+0\t0.000000E+0\t1.302694E-2\t1.167465E-1\t2.340419E-1\t3.607871E-1\t4.921498E-1\t6.229812E-1\t7.481692E-1\t8.628429E-1\t9.622834E-1\t1.041268E+0\t1.091924E+0\t1.091924E+0\t1.041268E+0\t9.622834E-1\t8.628429E-1\t7.481692E-1\t6.229812E-1\t4.921498E-1\t3.607871E-1\t2.340419E-1\t1.167465E-1\t1.302694E-2\t0.000000E+0\t0.000000E+0\t0.000000E+0\t0.000000E+0\t0.000000E+0\t0.000000E+0\t0.000000E+0\t0.000000E+0\t0.000000E+0\t0.000000E+0\t0.000000E+0\t0.000000E+0\t0.000000E+0\t0.000000E+0\t0.000000E+0\t0.000000E+0\t0.000000E+0\t0.000000E+0\t0.000000E+0\t0.000000E+0\t0.000000E+0\t0.000000E+0\t0.000000E+0\t0.000000E+0\t0.000000E+0\t0.000000E+0\t0.000000E+0\t0.000000E+0\t0.000000E+0\t0.000000E+0\t0.000000E+0\t0.000000E+0\t0.000000E+0\t0.000000E+0\t0.000000E+0\t0.000000E+0\t0.000000E+0\t0.000000E+0\t0.000000E+0\r\n7.780248E-1\t0.000000E+0\t0.000000E+0\t0.000000E+0\t0.000000E+0\t0.000000E+0\t0.000000E+0\t0.000000E+0\t0.000000E+0\t0.000000E+0\t0.000000E+0\t0.000000E+0\t0.000000E+0\t0.000000E+0\t0.000000E+0\t0.000000E+0\t0.000000E+0\t0.000000E+0\t0.000000E+0\t0.000000E+0\t0.000000E+0\t0.000000E+0\t0.000000E+0\t0.000000E+0\t0.000000E+0\t0.000000E+0\t0.000000E+0\t0.000000E+0\t0.000000E+0\t0.000000E+0\t0.000000E+0\t0.000000E+0\t0.000000E+0\t0.000000E+0\t0.000000E+0\t0.000000E+0\t0.000000E+0\t0.000000E+0\t0.000000E+0\t0.000000E+0\t7.018356E-2\t1.722913E-1\t2.862699E-1\t4.080642E-1\t5.330211E-1\t6.562709E-1\t7.730688E-1\t8.789939E-1\t9.698760E-1\t1.041220E+0\t1.086350E+0\t1.086350E+0\t1.041220E+0\t9.698760E-1\t8.789939E-1\t7.730688E-1\t6.562709E-1\t5.330211E-1\t4.080642E-1\t2.862699E-1\t1.722913E-1\t7.018356E-2\t0.000000E+0\t0.000000E+0\t0.000000E+0\t0.000000E+0\t0.000000E+0\t0.000000E+0\t0.000000E+0\t0.000000E+0\t0.000000E+0\t0.000000E+0\t0.000000E+0\t0.000000E+0\t0.000000E+0\t0.000000E+0\t0.000000E+0\t0.000000E+0\t0.000000E+0\t0.000000E+0\t0.000000E+0\t0.000000E+0\t0.000000E+0\t0.000000E+0\t0.000000E+0\t0.000000E+0\t0.000000E+0\t0.000000E+0\t0.000000E+0\t0.000000E+0\t0.000000E+0\t0.000000E+0\t0.000000E+0\t0.000000E+0\t0.000000E+0\t0.000000E+0\t0.000000E+0\t0.000000E+0\t0.000000E+0\t0.000000E+0\t0.000000E+0\r\n8.229825E-1\t0.000000E+0\t0.000000E+0\t0.000000E+0\t0.000000E+0\t0.000000E+0\t0.000000E+0\t0.000000E+0\t0.000000E+0\t0.000000E+0\t0.000000E+0\t0.000000E+0\t0.000000E+0\t0.000000E+0\t0.000000E+0\t0.000000E+0\t0.000000E+0\t0.000000E+0\t0.000000E+0\t0.000000E+0\t0.000000E+0\t0.000000E+0\t0.000000E+0\t0.000000E+0\t0.000000E+0\t0.000000E+0\t0.000000E+0\t0.000000E+0\t0.000000E+0\t0.000000E+0\t0.000000E+0\t0.000000E+0\t0.000000E+0\t0.000000E+0\t0.000000E+0\t0.000000E+0\t0.000000E+0\t0.000000E+0\t0.000000E+0\t3.327642E-2\t1.194243E-1\t2.189291E-1\t3.286752E-1\t4.447213E-1\t5.626329E-1\t6.778516E-1\t7.860220E-1\t8.831805E-1\t9.656933E-1\t1.029748E+0\t1.069746E+0\t1.069746E+0\t1.029748E+0\t9.656933E-1\t8.831805E-1\t7.860220E-1\t6.778516E-1\t5.626329E-1\t4.447213E-1\t3.286752E-1\t2.189291E-1\t1.194243E-1\t3.327642E-2\t0.000000E+0\t0.000000E+0\t0.000000E+0\t0.000000E+0\t0.000000E+0\t0.000000E+0\t0.000000E+0\t0.000000E+0\t0.000000E+0\t0.000000E+0\t0.000000E+0\t0.000000E+0\t0.000000E+0\t0.000000E+0\t0.000000E+0\t0.000000E+0\t0.000000E+0\t0.000000E+0\t0.000000E+0\t0.000000E+0\t0.000000E+0\t0.000000E+0\t0.000000E+0\t0.000000E+0\t0.000000E+0\t0.000000E+0\t0.000000E+0\t0.000000E+0\t0.000000E+0\t0.000000E+0\t0.000000E+0\t0.000000E+0\t0.000000E+0\t0.000000E+0\t0.000000E+0\t0.000000E+0\t0.000000E+0\t0.000000E+0\r\n8.679403E-1\t0.000000E+0\t0.000000E+0\t0.000000E+0\t0.000000E+0\t0.000000E+0\t0.000000E+0\t0.000000E+0\t0.000000E+0\t0.000000E+0\t0.000000E+0\t0.000000E+0\t0.000000E+0\t0.000000E+0\t0.000000E+0\t0.000000E+0\t0.000000E+0\t0.000000E+0\t0.000000E+0\t0.000000E+0\t0.000000E+0\t0.000000E+0\t0.000000E+0\t0.000000E+0\t0.000000E+0\t0.000000E+0\t0.000000E+0\t0.000000E+0\t0.000000E+0\t0.000000E+0\t0.000000E+0\t0.000000E+0\t0.000000E+0\t0.000000E+0\t0.000000E+0\t0.000000E+0\t0.000000E+0\t0.000000E+0\t5.902293E-3\t7.624960E-2\t1.604867E-1\t2.565016E-1\t3.612237E-1\t4.708628E-1\t5.812349E-1\t6.881165E-1\t7.875526E-1\t8.760341E-1\t9.504411E-1\t1.007591E+0\t1.042846E+0\t1.042846E+0\t1.007591E+0\t9.504411E-1\t8.760341E-1\t7.875526E-1\t6.881165E-1\t5.812349E-1\t4.708628E-1\t3.612237E-1\t2.565016E-1\t1.604867E-1\t7.624960E-2\t5.902293E-3\t0.000000E+0\t0.000000E+0\t0.000000E+0\t0.000000E+0\t0.000000E+0\t0.000000E+0\t0.000000E+0\t0.000000E+0\t0.000000E+0\t0.000000E+0\t0.000000E+0\t0.000000E+0\t0.000000E+0\t0.000000E+0\t0.000000E+0\t0.000000E+0\t0.000000E+0\t0.000000E+0\t0.000000E+0\t0.000000E+0\t0.000000E+0\t0.000000E+0\t0.000000E+0\t0.000000E+0\t0.000000E+0\t0.000000E+0\t0.000000E+0\t0.000000E+0\t0.000000E+0\t0.000000E+0\t0.000000E+0\t0.000000E+0\t0.000000E+0\t0.000000E+0\t0.000000E+0\t0.000000E+0\t0.000000E+0\r\n9.128981E-1\t0.000000E+0\t0.000000E+0\t0.000000E+0\t0.000000E+0\t0.000000E+0\t0.000000E+0\t0.000000E+0\t0.000000E+0\t0.000000E+0\t0.000000E+0\t0.000000E+0\t0.000000E+0\t0.000000E+0\t0.000000E+0\t0.000000E+0\t0.000000E+0\t0.000000E+0\t0.000000E+0\t0.000000E+0\t0.000000E+0\t0.000000E+0\t0.000000E+0\t0.000000E+0\t0.000000E+0\t0.000000E+0\t0.000000E+0\t0.000000E+0\t0.000000E+0\t0.000000E+0\t0.000000E+0\t0.000000E+0\t0.000000E+0\t0.000000E+0\t0.000000E+0\t0.000000E+0\t0.000000E+0\t0.000000E+0\t4.278971E-2\t1.118670E-1\t1.933521E-1\t2.851112E-1\t3.841539E-1\t4.868731E-1\t5.893592E-1\t6.877378E-1\t7.784570E-1\t8.584497E-1\t9.250796E-1\t9.757366E-1\t1.006630E+0\t1.006630E+0\t9.757366E-1\t9.250796E-1\t8.584497E-1\t7.784570E-1\t6.877378E-1\t5.893592E-1\t4.868731E-1\t3.841539E-1\t2.851112E-1\t1.933521E-1\t1.118670E-1\t4.278971E-2\t0.000000E+0\t0.000000E+0\t0.000000E+0\t0.000000E+0\t0.000000E+0\t0.000000E+0\t0.000000E+0\t0.000000E+0\t0.000000E+0\t0.000000E+0\t0.000000E+0\t0.000000E+0\t0.000000E+0\t0.000000E+0\t0.000000E+0\t0.000000E+0\t0.000000E+0\t0.000000E+0\t0.000000E+0\t0.000000E+0\t0.000000E+0\t0.000000E+0\t0.000000E+0\t0.000000E+0\t0.000000E+0\t0.000000E+0\t0.000000E+0\t0.000000E+0\t0.000000E+0\t0.000000E+0\t0.000000E+0\t0.000000E+0\t0.000000E+0\t0.000000E+0\t0.000000E+0\t0.000000E+0\t0.000000E+0\r\n9.578558E-1\t0.000000E+0\t0.000000E+0\t0.000000E+0\t0.000000E+0\t0.000000E+0\t0.000000E+0\t0.000000E+0\t0.000000E+0\t0.000000E+0\t0.000000E+0\t0.000000E+0\t0.000000E+0\t0.000000E+0\t0.000000E+0\t0.000000E+0\t0.000000E+0\t0.000000E+0\t0.000000E+0\t0.000000E+0\t0.000000E+0\t0.000000E+0\t0.000000E+0\t0.000000E+0\t0.000000E+0\t0.000000E+0\t0.000000E+0\t0.000000E+0\t0.000000E+0\t0.000000E+0\t0.000000E+0\t0.000000E+0\t0.000000E+0\t0.000000E+0\t0.000000E+0\t0.000000E+0\t0.000000E+0\t1.838587E-2\t7.319684E-2\t1.402221E-1\t2.182308E-1\t3.051004E-1\t3.979523E-1\t4.933866E-1\t5.877856E-1\t6.776298E-1\t7.597646E-1\t8.315449E-1\t8.907822E-1\t9.353798E-1\t9.622851E-1\t9.622851E-1\t9.353798E-1\t8.907822E-1\t8.315449E-1\t7.597646E-1\t6.776298E-1\t5.877856E-1\t4.933866E-1\t3.979523E-1\t3.051004E-1\t2.182308E-1\t1.402221E-1\t7.319684E-2\t1.838587E-2\t0.000000E+0\t0.000000E+0\t0.000000E+0\t0.000000E+0\t0.000000E+0\t0.000000E+0\t0.000000E+0\t0.000000E+0\t0.000000E+0\t0.000000E+0\t0.000000E+0\t0.000000E+0\t0.000000E+0\t0.000000E+0\t0.000000E+0\t0.000000E+0\t0.000000E+0\t0.000000E+0\t0.000000E+0\t0.000000E+0\t0.000000E+0\t0.000000E+0\t0.000000E+0\t0.000000E+0\t0.000000E+0\t0.000000E+0\t0.000000E+0\t0.000000E+0\t0.000000E+0\t0.000000E+0\t0.000000E+0\t0.000000E+0\t0.000000E+0\t0.000000E+0\t0.000000E+0\t0.000000E+0\r\n1.002814E+0\t0.000000E+0\t0.000000E+0\t0.000000E+0\t0.000000E+0\t0.000000E+0\t0.000000E+0\t0.000000E+0\t0.000000E+0\t0.000000E+0\t0.000000E+0\t0.000000E+0\t0.000000E+0\t0.000000E+0\t0.000000E+0\t0.000000E+0\t0.000000E+0\t0.000000E+0\t0.000000E+0\t0.000000E+0\t0.000000E+0\t0.000000E+0\t0.000000E+0\t0.000000E+0\t0.000000E+0\t0.000000E+0\t0.000000E+0\t0.000000E+0\t0.000000E+0\t0.000000E+0\t0.000000E+0\t0.000000E+0\t0.000000E+0\t0.000000E+0\t0.000000E+0\t0.000000E+0\t1.877236E-3\t4.390956E-2\t9.729937E-2\t1.616017E-1\t2.355362E-1\t3.170220E-1\t4.033171E-1\t4.912481E-1\t5.774980E-1\t6.589017E-1\t7.326884E-1\t7.966096E-1\t8.488847E-1\t8.878702E-1\t9.111505E-1\t9.111505E-1\t8.878702E-1\t8.488847E-1\t7.966096E-1\t7.326884E-1\t6.589017E-1\t5.774980E-1\t4.912481E-1\t4.033171E-1\t3.170220E-1\t2.355362E-1\t1.616017E-1\t9.729937E-2\t4.390956E-2\t1.877236E-3\t0.000000E+0\t0.000000E+0\t0.000000E+0\t0.000000E+0\t0.000000E+0\t0.000000E+0\t0.000000E+0\t0.000000E+0\t0.000000E+0\t0.000000E+0\t0.000000E+0\t0.000000E+0\t0.000000E+0\t0.000000E+0\t0.000000E+0\t0.000000E+0\t0.000000E+0\t0.000000E+0\t0.000000E+0\t0.000000E+0\t0.000000E+0\t0.000000E+0\t0.000000E+0\t0.000000E+0\t0.000000E+0\t0.000000E+0\t0.000000E+0\t0.000000E+0\t0.000000E+0\t0.000000E+0\t0.000000E+0\t0.000000E+0\t0.000000E+0\t0.000000E+0\t0.000000E+0\r\n1.047771E+0\t0.000000E+0\t0.000000E+0\t0.000000E+0\t0.000000E+0\t0.000000E+0\t0.000000E+0\t0.000000E+0\t0.000000E+0\t0.000000E+0\t0.000000E+0\t0.000000E+0\t0.000000E+0\t0.000000E+0\t0.000000E+0\t0.000000E+0\t0.000000E+0\t0.000000E+0\t0.000000E+0\t0.000000E+0\t0.000000E+0\t0.000000E+0\t0.000000E+0\t0.000000E+0\t0.000000E+0\t0.000000E+0\t0.000000E+0\t0.000000E+0\t0.000000E+0\t0.000000E+0\t0.000000E+0\t0.000000E+0\t0.000000E+0\t0.000000E+0\t0.000000E+0\t0.000000E+0\t2.292145E-2\t6.407032E-2\t1.154301E-1\t1.764579E-1\t2.458526E-1\t3.216003E-1\t4.011158E-1\t4.814646E-1\t5.596335E-1\t6.328036E-1\t6.985695E-1\t7.550493E-1\t8.008280E-1\t8.346569E-1\t8.546633E-1\t8.546633E-1\t8.346569E-1\t8.008280E-1\t7.550493E-1\t6.985695E-1\t6.328036E-1\t5.596335E-1\t4.814646E-1\t4.011158E-1\t3.216003E-1\t2.458526E-1\t1.764579E-1\t1.154301E-1\t6.407032E-2\t2.292145E-2\t0.000000E+0\t0.000000E+0\t0.000000E+0\t0.000000E+0\t0.000000E+0\t0.000000E+0\t0.000000E+0\t0.000000E+0\t0.000000E+0\t0.000000E+0\t0.000000E+0\t0.000000E+0\t0.000000E+0\t0.000000E+0\t0.000000E+0\t0.000000E+0\t0.000000E+0\t0.000000E+0\t0.000000E+0\t0.000000E+0\t0.000000E+0\t0.000000E+0\t0.000000E+0\t0.000000E+0\t0.000000E+0\t0.000000E+0\t0.000000E+0\t0.000000E+0\t0.000000E+0\t0.000000E+0\t0.000000E+0\t0.000000E+0\t0.000000E+0\t0.000000E+0\t0.000000E+0\r\n1.092729E+0\t0.000000E+0\t0.000000E+0\t0.000000E+0\t0.000000E+0\t0.000000E+0\t0.000000E+0\t0.000000E+0\t0.000000E+0\t0.000000E+0\t0.000000E+0\t0.000000E+0\t0.000000E+0\t0.000000E+0\t0.000000E+0\t0.000000E+0\t0.000000E+0\t0.000000E+0\t0.000000E+0\t0.000000E+0\t0.000000E+0\t0.000000E+0\t0.000000E+0\t0.000000E+0\t0.000000E+0\t0.000000E+0\t0.000000E+0\t0.000000E+0\t0.000000E+0\t0.000000E+0\t0.000000E+0\t0.000000E+0\t0.000000E+0\t0.000000E+0\t0.000000E+0\t8.840374E-3\t3.949578E-2\t7.921957E-2\t1.280508E-1\t1.853754E-1\t2.498965E-1\t3.196884E-1\t3.923377E-1\t4.651550E-1\t5.354279E-1\t6.006705E-1\t6.588195E-1\t7.083268E-1\t7.481003E-1\t7.772294E-1\t7.942988E-1\t7.942988E-1\t7.772294E-1\t7.481003E-1\t7.083268E-1\t6.588195E-1\t6.006705E-1\t5.354279E-1\t4.651550E-1\t3.923377E-1\t3.196884E-1\t2.498965E-1\t1.853754E-1\t1.280508E-1\t7.921957E-2\t3.949578E-2\t8.840374E-3\t0.000000E+0\t0.000000E+0\t0.000000E+0\t0.000000E+0\t0.000000E+0\t0.000000E+0\t0.000000E+0\t0.000000E+0\t0.000000E+0\t0.000000E+0\t0.000000E+0\t0.000000E+0\t0.000000E+0\t0.000000E+0\t0.000000E+0\t0.000000E+0\t0.000000E+0\t0.000000E+0\t0.000000E+0\t0.000000E+0\t0.000000E+0\t0.000000E+0\t0.000000E+0\t0.000000E+0\t0.000000E+0\t0.000000E+0\t0.000000E+0\t0.000000E+0\t0.000000E+0\t0.000000E+0\t0.000000E+0\t0.000000E+0\t0.000000E+0\t0.000000E+0\r\n1.137687E+0\t0.000000E+0\t0.000000E+0\t0.000000E+0\t0.000000E+0\t0.000000E+0\t0.000000E+0\t0.000000E+0\t0.000000E+0\t0.000000E+0\t0.000000E+0\t0.000000E+0\t0.000000E+0\t0.000000E+0\t0.000000E+0\t0.000000E+0\t0.000000E+0\t0.000000E+0\t0.000000E+0\t0.000000E+0\t0.000000E+0\t0.000000E+0\t0.000000E+0\t0.000000E+0\t0.000000E+0\t0.000000E+0\t0.000000E+0\t0.000000E+0\t0.000000E+0\t0.000000E+0\t0.000000E+0\t0.000000E+0\t0.000000E+0\t0.000000E+0\t1.685035E-4\t2.221717E-2\t5.194767E-2\t8.980467E-2\t1.357207E-1\t1.890349E-1\t2.484761E-1\t3.122236E-1\t3.780452E-1\t4.434979E-1\t5.061617E-1\t5.638663E-1\t6.148638E-1\t6.579055E-1\t6.921796E-1\t7.170611E-1\t7.315146E-1\t7.315146E-1\t7.170611E-1\t6.921796E-1\t6.579055E-1\t6.148638E-1\t5.638663E-1\t5.061617E-1\t4.434979E-1\t3.780452E-1\t3.122236E-1\t2.484761E-1\t1.890349E-1\t1.357207E-1\t8.980467E-2\t5.194767E-2\t2.221717E-2\t1.685035E-4\t0.000000E+0\t0.000000E+0\t0.000000E+0\t0.000000E+0\t0.000000E+0\t0.000000E+0\t0.000000E+0\t0.000000E+0\t0.000000E+0\t0.000000E+0\t0.000000E+0\t0.000000E+0\t0.000000E+0\t0.000000E+0\t0.000000E+0\t0.000000E+0\t0.000000E+0\t0.000000E+0\t0.000000E+0\t0.000000E+0\t0.000000E+0\t0.000000E+0\t0.000000E+0\t0.000000E+0\t0.000000E+0\t0.000000E+0\t0.000000E+0\t0.000000E+0\t0.000000E+0\t0.000000E+0\t0.000000E+0\t0.000000E+0\t0.000000E+0\r\n1.182645E+0\t0.000000E+0\t0.000000E+0\t0.000000E+0\t0.000000E+0\t0.000000E+0\t0.000000E+0\t0.000000E+0\t0.000000E+0\t0.000000E+0\t0.000000E+0\t0.000000E+0\t0.000000E+0\t0.000000E+0\t0.000000E+0\t0.000000E+0\t0.000000E+0\t0.000000E+0\t0.000000E+0\t0.000000E+0\t0.000000E+0\t0.000000E+0\t0.000000E+0\t0.000000E+0\t0.000000E+0\t0.000000E+0\t0.000000E+0\t0.000000E+0\t0.000000E+0\t0.000000E+0\t0.000000E+0\t0.000000E+0\t0.000000E+0\t0.000000E+0\t1.075635E-2\t3.227016E-2\t6.069213E-2\t9.634066E-2\t1.390645E-1\t1.881771E-1\t2.424510E-1\t3.001828E-1\t3.593264E-1\t4.176817E-1\t4.731087E-1\t5.237313E-1\t5.680888E-1\t6.051967E-1\t6.344826E-1\t6.555579E-1\t6.676987E-1\t6.676987E-1\t6.555579E-1\t6.344826E-1\t6.051967E-1\t5.680888E-1\t5.237313E-1\t4.731087E-1\t4.176817E-1\t3.593264E-1\t3.001828E-1\t2.424510E-1\t1.881771E-1\t1.390645E-1\t9.634066E-2\t6.069213E-2\t3.227016E-2\t1.075635E-2\t0.000000E+0\t0.000000E+0\t0.000000E+0\t0.000000E+0\t0.000000E+0\t0.000000E+0\t0.000000E+0\t0.000000E+0\t0.000000E+0\t0.000000E+0\t0.000000E+0\t0.000000E+0\t0.000000E+0\t0.000000E+0\t0.000000E+0\t0.000000E+0\t0.000000E+0\t0.000000E+0\t0.000000E+0\t0.000000E+0\t0.000000E+0\t0.000000E+0\t0.000000E+0\t0.000000E+0\t0.000000E+0\t0.000000E+0\t0.000000E+0\t0.000000E+0\t0.000000E+0\t0.000000E+0\t0.000000E+0\t0.000000E+0\t0.000000E+0\r\n1.227602E+0\t0.000000E+0\t0.000000E+0\t0.000000E+0\t0.000000E+0\t0.000000E+0\t0.000000E+0\t0.000000E+0\t0.000000E+0\t0.000000E+0\t0.000000E+0\t0.000000E+0\t0.000000E+0\t0.000000E+0\t0.000000E+0\t0.000000E+0\t0.000000E+0\t0.000000E+0\t0.000000E+0\t0.000000E+0\t0.000000E+0\t0.000000E+0\t0.000000E+0\t0.000000E+0\t0.000000E+0\t0.000000E+0\t0.000000E+0\t0.000000E+0\t0.000000E+0\t0.000000E+0\t0.000000E+0\t0.000000E+0\t0.000000E+0\t3.681199E-3\t1.871773E-2\t3.937014E-2\t6.618740E-2\t9.938220E-2\t1.387399E-1\t1.835669E-1\t2.326937E-1\t2.845419E-1\t3.372527E-1\t3.888609E-1\t4.374908E-1\t4.815371E-1\t5.197967E-1\t5.515146E-1\t5.763195E-1\t5.940144E-1\t6.041268E-1\t6.041268E-1\t5.940144E-1\t5.763195E-1\t5.515146E-1\t5.197967E-1\t4.815371E-1\t4.374908E-1\t3.888609E-1\t3.372527E-1\t2.845419E-1\t2.326937E-1\t1.835669E-1\t1.387399E-1\t9.938220E-2\t6.618740E-2\t3.937014E-2\t1.871773E-2\t3.681199E-3\t0.000000E+0\t0.000000E+0\t0.000000E+0\t0.000000E+0\t0.000000E+0\t0.000000E+0\t0.000000E+0\t0.000000E+0\t0.000000E+0\t0.000000E+0\t0.000000E+0\t0.000000E+0\t0.000000E+0\t0.000000E+0\t0.000000E+0\t0.000000E+0\t0.000000E+0\t0.000000E+0\t0.000000E+0\t0.000000E+0\t0.000000E+0\t0.000000E+0\t0.000000E+0\t0.000000E+0\t0.000000E+0\t0.000000E+0\t0.000000E+0\t0.000000E+0\t0.000000E+0\t0.000000E+0\t0.000000E+0\t0.000000E+0\r\n1.272560E+0\t0.000000E+0\t0.000000E+0\t0.000000E+0\t0.000000E+0\t0.000000E+0\t0.000000E+0\t0.000000E+0\t0.000000E+0\t0.000000E+0\t0.000000E+0\t0.000000E+0\t0.000000E+0\t0.000000E+0\t0.000000E+0\t0.000000E+0\t0.000000E+0\t0.000000E+0\t0.000000E+0\t0.000000E+0\t0.000000E+0\t0.000000E+0\t0.000000E+0\t0.000000E+0\t0.000000E+0\t0.000000E+0\t0.000000E+0\t0.000000E+0\t0.000000E+0\t0.000000E+0\t0.000000E+0\t0.000000E+0\t0.000000E+0\t9.858804E-3\t2.437298E-2\t4.391227E-2\t6.891183E-2\t9.949760E-2\t1.354097E-1\t1.759626E-1\t2.200556E-1\t2.662399E-1\t3.128407E-1\t3.581173E-1\t4.004396E-1\t4.384485E-1\t4.711682E-1\t4.980406E-1\t5.188592E-1\t5.335793E-1\t5.419270E-1\t5.419270E-1\t5.335793E-1\t5.188592E-1\t4.980406E-1\t4.711682E-1\t4.384485E-1\t4.004396E-1\t3.581173E-1\t3.128407E-1\t2.662399E-1\t2.200556E-1\t1.759626E-1\t1.354097E-1\t9.949760E-2\t6.891183E-2\t4.391227E-2\t2.437298E-2\t9.858804E-3\t0.000000E+0\t0.000000E+0\t0.000000E+0\t0.000000E+0\t0.000000E+0\t0.000000E+0\t0.000000E+0\t0.000000E+0\t0.000000E+0\t0.000000E+0\t0.000000E+0\t0.000000E+0\t0.000000E+0\t0.000000E+0\t0.000000E+0\t0.000000E+0\t0.000000E+0\t0.000000E+0\t0.000000E+0\t0.000000E+0\t0.000000E+0\t0.000000E+0\t0.000000E+0\t0.000000E+0\t0.000000E+0\t0.000000E+0\t0.000000E+0\t0.000000E+0\t0.000000E+0\t0.000000E+0\t0.000000E+0\t0.000000E+0\r\n1.317518E+0\t0.000000E+0\t0.000000E+0\t0.000000E+0\t0.000000E+0\t0.000000E+0\t0.000000E+0\t0.000000E+0\t0.000000E+0\t0.000000E+0\t0.000000E+0\t0.000000E+0\t0.000000E+0\t0.000000E+0\t0.000000E+0\t0.000000E+0\t0.000000E+0\t0.000000E+0\t0.000000E+0\t0.000000E+0\t0.000000E+0\t0.000000E+0\t0.000000E+0\t0.000000E+0\t0.000000E+0\t0.000000E+0\t0.000000E+0\t0.000000E+0\t0.000000E+0\t0.000000E+0\t0.000000E+0\t0.000000E+0\t4.414101E-3\t1.427091E-2\t2.805312E-2\t4.629781E-2\t6.934322E-2\t9.724567E-2\t1.297157E-1\t1.660883E-1\t2.053389E-1\t2.461498E-1\t2.870237E-1\t3.264313E-1\t3.629679E-1\t3.954954E-1\t4.232361E-1\t4.457972E-1\t4.631050E-1\t4.752315E-1\t4.820573E-1\t4.820573E-1\t4.752315E-1\t4.631050E-1\t4.457972E-1\t4.232361E-1\t3.954954E-1\t3.629679E-1\t3.264313E-1\t2.870237E-1\t2.461498E-1\t2.053389E-1\t1.660883E-1\t1.297157E-1\t9.724567E-2\t6.934322E-2\t4.629781E-2\t2.805312E-2\t1.427091E-2\t4.414101E-3\t0.000000E+0\t0.000000E+0\t0.000000E+0\t0.000000E+0\t0.000000E+0\t0.000000E+0\t0.000000E+0\t0.000000E+0\t0.000000E+0\t0.000000E+0\t0.000000E+0\t0.000000E+0\t0.000000E+0\t0.000000E+0\t0.000000E+0\t0.000000E+0\t0.000000E+0\t0.000000E+0\t0.000000E+0\t0.000000E+0\t0.000000E+0\t0.000000E+0\t0.000000E+0\t0.000000E+0\t0.000000E+0\t0.000000E+0\t0.000000E+0\t0.000000E+0\t0.000000E+0\t0.000000E+0\t0.000000E+0\r\n1.362476E+0\t0.000000E+0\t0.000000E+0\t0.000000E+0\t0.000000E+0\t0.000000E+0\t0.000000E+0\t0.000000E+0\t0.000000E+0\t0.000000E+0\t0.000000E+0\t0.000000E+0\t0.000000E+0\t0.000000E+0\t0.000000E+0\t0.000000E+0\t0.000000E+0\t0.000000E+0\t0.000000E+0\t0.000000E+0\t0.000000E+0\t0.000000E+0\t0.000000E+0\t0.000000E+0\t0.000000E+0\t0.000000E+0\t0.000000E+0\t0.000000E+0\t0.000000E+0\t0.000000E+0\t0.000000E+0\t1.320619E-3\t7.781649E-3\t1.718730E-2\t3.008594E-2\t4.691831E-2\t6.794129E-2\t9.315671E-2\t1.222588E-1\t1.546128E-1\t1.892746E-1\t2.250559E-1\t2.606289E-1\t2.946599E-1\t3.259493E-1\t3.535541E-1\t3.768673E-1\t3.956325E-1\t4.098792E-1\t4.197667E-1\t4.252916E-1\t4.252916E-1\t4.197667E-1\t4.098792E-1\t3.956325E-1\t3.768673E-1\t3.535541E-1\t3.259493E-1\t2.946599E-1\t2.606289E-1\t2.250559E-1\t1.892746E-1\t1.546128E-1\t1.222588E-1\t9.315671E-2\t6.794129E-2\t4.691831E-2\t3.008594E-2\t1.718730E-2\t7.781649E-3\t1.320619E-3\t0.000000E+0\t0.000000E+0\t0.000000E+0\t0.000000E+0\t0.000000E+0\t0.000000E+0\t0.000000E+0\t0.000000E+0\t0.000000E+0\t0.000000E+0\t0.000000E+0\t0.000000E+0\t0.000000E+0\t0.000000E+0\t0.000000E+0\t0.000000E+0\t0.000000E+0\t0.000000E+0\t0.000000E+0\t0.000000E+0\t0.000000E+0\t0.000000E+0\t0.000000E+0\t0.000000E+0\t0.000000E+0\t0.000000E+0\t0.000000E+0\t0.000000E+0\t0.000000E+0\t0.000000E+0\r\n1.407434E+0\t0.000000E+0\t0.000000E+0\t0.000000E+0\t0.000000E+0\t0.000000E+0\t0.000000E+0\t0.000000E+0\t0.000000E+0\t0.000000E+0\t0.000000E+0\t0.000000E+0\t0.000000E+0\t0.000000E+0\t0.000000E+0\t0.000000E+0\t0.000000E+0\t0.000000E+0\t0.000000E+0\t0.000000E+0\t0.000000E+0\t0.000000E+0\t0.000000E+0\t0.000000E+0\t0.000000E+0\t0.000000E+0\t0.000000E+0\t0.000000E+0\t0.000000E+0\t0.000000E+0\t0.000000E+0\t3.832863E-3\t1.003860E-2\t1.886907E-2\t3.078453E-2\t4.614295E-2\t6.513381E-2\t8.771773E-2\t1.135835E-1\t1.421336E-1\t1.725068E-1\t2.036398E-1\t2.343639E-1\t2.635252E-1\t2.901076E-1\t3.133390E-1\t3.327566E-1\t3.482143E-1\t3.598198E-1\t3.677935E-1\t3.722168E-1\t3.722168E-1\t3.677935E-1\t3.598198E-1\t3.482143E-1\t3.327566E-1\t3.133390E-1\t2.901076E-1\t2.635252E-1\t2.343639E-1\t2.036398E-1\t1.725068E-1\t1.421336E-1\t1.135835E-1\t8.771773E-2\t6.513381E-2\t4.614295E-2\t3.078453E-2\t1.886907E-2\t1.003860E-2\t3.832863E-3\t0.000000E+0\t0.000000E+0\t0.000000E+0\t0.000000E+0\t0.000000E+0\t0.000000E+0\t0.000000E+0\t0.000000E+0\t0.000000E+0\t0.000000E+0\t0.000000E+0\t0.000000E+0\t0.000000E+0\t0.000000E+0\t0.000000E+0\t0.000000E+0\t0.000000E+0\t0.000000E+0\t0.000000E+0\t0.000000E+0\t0.000000E+0\t0.000000E+0\t0.000000E+0\t0.000000E+0\t0.000000E+0\t0.000000E+0\t0.000000E+0\t0.000000E+0\t0.000000E+0\t0.000000E+0\r\n1.452391E+0\t0.000000E+0\t0.000000E+0\t0.000000E+0\t0.000000E+0\t0.000000E+0\t0.000000E+0\t0.000000E+0\t0.000000E+0\t0.000000E+0\t0.000000E+0\t0.000000E+0\t0.000000E+0\t0.000000E+0\t0.000000E+0\t0.000000E+0\t0.000000E+0\t0.000000E+0\t0.000000E+0\t0.000000E+0\t0.000000E+0\t0.000000E+0\t0.000000E+0\t0.000000E+0\t0.000000E+0\t0.000000E+0\t0.000000E+0\t0.000000E+0\t0.000000E+0\t0.000000E+0\t1.582114E-3\t5.536715E-3\t1.138788E-2\t1.956064E-2\t3.043847E-2\t4.430894E-2\t6.130663E-2\t8.136220E-2\t1.041677E-1\t1.291679E-1\t1.555840E-1\t1.824720E-1\t2.088109E-1\t2.336094E-1\t2.560143E-1\t2.754011E-1\t2.914272E-1\t3.040335E-1\t3.133840E-1\t3.197390E-1\t3.232387E-1\t3.232387E-1\t3.197390E-1\t3.133840E-1\t3.040335E-1\t2.914272E-1\t2.754011E-1\t2.560143E-1\t2.336094E-1\t2.088109E-1\t1.824720E-1\t1.555840E-1\t1.291679E-1\t1.041677E-1\t8.136220E-2\t6.130663E-2\t4.430894E-2\t3.043847E-2\t1.956064E-2\t1.138788E-2\t5.536715E-3\t1.582114E-3\t0.000000E+0\t0.000000E+0\t0.000000E+0\t0.000000E+0\t0.000000E+0\t0.000000E+0\t0.000000E+0\t0.000000E+0\t0.000000E+0\t0.000000E+0\t0.000000E+0\t0.000000E+0\t0.000000E+0\t0.000000E+0\t0.000000E+0\t0.000000E+0\t0.000000E+0\t0.000000E+0\t0.000000E+0\t0.000000E+0\t0.000000E+0\t0.000000E+0\t0.000000E+0\t0.000000E+0\t0.000000E+0\t0.000000E+0\t0.000000E+0\t0.000000E+0\t0.000000E+0\r\n1.497349E+0\t0.000000E+0\t0.000000E+0\t0.000000E+0\t0.000000E+0\t0.000000E+0\t0.000000E+0\t0.000000E+0\t0.000000E+0\t0.000000E+0\t0.000000E+0\t0.000000E+0\t0.000000E+0\t0.000000E+0\t0.000000E+0\t0.000000E+0\t0.000000E+0\t0.000000E+0\t0.000000E+0\t0.000000E+0\t0.000000E+0\t0.000000E+0\t0.000000E+0\t0.000000E+0\t0.000000E+0\t0.000000E+0\t0.000000E+0\t0.000000E+0\t0.000000E+0\t4.053376E-4\t2.836092E-3\t6.586182E-3\t1.201593E-2\t1.948405E-2\t2.930773E-2\t4.171530E-2\t5.679734E-2\t7.446403E-2\t9.441751E-2\t1.161475E-1\t1.389559E-1\t1.620109E-1\t1.844265E-1\t2.053576E-1\t2.240935E-1\t2.401357E-1\t2.532402E-1\t2.634145E-1\t2.708605E-1\t2.758610E-1\t2.785944E-1\t2.785944E-1\t2.758610E-1\t2.708605E-1\t2.634145E-1\t2.532402E-1\t2.401357E-1\t2.240935E-1\t2.053576E-1\t1.844265E-1\t1.620109E-1\t1.389559E-1\t1.161475E-1\t9.441751E-2\t7.446403E-2\t5.679734E-2\t4.171530E-2\t2.930773E-2\t1.948405E-2\t1.201593E-2\t6.586182E-3\t2.836092E-3\t4.053376E-4\t0.000000E+0\t0.000000E+0\t0.000000E+0\t0.000000E+0\t0.000000E+0\t0.000000E+0\t0.000000E+0\t0.000000E+0\t0.000000E+0\t0.000000E+0\t0.000000E+0\t0.000000E+0\t0.000000E+0\t0.000000E+0\t0.000000E+0\t0.000000E+0\t0.000000E+0\t0.000000E+0\t0.000000E+0\t0.000000E+0\t0.000000E+0\t0.000000E+0\t0.000000E+0\t0.000000E+0\t0.000000E+0\t0.000000E+0\t0.000000E+0\t0.000000E+0\r\n1.542307E+0\t0.000000E+0\t0.000000E+0\t0.000000E+0\t0.000000E+0\t0.000000E+0\t0.000000E+0\t0.000000E+0\t0.000000E+0\t0.000000E+0\t0.000000E+0\t0.000000E+0\t0.000000E+0\t0.000000E+0\t0.000000E+0\t0.000000E+0\t0.000000E+0\t0.000000E+0\t0.000000E+0\t0.000000E+0\t0.000000E+0\t0.000000E+0\t0.000000E+0\t0.000000E+0\t0.000000E+0\t0.000000E+0\t0.000000E+0\t0.000000E+0\t0.000000E+0\t1.304719E-3\t3.627547E-3\t7.120251E-3\t1.208920E-2\t1.883533E-2\t2.761905E-2\t3.861940E-2\t5.189237E-2\t6.733542E-2\t8.466576E-2\t1.034194E-1\t1.229755E-1\t1.426062E-1\t1.615481E-1\t1.790856E-1\t1.946319E-1\t2.077944E-1\t2.184086E-1\t2.265312E-1\t2.323866E-1\t2.362665E-1\t2.383709E-1\t2.383709E-1\t2.362665E-1\t2.323866E-1\t2.265312E-1\t2.184086E-1\t2.077944E-1\t1.946319E-1\t1.790856E-1\t1.615481E-1\t1.426062E-1\t1.229755E-1\t1.034194E-1\t8.466576E-2\t6.733542E-2\t5.189237E-2\t3.861940E-2\t2.761905E-2\t1.883533E-2\t1.208920E-2\t7.120251E-3\t3.627547E-3\t1.304719E-3\t0.000000E+0\t0.000000E+0\t0.000000E+0\t0.000000E+0\t0.000000E+0\t0.000000E+0\t0.000000E+0\t0.000000E+0\t0.000000E+0\t0.000000E+0\t0.000000E+0\t0.000000E+0\t0.000000E+0\t0.000000E+0\t0.000000E+0\t0.000000E+0\t0.000000E+0\t0.000000E+0\t0.000000E+0\t0.000000E+0\t0.000000E+0\t0.000000E+0\t0.000000E+0\t0.000000E+0\t0.000000E+0\t0.000000E+0\t0.000000E+0\t0.000000E+0\r\n1.587265E+0\t0.000000E+0\t0.000000E+0\t0.000000E+0\t0.000000E+0\t0.000000E+0\t0.000000E+0\t0.000000E+0\t0.000000E+0\t0.000000E+0\t0.000000E+0\t0.000000E+0\t0.000000E+0\t0.000000E+0\t0.000000E+0\t0.000000E+0\t0.000000E+0\t0.000000E+0\t0.000000E+0\t0.000000E+0\t0.000000E+0\t0.000000E+0\t0.000000E+0\t0.000000E+0\t0.000000E+0\t0.000000E+0\t0.000000E+0\t0.000000E+0\t4.947565E-4\t1.883685E-3\t4.057794E-3\t7.261009E-3\t1.175237E-2\t1.778279E-2\t2.556457E-2\t3.523615E-2\t4.682691E-2\t6.022783E-2\t7.517466E-2\t9.124954E-2\t1.079045E-1\t1.245072E-1\t1.404040E-1\t1.549931E-1\t1.677940E-1\t1.785023E-1\t1.870162E-1\t1.934268E-1\t1.979691E-1\t2.009328E-1\t2.025268E-1\t2.025268E-1\t2.009328E-1\t1.979691E-1\t1.934268E-1\t1.870162E-1\t1.785023E-1\t1.677940E-1\t1.549931E-1\t1.404040E-1\t1.245072E-1\t1.079045E-1\t9.124954E-2\t7.517466E-2\t6.022783E-2\t4.682691E-2\t3.523615E-2\t2.556457E-2\t1.778279E-2\t1.175237E-2\t7.261009E-3\t4.057794E-3\t1.883685E-3\t4.947565E-4\t0.000000E+0\t0.000000E+0\t0.000000E+0\t0.000000E+0\t0.000000E+0\t0.000000E+0\t0.000000E+0\t0.000000E+0\t0.000000E+0\t0.000000E+0\t0.000000E+0\t0.000000E+0\t0.000000E+0\t0.000000E+0\t0.000000E+0\t0.000000E+0\t0.000000E+0\t0.000000E+0\t0.000000E+0\t0.000000E+0\t0.000000E+0\t0.000000E+0\t0.000000E+0\t0.000000E+0\t0.000000E+0\t0.000000E+0\t0.000000E+0\r\n1.632222E+0\t0.000000E+0\t0.000000E+0\t0.000000E+0\t0.000000E+0\t0.000000E+0\t0.000000E+0\t0.000000E+0\t0.000000E+0\t0.000000E+0\t0.000000E+0\t0.000000E+0\t0.000000E+0\t0.000000E+0\t0.000000E+0\t0.000000E+0\t0.000000E+0\t0.000000E+0\t0.000000E+0\t0.000000E+0\t0.000000E+0\t0.000000E+0\t0.000000E+0\t0.000000E+0\t0.000000E+0\t0.000000E+0\t0.000000E+0\t1.052978E-4\t9.058000E-4\t2.214467E-3\t4.214441E-3\t7.112937E-3\t1.112778E-2\t1.646699E-2\t2.330234E-2\t3.173928E-2\t4.178722E-2\t5.333554E-2\t6.614074E-2\t7.982983E-2\t9.392274E-2\t1.078735E-1\t1.211263E-1\t1.331781E-1\t1.436390E-1\t1.522768E-1\t1.590380E-1\t1.640363E-1\t1.675075E-1\t1.697314E-1\t1.709163E-1\t1.709163E-1\t1.697314E-1\t1.675075E-1\t1.640363E-1\t1.590380E-1\t1.522768E-1\t1.436390E-1\t1.331781E-1\t1.211263E-1\t1.078735E-1\t9.392274E-2\t7.982983E-2\t6.614074E-2\t5.333554E-2\t4.178722E-2\t3.173928E-2\t2.330234E-2\t1.646699E-2\t1.112778E-2\t7.112937E-3\t4.214441E-3\t2.214467E-3\t9.058000E-4\t1.052978E-4\t0.000000E+0\t0.000000E+0\t0.000000E+0\t0.000000E+0\t0.000000E+0\t0.000000E+0\t0.000000E+0\t0.000000E+0\t0.000000E+0\t0.000000E+0\t0.000000E+0\t0.000000E+0\t0.000000E+0\t0.000000E+0\t0.000000E+0\t0.000000E+0\t0.000000E+0\t0.000000E+0\t0.000000E+0\t0.000000E+0\t0.000000E+0\t0.000000E+0\t0.000000E+0\t0.000000E+0\t0.000000E+0\t0.000000E+0\r\n1.677180E+0\t0.000000E+0\t0.000000E+0\t0.000000E+0\t0.000000E+0\t0.000000E+0\t0.000000E+0\t0.000000E+0\t0.000000E+0\t0.000000E+0\t0.000000E+0\t0.000000E+0\t0.000000E+0\t0.000000E+0\t0.000000E+0\t0.000000E+0\t0.000000E+0\t0.000000E+0\t0.000000E+0\t0.000000E+0\t0.000000E+0\t0.000000E+0\t0.000000E+0\t0.000000E+0\t0.000000E+0\t0.000000E+0\t0.000000E+0\t3.887008E-4\t1.149716E-3\t2.358592E-3\t4.171368E-3\t6.763152E-3\t1.031614E-2\t1.500183E-2\t2.095819E-2\t2.826413E-2\t3.691459E-2\t4.680103E-2\t5.770179E-2\t6.928675E-2\t8.113823E-2\t9.278787E-2\t1.037656E-1\t1.136542E-1\t1.221394E-1\t1.290479E-1\t1.343621E-1\t1.382087E-1\t1.408172E-1\t1.424516E-1\t1.433131E-1\t1.433131E-1\t1.424516E-1\t1.408172E-1\t1.382087E-1\t1.343621E-1\t1.290479E-1\t1.221394E-1\t1.136542E-1\t1.037656E-1\t9.278787E-2\t8.113823E-2\t6.928675E-2\t5.770179E-2\t4.680103E-2\t3.691459E-2\t2.826413E-2\t2.095819E-2\t1.500183E-2\t1.031614E-2\t6.763152E-3\t4.171368E-3\t2.358592E-3\t1.149716E-3\t3.887008E-4\t0.000000E+0\t0.000000E+0\t0.000000E+0\t0.000000E+0\t0.000000E+0\t0.000000E+0\t0.000000E+0\t0.000000E+0\t0.000000E+0\t0.000000E+0\t0.000000E+0\t0.000000E+0\t0.000000E+0\t0.000000E+0\t0.000000E+0\t0.000000E+0\t0.000000E+0\t0.000000E+0\t0.000000E+0\t0.000000E+0\t0.000000E+0\t0.000000E+0\t0.000000E+0\t0.000000E+0\t0.000000E+0\t0.000000E+0\r\n1.722138E+0\t0.000000E+0\t0.000000E+0\t0.000000E+0\t0.000000E+0\t0.000000E+0\t0.000000E+0\t0.000000E+0\t0.000000E+0\t0.000000E+0\t0.000000E+0\t0.000000E+0\t0.000000E+0\t0.000000E+0\t0.000000E+0\t0.000000E+0\t0.000000E+0\t0.000000E+0\t0.000000E+0\t0.000000E+0\t0.000000E+0\t0.000000E+0\t0.000000E+0\t0.000000E+0\t0.000000E+0\t0.000000E+0\t1.348436E-4\t5.618309E-4\t1.268796E-3\t2.367211E-3\t3.989332E-3\t6.282381E-3\t9.397990E-3\t1.347675E-2\t1.862868E-2\t2.491161E-2\t3.231046E-2\t4.072140E-2\t4.994493E-2\t5.969114E-2\t6.959904E-2\t7.926928E-2\t8.830678E-2\t9.636727E-2\t1.032000E-1\t1.086783E-1\t1.128108E-1\t1.157295E-1\t1.176521E-1\t1.188235E-1\t1.194328E-1\t1.194328E-1\t1.188235E-1\t1.176521E-1\t1.157295E-1\t1.128108E-1\t1.086783E-1\t1.032000E-1\t9.636727E-2\t8.830678E-2\t7.926928E-2\t6.959904E-2\t5.969114E-2\t4.994493E-2\t4.072140E-2\t3.231046E-2\t2.491161E-2\t1.862868E-2\t1.347675E-2\t9.397990E-3\t6.282381E-3\t3.989332E-3\t2.367211E-3\t1.268796E-3\t5.618309E-4\t1.348436E-4\t0.000000E+0\t0.000000E+0\t0.000000E+0\t0.000000E+0\t0.000000E+0\t0.000000E+0\t0.000000E+0\t0.000000E+0\t0.000000E+0\t0.000000E+0\t0.000000E+0\t0.000000E+0\t0.000000E+0\t0.000000E+0\t0.000000E+0\t0.000000E+0\t0.000000E+0\t0.000000E+0\t0.000000E+0\t0.000000E+0\t0.000000E+0\t0.000000E+0\t0.000000E+0\t0.000000E+0\t0.000000E+0\r\n1.767096E+0\t0.000000E+0\t0.000000E+0\t0.000000E+0\t0.000000E+0\t0.000000E+0\t0.000000E+0\t0.000000E+0\t0.000000E+0\t0.000000E+0\t0.000000E+0\t0.000000E+0\t0.000000E+0\t0.000000E+0\t0.000000E+0\t0.000000E+0\t0.000000E+0\t0.000000E+0\t0.000000E+0\t0.000000E+0\t0.000000E+0\t0.000000E+0\t0.000000E+0\t0.000000E+0\t0.000000E+0\t2.271382E-5\t2.534532E-4\t6.531471E-4\t1.297723E-3\t2.281832E-3\t3.717009E-3\t5.726431E-3\t8.435671E-3\t1.195938E-2\t1.638463E-2\t2.175274E-2\t2.804210E-2\t3.515548E-2\t4.291508E-2\t5.106821E-2\t5.930489E-2\t6.728657E-2\t7.468303E-2\t8.121203E-2\t8.667506E-2\t9.098218E-2\t9.416019E-2\t9.634034E-2\t9.772553E-2\t9.853887E-2\t9.895476E-2\t9.895476E-2\t9.853887E-2\t9.772553E-2\t9.634034E-2\t9.416019E-2\t9.098218E-2\t8.667506E-2\t8.121203E-2\t7.468303E-2\t6.728657E-2\t5.930489E-2\t5.106821E-2\t4.291508E-2\t3.515548E-2\t2.804210E-2\t2.175274E-2\t1.638463E-2\t1.195938E-2\t8.435671E-3\t5.726431E-3\t3.717009E-3\t2.281832E-3\t1.297723E-3\t6.531471E-4\t2.534532E-4\t2.271382E-5\t0.000000E+0\t0.000000E+0\t0.000000E+0\t0.000000E+0\t0.000000E+0\t0.000000E+0\t0.000000E+0\t0.000000E+0\t0.000000E+0\t0.000000E+0\t0.000000E+0\t0.000000E+0\t0.000000E+0\t0.000000E+0\t0.000000E+0\t0.000000E+0\t0.000000E+0\t0.000000E+0\t0.000000E+0\t0.000000E+0\t0.000000E+0\t0.000000E+0\t0.000000E+0\t0.000000E+0\r\n1.812053E+0\t0.000000E+0\t0.000000E+0\t0.000000E+0\t0.000000E+0\t0.000000E+0\t0.000000E+0\t0.000000E+0\t0.000000E+0\t0.000000E+0\t0.000000E+0\t0.000000E+0\t0.000000E+0\t0.000000E+0\t0.000000E+0\t0.000000E+0\t0.000000E+0\t0.000000E+0\t0.000000E+0\t0.000000E+0\t0.000000E+0\t0.000000E+0\t0.000000E+0\t0.000000E+0\t0.000000E+0\t1.013116E-4\t3.195368E-4\t6.856775E-4\t1.264274E-3\t2.135290E-3\t3.392330E-3\t5.137971E-3\t7.475715E-3\t1.049857E-2\t1.427494E-2\t1.883339E-2\t2.414852E-2\t3.013082E-2\t3.662331E-2\t4.340731E-2\t5.021825E-2\t5.677075E-2\t6.279030E-2\t6.804687E-2\t7.238461E-2\t7.574203E-2\t7.815750E-2\t7.975757E-2\t8.072792E-2\t8.126919E-2\t8.153933E-2\t8.153933E-2\t8.126919E-2\t8.072792E-2\t7.975757E-2\t7.815750E-2\t7.574203E-2\t7.238461E-2\t6.804687E-2\t6.279030E-2\t5.677075E-2\t5.021825E-2\t4.340731E-2\t3.662331E-2\t3.013082E-2\t2.414852E-2\t1.883339E-2\t1.427494E-2\t1.049857E-2\t7.475715E-3\t5.137971E-3\t3.392330E-3\t2.135290E-3\t1.264274E-3\t6.856775E-4\t3.195368E-4\t1.013116E-4\t0.000000E+0\t0.000000E+0\t0.000000E+0\t0.000000E+0\t0.000000E+0\t0.000000E+0\t0.000000E+0\t0.000000E+0\t0.000000E+0\t0.000000E+0\t0.000000E+0\t0.000000E+0\t0.000000E+0\t0.000000E+0\t0.000000E+0\t0.000000E+0\t0.000000E+0\t0.000000E+0\t0.000000E+0\t0.000000E+0\t0.000000E+0\t0.000000E+0\t0.000000E+0\t0.000000E+0\r\n1.857011E+0\t0.000000E+0\t0.000000E+0\t0.000000E+0\t0.000000E+0\t0.000000E+0\t0.000000E+0\t0.000000E+0\t0.000000E+0\t0.000000E+0\t0.000000E+0\t0.000000E+0\t0.000000E+0\t0.000000E+0\t0.000000E+0\t0.000000E+0\t0.000000E+0\t0.000000E+0\t0.000000E+0\t0.000000E+0\t0.000000E+0\t0.000000E+0\t0.000000E+0\t0.000000E+0\t3.198920E-5\t1.468821E-4\t3.480693E-4\t6.776350E-4\t1.190157E-3\t1.952862E-3\t3.043945E-3\t4.548440E-3\t6.551270E-3\t9.127506E-3\t1.233048E-2\t1.617906E-2\t2.064613E-2\t2.565048E-2\t3.105474E-2\t3.667093E-2\t4.227455E-2\t4.762635E-2\t5.249934E-2\t5.670707E-2\t6.012826E-2\t6.272297E-2\t6.453618E-2\t6.568684E-2\t6.634234E-2\t6.668091E-2\t6.684349E-2\t6.684349E-2\t6.668091E-2\t6.634234E-2\t6.568684E-2\t6.453618E-2\t6.272297E-2\t6.012826E-2\t5.670707E-2\t5.249934E-2\t4.762635E-2\t4.227455E-2\t3.667093E-2\t3.105474E-2\t2.565048E-2\t2.064613E-2\t1.617906E-2\t1.233048E-2\t9.127506E-3\t6.551270E-3\t4.548440E-3\t3.043945E-3\t1.952862E-3\t1.190157E-3\t6.776350E-4\t3.480693E-4\t1.468821E-4\t3.198920E-5\t0.000000E+0\t0.000000E+0\t0.000000E+0\t0.000000E+0\t0.000000E+0\t0.000000E+0\t0.000000E+0\t0.000000E+0\t0.000000E+0\t0.000000E+0\t0.000000E+0\t0.000000E+0\t0.000000E+0\t0.000000E+0\t0.000000E+0\t0.000000E+0\t0.000000E+0\t0.000000E+0\t0.000000E+0\t0.000000E+0\t0.000000E+0\t0.000000E+0\t0.000000E+0\r\n1.901969E+0\t0.000000E+0\t0.000000E+0\t0.000000E+0\t0.000000E+0\t0.000000E+0\t0.000000E+0\t0.000000E+0\t0.000000E+0\t0.000000E+0\t0.000000E+0\t0.000000E+0\t0.000000E+0\t0.000000E+0\t0.000000E+0\t0.000000E+0\t0.000000E+0\t0.000000E+0\t0.000000E+0\t0.000000E+0\t0.000000E+0\t0.000000E+0\t0.000000E+0\t3.909764E-6\t6.212014E-5\t1.689628E-4\t3.507488E-4\t6.430829E-4\t1.091891E-3\t1.753427E-3\t2.692720E-3\t3.979955E-3\t5.684505E-3\t7.866667E-3\t1.056769E-2\t1.379924E-2\t1.753396E-2\t2.169915E-2\t2.617557E-2\t3.080265E-2\t3.539100E-2\t3.974109E-2\t4.366617E-2\t4.701592E-2\t4.969679E-2\t5.168484E-2\t5.302790E-2\t5.383546E-2\t5.425649E-2\t5.444750E-2\t5.453266E-2\t5.453266E-2\t5.444750E-2\t5.425649E-2\t5.383546E-2\t5.302790E-2\t5.168484E-2\t4.969679E-2\t4.701592E-2\t4.366617E-2\t3.974109E-2\t3.539100E-2\t3.080265E-2\t2.617557E-2\t2.169915E-2\t1.753396E-2\t1.379924E-2\t1.056769E-2\t7.866667E-3\t5.684505E-3\t3.979955E-3\t2.692720E-3\t1.753427E-3\t1.091891E-3\t6.430829E-4\t3.507488E-4\t1.689628E-4\t6.212014E-5\t3.909764E-6\t0.000000E+0\t0.000000E+0\t0.000000E+0\t0.000000E+0\t0.000000E+0\t0.000000E+0\t0.000000E+0\t0.000000E+0\t0.000000E+0\t0.000000E+0\t0.000000E+0\t0.000000E+0\t0.000000E+0\t0.000000E+0\t0.000000E+0\t0.000000E+0\t0.000000E+0\t0.000000E+0\t0.000000E+0\t0.000000E+0\t0.000000E+0\t0.000000E+0\r\n1.946927E+0\t0.000000E+0\t0.000000E+0\t0.000000E+0\t0.000000E+0\t0.000000E+0\t0.000000E+0\t0.000000E+0\t0.000000E+0\t0.000000E+0\t0.000000E+0\t0.000000E+0\t0.000000E+0\t0.000000E+0\t0.000000E+0\t0.000000E+0\t0.000000E+0\t0.000000E+0\t0.000000E+0\t0.000000E+0\t0.000000E+0\t0.000000E+0\t0.000000E+0\t2.309373E-5\t7.786561E-5\t1.749146E-4\t3.365039E-4\t5.926041E-4\t9.816766E-4\t1.550583E-3\t2.353169E-3\t3.447118E-3\t4.888859E-3\t6.726593E-3\t8.991969E-3\t1.169139E-2\t1.479835E-2\t1.824853E-2\t2.193916E-2\t2.573400E-2\t2.947413E-2\t3.299399E-2\t3.614066E-2\t3.879363E-2\t4.088133E-2\t4.239144E-2\t4.337188E-2\t4.392167E-2\t4.417184E-2\t4.425844E-2\t4.428958E-2\t4.428958E-2\t4.425844E-2\t4.417184E-2\t4.392167E-2\t4.337188E-2\t4.239144E-2\t4.088133E-2\t3.879363E-2\t3.614066E-2\t3.299399E-2\t2.947413E-2\t2.573400E-2\t2.193916E-2\t1.824853E-2\t1.479835E-2\t1.169139E-2\t8.991969E-3\t6.726593E-3\t4.888859E-3\t3.447118E-3\t2.353169E-3\t1.550583E-3\t9.816766E-4\t5.926041E-4\t3.365039E-4\t1.749146E-4\t7.786561E-5\t2.309373E-5\t0.000000E+0\t0.000000E+0\t0.000000E+0\t0.000000E+0\t0.000000E+0\t0.000000E+0\t0.000000E+0\t0.000000E+0\t0.000000E+0\t0.000000E+0\t0.000000E+0\t0.000000E+0\t0.000000E+0\t0.000000E+0\t0.000000E+0\t0.000000E+0\t0.000000E+0\t0.000000E+0\t0.000000E+0\t0.000000E+0\t0.000000E+0\t0.000000E+0\r\n1.991884E+0\t0.000000E+0\t0.000000E+0\t0.000000E+0\t0.000000E+0\t0.000000E+0\t0.000000E+0\t0.000000E+0\t0.000000E+0\t0.000000E+0\t0.000000E+0\t0.000000E+0\t0.000000E+0\t0.000000E+0\t0.000000E+0\t0.000000E+0\t0.000000E+0\t0.000000E+0\t0.000000E+0\t0.000000E+0\t0.000000E+0\t0.000000E+0\t6.595111E-6\t3.365434E-5\t8.376317E-5\t1.702921E-4\t3.119811E-4\t5.339354E-4\t8.682179E-4\t1.353695E-3\t2.034765E-3\t2.958644E-3\t4.171040E-3\t5.710307E-3\t7.600527E-3\t9.844365E-3\t1.241690E-2\t1.526178E-2\t1.829113E-2\t2.138999E-2\t2.442575E-2\t2.726170E-2\t2.977324E-2\t3.186419E-2\t3.348033E-2\t3.461746E-2\t3.532170E-2\t3.568126E-2\t3.581014E-2\t3.582548E-2\t3.582043E-2\t3.582043E-2\t3.582548E-2\t3.581014E-2\t3.568126E-2\t3.532170E-2\t3.461746E-2\t3.348033E-2\t3.186419E-2\t2.977324E-2\t2.726170E-2\t2.442575E-2\t2.138999E-2\t1.829113E-2\t1.526178E-2\t1.241690E-2\t9.844365E-3\t7.600527E-3\t5.710307E-3\t4.171040E-3\t2.958644E-3\t2.034765E-3\t1.353695E-3\t8.682179E-4\t5.339354E-4\t3.119811E-4\t1.702921E-4\t8.376317E-5\t3.365434E-5\t6.595111E-6\t0.000000E+0\t0.000000E+0\t0.000000E+0\t0.000000E+0\t0.000000E+0\t0.000000E+0\t0.000000E+0\t0.000000E+0\t0.000000E+0\t0.000000E+0\t0.000000E+0\t0.000000E+0\t0.000000E+0\t0.000000E+0\t0.000000E+0\t0.000000E+0\t0.000000E+0\t0.000000E+0\t0.000000E+0\t0.000000E+0\t0.000000E+0\r\n2.036842E+0\t0.000000E+0\t0.000000E+0\t0.000000E+0\t0.000000E+0\t0.000000E+0\t0.000000E+0\t0.000000E+0\t0.000000E+0\t0.000000E+0\t0.000000E+0\t0.000000E+0\t0.000000E+0\t0.000000E+0\t0.000000E+0\t0.000000E+0\t0.000000E+0\t0.000000E+0\t0.000000E+0\t0.000000E+0\t0.000000E+0\t4.814538E-7\t1.333405E-5\t3.833185E-5\t8.319888E-5\t1.591869E-4\t2.819912E-4\t4.725431E-4\t7.574531E-4\t1.168820E-3\t1.743101E-3\t2.518789E-3\t3.532762E-3\t4.815401E-3\t6.384868E-3\t8.241271E-3\t1.036170E-2\t1.269728E-2\t1.517335E-2\t1.769352E-2\t2.014767E-2\t2.242347E-2\t2.441983E-2\t2.606038E-2\t2.730444E-2\t2.815325E-2\t2.864987E-2\t2.887185E-2\t2.891740E-2\t2.888647E-2\t2.885856E-2\t2.885856E-2\t2.888647E-2\t2.891740E-2\t2.887185E-2\t2.864987E-2\t2.815325E-2\t2.730444E-2\t2.606038E-2\t2.441983E-2\t2.242347E-2\t2.014767E-2\t1.769352E-2\t1.517335E-2\t1.269728E-2\t1.036170E-2\t8.241271E-3\t6.384868E-3\t4.815401E-3\t3.532762E-3\t2.518789E-3\t1.743101E-3\t1.168820E-3\t7.574531E-4\t4.725431E-4\t2.819912E-4\t1.591869E-4\t8.319888E-5\t3.833185E-5\t1.333405E-5\t4.814538E-7\t0.000000E+0\t0.000000E+0\t0.000000E+0\t0.000000E+0\t0.000000E+0\t0.000000E+0\t0.000000E+0\t0.000000E+0\t0.000000E+0\t0.000000E+0\t0.000000E+0\t0.000000E+0\t0.000000E+0\t0.000000E+0\t0.000000E+0\t0.000000E+0\t0.000000E+0\t0.000000E+0\t0.000000E+0\t0.000000E+0\r\n2.081800E+0\t0.000000E+0\t0.000000E+0\t0.000000E+0\t0.000000E+0\t0.000000E+0\t0.000000E+0\t0.000000E+0\t0.000000E+0\t0.000000E+0\t0.000000E+0\t0.000000E+0\t0.000000E+0\t0.000000E+0\t0.000000E+0\t0.000000E+0\t0.000000E+0\t0.000000E+0\t0.000000E+0\t0.000000E+0\t0.000000E+0\t4.602087E-6\t1.663488E-5\t3.914860E-5\t7.864096E-5\t1.445318E-4\t2.499032E-4\t4.121274E-4\t6.531940E-4\t9.995018E-4\t1.480869E-3\t2.128554E-3\t2.972192E-3\t4.035743E-3\t5.332781E-3\t6.861743E-3\t8.601960E-3\t1.051141E-2\t1.252711E-2\t1.456865E-2\t1.654508E-2\t1.836451E-2\t1.994531E-2\t2.122710E-2\t2.217964E-2\t2.280767E-2\t2.315041E-2\t2.327524E-2\t2.326597E-2\t2.320719E-2\t2.316615E-2\t2.316615E-2\t2.320719E-2\t2.326597E-2\t2.327524E-2\t2.315041E-2\t2.280767E-2\t2.217964E-2\t2.122710E-2\t1.994531E-2\t1.836451E-2\t1.654508E-2\t1.456865E-2\t1.252711E-2\t1.051141E-2\t8.601960E-3\t6.861743E-3\t5.332781E-3\t4.035743E-3\t2.972192E-3\t2.128554E-3\t1.480869E-3\t9.995018E-4\t6.531940E-4\t4.121274E-4\t2.499032E-4\t1.445318E-4\t7.864096E-5\t3.914860E-5\t1.663488E-5\t4.602087E-6\t0.000000E+0\t0.000000E+0\t0.000000E+0\t0.000000E+0\t0.000000E+0\t0.000000E+0\t0.000000E+0\t0.000000E+0\t0.000000E+0\t0.000000E+0\t0.000000E+0\t0.000000E+0\t0.000000E+0\t0.000000E+0\t0.000000E+0\t0.000000E+0\t0.000000E+0\t0.000000E+0\t0.000000E+0\t0.000000E+0\r\n2.126758E+0\t0.000000E+0\t0.000000E+0\t0.000000E+0\t0.000000E+0\t0.000000E+0\t0.000000E+0\t0.000000E+0\t0.000000E+0\t0.000000E+0\t0.000000E+0\t0.000000E+0\t0.000000E+0\t0.000000E+0\t0.000000E+0\t0.000000E+0\t0.000000E+0\t0.000000E+0\t0.000000E+0\t0.000000E+0\t1.179181E-6\t6.757312E-6\t1.768103E-5\t3.756377E-5\t7.184225E-5\t1.283636E-4\t2.179809E-4\t3.550490E-4\t5.576616E-4\t8.474416E-4\t1.248680E-3\t1.786663E-3\t2.485117E-3\t3.362854E-3\t4.429921E-3\t5.683743E-3\t7.105967E-3\t8.660767E-3\t1.029533E-2\t1.194296E-2\t1.352891E-2\t1.497835E-2\t1.622565E-2\t1.722328E-2\t1.794899E-2\t1.840953E-2\t1.863994E-2\t1.869813E-2\t1.865503E-2\t1.858163E-2\t1.853436E-2\t1.853436E-2\t1.858163E-2\t1.865503E-2\t1.869813E-2\t1.863994E-2\t1.840953E-2\t1.794899E-2\t1.722328E-2\t1.622565E-2\t1.497835E-2\t1.352891E-2\t1.194296E-2\t1.029533E-2\t8.660767E-3\t7.105967E-3\t5.683743E-3\t4.429921E-3\t3.362854E-3\t2.485117E-3\t1.786663E-3\t1.248680E-3\t8.474416E-4\t5.576616E-4\t3.550490E-4\t2.179809E-4\t1.283636E-4\t7.184225E-5\t3.756377E-5\t1.768103E-5\t6.757312E-6\t1.179181E-6\t0.000000E+0\t0.000000E+0\t0.000000E+0\t0.000000E+0\t0.000000E+0\t0.000000E+0\t0.000000E+0\t0.000000E+0\t0.000000E+0\t0.000000E+0\t0.000000E+0\t0.000000E+0\t0.000000E+0\t0.000000E+0\t0.000000E+0\t0.000000E+0\t0.000000E+0\t0.000000E+0\t0.000000E+0\r\n2.171716E+0\t0.000000E+0\t0.000000E+0\t0.000000E+0\t0.000000E+0\t0.000000E+0\t0.000000E+0\t0.000000E+0\t0.000000E+0\t0.000000E+0\t0.000000E+0\t0.000000E+0\t0.000000E+0\t0.000000E+0\t0.000000E+0\t0.000000E+0\t0.000000E+0\t0.000000E+0\t0.000000E+0\t2.255367E-8\t2.506198E-6\t7.625638E-6\t1.731776E-5\t3.460403E-5\t6.401014E-5\t1.120417E-4\t1.876620E-4\t3.026806E-4\t4.719240E-4\t7.130314E-4\t1.045715E-3\t1.490351E-3\t2.065864E-3\t2.786963E-3\t3.661005E-3\t4.684881E-3\t5.842517E-3\t7.103605E-3\t8.424133E-3\t9.749083E-3\t1.101731E-2\t1.216816E-2\t1.314907E-2\t1.392280E-2\t1.447314E-2\t1.480780E-2\t1.495759E-2\t1.497177E-2\t1.490987E-2\t1.483106E-2\t1.478228E-2\t1.478228E-2\t1.483106E-2\t1.490987E-2\t1.497177E-2\t1.495759E-2\t1.480780E-2\t1.447314E-2\t1.392280E-2\t1.314907E-2\t1.216816E-2\t1.101731E-2\t9.749083E-3\t8.424133E-3\t7.103605E-3\t5.842517E-3\t4.684881E-3\t3.661005E-3\t2.786963E-3\t2.065864E-3\t1.490351E-3\t1.045715E-3\t7.130314E-4\t4.719240E-4\t3.026806E-4\t1.876620E-4\t1.120417E-4\t6.401014E-5\t3.460403E-5\t1.731776E-5\t7.625638E-6\t2.506198E-6\t2.255367E-8\t0.000000E+0\t0.000000E+0\t0.000000E+0\t0.000000E+0\t0.000000E+0\t0.000000E+0\t0.000000E+0\t0.000000E+0\t0.000000E+0\t0.000000E+0\t0.000000E+0\t0.000000E+0\t0.000000E+0\t0.000000E+0\t0.000000E+0\t0.000000E+0\t0.000000E+0\t0.000000E+0\r\n2.216673E+0\t0.000000E+0\t0.000000E+0\t0.000000E+0\t0.000000E+0\t0.000000E+0\t0.000000E+0\t0.000000E+0\t0.000000E+0\t0.000000E+0\t0.000000E+0\t0.000000E+0\t0.000000E+0\t0.000000E+0\t0.000000E+0\t0.000000E+0\t0.000000E+0\t0.000000E+0\t0.000000E+0\t8.014110E-7\t3.115328E-6\t7.686784E-6\t1.613433E-5\t3.097102E-5\t5.594552E-5\t9.642616E-5\t1.597825E-4\t2.556887E-4\t3.962436E-4\t5.957794E-4\t8.702300E-4\t1.235956E-3\t1.707993E-3\t2.297797E-3\t3.010690E-3\t3.843367E-3\t4.781920E-3\t5.800896E-3\t6.863838E-3\t7.925594E-3\t8.936387E-3\t9.847275E-3\t1.061632E-2\t1.121446E-2\t1.163004E-2\t1.187099E-2\t1.196400E-2\t1.195061E-2\t1.188038E-2\t1.180227E-2\t1.175508E-2\t1.175508E-2\t1.180227E-2\t1.188038E-2\t1.195061E-2\t1.196400E-2\t1.187099E-2\t1.163004E-2\t1.121446E-2\t1.061632E-2\t9.847275E-3\t8.936387E-3\t7.925594E-3\t6.863838E-3\t5.800896E-3\t4.781920E-3\t3.843367E-3\t3.010690E-3\t2.297797E-3\t1.707993E-3\t1.235956E-3\t8.702300E-4\t5.957794E-4\t3.962436E-4\t2.556887E-4\t1.597825E-4\t9.642616E-5\t5.594552E-5\t3.097102E-5\t1.613433E-5\t7.686784E-6\t3.115328E-6\t8.014110E-7\t0.000000E+0\t0.000000E+0\t0.000000E+0\t0.000000E+0\t0.000000E+0\t0.000000E+0\t0.000000E+0\t0.000000E+0\t0.000000E+0\t0.000000E+0\t0.000000E+0\t0.000000E+0\t0.000000E+0\t0.000000E+0\t0.000000E+0\t0.000000E+0\t0.000000E+0\t0.000000E+0\r\n2.261631E+0\t0.000000E+0\t0.000000E+0\t0.000000E+0\t0.000000E+0\t0.000000E+0\t0.000000E+0\t0.000000E+0\t0.000000E+0\t0.000000E+0\t0.000000E+0\t0.000000E+0\t0.000000E+0\t0.000000E+0\t0.000000E+0\t0.000000E+0\t0.000000E+0\t0.000000E+0\t1.823214E-7\t1.188838E-6\t3.273327E-6\t7.272154E-6\t1.453034E-5\t2.712737E-5\t4.815342E-5\t8.201809E-5\t1.347539E-4\t2.142524E-4\t3.303458E-4\t4.946332E-4\t7.199450E-4\t1.019368E-3\t1.404805E-3\t1.885142E-3\t2.464179E-3\t3.138641E-3\t3.896625E-3\t4.716904E-3\t5.569455E-3\t6.417414E-3\t7.220449E-3\t7.939233E-3\t8.540444E-3\t9.001494E-3\t9.314096E-3\t9.485926E-3\t9.539838E-3\t9.510525E-3\t9.438974E-3\t9.365418E-3\t9.321686E-3\t9.321686E-3\t9.365418E-3\t9.438974E-3\t9.510525E-3\t9.539838E-3\t9.485926E-3\t9.314096E-3\t9.001494E-3\t8.540444E-3\t7.939233E-3\t7.220449E-3\t6.417414E-3\t5.569455E-3\t4.716904E-3\t3.896625E-3\t3.138641E-3\t2.464179E-3\t1.885142E-3\t1.404805E-3\t1.019368E-3\t7.199450E-4\t4.946332E-4\t3.303458E-4\t2.142524E-4\t1.347539E-4\t8.201809E-5\t4.815342E-5\t2.712737E-5\t1.453034E-5\t7.272154E-6\t3.273327E-6\t1.188838E-6\t1.823214E-7\t0.000000E+0\t0.000000E+0\t0.000000E+0\t0.000000E+0\t0.000000E+0\t0.000000E+0\t0.000000E+0\t0.000000E+0\t0.000000E+0\t0.000000E+0\t0.000000E+0\t0.000000E+0\t0.000000E+0\t0.000000E+0\t0.000000E+0\t0.000000E+0\t0.000000E+0\r\n2.306589E+0\t0.000000E+0\t0.000000E+0\t0.000000E+0\t0.000000E+0\t0.000000E+0\t0.000000E+0\t0.000000E+0\t0.000000E+0\t0.000000E+0\t0.000000E+0\t0.000000E+0\t0.000000E+0\t0.000000E+0\t0.000000E+0\t0.000000E+0\t0.000000E+0\t0.000000E+0\t4.123988E-7\t1.330162E-6\t3.162790E-6\t6.604713E-6\t1.276771E-5\t2.336399E-5\t4.092891E-5\t6.906827E-5\t1.126987E-4\t1.782301E-4\t2.736205E-4\t4.082195E-4\t5.923190E-4\t8.363478E-4\t1.149696E-3\t1.539226E-3\t2.007613E-3\t2.551757E-3\t3.161569E-3\t3.819469E-3\t4.500870E-3\t5.175828E-3\t5.811814E-3\t6.377360E-3\t6.846096E-3\t7.200527E-3\t7.434847E-3\t7.556188E-3\t7.583882E-3\t7.546689E-3\t7.478256E-3\t7.411432E-3\t7.372158E-3\t7.372158E-3\t7.411432E-3\t7.478256E-3\t7.546689E-3\t7.583882E-3\t7.556188E-3\t7.434847E-3\t7.200527E-3\t6.846096E-3\t6.377360E-3\t5.811814E-3\t5.175828E-3\t4.500870E-3\t3.819469E-3\t3.161569E-3\t2.551757E-3\t2.007613E-3\t1.539226E-3\t1.149696E-3\t8.363478E-4\t5.923190E-4\t4.082195E-4\t2.736205E-4\t1.782301E-4\t1.126987E-4\t6.906827E-5\t4.092891E-5\t2.336399E-5\t1.276771E-5\t6.604713E-6\t3.162790E-6\t1.330162E-6\t4.123988E-7\t0.000000E+0\t0.000000E+0\t0.000000E+0\t0.000000E+0\t0.000000E+0\t0.000000E+0\t0.000000E+0\t0.000000E+0\t0.000000E+0\t0.000000E+0\t0.000000E+0\t0.000000E+0\t0.000000E+0\t0.000000E+0\t0.000000E+0\t0.000000E+0\t0.000000E+0\r\n2.351547E+0\t0.000000E+0\t0.000000E+0\t0.000000E+0\t0.000000E+0\t0.000000E+0\t0.000000E+0\t0.000000E+0\t0.000000E+0\t0.000000E+0\t0.000000E+0\t0.000000E+0\t0.000000E+0\t0.000000E+0\t0.000000E+0\t0.000000E+0\t0.000000E+0\t1.218928E-7\t5.114020E-7\t1.323944E-6\t2.905600E-6\t5.829757E-6\t1.101070E-5\t1.985139E-5\t3.442237E-5\t5.765897E-5\t9.355095E-5\t1.472830E-4\t2.252695E-4\t3.350171E-4\t4.847496E-4\t6.827471E-4\t9.363903E-4\t1.250958E-3\t1.628301E-3\t2.065580E-3\t2.554323E-3\t3.080061E-3\t3.622774E-3\t4.158257E-3\t4.660395E-3\t5.104116E-3\t5.468630E-3\t5.740435E-3\t5.915530E-3\t6.000339E-3\t6.011052E-3\t5.971324E-3\t5.908594E-3\t5.849514E-3\t5.815092E-3\t5.815092E-3\t5.849514E-3\t5.908594E-3\t5.971324E-3\t6.011052E-3\t6.000339E-3\t5.915530E-3\t5.740435E-3\t5.468630E-3\t5.104116E-3\t4.660395E-3\t4.158257E-3\t3.622774E-3\t3.080061E-3\t2.554323E-3\t2.065580E-3\t1.628301E-3\t1.250958E-3\t9.363903E-4\t6.827471E-4\t4.847496E-4\t3.350171E-4\t2.252695E-4\t1.472830E-4\t9.355095E-5\t5.765897E-5\t3.442237E-5\t1.985139E-5\t1.101070E-5\t5.829757E-6\t2.905600E-6\t1.323944E-6\t5.114020E-7\t1.218928E-7\t0.000000E+0\t0.000000E+0\t0.000000E+0\t0.000000E+0\t0.000000E+0\t0.000000E+0\t0.000000E+0\t0.000000E+0\t0.000000E+0\t0.000000E+0\t0.000000E+0\t0.000000E+0\t0.000000E+0\t0.000000E+0\t0.000000E+0\t0.000000E+0\r\n2.396504E+0\t0.000000E+0\t0.000000E+0\t0.000000E+0\t0.000000E+0\t0.000000E+0\t0.000000E+0\t0.000000E+0\t0.000000E+0\t0.000000E+0\t0.000000E+0\t0.000000E+0\t0.000000E+0\t0.000000E+0\t0.000000E+0\t0.000000E+0\t2.427829E-8\t1.832495E-7\t5.314494E-7\t1.235448E-6\t2.580704E-6\t5.038149E-6\t9.355896E-6\t1.667806E-5\t2.868781E-5\t4.776403E-5\t7.713032E-5\t1.209626E-4\t1.844100E-4\t2.734752E-4\t3.947043E-4\t5.546467E-4\t7.590829E-4\t1.012058E-3\t1.314825E-3\t1.664849E-3\t2.055075E-3\t2.473671E-3\t2.904421E-3\t3.327857E-3\t3.723109E-3\t4.070282E-3\t4.353047E-3\t4.561024E-3\t4.691503E-3\t4.750139E-3\t4.750359E-3\t4.711481E-3\t4.655736E-3\t4.604616E-3\t4.575033E-3\t4.575033E-3\t4.604616E-3\t4.655736E-3\t4.711481E-3\t4.750359E-3\t4.750139E-3\t4.691503E-3\t4.561024E-3\t4.353047E-3\t4.070282E-3\t3.723109E-3\t3.327857E-3\t2.904421E-3\t2.473671E-3\t2.055075E-3\t1.664849E-3\t1.314825E-3\t1.012058E-3\t7.590829E-4\t5.546467E-4\t3.947043E-4\t2.734752E-4\t1.844100E-4\t1.209626E-4\t7.713032E-5\t4.776403E-5\t2.868781E-5\t1.667806E-5\t9.355896E-6\t5.038149E-6\t2.580704E-6\t1.235448E-6\t5.314494E-7\t1.832495E-7\t2.427829E-8\t0.000000E+0\t0.000000E+0\t0.000000E+0\t0.000000E+0\t0.000000E+0\t0.000000E+0\t0.000000E+0\t0.000000E+0\t0.000000E+0\t0.000000E+0\t0.000000E+0\t0.000000E+0\t0.000000E+0\t0.000000E+0\t0.000000E+0\r\n2.441462E+0\t0.000000E+0\t0.000000E+0\t0.000000E+0\t0.000000E+0\t0.000000E+0\t0.000000E+0\t0.000000E+0\t0.000000E+0\t0.000000E+0\t0.000000E+0\t0.000000E+0\t0.000000E+0\t0.000000E+0\t0.000000E+0\t0.000000E+0\t5.940029E-8\t2.034281E-7\t5.067683E-7\t1.106681E-6\t2.237323E-6\t4.283479E-6\t7.854299E-6\t1.387840E-5\t2.371780E-5\t3.929185E-5\t6.319382E-5\t9.877291E-5\t1.501453E-4\t2.220922E-4\t3.198035E-4\t4.484409E-4\t6.125149E-4\t8.151135E-4\t1.057062E-3\t1.336143E-3\t1.646527E-3\t1.978599E-3\t2.319293E-3\t2.653028E-3\t2.963198E-3\t3.234083E-3\t3.452907E-3\t3.611714E-3\t3.708713E-3\t3.748783E-3\t3.742966E-3\t3.706925E-3\t3.658564E-3\t3.615112E-3\t3.590103E-3\t3.590103E-3\t3.615112E-3\t3.658564E-3\t3.706925E-3\t3.742966E-3\t3.748783E-3\t3.708713E-3\t3.611714E-3\t3.452907E-3\t3.234083E-3\t2.963198E-3\t2.653028E-3\t2.319293E-3\t1.978599E-3\t1.646527E-3\t1.336143E-3\t1.057062E-3\t8.151135E-4\t6.125149E-4\t4.484409E-4\t3.198035E-4\t2.220922E-4\t1.501453E-4\t9.877291E-5\t6.319382E-5\t3.929185E-5\t2.371780E-5\t1.387840E-5\t7.854299E-6\t4.283479E-6\t2.237323E-6\t1.106681E-6\t5.067683E-7\t2.034281E-7\t5.940029E-8\t0.000000E+0\t0.000000E+0\t0.000000E+0\t0.000000E+0\t0.000000E+0\t0.000000E+0\t0.000000E+0\t0.000000E+0\t0.000000E+0\t0.000000E+0\t0.000000E+0\t0.000000E+0\t0.000000E+0\t0.000000E+0\t0.000000E+0\r\n2.486420E+0\t0.000000E+0\t0.000000E+0\t0.000000E+0\t0.000000E+0\t0.000000E+0\t0.000000E+0\t0.000000E+0\t0.000000E+0\t0.000000E+0\t0.000000E+0\t0.000000E+0\t0.000000E+0\t0.000000E+0\t0.000000E+0\t1.618312E-8\t7.358022E-8\t2.000106E-7\t4.592474E-7\t9.637455E-7\t1.904552E-6\t3.594481E-6\t6.527124E-6\t1.145265E-5\t1.946818E-5\t3.211539E-5\t5.147137E-5\t8.021084E-5\t1.216107E-4\t1.794635E-4\t2.578682E-4\t3.608773E-4\t4.919977E-4\t6.535774E-4\t8.461418E-4\t1.067781E-3\t1.313719E-3\t1.576184E-3\t1.844704E-3\t2.106869E-3\t2.349526E-3\t2.560304E-3\t2.729244E-3\t2.850269E-3\t2.922229E-3\t2.949267E-3\t2.940387E-3\t2.908209E-3\t2.867060E-3\t2.830677E-3\t2.809830E-3\t2.809830E-3\t2.830677E-3\t2.867060E-3\t2.908209E-3\t2.940387E-3\t2.949267E-3\t2.922229E-3\t2.850269E-3\t2.729244E-3\t2.560304E-3\t2.349526E-3\t2.106869E-3\t1.844704E-3\t1.576184E-3\t1.313719E-3\t1.067781E-3\t8.461418E-4\t6.535774E-4\t4.919977E-4\t3.608773E-4\t2.578682E-4\t1.794635E-4\t1.216107E-4\t8.021084E-5\t5.147137E-5\t3.211539E-5\t1.946818E-5\t1.145265E-5\t6.527124E-6\t3.594481E-6\t1.904552E-6\t9.637455E-7\t4.592474E-7\t2.000106E-7\t7.358022E-8\t1.618312E-8\t0.000000E+0\t0.000000E+0\t0.000000E+0\t0.000000E+0\t0.000000E+0\t0.000000E+0\t0.000000E+0\t0.000000E+0\t0.000000E+0\t0.000000E+0\t0.000000E+0\t0.000000E+0\t0.000000E+0\t0.000000E+0\r\n2.531378E+0\t0.000000E+0\t0.000000E+0\t0.000000E+0\t0.000000E+0\t0.000000E+0\t0.000000E+0\t0.000000E+0\t0.000000E+0\t0.000000E+0\t0.000000E+0\t0.000000E+0\t0.000000E+0\t0.000000E+0\t2.767232E-9\t2.474515E-8\t7.566434E-8\t1.841639E-7\t4.024332E-7\t8.220939E-7\t1.598209E-6\t2.983813E-6\t5.376937E-6\t9.380760E-6\t1.587497E-5\t2.609234E-5\t4.168925E-5\t6.479260E-5\t9.800017E-5\t1.443082E-4\t2.069412E-4\t2.890686E-4\t3.934074E-4\t5.217359E-4\t6.743719E-4\t8.496958E-4\t1.043818E-3\t1.250498E-3\t1.461384E-3\t1.666638E-3\t1.855888E-3\t2.019441E-3\t2.149559E-3\t2.241618E-3\t2.294907E-3\t2.312896E-3\t2.302870E-3\t2.274932E-3\t2.240484E-3\t2.210416E-3\t2.193250E-3\t2.193250E-3\t2.210416E-3\t2.240484E-3\t2.274932E-3\t2.302870E-3\t2.312896E-3\t2.294907E-3\t2.241618E-3\t2.149559E-3\t2.019441E-3\t1.855888E-3\t1.666638E-3\t1.461384E-3\t1.250498E-3\t1.043818E-3\t8.496958E-4\t6.743719E-4\t5.217359E-4\t3.934074E-4\t2.890686E-4\t2.069412E-4\t1.443082E-4\t9.800017E-5\t6.479260E-5\t4.168925E-5\t2.609234E-5\t1.587497E-5\t9.380760E-6\t5.376937E-6\t2.983813E-6\t1.598209E-6\t8.220939E-7\t4.024332E-7\t1.841639E-7\t7.566434E-8\t2.474515E-8\t2.767232E-9\t0.000000E+0\t0.000000E+0\t0.000000E+0\t0.000000E+0\t0.000000E+0\t0.000000E+0\t0.000000E+0\t0.000000E+0\t0.000000E+0\t0.000000E+0\t0.000000E+0\t0.000000E+0\t0.000000E+0\r\n2.576335E+0\t0.000000E+0\t0.000000E+0\t0.000000E+0\t0.000000E+0\t0.000000E+0\t0.000000E+0\t0.000000E+0\t0.000000E+0\t0.000000E+0\t0.000000E+0\t0.000000E+0\t0.000000E+0\t0.000000E+0\t7.487570E-9\t2.727496E-8\t7.123063E-8\t1.627682E-7\t3.443505E-7\t6.902235E-7\t1.325598E-6\t2.454140E-6\t4.395278E-6\t7.631725E-6\t1.286559E-5\t2.107821E-5\t3.358464E-5\t5.206887E-5\t7.858163E-5\t1.154802E-4\t1.652914E-4\t2.304843E-4\t3.131563E-4\t4.146491E-4\t5.351401E-4\t6.732726E-4\t8.259023E-4\t9.880427E-4\t1.153071E-3\t1.313222E-3\t1.460356E-3\t1.586904E-3\t1.686882E-3\t1.756779E-3\t1.796180E-3\t1.807957E-3\t1.797963E-3\t1.774233E-3\t1.745792E-3\t1.721227E-3\t1.707246E-3\t1.707246E-3\t1.721227E-3\t1.745792E-3\t1.774233E-3\t1.797963E-3\t1.807957E-3\t1.796180E-3\t1.756779E-3\t1.686882E-3\t1.586904E-3\t1.460356E-3\t1.313222E-3\t1.153071E-3\t9.880427E-4\t8.259023E-4\t6.732726E-4\t5.351401E-4\t4.146491E-4\t3.131563E-4\t2.304843E-4\t1.652914E-4\t1.154802E-4\t7.858163E-5\t5.206887E-5\t3.358464E-5\t2.107821E-5\t1.286559E-5\t7.631725E-6\t4.395278E-6\t2.454140E-6\t1.325598E-6\t6.902235E-7\t3.443505E-7\t1.627682E-7\t7.123063E-8\t2.727496E-8\t7.487570E-9\t0.000000E+0\t0.000000E+0\t0.000000E+0\t0.000000E+0\t0.000000E+0\t0.000000E+0\t0.000000E+0\t0.000000E+0\t0.000000E+0\t0.000000E+0\t0.000000E+0\t0.000000E+0\t0.000000E+0\r\n2.621293E+0\t0.000000E+0\t0.000000E+0\t0.000000E+0\t0.000000E+0\t0.000000E+0\t0.000000E+0\t0.000000E+0\t0.000000E+0\t0.000000E+0\t0.000000E+0\t0.000000E+0\t0.000000E+0\t1.874093E-9\t9.278256E-9\t2.650076E-8\t6.369853E-8\t1.398975E-7\t2.894538E-7\t5.722146E-7\t1.088771E-6\t2.002246E-6\t3.567753E-6\t6.169782E-6\t1.036613E-5\t1.693444E-5\t2.691414E-5\t4.163276E-5\t6.270229E-5\t9.196975E-5\t1.314069E-4\t1.829305E-4\t2.481531E-4\t3.280832E-4\t4.228060E-4\t5.311975E-4\t6.507325E-4\t7.774496E-4\t9.061209E-4\t1.030649E-3\t1.144671E-3\t1.242305E-3\t1.318935E-3\t1.371908E-3\t1.401002E-3\t1.408568E-3\t1.399274E-3\t1.379478E-3\t1.356279E-3\t1.336416E-3\t1.325140E-3\t1.325140E-3\t1.336416E-3\t1.356279E-3\t1.379478E-3\t1.399274E-3\t1.408568E-3\t1.401002E-3\t1.371908E-3\t1.318935E-3\t1.242305E-3\t1.144671E-3\t1.030649E-3\t9.061209E-4\t7.774496E-4\t6.507325E-4\t5.311975E-4\t4.228060E-4\t3.280832E-4\t2.481531E-4\t1.829305E-4\t1.314069E-4\t9.196975E-5\t6.270229E-5\t4.163276E-5\t2.691414E-5\t1.693444E-5\t1.036613E-5\t6.169782E-6\t3.567753E-6\t2.002246E-6\t1.088771E-6\t5.722146E-7\t2.894538E-7\t1.398975E-7\t6.369853E-8\t2.650076E-8\t9.278256E-9\t1.874093E-9\t0.000000E+0\t0.000000E+0\t0.000000E+0\t0.000000E+0\t0.000000E+0\t0.000000E+0\t0.000000E+0\t0.000000E+0\t0.000000E+0\t0.000000E+0\t0.000000E+0\t0.000000E+0\r\n2.666251E+0\t0.000000E+0\t0.000000E+0\t0.000000E+0\t0.000000E+0\t0.000000E+0\t0.000000E+0\t0.000000E+0\t0.000000E+0\t0.000000E+0\t0.000000E+0\t0.000000E+0\t2.673031E-10\t2.926970E-9\t9.445939E-9\t2.408559E-8\t5.508996E-8\t1.178297E-7\t2.399504E-7\t4.694404E-7\t8.867032E-7\t1.621745E-6\t2.877333E-6\t4.958273E-6\t8.305653E-6\t1.353291E-5\t2.145795E-5\t3.312269E-5\t4.978886E-5\t7.289759E-5\t1.039815E-4\t1.445222E-4\t1.957557E-4\t2.584366E-4\t3.325918E-4\t4.172995E-4\t5.105443E-4\t6.091963E-4\t7.091497E-4\t8.056383E-4\t8.937104E-4\t9.688124E-4\t1.027399E-3\t1.067471E-3\t1.088929E-3\t1.093678E-3\t1.085419E-3\t1.069150E-3\t1.050431E-3\t1.034518E-3\t1.025506E-3\t1.025506E-3\t1.034518E-3\t1.050431E-3\t1.069150E-3\t1.085419E-3\t1.093678E-3\t1.088929E-3\t1.067471E-3\t1.027399E-3\t9.688124E-4\t8.937104E-4\t8.056383E-4\t7.091497E-4\t6.091963E-4\t5.105443E-4\t4.172995E-4\t3.325918E-4\t2.584366E-4\t1.957557E-4\t1.445222E-4\t1.039815E-4\t7.289759E-5\t4.978886E-5\t3.312269E-5\t2.145795E-5\t1.353291E-5\t8.305653E-6\t4.958273E-6\t2.877333E-6\t1.621745E-6\t8.867032E-7\t4.694404E-7\t2.399504E-7\t1.178297E-7\t5.508996E-8\t2.408559E-8\t9.445939E-9\t2.926970E-9\t2.673031E-10\t0.000000E+0\t0.000000E+0\t0.000000E+0\t0.000000E+0\t0.000000E+0\t0.000000E+0\t0.000000E+0\t0.000000E+0\t0.000000E+0\t0.000000E+0\t0.000000E+0\r\n2.711209E+0\t0.000000E+0\t0.000000E+0\t0.000000E+0\t0.000000E+0\t0.000000E+0\t0.000000E+0\t0.000000E+0\t0.000000E+0\t0.000000E+0\t0.000000E+0\t0.000000E+0\t8.258029E-10\t3.205778E-9\t8.782188E-9\t2.101043E-8\t4.654142E-8\t9.772272E-8\t1.966801E-7\t3.816932E-7\t7.167048E-7\t1.304816E-6\t2.306410E-6\t3.961975E-6\t6.618689E-6\t1.075824E-5\t1.702132E-5\t2.622211E-5\t3.934391E-5\t5.750642E-5\t8.189602E-5\t1.136538E-4\t1.537231E-4\t2.026668E-4\t2.604764E-4\t3.264029E-4\t3.988479E-4\t4.753516E-4\t5.527050E-4\t6.271998E-4\t6.949995E-4\t7.525934E-4\t7.972687E-4\t8.275218E-4\t8.433308E-4\t8.462250E-4\t8.391194E-4\t8.259223E-4\t8.109628E-4\t7.983239E-4\t7.911796E-4\t7.911796E-4\t7.983239E-4\t8.109628E-4\t8.259223E-4\t8.391194E-4\t8.462250E-4\t8.433308E-4\t8.275218E-4\t7.972687E-4\t7.525934E-4\t6.949995E-4\t6.271998E-4\t5.527050E-4\t4.753516E-4\t3.988479E-4\t3.264029E-4\t2.604764E-4\t2.026668E-4\t1.537231E-4\t1.136538E-4\t8.189602E-5\t5.750642E-5\t3.934391E-5\t2.622211E-5\t1.702132E-5\t1.075824E-5\t6.618689E-6\t3.961975E-6\t2.306410E-6\t1.304816E-6\t7.167048E-7\t3.816932E-7\t1.966801E-7\t9.772272E-8\t4.654142E-8\t2.101043E-8\t8.782188E-9\t3.205778E-9\t8.258029E-10\t0.000000E+0\t0.000000E+0\t0.000000E+0\t0.000000E+0\t0.000000E+0\t0.000000E+0\t0.000000E+0\t0.000000E+0\t0.000000E+0\t0.000000E+0\t0.000000E+0\r\n2.756167E+0\t0.000000E+0\t0.000000E+0\t0.000000E+0\t0.000000E+0\t0.000000E+0\t0.000000E+0\t0.000000E+0\t0.000000E+0\t0.000000E+0\t0.000000E+0\t1.891343E-10\t1.025285E-9\t3.079292E-9\t7.752341E-9\t1.782853E-8\t3.864207E-8\t8.005697E-8\t1.596868E-7\t3.079085E-7\t5.753171E-7\t1.043273E-6\t1.838017E-6\t3.148392E-6\t5.246379E-6\t8.508469E-6\t1.343429E-5\t2.065723E-5\t3.094027E-5\t4.514972E-5\t6.420015E-5\t8.896688E-5\t1.201673E-4\t1.582195E-4\t2.030955E-4\t2.541920E-4\t3.102487E-4\t3.693424E-4\t4.289776E-4\t4.862822E-4\t5.382967E-4\t5.823254E-4\t6.163001E-4\t6.390943E-4\t6.507296E-4\t6.524238E-4\t6.464590E-4\t6.358745E-4\t6.240248E-4\t6.140652E-4\t6.084450E-4\t6.084450E-4\t6.140652E-4\t6.240248E-4\t6.358745E-4\t6.464590E-4\t6.524238E-4\t6.507296E-4\t6.390943E-4\t6.163001E-4\t5.823254E-4\t5.382967E-4\t4.862822E-4\t4.289776E-4\t3.693424E-4\t3.102487E-4\t2.541920E-4\t2.030955E-4\t1.582195E-4\t1.201673E-4\t8.896688E-5\t6.420015E-5\t4.514972E-5\t3.094027E-5\t2.065723E-5\t1.343429E-5\t8.508469E-6\t5.246379E-6\t3.148392E-6\t1.838017E-6\t1.043273E-6\t5.753171E-7\t3.079085E-7\t1.596868E-7\t8.005697E-8\t3.864207E-8\t1.782853E-8\t7.752341E-9\t3.079292E-9\t1.025285E-9\t1.891343E-10\t0.000000E+0\t0.000000E+0\t0.000000E+0\t0.000000E+0\t0.000000E+0\t0.000000E+0\t0.000000E+0\t0.000000E+0\t0.000000E+0\t0.000000E+0\r\n"
  out "V PDF outputs (rectified and true)":string="Rectified U bin centre value\tRectified PDF (U)\tInferred true U bin centre value\tInferred true PDF (U)\r\n-3.411158E+0\t0.000000E+0\t-3.411158E+0\t2.811894E-6\r\n-3.342246E+0\t0.000000E+0\t-3.342246E+0\t4.586801E-6\r\n-3.273333E+0\t0.000000E+0\t-3.273333E+0\t7.407708E-6\r\n-3.204421E+0\t0.000000E+0\t-3.204421E+0\t1.184461E-5\r\n-3.135509E+0\t0.000000E+0\t-3.135509E+0\t1.875085E-5\r\n-3.066596E+0\t0.000000E+0\t-3.066596E+0\t2.938894E-5\r\n-2.997684E+0\t0.000000E+0\t-2.997684E+0\t4.560475E-5\r\n-2.928772E+0\t0.000000E+0\t-2.928772E+0\t7.006470E-5\r\n-2.859860E+0\t0.000000E+0\t-2.859860E+0\t1.065741E-4\r\n-2.790947E+0\t0.000000E+0\t-2.790947E+0\t1.604969E-4\r\n-2.722035E+0\t8.503054E-12\t-2.722035E+0\t2.393013E-4\r\n-2.653123E+0\t9.523815E-11\t-2.653123E+0\t3.532535E-4\r\n-2.584211E+0\t4.984078E-10\t-2.584211E+0\t5.162865E-4\r\n-2.515298E+0\t2.046187E-9\t-2.515298E+0\t7.470647E-4\r\n-2.446386E+0\t7.086628E-9\t-2.446386E+0\t1.070259E-3\r\n-2.377474E+0\t2.284420E-8\t-2.377474E+0\t1.518037E-3\r\n-2.308561E+0\t6.703293E-8\t-2.308561E+0\t2.131762E-3\r\n-2.239649E+0\t1.904475E-7\t-2.239649E+0\t2.963865E-3\r\n-2.170737E+0\t5.042624E-7\t-2.170737E+0\t4.079820E-3\r\n-2.101825E+0\t1.306307E-6\t-2.101825E+0\t5.560153E-3\r\n-2.032912E+0\t3.200365E-6\t-2.032912E+0\t7.502318E-3\r\n-1.964000E+0\t7.647539E-6\t-1.964000E+0\t1.002230E-2\r\n-1.895088E+0\t1.748317E-5\t-1.895088E+0\t1.325568E-2\r\n-1.826175E+0\t3.884494E-5\t-1.826175E+0\t1.735801E-2\r\n-1.757263E+0\t8.319203E-5\t-1.757263E+0\t2.250406E-2\r\n-1.688351E+0\t1.726089E-4\t-1.688351E+0\t2.888582E-2\r\n-1.619439E+0\t3.469934E-4\t-1.619439E+0\t3.670893E-2\r\n-1.550526E+0\t6.741077E-4\t-1.550526E+0\t4.618721E-2\r\n-1.481614E+0\t1.273496E-3\t-1.481614E+0\t5.753536E-2\r\n-1.412702E+0\t2.320915E-3\t-1.412702E+0\t7.095956E-2\r\n-1.343789E+0\t4.123843E-3\t-1.343789E+0\t8.664631E-2\r\n-1.274877E+0\t7.061583E-3\t-1.274877E+0\t1.047496E-1\r\n-1.205965E+0\t1.181055E-2\t-1.205965E+0\t1.253769E-1\r\n-1.137053E+0\t1.903846E-2\t-1.137053E+0\t1.485750E-1\r\n-1.068140E+0\t2.998935E-2\t-1.068140E+0\t1.743159E-1\r\n-9.992281E-1\t4.562922E-2\t-9.992281E-1\t2.024843E-1\r\n-9.303158E-1\t6.770698E-2\t-9.303158E-1\t2.328675E-1\r\n-8.614035E-1\t9.736192E-2\t-8.614035E-1\t2.651486E-1\r\n-7.924912E-1\t1.364082E-1\t-7.924912E-1\t2.989047E-1\r\n-7.235789E-1\t1.857406E-1\t-7.235789E-1\t3.336102E-1\r\n-6.546667E-1\t2.464213E-1\t-6.546667E-1\t3.686455E-1\r\n-5.857544E-1\t3.186102E-1\t-5.857544E-1\t4.033124E-1\r\n-5.168421E-1\t4.017743E-1\t-5.168421E-1\t4.368549E-1\r\n-4.479298E-1\t4.951742E-1\t-4.479298E-1\t4.684852E-1\r\n-3.790175E-1\t5.963527E-1\t-3.790175E-1\t4.974136E-1\r\n-3.101053E-1\t7.040418E-1\t-3.101053E-1\t5.228805E-1\r\n-2.411930E-1\t8.140450E-1\t-2.411930E-1\t5.441896E-1\r\n-1.722807E-1\t9.246448E-1\t-1.722807E-1\t5.607395E-1\r\n-1.033684E-1\t1.028490E+0\t-1.033684E-1\t5.720514E-1\r\n-3.445614E-2\t1.116235E+0\t-3.445614E-2\t5.777926E-1\r\n3.445614E-2\t1.116235E+0\t3.445614E-2\t5.777926E-1\r\n1.033684E-1\t1.028490E+0\t1.033684E-1\t5.720514E-1\r\n1.722807E-1\t9.246448E-1\t1.722807E-1\t5.607395E-1\r\n2.411930E-1\t8.140450E-1\t2.411930E-1\t5.441896E-1\r\n3.101053E-1\t7.040418E-1\t3.101053E-1\t5.228805E-1\r\n3.790175E-1\t5.963527E-1\t3.790175E-1\t4.974136E-1\r\n4.479298E-1\t4.951742E-1\t4.479298E-1\t4.684852E-1\r\n5.168421E-1\t4.017743E-1\t5.168421E-1\t4.368549E-1\r\n5.857544E-1\t3.186102E-1\t5.857544E-1\t4.033124E-1\r\n6.546667E-1\t2.464213E-1\t6.546667E-1\t3.686455E-1\r\n7.235789E-1\t1.857406E-1\t7.235789E-1\t3.336102E-1\r\n7.924912E-1\t1.364082E-1\t7.924912E-1\t2.989047E-1\r\n8.614035E-1\t9.736192E-2\t8.614035E-1\t2.651486E-1\r\n9.303158E-1\t6.770698E-2\t9.303158E-1\t2.328675E-1\r\n9.992281E-1\t4.562922E-2\t9.992281E-1\t2.024843E-1\r\n1.068140E+0\t2.998935E-2\t1.068140E+0\t1.743159E-1\r\n1.137053E+0\t1.903846E-2\t1.137053E+0\t1.485750E-1\r\n1.205965E+0\t1.181055E-2\t1.205965E+0\t1.253769E-1\r\n1.274877E+0\t7.061583E-3\t1.274877E+0\t1.047496E-1\r\n1.343789E+0\t4.123843E-3\t1.343789E+0\t8.664631E-2\r\n1.412702E+0\t2.320915E-3\t1.412702E+0\t7.095956E-2\r\n1.481614E+0\t1.273496E-3\t1.481614E+0\t5.753536E-2\r\n1.550526E+0\t6.741077E-4\t1.550526E+0\t4.618721E-2\r\n1.619439E+0\t3.469934E-4\t1.619439E+0\t3.670893E-2\r\n1.688351E+0\t1.726089E-4\t1.688351E+0\t2.888582E-2\r\n1.757263E+0\t8.319203E-5\t1.757263E+0\t2.250406E-2\r\n1.826175E+0\t3.884494E-5\t1.826175E+0\t1.735801E-2\r\n1.895088E+0\t1.748317E-5\t1.895088E+0\t1.325568E-2\r\n1.964000E+0\t7.647539E-6\t1.964000E+0\t1.002230E-2\r\n2.032912E+0\t3.200365E-6\t2.032912E+0\t7.502318E-3\r\n2.101825E+0\t1.306307E-6\t2.101825E+0\t5.560153E-3\r\n2.170737E+0\t5.042624E-7\t2.170737E+0\t4.079820E-3\r\n2.239649E+0\t1.904475E-7\t2.239649E+0\t2.963865E-3\r\n2.308561E+0\t6.703293E-8\t2.308561E+0\t2.131762E-3\r\n2.377474E+0\t2.284420E-8\t2.377474E+0\t1.518037E-3\r\n2.446386E+0\t7.086628E-9\t2.446386E+0\t1.070259E-3\r\n2.515298E+0\t2.046187E-9\t2.515298E+0\t7.470647E-4\r\n2.584211E+0\t4.984078E-10\t2.584211E+0\t5.162865E-4\r\n2.653123E+0\t9.523815E-11\t2.653123E+0\t3.532535E-4\r\n2.722035E+0\t8.503054E-12\t2.722035E+0\t2.393013E-4\r\n2.790947E+0\t0.000000E+0\t2.790947E+0\t1.604969E-4\r\n2.859860E+0\t0.000000E+0\t2.859860E+0\t1.065741E-4\r\n2.928772E+0\t0.000000E+0\t2.928772E+0\t7.006470E-5\r\n2.997684E+0\t0.000000E+0\t2.997684E+0\t4.560475E-5\r\n3.066596E+0\t0.000000E+0\t3.066596E+0\t2.938894E-5\r\n3.135509E+0\t0.000000E+0\t3.135509E+0\t1.875085E-5\r\n3.204421E+0\t0.000000E+0\t3.204421E+0\t1.184461E-5\r\n3.273333E+0\t0.000000E+0\t3.273333E+0\t7.407708E-6\r\n3.342246E+0\t0.000000E+0\t3.342246E+0\t4.586801E-6\r\n3.411158E+0\t0.000000E+0\t3.411158E+0\t2.811894E-6\r\n"
  out "U PDF outputs (rectified and true)":string="Rectified U bin centre value\tRectified PDF (U)\tInferred true U bin centre value\tInferred true PDF (U)\r\n-1.694652E+0\t0.000000E+0\t-1.694652E+0\t3.982327E-6\r\n-1.649695E+0\t0.000000E+0\t-1.649695E+0\t6.516630E-6\r\n-1.604737E+0\t0.000000E+0\t-1.604737E+0\t1.055712E-5\r\n-1.559779E+0\t0.000000E+0\t-1.559779E+0\t1.693182E-5\r\n-1.514821E+0\t0.000000E+0\t-1.514821E+0\t2.688425E-5\r\n-1.469864E+0\t0.000000E+0\t-1.469864E+0\t4.225990E-5\r\n-1.424906E+0\t0.000000E+0\t-1.424906E+0\t6.576502E-5\r\n-1.379948E+0\t0.000000E+0\t-1.379948E+0\t1.013206E-4\r\n-1.334990E+0\t0.000000E+0\t-1.334990E+0\t1.545383E-4\r\n-1.290033E+0\t0.000000E+0\t-1.290033E+0\t2.333517E-4\r\n-1.245075E+0\t0.000000E+0\t-1.245075E+0\t3.488364E-4\r\n-1.200117E+0\t0.000000E+0\t-1.200117E+0\t5.162602E-4\r\n-1.155159E+0\t0.000000E+0\t-1.155159E+0\t7.564002E-4\r\n-1.110201E+0\t0.000000E+0\t-1.110201E+0\t1.097162E-3\r\n-1.065244E+0\t0.000000E+0\t-1.065244E+0\t1.575527E-3\r\n-1.020286E+0\t0.000000E+0\t-1.020286E+0\t2.239840E-3\r\n-9.753281E-1\t0.000000E+0\t-9.753281E-1\t3.152421E-3\r\n-9.303704E-1\t0.000000E+0\t-9.303704E-1\t4.392457E-3\r\n-8.854126E-1\t0.000000E+0\t-8.854126E-1\t6.059083E-3\r\n-8.404548E-1\t0.000000E+0\t-8.404548E-1\t8.274511E-3\r\n-7.954971E-1\t0.000000E+0\t-7.954971E-1\t1.118701E-2\r\n-7.505393E-1\t0.000000E+0\t-7.505393E-1\t1.497344E-2\r\n-7.055815E-1\t0.000000E+0\t-7.055815E-1\t1.984107E-2\r\n-6.606238E-1\t0.000000E+0\t-6.606238E-1\t2.602825E-2\r\n-6.156660E-1\t0.000000E+0\t-6.156660E-1\t3.380343E-2\r\n-5.707082E-1\t0.000000E+0\t-5.707082E-1\t4.346229E-2\r\n-5.257505E-1\t0.000000E+0\t-5.257505E-1\t5.532234E-2\r\n-4.807927E-1\t0.000000E+0\t-4.807927E-1\t6.971474E-2\r\n-4.358349E-1\t0.000000E+0\t-4.358349E-1\t8.697305E-2\r\n-3.908772E-1\t0.000000E+0\t-3.908772E-1\t1.074189E-1\r\n-3.459194E-1\t0.000000E+0\t-3.459194E-1\t1.313449E-1\r\n-3.009616E-1\t0.000000E+0\t-3.009616E-1\t1.589943E-1\r\n-2.560039E-1\t0.000000E+0\t-2.560039E-1\t1.905399E-1\r\n-2.110461E-1\t0.000000E+0\t-2.110461E-1\t2.260613E-1\r\n-1.660883E-1\t0.000000E+0\t-1.660883E-1\t2.655234E-1\r\n-1.211306E-1\t0.000000E+0\t-1.211306E-1\t3.087560E-1\r\n-7.617280E-2\t0.000000E+0\t-7.617280E-2\t3.554382E-1\r\n-3.121503E-2\t0.000000E+0\t-3.121503E-2\t4.050875E-1\r\n1.374274E-2\t0.000000E+0\t1.374274E-2\t4.570563E-1\r\n5.870050E-2\t8.538010E-3\t5.870050E-2\t5.105363E-1\r\n1.036583E-1\t2.384036E-2\t1.036583E-1\t5.645723E-1\r\n1.486160E-1\t5.421473E-2\t1.486160E-1\t6.180856E-1\r\n1.935738E-1\t9.118579E-2\t1.935738E-1\t6.699058E-1\r\n2.385316E-1\t1.352868E-1\t2.385316E-1\t7.188113E-1\r\n2.834893E-1\t1.924613E-1\t2.834893E-1\t7.635758E-1\r\n3.284471E-1\t2.544530E-1\t3.284471E-1\t8.030184E-1\r\n3.734049E-1\t3.222235E-1\t3.734049E-1\t8.360551E-1\r\n4.183626E-1\t3.985202E-1\t4.183626E-1\t8.617482E-1\r\n4.633204E-1\t4.756754E-1\t4.633204E-1\t8.793503E-1\r\n5.082782E-1\t5.546628E-1\t5.082782E-1\t8.883407E-1\r\n5.532359E-1\t6.351569E-1\t5.532359E-1\t8.884505E-1\r\n5.981937E-1\t7.106684E-1\t5.981937E-1\t8.796765E-1\r\n6.431515E-1\t7.822129E-1\t6.431515E-1\t8.622810E-1\r\n6.881092E-1\t8.475527E-1\t6.881092E-1\t8.367789E-1\r\n7.330670E-1\t9.022300E-1\t7.330670E-1\t8.039123E-1\r\n7.780248E-1\t9.476279E-1\t7.780248E-1\t7.646149E-1\r\n8.229825E-1\t9.812972E-1\t8.229825E-1\t7.199674E-1\r\n8.679403E-1\t1.001301E+0\t8.679403E-1\t6.711492E-1\r\n9.128981E-1\t1.009647E+0\t9.128981E-1\t6.193859E-1\r\n9.578558E-1\t1.004968E+0\t9.578558E-1\t5.658999E-1\r\n1.002814E+0\t9.875701E-1\t1.002814E+0\t5.118634E-1\r\n1.047771E+0\t9.599642E-1\t1.047771E+0\t4.583577E-1\r\n1.092729E+0\t9.221749E-1\t1.092729E+0\t4.063414E-1\r\n1.137687E+0\t8.758322E-1\t1.137687E+0\t3.566266E-1\r\n1.182645E+0\t8.234752E-1\t1.182645E+0\t3.098649E-1\r\n1.227602E+0\t7.660006E-1\t1.227602E+0\t2.665429E-1\r\n1.272560E+0\t7.053368E-1\t1.272560E+0\t2.269854E-1\r\n1.317518E+0\t6.434013E-1\t1.317518E+0\t1.913661E-1\r\n1.362476E+0\t5.813197E-1\t1.362476E+0\t1.597232E-1\r\n1.407434E+0\t5.204972E-1\t1.407434E+0\t1.319796E-1\r\n1.452391E+0\t4.620614E-1\t1.452391E+0\t1.079648E-1\r\n1.497349E+0\t4.067379E-1\t1.497349E+0\t8.743660E-2\r\n1.542307E+0\t3.551924E-1\t1.542307E+0\t7.010363E-2\r\n1.587265E+0\t3.078296E-1\t1.587265E+0\t5.564471E-2\r\n1.632222E+0\t2.648338E-1\t1.632222E+0\t4.372636E-2\r\n1.677180E+0\t2.262751E-1\t1.677180E+0\t3.401722E-2\r\n1.722138E+0\t1.920663E-1\t1.722138E+0\t2.619934E-2\r\n1.767096E+0\t1.620168E-1\t1.767096E+0\t1.997643E-2\r\n1.812053E+0\t1.358720E-1\t1.812053E+0\t1.507932E-2\r\n1.857011E+0\t1.133192E-1\t1.857011E+0\t1.126890E-2\r\n1.901969E+0\t9.402007E-2\t1.901969E+0\t8.337143E-3\r\n1.946927E+0\t7.762899E-2\t1.946927E+0\t6.106455E-3\r\n1.991884E+0\t6.380220E-2\t1.991884E+0\t4.427893E-3\r\n2.036842E+0\t5.221216E-2\t2.036842E+0\t3.178639E-3\r\n2.081800E+0\t4.255382E-2\t2.081800E+0\t2.259027E-3\r\n2.126758E+0\t3.454811E-2\t2.126758E+0\t1.589416E-3\r\n2.171716E+0\t2.794508E-2\t2.171716E+0\t1.107108E-3\r\n2.216673E+0\t2.252394E-2\t2.216673E+0\t7.634457E-4\r\n2.261631E+0\t1.809199E-2\t2.261631E+0\t5.211978E-4\r\n2.306589E+0\t1.448320E-2\t2.306589E+0\t3.522598E-4\r\n2.351547E+0\t1.155575E-2\t2.351547E+0\t2.357000E-4\r\n2.396504E+0\t9.189532E-3\t2.396504E+0\t1.561321E-4\r\n2.441462E+0\t7.283606E-3\t2.441462E+0\t1.023908E-4\r\n2.486420E+0\t5.753659E-3\t2.486420E+0\t6.647614E-5\r\n2.531378E+0\t4.529663E-3\t2.531378E+0\t4.272741E-5\r\n2.576335E+0\t3.553740E-3\t2.576335E+0\t2.718839E-5\r\n2.621293E+0\t2.778262E-3\t2.621293E+0\t1.712760E-5\r\n2.666251E+0\t2.164191E-3\t2.666251E+0\t1.068183E-5\r\n2.711209E+0\t1.679652E-3\t2.711209E+0\t6.595242E-6\r\n2.756167E+0\t1.298705E-3\t2.756167E+0\t4.031363E-6\r\n"
  out "1D marginal pdf(V), rectified and true":T2(graph)=[{"V bin centre vals"=[-3.4111578892427943, -3.342245608652031, -3.273333328061268, -3.204421047470505, -3.1355087668797417, -3.0665964862889785, -2.9976842056982154, -2.928771925107452, -2.859859644516689, -2.790947363925926, -2.7220350833351628, -2.6531228027443996, -2.5842105221536364, -2.5152982415628733, -2.44638596097211, -2.377473680381347, -2.308561399790584, -2.2396491191998207, -2.1707368386090575, -2.1018245580182944, -2.0329122774275312, -1.9639999968367678, -1.8950877162460047, -1.8261754356552415, -1.7572631550644782, -1.688350874473715, -1.6194385938829519, -1.5505263132921887, -1.4816140327014256, -1.4127017521106624, -1.3437894715198992, -1.274877190929136, -1.205964910338373, -1.1370526297476098, -1.0681403491568466, -0.9992280685660835, -0.9303157879753203, -0.8614035073845572, -0.792491226793794, -0.7235789462030309, -0.6546666656122677, -0.5857543850215046, -0.5168421044307414, -0.44792982383997826, -0.3790175432492151, -0.31010526265845195, -0.2411929820676888, -0.17228070147692565, -0.10336842088616205, -0.034456140295398896, 0.03445614029536426, 0.10336842088612741, 0.17228070147689056, 0.24119298206765372, 0.31010526265841687, 0.37901754324918, 0.4479298238399432, 0.5168421044307063, 0.585754385021469, 0.6546666656122322, 0.7235789462029953, 0.7924912267937585, 0.8614035073845216, 0.9303157879752848, 0.9992280685660488, 1.068140349156812, 1.1370526297475751, 1.2059649103383383, 1.2748771909291015, 1.3437894715198646, 1.4127017521106278, 1.481614032701391, 1.550526313292154, 1.6194385938829172, 1.6883508744736804, 1.7572631550644435, 1.8261754356552067, 1.8950877162459698, 1.963999996836733, 2.032912277427496, 2.1018245580182593, 2.1707368386090224, 2.2396491191997856, 2.3085613997905488, 2.377473680381312, 2.446385960972075, 2.515298241562838, 2.5842105221536014, 2.6531228027443645, 2.7220350833351277, 2.790947363925891, 2.859859644516654, 2.928771925107417, 2.9976842056981803, 3.0665964862889434, 3.1355087668797066, 3.2044210474704697, 3.273333328061233, 3.342245608651996, 3.411157889242759], "1D marginal PDF (V)"=[0.0, 0.0, 0.0, 0.0, 0.0, 0.0, 0.0, 0.0, 0.0, 0.0, 8.503053933180236e-12, 9.52381507051715e-11, 4.984078102465518e-10, 2.046186520316511e-09, 7.08662791196724e-09, 2.2844199456873713e-08, 6.703293146820771e-08, 1.9044749430451872e-07, 5.042623742357638e-07, 1.306306681679308e-06, 3.2003654963443685e-06, 7.647539222323066e-06, 1.748317124407695e-05, 3.884493859571644e-05, 8.319202658366711e-05, 0.00017260892448543776, 0.0003469934194782895, 0.0006741076748014726, 0.0012734956757999977, 0.0023209145160831683, 0.0041238427676304305, 0.007061582677977399, 0.011810554171689807, 0.019038458634381188, 0.029989347712094105, 0.045629223822258924, 0.06770697985471975, 0.09736191998145327, 0.1364081770934655, 0.1857406221499708, 0.24642130416766514, 0.3186101659259761, 0.4017742815643665, 0.49517424246406033, 0.5963527420678829, 0.7040417560395794, 0.8140450016334541, 0.9246447800823607, 1.0284901212343094, 1.1162351334239125, 1.1162351334239402, 1.0284901212343907, 0.9246447800822718, 0.8140450016335102, 0.7040417560397567, 0.5963527420678515, 0.49517424246409275, 0.4017742815644499, 0.3186101659259486, 0.24642130416777494, 0.18574062215001078, 0.1364081770935296, 0.0973619199814515, 0.06770697985474117, 0.04562922382226179, 0.02998934771209714, 0.019038458634410726, 0.011810554171694722, 0.00706158267797848, 0.004123842767632763, 0.002320914516084419, 0.001273495675800934, 0.0006741076748018627, 0.00034699341947856015, 0.00017260892448560123, 8.319202658376202e-05, 3.8844938595764834e-05, 1.7483171244103792e-05, 7.647539222333403e-06, 3.200365496350313e-06, 1.306306681681191e-06, 5.042623742387546e-07, 1.904474943048864e-07, 6.703293146830954e-08, 2.284419945691668e-08, 7.086627911979661e-09, 2.046186520322113e-09, 4.984078102476285e-10, 9.523815070549635e-11, 8.503053933219302e-12, 0.0, 0.0, 0.0, 0.0, 0.0, 0.0, 0.0, 0.0, 0.0, 0.0]}, {"V bin centre vals"=[-3.4111578892427943, -3.342245608652031, -3.273333328061268, -3.204421047470505, -3.1355087668797417, -3.0665964862889785, -2.9976842056982154, -2.928771925107452, -2.859859644516689, -2.790947363925926, -2.7220350833351628, -2.6531228027443996, -2.5842105221536364, -2.5152982415628733, -2.44638596097211, -2.377473680381347, -2.308561399790584, -2.2396491191998207, -2.1707368386090575, -2.1018245580182944, -2.0329122774275312, -1.9639999968367678, -1.8950877162460047, -1.8261754356552415, -1.7572631550644782, -1.688350874473715, -1.6194385938829519, -1.5505263132921887, -1.4816140327014256, -1.4127017521106624, -1.3437894715198992, -1.274877190929136, -1.205964910338373, -1.1370526297476098, -1.0681403491568466, -0.9992280685660835, -0.9303157879753203, -0.8614035073845572, -0.792491226793794, -0.7235789462030309, -0.6546666656122677, -0.5857543850215046, -0.5168421044307414, -0.44792982383997826, -0.3790175432492151, -0.31010526265845195, -0.2411929820676888, -0.17228070147692565, -0.10336842088616205, -0.034456140295398896, 0.03445614029536426, 0.10336842088612741, 0.17228070147689056, 0.24119298206765372, 0.31010526265841687, 0.37901754324918, 0.4479298238399432, 0.5168421044307063, 0.585754385021469, 0.6546666656122322, 0.7235789462029953, 0.7924912267937585, 0.8614035073845216, 0.9303157879752848, 0.9992280685660488, 1.068140349156812, 1.1370526297475751, 1.2059649103383383, 1.2748771909291015, 1.3437894715198646, 1.4127017521106278, 1.481614032701391, 1.550526313292154, 1.6194385938829172, 1.6883508744736804, 1.7572631550644435, 1.8261754356552067, 1.8950877162459698, 1.963999996836733, 2.032912277427496, 2.1018245580182593, 2.1707368386090224, 2.2396491191997856, 2.3085613997905488, 2.377473680381312, 2.446385960972075, 2.515298241562838, 2.5842105221536014, 2.6531228027443645, 2.7220350833351277, 2.790947363925891, 2.859859644516654, 2.928771925107417, 2.9976842056981803, 3.0665964862889434, 3.1355087668797066, 3.2044210474704697, 3.273333328061233, 3.342245608651996, 3.411157889242759], "1D marginal PDF (V)"=[2.81189396978154e-06, 4.586800625348959e-06, 7.407707544315141e-06, 1.1844611909083613e-05, 1.8750846794800077e-05, 2.9388943749697854e-05, 4.560475346051604e-05, 7.006470362934354e-05, 0.0001065740594930053, 0.0001604969451323039, 0.0002393013092784852, 0.0003532534576023598, 0.0005162865490028934, 0.0007470647446849687, 0.0010702585735987305, 0.0015180365621668879, 0.0021317623630035974, 0.002963864816150588, 0.004079820301102679, 0.005560152719709515, 0.007502317654371706, 0.010022295862314116, 0.013255680631405491, 0.01735800812993159, 0.02250405523855946, 0.02888582164078427, 0.036708928483932646, 0.046187210410684486, 0.057535355396597695, 0.0709595593295445, 0.08664630794946311, 0.10474957182089699, 0.12537689012269432, 0.14857501151405536, 0.1743159368239605, 0.20248434817765673, 0.2328674914675413, 0.2651485849413528, 0.29890474197479927, 0.33361021387866807, 0.3686454811278907, 0.40331236132127496, 0.4368548825033163, 0.4684852233367612, 0.49741358568557675, 0.5228804820016852, 0.5441896295116538, 0.5607394794016823, 0.5720513953940095, 0.577792641954299, 0.5777926419542986, 0.5720513953940084, 0.5607394794016807, 0.5441896295116516, 0.5228804820016825, 0.49741358568557353, 0.4684852233367575, 0.4368548825033124, 0.40331236132127113, 0.36864548112788675, 0.33361021387866413, 0.2989047419747954, 0.265148584941349, 0.23286749146753774, 0.20248434817765304, 0.17431593682395716, 0.1485750115140524, 0.12537689012269163, 0.10474957182089462, 0.08664630794946104, 0.0709595593295427, 0.05753535539659619, 0.046187210410683216, 0.036708928483931584, 0.0288858216407834, 0.02250405523855876, 0.017358008129931046, 0.013255680631405056, 0.010022295862313776, 0.007502317654371435, 0.0055601527197093065, 0.004079820301102521, 0.0029638648161504706, 0.0021317623630035098, 0.0015180365621668237, 0.001070258573598684, 0.0007470647446849354, 0.0005162865490028697, 0.0003532534576023432, 0.0002393013092784736, 0.00016049694513229593, 0.00010657405949299988, 7.00647036293399e-05, 4.560475346051361e-05, 2.9388943749696258e-05, 1.8750846794799034e-05, 1.1844611909082937e-05, 7.4077075443147105e-06, 4.586800625348688e-06, 2.8118939697813694e-06]}]
  out "1D marginal pdf(U) - rectified and true":T3(graph)=[{"U bin centre vals"=[-1.6946524176067983, -1.649694650389296, -1.6047368831717936, -1.5597791159542913, -1.5148213487367892, -1.4698635815192869, -1.4249058143017845, -1.3799480470842824, -1.3349902798667799, -1.2900325126492778, -1.2450747454317754, -1.200116978214273, -1.155159210996771, -1.1102014437792687, -1.0652436765617663, -1.0202859093442642, -0.9753281421267618, -0.9303703749092596, -0.8854126076917572, -0.840454840474255, -0.7954970732567527, -0.7505393060392505, -0.7055815388217481, -0.6606237716042458, -0.6156660043867437, -0.5707082371692414, -0.525750469951739, -0.4807927027342367, -0.4358349355167346, -0.39087716829923225, -0.3459194010817299, -0.3009616338642276, -0.2560038666467255, -0.21104609942922314, -0.1660883322117208, -0.12113056499421848, -0.07617279777671637, -0.03121503055921404, 0.01374273665828829, 0.05870050387579062, 0.10365827109329273, 0.14861603831079506, 0.1935738055282974, 0.23853157274579972, 0.28348933996330206, 0.32844710718080417, 0.3734048743983063, 0.41836264161580883, 0.46332040883331094, 0.5082781760508135, 0.5532359432683156, 0.5981937104858177, 0.6431514777033203, 0.6881092449208224, 0.7330670121383245, 0.778024779355827, 0.8229825465733291, 0.8679403137908317, 0.9128980810083338, 0.9578558482258359, 1.0028136154433385, 1.0477713826608406, 1.0927291498783427, 1.1376869170958452, 1.1826446843133473, 1.22760245153085, 1.272560218748352, 1.3175179859658541, 1.3624757531833567, 1.4074335204008588, 1.452391287618361, 1.4973490548358634, 1.5423068220533656, 1.587264589270868, 1.6322223564883702, 1.6771801237058723, 1.7221378909233749, 1.767095658140877, 1.812053425358379, 1.8570111925758817, 1.9019689597933838, 1.9469267270108863, 1.9918844942283884, 2.0368422614458908, 2.081800028663393, 2.126757795880895, 2.171715563098397, 2.2166733303159, 2.261631097533402, 2.3065888647509043, 2.3515466319684064, 2.3965043991859085, 2.4414621664034106, 2.4864199336209136, 2.5313777008384157, 2.576335468055918, 2.62129323527342, 2.666251002490922, 2.711208769708424, 2.756166536925927], "1D marginal PDF (U)"=[0.0, 0.0, 0.0, 0.0, 0.0, 0.0, 0.0, 0.0, 0.0, 0.0, 0.0, 0.0, 0.0, 0.0, 0.0, 0.0, 0.0, 0.0, 0.0, 0.0, 0.0, 0.0, 0.0, 0.0, 0.0, 0.0, 0.0, 0.0, 0.0, 0.0, 0.0, 0.0, 0.0, 0.0, 0.0, 0.0, 0.0, 0.0, 0.0, 0.008538009530284676, 0.02384035514851284, 0.05421473202404496, 0.09118579399856334, 0.13528676580801752, 0.19246133162901144, 0.2544529563171784, 0.3222235413793284, 0.3985201806585478, 0.47567539784059704, 0.554662755114583, 0.6351568798413706, 0.7106684190615463, 0.7822129408505022, 0.8475526642479021, 0.902230036097575, 0.9476279440728921, 0.9812972093349259, 1.0013012850277356, 1.0096471848163455, 1.004968048961473, 0.9875700917640116, 0.9599642208179062, 0.9221748830525375, 0.8758322304119589, 0.8234752379386798, 0.7660005761977592, 0.7053367602828937, 0.6434012856664872, 0.5813196517012948, 0.5204971897680115, 0.4620614387084376, 0.40673788880472145, 0.3551923714835494, 0.30782963912905437, 0.26483382442060127, 0.22627509711015714, 0.1920663446557563, 0.1620167741430313, 0.13587204079065926, 0.11331919968559562, 0.09402006686247412, 0.07762898885235822, 0.0638021968250603, 0.05221215687633605, 0.04255382409540433, 0.034548114935753126, 0.02794508467841214, 0.022523935593024784, 0.01809199454289562, 0.014483204790363123, 0.011555751305327005, 0.009189532152102182, 0.007283605611983019, 0.005753659240383096, 0.004529663445559322, 0.003553740089672613, 0.0027782615251085835, 0.0021641912770618416, 0.0016796524290702075, 0.0012987054480042204]}, {"U bin centre vals"=[-1.6946524176067983, -1.649694650389296, -1.6047368831717936, -1.5597791159542913, -1.5148213487367892, -1.4698635815192869, -1.4249058143017845, -1.3799480470842824, -1.3349902798667799, -1.2900325126492778, -1.2450747454317754, -1.200116978214273, -1.155159210996771, -1.1102014437792687, -1.0652436765617663, -1.0202859093442642, -0.9753281421267618, -0.9303703749092596, -0.8854126076917572, -0.840454840474255, -0.7954970732567527, -0.7505393060392505, -0.7055815388217481, -0.6606237716042458, -0.6156660043867437, -0.5707082371692414, -0.525750469951739, -0.4807927027342367, -0.4358349355167346, -0.39087716829923225, -0.3459194010817299, -0.3009616338642276, -0.2560038666467255, -0.21104609942922314, -0.1660883322117208, -0.12113056499421848, -0.07617279777671637, -0.03121503055921404, 0.01374273665828829, 0.05870050387579062, 0.10365827109329273, 0.14861603831079506, 0.1935738055282974, 0.23853157274579972, 0.28348933996330206, 0.32844710718080417, 0.3734048743983063, 0.41836264161580883, 0.46332040883331094, 0.5082781760508135, 0.5532359432683156, 0.5981937104858177, 0.6431514777033203, 0.6881092449208224, 0.7330670121383245, 0.778024779355827, 0.8229825465733291, 0.8679403137908317, 0.9128980810083338, 0.9578558482258359, 1.0028136154433385, 1.0477713826608406, 1.0927291498783427, 1.1376869170958452, 1.1826446843133473, 1.22760245153085, 1.272560218748352, 1.3175179859658541, 1.3624757531833567, 1.4074335204008588, 1.452391287618361, 1.4973490548358634, 1.5423068220533656, 1.587264589270868, 1.6322223564883702, 1.6771801237058723, 1.7221378909233749, 1.767095658140877, 1.812053425358379, 1.8570111925758817, 1.9019689597933838, 1.9469267270108863, 1.9918844942283884, 2.0368422614458908, 2.081800028663393, 2.126757795880895, 2.171715563098397, 2.2166733303159, 2.261631097533402, 2.3065888647509043, 2.3515466319684064, 2.3965043991859085, 2.4414621664034106, 2.4864199336209136, 2.5313777008384157, 2.576335468055918, 2.62129323527342, 2.666251002490922, 2.711208769708424, 2.756166536925927], "1D marginal PDF (U)"=[3.982326772399644e-06, 6.516629940143578e-06, 1.0557116089551142e-05, 1.6931818596688723e-05, 2.688425390842314e-05, 4.2259897743069624e-05, 6.576502160395423e-05, 0.00010132055598135839, 0.00015453833657078382, 0.00023335170267661765, 0.0003488363927109819, 0.000516260231043145, 0.000756400187595535, 0.0010971617441281635, 0.0015755266599102634, 0.0022398396505442183, 0.003152420712772469, 0.004392456691167899, 0.006059082638219961, 0.008274510954817871, 0.011187005887437242, 0.01497343597294794, 0.01984107254255832, 0.026028245353833784, 0.033803425394029606, 0.04346228961666423, 0.05532234287707354, 0.06971473781937322, 0.08697305087857017, 0.10741894504034796, 0.131344875404652, 0.15899426330167002, 0.19053986294472255, 0.22606134859162136, 0.2655234312038861, 0.30875603909326965, 0.35543823372516675, 0.40508754946583275, 0.45705632159669246, 0.5105362885846703, 0.5645723250888404, 0.6180856006206816, 0.6699058008469067, 0.7188113445654757, 0.763575840373808, 0.8030184188056219, 0.8360551119018911, 0.8617481869098595, 0.8793503117907729, 0.8883406534683747, 0.888450476551307, 0.8796764870076109, 0.8622809962845182, 0.8367788944638114, 0.8039123351565549, 0.7646148687950843, 0.719967442270031, 0.6711491553287686, 0.6193858936043304, 0.5658999352428364, 0.5118633682663056, 0.4583576962867414, 0.4063414047588604, 0.35662657213871213, 0.3098649059602466, 0.2665429241236301, 0.22698543726111195, 0.19136605498971201, 0.15972315670897705, 0.1319796394402392, 0.10796476956318542, 0.08743659939796573, 0.07010363329096557, 0.05564470791480524, 0.04372635528045967, 0.03401721563755037, 0.0261993380623187, 0.019976433158350917, 0.015079316126325586, 0.011268897206382852, 0.008337143190112877, 0.006106455205627178, 0.0044278934587388555, 0.003178639101040938, 0.002259026638250576, 0.0015894159052049829, 0.0011071075923201198, 0.0007634457387135898, 0.0005211978235681497, 0.00035225979945604195, 0.00023570003411709, 0.00015613212805971682, 0.00010239081143089897, 6.647613516381056e-05, 4.2727414275874753e-05, 2.7188392613534048e-05, 1.712760054963687e-05, 1.0681828247669181e-05, 6.595241873864914e-06, 4.0313632842250874e-06]}]
  in  "Wmax":dbl=3.0
  in  "Wmin":dbl=-3.0
  out "Inferred true PDF":dbl[][](graph)
  in  "Lambda vector":dbl[](array[numeric])=[1.0, 1.0, 0.0, 1.0, 1.0, 1.0, 1.0, 0.0, 0.0]
  out "Calculated stats":dbl[](array[numeric])=[0.9994469063082452, 4.3517017693305085e-15, 0.0, 0.15699686515784403, 0.1553694092329591, 0.156025, 9.870419133280024e-16, 0.0, 0.0] format="%#_3g"
  out "Reconstructed, rectified pdf p(U*, V*)":dbl[][](graph)
  in  "Correct for k":bool
  in  "Const W used in proc.":dbl
  in  "h2":dbl=1.0
  in  "h1":dbl=1.0
  in  "Const k2":dbl
  in  "Const k1":dbl
  in  "Bounds multiple of st dev":i32=5
  out "Relative errors":T4(graph)={"Numeric"=0.0005530936917548246, "Numeric"=-4.3517017693305085e-15, "Numeric"=-0.0009718651578440318, "Numeric"=0.0006555907670408867, "Numeric"=-9.870419133280024e-16}
  in  "tolerance":dbl=0.001
  in  "Max iter":i32=50
  in  "NbinsW":i32=100
  in  "NbinsV":i32=100
  in  "NbinsU":i32=100
  # "U\n\nV\n\nW\n\nu^2\n\nv^2\n\nw^2\n\nuv\n\nuw\n\nvw"
  # "U\n\nV\n\nW\n\nu^2\n\nv^2\n\nw^2\n\nuv\n\nuw\n\nvw"
  # "(absolute)"
  # "U\n\nV\n\nW\n\nu^2\n\nv^2\n\nw^2\n\nuv\n\nuw\n\nvw"
  # "U\n\nV\n\nW\n\nu^2\n\nv^2\n\nw^2\n\nuv\n\nuw\n\nvw"
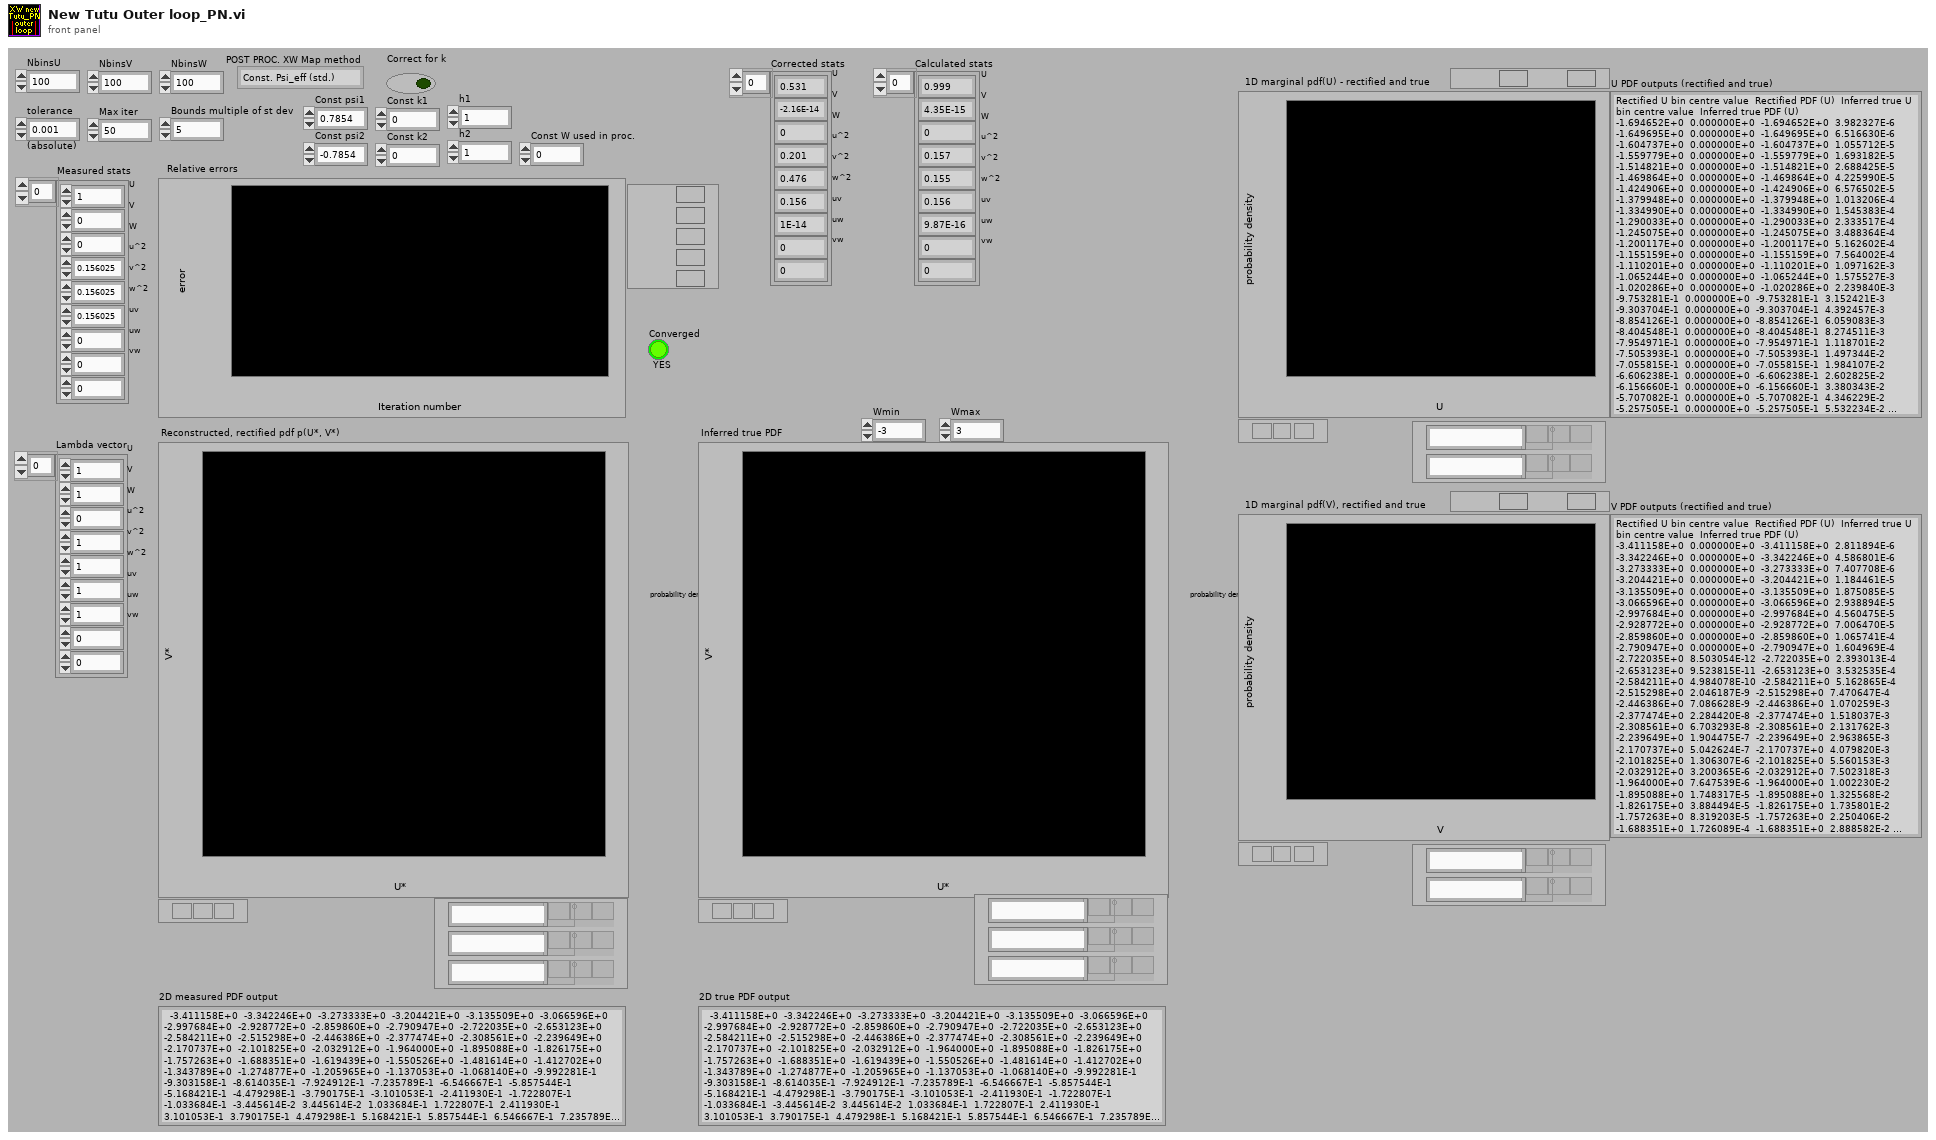
[diagram p1: front panel]
types:
  T1 = typedef "Map method.ctl" = enum16{"Triangle mesh", "Polynomial surface", "Const. Psi_eff (std.)", "Psi_eff = f(Umagn.)", "Psi_eff, k = f(Umagn.)"}
  T2 = cluster{"V bin centre vals":dbl[], "1D marginal PDF (V)":dbl[]}[]
  T3 = cluster{"U bin centre vals":dbl[], "1D marginal PDF (U)":dbl[]}[]
  T4 = cluster{"Numeric":dbl, "Numeric":dbl, "Numeric":dbl, "Numeric":dbl, "Numeric":dbl}
  T5 = cluster{"Numeric":dbl, "Numeric":dbl, "Numeric":dbl, "Numeric":dbl, "Numeric":dbl}[]
  T6 = cluster{"U bin centre vals":dbl[], "1D marginal PDF (U)":dbl[]}
  T7 = cluster{"V bin centre vals":dbl[], "1D marginal PDF (V)":dbl[]}
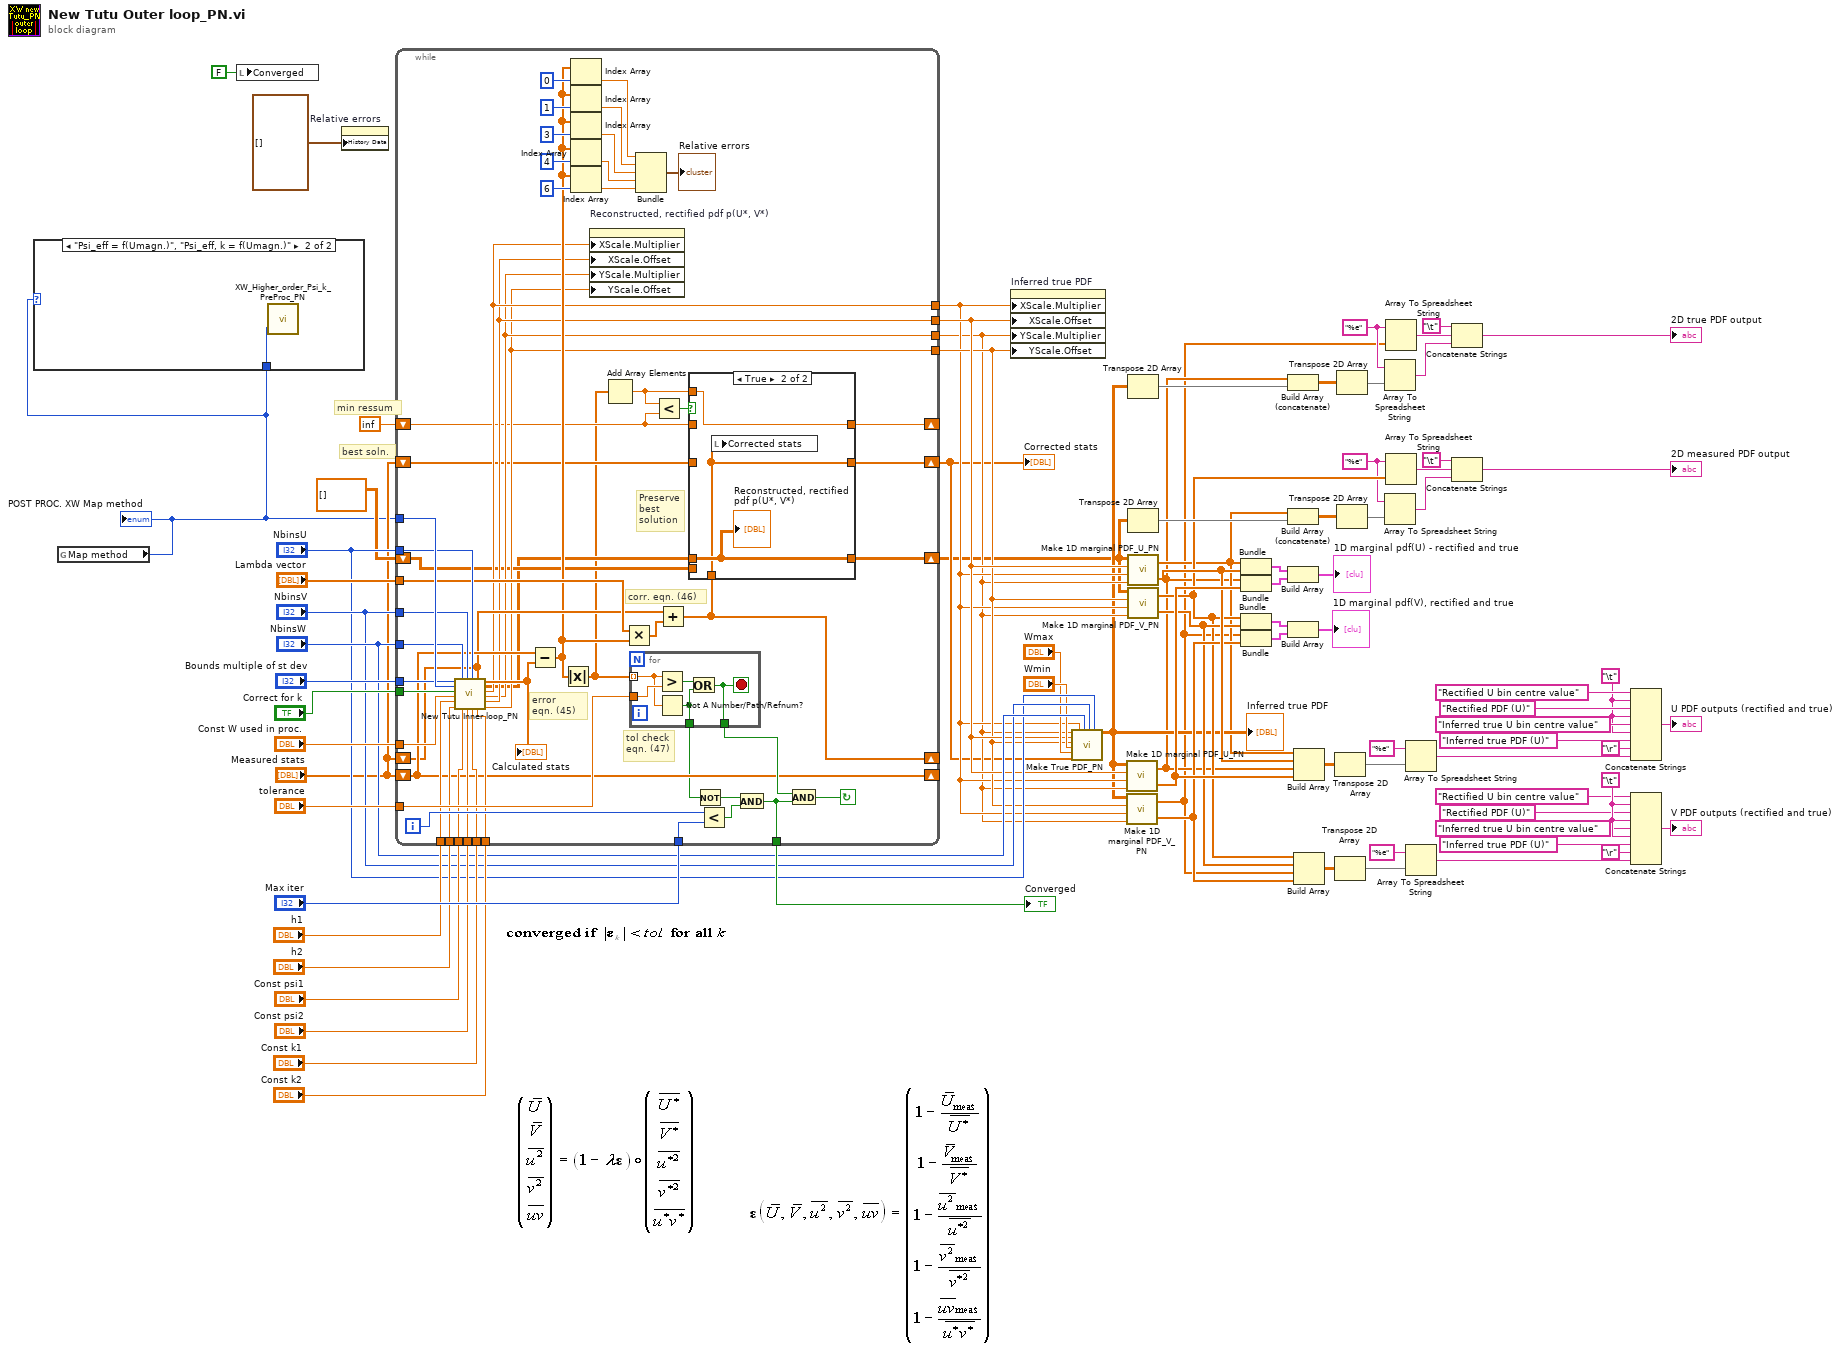
[diagram p0: block diagram]
diagram:
  w13 = "%e" ("format string")
  w22 = "%e" ("format string")
  w34 = "\t"
  w49 = "\t"
  # "best soln."
  # "min ressum"
  n1 = global read "XW_Map_Global.vi" "Map method"() -> (w1:T1)
  "POST PROC. XW Map method" <- w1
  n2 = case shown="\"Psi_eff = f(Umagn.)\", \"Psi_eff, k = f(Umagn.)\"" w1 {
    tunnel: w1 -> [_ w84]
    frame "Triangle mesh", Default {
    }
    frame "Psi_eff = f(Umagn.)", "Psi_eff, k = f(Umagn.)" {
      n3 = call "XW_Higher_order_Psi_k_PreProc_PN.vi"("Map method"=w84) -> ()  [unwired: 1 in, 1 out]
    }
  }
  n4 = local write "Converged"(FALSE ("Converged")) -> ()
  n5 = property on="Relative errors" class="WFChart (strict)"("History Data"=T5 []) -> ()  [unwired: 2 in, 2 out]
  n6 = while {
    tunnel: "Max iter" -> [w137]
    tunnel: "tolerance" -> [w136]
    shift-right: [w95] -> _
    shift-left: "Measured stats" -> [w117]
    tunnel: "Lambda vector" -> [w120]
    shift-right: [w119] -> _
    shift-left: "Measured stats" -> [w119]
    tunnel: "NbinsW" -> [w123]
    tunnel: "NbinsV" -> [w122]
    tunnel: "NbinsU" -> [w121]
    tunnel: [w96] -> w81
    tunnel: w1 -> [w125]
    tunnel: "Bounds multiple of st dev" -> [w124]
    tunnel: "Const psi1" -> [w130]
    tunnel: "Const k1" -> [w132]
    tunnel: "Const k2" -> [w133]
    tunnel: "Const psi2" -> [w131]
    tunnel: "h2" -> [w129]
    tunnel: "h1" -> [w128]
    tunnel: "Const W used in proc." -> [w127]
    tunnel: "Correct for k" -> [w126]
    tunnel: [w103] -> w61
    tunnel: [w102] -> w63
    tunnel: [w101] -> w60
    tunnel: [w100] -> w62
    shift-right: [w94] -> w2
    shift-left: dbl[][] [] ("Re-constructed pdf") -> [w93]
    shift-right: [w90] -> w3
    shift-left: "Measured stats" -> [w91]
    shift-right: [w89] -> _
    shift-left: inf -> [w87]
    i -> [w138]
    stop <- w135 continue-if-true
    # "Preserve best solution"
    # "tol check eqn. (47)"
    # "corr. eqn. (46)"
    # "error\neqn. (45)"
    n7 = call "New Tutu Inner loop_PN.vi"("Bounds multiple of st dev"=w124, "POST PROC. XW Map method"=w125, "Correct for k"=w126, "Const W used in proc."=w127, "h1"=w128, "h2"=w129, "NbinsW"=w123, "Const psi1 (rad)"=w130, "NbinsV"=w122, "Const psi2 (rad)"=w131, "NbinsU"=w121, "Const k1"=w132, "Current stats"=w117, "Const k2"=w133) -> ("Calculated stats"=w118:dbl[], "Re-constructed pdf"=w92:dbl[][], "dU*"=w103:dbl, "dV*"=w101:dbl, "U*min"=w102:dbl, "V*min"=w100:dbl)
    "Calculated stats" <- w118
    n8 = Subtract(x=w119, y=w118) -> (x-y=w107:dbl[])
    n9 = Absolute Value(x=w107) -> (abs(x)=w86:dbl[])
    n10 = Index Array(array=w107, index=0) -> (element=w114:dbl)
    n11 = Index Array(array=w107, index=1) -> (element=w112:dbl)
    n12 = Index Array(array=w107, index=3) -> (element=w106:dbl)
    n13 = Index Array(array=w107, index=4) -> (element=w105:dbl)
    n14 = Index Array(array=w107, index=6) -> (element=w104:dbl)
    n15 = property on="Reconstructed, rectified pdf p(U*, V*)" class="IntGraph (strict)"("XScale.Multiplier"=w103, "XScale.Offset"=w102, "YScale.Multiplier"=w101, "YScale.Offset"=w100) -> ()  [unwired: 2 in, 2 out]
    n16 = Add Array Elements(numeric array=w86) -> (sum=w88:dbl)
    n17 = Multiply(x=w120, y=w107) -> (x*y=w116:dbl[])
    n18 = for {
      tunnel: w86 -> [w146] mode=indexing
      tunnel: w136 -> [w149]
      tunnel: [w147] -> w134
      tunnel: [w145] -> w98
      stop <- w147 stop-if-true
      n19 = Greater?(x=w146, y=w149) -> (0:w148:bool)
      n20 = Not A Number/Path/Refnum?(number/path/refnum=w146) -> (NaN/Path/Refnum?=w145:bool)
      n21 = Or(x=w148, y=w145) -> (x .or. y?=w147:bool)
    }
    n22 = Bundle("Numeric"=w114, "Numeric"=w112, "Numeric"=w106, "Numeric"=w105, "Numeric"=w104) -> (→"Relative errors":T4)  [unwired: 1 out]
    n23 = Less?(x=w88, y=w87) -> (x < y?=w85:bool)
    n24 = Add(x=w117, y=w116) -> (x+y=w95:dbl[])
    n25 = case shown="True" w85 {
      tunnel: [w140 w144] -> w89
      tunnel: w88 -> [_ w144]
      tunnel: [w141 w142] -> w90
      tunnel: w95 -> [_ w142]
      tunnel: w91 -> [w141 _]
      tunnel: w87 -> [w140 _]
      tunnel: [w139 w143] -> w94
      tunnel: w92 -> [_ w143]
      tunnel: w93 -> [w139 _]
      frame False {
      }
      frame True {
        n26 = local write "Corrected stats"(w142) -> ()
        "Reconstructed, rectified pdf p(U*, V*)" <- w143
      }
    }
    n27 = Not(x=w98) -> (.not. x?=w99:bool)
    n28 = Less?(x=w138, y=w137) -> (x < y?=w97:bool)
    n29 = And(x=w99, y=w97) -> (x .and. y?=w96:bool)
    n30 = And(x=w134, y=w96) -> (x .and. y?=w135:bool)
  }
  "Converged" <- w81
  "Corrected stats" <- w3
  n31 = property on="Inferred true PDF" class="IntGraph (strict)"("XScale.Multiplier"=w61, "XScale.Offset"=w63, "YScale.Multiplier"=w60, "YScale.Offset"=w62) -> ()  [unwired: 2 in, 2 out]
  n32 = call "Make True PDF_PN.vi"("dV*"=w60, "U*min"=w63, "V*min"=w62, "Wmin"="Wmin", "Wmax"="Wmax", "Current stats"=w3, "dU*"=w61, "NbinsW"="NbinsW", "NbinsV"="NbinsV", "NbinsU"="NbinsU") -> ("True pdf"=w18:dbl[][])  [unwired: 9 out]
  "Inferred true PDF" <- w18
  n33 = call "Make 1D marginal PDF_U_PN.vi"("dV"=w60, "dU*"=w61, "U*min"=w63, "2D PDF (U,V)"=w18) -> ("1D marginal PDF (U)"=w42:dbl[], "U bin centre vals"=w9:dbl[])
  n34 = call "Make 1D marginal PDF_V_PN.vi"("dV"=w60, "dU*"=w61, "V*min"=w62, "2D PDF (U,V)"=w18) -> ("1D marginal PDF (V)"=w29:dbl[], "V bin centre vals"=w8:dbl[])
  n35 = Transpose 2D Array(2D array=w18) -> (transposed array=w17:dbl[][])
  n36 = Transpose 2D Array(2D array=w2) -> (transposed array=w26:dbl[][])
  n37 = call "Make 1D marginal PDF_U_PN.vi"("dV"=w60, "dU*"=w61, "U*min"=w63, "2D PDF (U,V)"=w2) -> ("1D marginal PDF (U)"=w41:dbl[], "U bin centre vals"=w16:dbl[])
  n38 = call "Make 1D marginal PDF_V_PN.vi"("dV"=w60, "dU*"=w61, "V*min"=w62, "2D PDF (U,V)"=w2) -> ("1D marginal PDF (V)"=w28:dbl[], "V bin centre vals"=w23:dbl[])
  n39 = Bundle("U bin centre vals"=w16, "1D marginal PDF (U)"=w41) -> (w59:T6)  [unwired: 1 out]
  n40 = Bundle("U bin centre vals"=w9, "1D marginal PDF (U)"=w42) -> (w58:T6)  [unwired: 1 out]
  n41 = Bundle("V bin centre vals"=w23, "1D marginal PDF (V)"=w28) -> (w55:T7)  [unwired: 1 out]
  n42 = Bundle("V bin centre vals"=w8, "1D marginal PDF (V)"=w29) -> (w56:T7)  [unwired: 1 out]
  n43 = Build Array (concatenate)(w9, w17) -> (w10:dbl[][])
  n44 = Build Array (concatenate)(w16, w26) -> (w27:dbl[][])
  n45 = Build Array(w59, w58) -> (→"1D marginal pdf(U) - rectified and true":T3)
  n46 = Build Array(w55, w56) -> (→"1D marginal pdf(V), rectified and true":T2)
  n47 = Build Array(w16, w41, w9, w42) -> (w44:dbl[][])
  n48 = Build Array(w23, w28, w8, w29) -> (w39:dbl[][])
  n49 = Transpose 2D Array(2D array=w44) -> (transposed array=w43:dbl[][])
  n50 = Transpose 2D Array(2D array=w39) -> (transposed array=w40:dbl[][])
  n51 = Transpose 2D Array(2D array=w10) -> (transposed array=w11:dbl[][])
  n52 = Transpose 2D Array(2D array=w27) -> (transposed array=w25:dbl[][])
  n53 = Array To Spreadsheet String(array=w11, 3:w13) -> (spreadsheet string=w15:string)  [unwired: 1 out]
  n54 = Array To Spreadsheet String(array=w25, 3:w22) -> (spreadsheet string=w20:string)  [unwired: 1 out]
  n55 = Array To Spreadsheet String(array=w8, 3:w13) -> (spreadsheet string=w14:string)  [unwired: 1 out]
  n56 = Array To Spreadsheet String(array=w23, 3:w22) -> (spreadsheet string=w21:string)  [unwired: 1 out]
  n57 = Array To Spreadsheet String(array=w43, 3:"%e" ("format string")) -> (spreadsheet string=w46:string)  [unwired: 1 out]
  n58 = Array To Spreadsheet String(array=w40, 3:"%e" ("format string")) -> (spreadsheet string=w37:string)  [unwired: 1 out]
  n59 = Concatenate Strings("\t", w14, w15) -> (→"2D true PDF output":string)
  n60 = Concatenate Strings("\t", w21, w20) -> (→"2D measured PDF output":string)
  n61 = Concatenate Strings("Rectified U bin centre value", w49, "Rectified PDF (U)", w49, "Inferred true U bin centre value", w49, "Inferred true PDF (U)", "\r", w46) -> (→"U PDF outputs (rectified and true)":string)
  n62 = Concatenate Strings("Rectified U bin centre value", w34, "Rectified PDF (U)", w34, "Inferred true U bin centre value", w34, "Inferred true PDF (U)", "\r", w37) -> (→"V PDF outputs (rectified and true)":string)
